vi "Lab Panel V4.5.vi"() -> ()   [LabVIEW 2013]
uses:
  <vilib>/Platform/TimedLoop/XDataNode/timing_clust.ctl
  <vilib>/Platform/TimedLoop/XDataNode/nitl_modes.ctl
  <vilib>/Platform/TimedLoop/XDataNode/wakeup.ctl
  Global 1.vi
  <vilib>/platform/TimedLoop/XDataNode/XDataNode.xnode
  <vilib>/Platform/TimedLoop/XDataNode/XDNodeRunTimeDep.lvlib
panel:
  in  "ADMIN PAGE":bool
  out "TEMP update":bool
  out "AI update":bool
  in  "Tab Control 2":T1(tab)
  out "SIG LAB05-2":T2 {"PF" format="%.2f"; "AMPS" format="%.1f"}
  out "SIG LAB05-1":T2 {"PF" format="%.2f"; "AMPS" format="%.1f"}
  out "SIG LAB04-2":T2 {"PF" format="%.2f"; "AMPS" format="%.1f"}
  out "SIG LAB04-1":T2 {"PF" format="%.2f"; "AMPS" format="%.1f"}
  out "SIG LAB03-2":T2 {"PF" format="%.2f"; "AMPS" format="%.1f"}
  out "SIG LAB03-1":T2 {"PF" format="%.2f"; "AMPS" format="%.1f"}
  out "SIG LAB02-2":T2 {"PF" format="%.2f"; "AMPS" format="%.1f"}
  in  "RUN LAB01-1":bool
  in  "O/I  LAB05-1":bool
  in  "O/I  LAB05-2":bool
  in  "O/I  LAB04-1":bool
  in  "O/I  LAB04-2":bool
  in  "O/I  LAB02-1":bool
  in  "O/I  LAB02-2":bool
  in  "O/I  LAB01-2":bool
  in  "O/I  LAB01-1":bool
  in  "O/I  LAB03-1":bool
  in  "RUN LAB05-2":bool
  in  "RUN LAB05-1":bool
  in  "RUN LAB04-2":bool
  in  "RUN LAB04-1":bool
  in  "RUN LAB03-2":bool
  in  "RUN LAB03-1":bool
  in  "RUN LAB02-2":bool
  in  "RUN LAB02-1":bool
  in  "RUN LAB01-2":bool
  in  "SELECT LAB05-2":T3(radio)
  in  "SELECT LAB05-1":T3(radio)
  in  "SELECT LAB04-2":T3(radio)
  in  "SELECT LAB04-1":T3(radio)
  in  "SELECT LAB03-2":T3(radio)
  in  "SELECT LAB03-1":T3(radio)
  in  "SELECT LAB02-2":T3(radio)
  in  "SELECT LAB02-1":T3(radio)
  in  "SELECT LAB01-2":T3(radio)
  in  "SELECT LAB01-1":T3(radio)
  in  "O/I  LAB03-2":bool
  out "SIG LAB01-1":T2 {"PF" format="%.2f"; "AMPS" format="%.1f"}
  out "SIG LAB01-2":T2 {"PF" format="%.2f"; "AMPS" format="%.1f"}
  out "SIG LAB02-1":T2 {"PF" format="%.2f"; "AMPS" format="%.1f"}
  out "DISP LAB05-2":T4 {"MINS" format="%.2g"}
  out "DISP LAB05-1":T4 {"MINS" format="%.2g"}
  out "DISP LAB04-2":T4 {"MINS" format="%.2g"}
  out "DISP LAB04-1":T4 {"MINS" format="%.2g"}
  out "DISP LAB03-2":T4 {"MINS" format="%.2g"}
  out "DISP LAB03-1":T4 {"MINS" format="%.2g"}
  in  "SET LAB05-2":T5={"NAME"="", "DESCRIPTION"="", "CYCLES"=5.0, "T-RISE mins"=0.0, "T-RISE deg C"=0.0} {"CYCLES" min=5.0 step=1.0}
  in  "SET LAB05-1":T5={"NAME"="", "DESCRIPTION"="", "CYCLES"=5.0, "T-RISE mins"=0.0, "T-RISE deg C"=0.0} {"CYCLES" min=5.0 step=1.0}
  in  "SET LAB04-2":T5={"NAME"="", "DESCRIPTION"="", "CYCLES"=5.0, "T-RISE mins"=0.0, "T-RISE deg C"=0.0} {"CYCLES" min=5.0 step=1.0}
  in  "SET LAB04-1":T5={"NAME"="", "DESCRIPTION"="", "CYCLES"=5.0, "T-RISE mins"=0.0, "T-RISE deg C"=0.0} {"CYCLES" min=5.0 step=1.0}
  in  "SET LAB03-2":T5={"NAME"="", "DESCRIPTION"="", "CYCLES"=5.0, "T-RISE mins"=0.0, "T-RISE deg C"=0.0} {"CYCLES" min=5.0 step=1.0}
  in  "SET LAB03-1":T5={"NAME"="", "DESCRIPTION"="", "CYCLES"=5.0, "T-RISE mins"=0.0, "T-RISE deg C"=0.0} {"CYCLES" min=5.0 step=1.0}
  out "DISP LAB02-2":T4 {"MINS" format="%.2g"}
  out "DISP LAB02-1":T4 {"MINS" format="%.2g"}
  in  "SET LAB02-2":T5={"NAME"="", "DESCRIPTION"="", "CYCLES"=5.0, "T-RISE mins"=0.0, "T-RISE deg C"=0.0} {"CYCLES" min=5.0 step=1.0}
  in  "SET LAB02-1":T5={"NAME"="", "DESCRIPTION"="", "CYCLES"=5.0, "T-RISE mins"=0.0, "T-RISE deg C"=0.0} {"CYCLES" min=5.0 step=1.0}
  out "RESULT LAB05-2":bool
  out "RESULT LAB05-1":bool
  out "RESULT LAB04-2":bool
  out "RESULT LAB04-1":bool
  out "RESULT LAB03-2":bool
  out "RESULT LAB03-1":bool
  out "RESULT LAB02-2":bool
  out "RESULT LAB02-1":bool
  out "RESULT LAB01-2":bool
  out "RESULT LAB01-1":bool
  in  "SET LAB01-1":T5={"NAME"="", "DESCRIPTION"="", "CYCLES"=5.0, "T-RISE mins"=0.0, "T-RISE deg C"=0.0} {"CYCLES" min=5.0 step=1.0}
  in  "SET LAB01-2":T5={"NAME"="", "DESCRIPTION"="", "CYCLES"=5.0, "T-RISE mins"=0.0, "T-RISE deg C"=0.0} {"CYCLES" min=5.0 step=1.0}
  out "DISP LAB01-1":T4 {"MINS" format="%.2g"}
  out "DISP LAB01-2":T4 {"MINS" format="%.2f"}
  out "TEMP RISE LAB05-2":cluster{"TL":dbl, "TN":dbl}
  out "TEMP RISE LAB05-1":cluster{"TL":dbl, "TN":dbl}
  out "TEMP RISE LAB04-2":cluster{"TL":dbl, "TN":dbl}
  out "TEMP RISE LAB04-1":cluster{"TL":dbl, "TN":dbl}
  out "TEMP RISE LAB03-2":cluster{"TL":dbl, "TN":dbl}
  out "TEMP RISE LAB03-1":cluster{"TL":dbl, "TN":dbl}
  out "TEMP RISE LAB02-2":cluster{"TL":dbl, "TN":dbl}
  out "TEMP RISE LAB02-1":cluster{"TL":dbl, "TN":dbl}
  out "TEMP RISE LAB01-2":cluster{"TL":dbl, "TN":dbl}
  out "TEMP RISE LAB01-1":cluster{"TL":dbl, "TN":dbl}
  in  "JIG OFF TIME (S)":dbl=2.0 min=2.0 max=10.0 step=0.5 format="%.1g"
  in  "JIG ON TIME (S)":dbl=1.0 min=1.0 max=10.0 step=0.5 format="%.1g"
  out "JIG LAB05-2":bool
  out "JIG LAB05-1":bool
  out "JIG LAB04-2":bool
  out "JIG LAB04-1":bool
  out "JIG LAB03-2":bool
  out "JIG LAB03-1":bool
  out "JIG LAB02-2":bool
  out "JIG LAB02-1":bool
  out "JIG LAB01-2":bool
  out "JIG LAB01-1":bool
  out "TEMP START LAB01-1":cluster{"TL":dbl, "TN":dbl}
  out "TEMP START LAB02-1":cluster{"TL":dbl, "TN":dbl}
  out "TEMP START LAB03-1":cluster{"TL":dbl, "TN":dbl}
  out "TEMP START LAB04-1":cluster{"TL":dbl, "TN":dbl}
  out "TEMP START LAB01-2":cluster{"TL":dbl, "TN":dbl}
  out "TEMP START LAB02-2":cluster{"TL":dbl, "TN":dbl}
  out "TEMP START LAB03-2":cluster{"TL":dbl, "TN":dbl}
  out "TEMP START LAB04-2":cluster{"TL":dbl, "TN":dbl}
  out "TEMP START LAB05-2":cluster{"TL":dbl, "TN":dbl}
  out "TEMP START LAB05-1":cluster{"TL":dbl, "TN":dbl}
  in  "MAIL SETTINGS":T6
  out "MAIL REPORT":string
  in  "TO (string):":string
  in  "Send Mail Now":bool
  in  "Auto Mail Send":bool
  in  "Network Directory":path
  out "CAL LAB01":T7 {"2 (TN) cal" min=0.0 step=0.01 format="%.2f"; "2 (TL) cal" min=0.0 step=0.01 format="%.2f"; "2 (PF) cal" min=0.0 step=0.01 format="%.2f"; "2 (V) cal" min=0.0 step=0.01 format="%.2f"; "2 (A) cal" min=0.0 step=0.01 format="%.2f"; "1 (TN) cal" min=0.0 step=0.01 format="%.2f"; "1 (TL) cal" min=0.0 step=0.01 format="%.2f"; "1 (PF) cal" min=0.0 step=0.01 format="%.2f"; "1 (V) cal" min=0.0 step=0.01 format="%.2f"; "1  (A) cal" min=0.0 step=0.01 format="%.2f"}
  out "CAL LAB03":T7 {"2 (TN) cal" min=0.0 step=0.01 format="%.2f"; "2 (TL) cal" min=0.0 step=0.01 format="%.2f"; "2 (PF) cal" min=0.0 step=0.01 format="%.2f"; "2 (V) cal" min=0.0 step=0.01 format="%.2f"; "2 (A) cal" min=0.0 step=0.01 format="%.2f"; "1 (TN) cal" min=0.0 step=0.01 format="%.2f"; "1 (TL) cal" min=0.0 step=0.01 format="%.2f"; "1 (PF) cal" min=0.0 step=0.01 format="%.2f"; "1 (V) cal" min=0.0 step=0.01 format="%.2f"; "1  (A) cal" min=0.0 step=0.01 format="%.2f"}
  out "CAL LAB02":T8 {"2 (TN) cal" min=0.0 step=0.01 format="%.2f"; "2 (TL) cal" min=0.0 step=0.01 format="%.2f"; "2 (PF) cal" min=0.0 step=0.01 format="%.2f"; "2 (V) cal" min=0.0 step=0.01 format="%.2f"; "2 (A) cal" min=0.0 step=0.01 format="%.2f"; "1 (TN) cal" min=0.0 step=0.01 format="%.2f"; "1 (TL) cal" min=0.0 step=0.01 format="%.2f"; "1 (PF) cal" min=0.0 step=0.01 format="%.2f"; "1 (V) cal" min=0.0 step=0.01 format="%.2f"; "1 (A) cal" min=0.0 step=0.01 format="%.2f"}
  out "CAL LAB05":T7 {"2 (TN) cal" min=0.0 step=0.01 format="%.2f"; "2 (TL) cal" min=0.0 step=0.01 format="%.2f"; "2 (PF) cal" min=0.0 step=0.01 format="%.2f"; "2 (V) cal" min=0.0 step=0.01 format="%.2f"; "2 (A) cal" min=0.0 step=0.01 format="%.2f"; "1 (TN) cal" min=0.0 step=0.01 format="%.2f"; "1 (TL) cal" min=0.0 step=0.01 format="%.2f"; "1 (PF) cal" min=0.0 step=0.01 format="%.2f"; "1 (V) cal" min=0.0 step=0.01 format="%.2f"; "1  (A) cal" min=0.0 step=0.01 format="%.2f"}
  out "CAL LAB04":T7 {"2 (TN) cal" min=0.0 step=0.01 format="%.2f"; "2 (TL) cal" min=0.0 step=0.01 format="%.2f"; "2 (PF) cal" min=0.0 step=0.01 format="%.2f"; "2 (V) cal" min=0.0 step=0.01 format="%.2f"; "2 (A) cal" min=0.0 step=0.01 format="%.2f"; "1 (TN) cal" min=0.0 step=0.01 format="%.2f"; "1 (TL) cal" min=0.0 step=0.01 format="%.2f"; "1 (PF) cal" min=0.0 step=0.01 format="%.2f"; "1 (V) cal" min=0.0 step=0.01 format="%.2f"; "1  (A) cal" min=0.0 step=0.01 format="%.2f"}
  out "calibration file error out":errorcluster
  in  "CALIBRATE":bool
  out "ON L05-2":cluster{"amps":dbl, "volts":dbl, "pf":dbl}
  out "ON L05-1":cluster{"amps":dbl, "volts":dbl, "pf":dbl}
  out "FAIL LAB05-2":cluster{"LO":dbl, "HI":dbl}
  out "FAIL LAB05-1":cluster{"LO":dbl, "HI":dbl}
  out "FAIL LAB04-2":cluster{"LO":dbl, "HI":dbl}
  out "FAIL LAB04-1":cluster{"LO":dbl, "HI":dbl}
  out "FAIL LAB03-2":cluster{"LO":dbl, "HI":dbl}
  out "FAIL LAB03-1":cluster{"LO":dbl, "HI":dbl}
  out "FAIL LAB02-2":cluster{"LO":dbl, "HI":dbl}
  out "FAIL LAB02-1":cluster{"LO":dbl, "HI":dbl}
  out "FAIL LAB01-2":cluster{"LO":dbl, "HI":dbl}
  out "FAIL LAB01-1":cluster{"LO":dbl, "HI":dbl}
  out "ON L01-1":cluster{"amps":dbl, "volts":dbl, "pf":dbl}
  out "ON L01-2":cluster{"amps":dbl, "volts":dbl, "pf":dbl}
  out "ON L02-1":cluster{"amps":dbl, "volts":dbl, "pf":dbl}
  out "ON L02-2":cluster{"amps":dbl, "volts":dbl, "pf":dbl}
  out "ON L03-1":cluster{"amps":dbl, "volts":dbl, "pf":dbl}
  out "ON L03-2":cluster{"amps":dbl, "volts":dbl, "pf":dbl}
  out "ON L04-1":cluster{"amps":dbl, "volts":dbl, "pf":dbl}
  out "ON L04-2":cluster{"amps":dbl, "volts":dbl, "pf":dbl}
  out "TEST VOLTS CHART":T9(graph)
  in  "Select  Cycle":enum32{"ON CYCLE", "OFF CYCLE"}(radio)
  out "TEST AMPS CHART":T9(graph)
  out "TEMPERATURE (N) CHART":T9(graph)
  out "TEMPERATURE (L) CHART":T9(graph)
  in  "SAMPLES":dbl
  in  "RATE (Hz)":dbl
  in  "JIG TEST":T10
  in  "C drive data root dir":path
  out "run lab05-2":bool
  out "run lab05-1":bool
  out "run lab04-2":bool
  out "run lab04-1":bool
  out "run lab03-2":bool
  out "run lab03-1":bool
  out "run lab02-2":bool
  out "run lab02-1":bool
  out "run lab01-2":bool
  out "run lab01-1":bool
  out "stop2":bool
  in  "Tab Control":T11(tab)
  out "LAB01-2 (GRAPH)":dynamicdata(graph)
  out "LAB01-1 (GRAPH)":dynamicdata(graph)
  out "LAB02-2 (GRAPH)":dynamicdata(graph)
  out "LAB02-1 (GRAPH)":dynamicdata(graph)
  out "LAB03-2 (GRAPH)":dynamicdata(graph)
  out "LAB03-1 (GRAPH)":dynamicdata(graph)
  out "LAB04-2 (GRAPH)":dynamicdata(graph)
  out "LAB04-1 (GRAPH)":dynamicdata(graph)
  out "LAB05-2 (GRAPH)":dynamicdata(graph)
  out "LAB05-1 (GRAPH)":dynamicdata(graph)
  out "LAB05 TEMP":T12
  out "LAB04 TEMP":T12
  out "LAB02 TEMP":T12
  out "LAB01 TEMP":T12
  out "LAB03 TEMP":T12
  out "Analog Error Array":errorcluster[](array[cluster])
  out "AI loop time":dbl format="%.6g"
  out "loops":dbl
  in  "loop  delay(mS)":dbl
  out "on loops":dbl
  out "off loops":dbl
  out "jig cycle":dbl
  out "TDMS LAB01-1":refnum<k34>
  out "data file error":errorcluster
  out "TDMS LAB02-1":refnum<k34>
  out "TDMS LAB01-2":refnum<k34>
  out "TDMS LAB02-2":refnum<k34>
  out "TDMS LAB03-1":refnum<k34>
  out "TDMS LAB03-2":refnum<k34>
  out "TDMS LAB04-1":refnum<k34>
  out "TDMS LAB04-2":refnum<k34>
  out "TDMS LAB05-1":refnum<k34>
  out "TDMS LAB05-2":refnum<k34>
  out "mail control":string
  out "File Time Stamp":timestamp
  in  "stop":bool
  # "LAB01"
  # "LAB02"
  # "LAB05"
  # "LAB03"
  # "LAB04"
  # "LAB01"
  # "LAB02"
  # "LAB03"
  # "LAB04"
  # "LAB05"
  # "JIG SET"
  # "(Enter recipients address seperated by comma)"
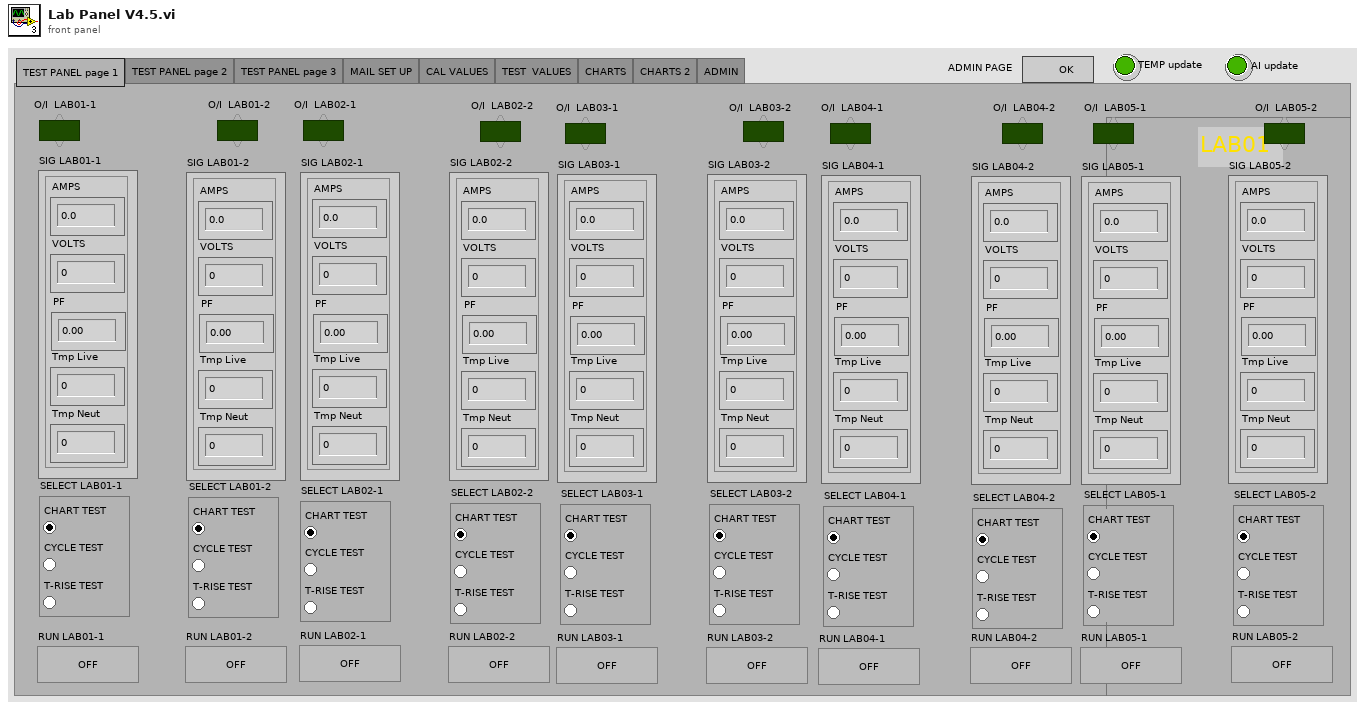
[diagram p1: front panel]
types:
  T1 = enum32{"TEST PANEL page 1", "TEST PANEL page 2", "TEST PANEL page 3", "MAIL SET UP", "CAL VALUES", "TEST  VALUES", "CHARTS", "CHARTS 2", "ADMIN"}
  T2 = cluster{"AMPS":dbl, "VOLTS":dbl, "PF":dbl, "Tmp Live":dbl, "Tmp Neut":dbl}
  T3 = enum32{"CHART TEST", "CYCLE TEST", "T-RISE TEST"}
  T4 = cluster{"CYCLE":dbl, "MINS":dbl, "STATUS":string}
  T5 = cluster{"NAME":string, "DESCRIPTION":string, "CYCLES":dbl, "T-RISE mins":dbl, "T-RISE deg C":dbl}
  T6 = cluster{"OUT SERVER ADDRESS":string, "FROM ACCOUNT":string, "USER NAME":string, "PASSWORD":string, "TEST MAIL":bool, "TEST MAIL STATUS":string, "mail error":errorcluster}
  T7 = cluster{"1  (A) cal":dbl, "1 (V) cal":dbl, "1 (PF) cal":dbl, "1 (TL) cal":dbl, "1 (TN) cal":dbl, "2 (A) cal":dbl, "2 (V) cal":dbl, "2 (PF) cal":dbl, "2 (TL) cal":dbl, "2 (TN) cal":dbl}
  T8 = cluster{"1 (A) cal":dbl, "1 (V) cal":dbl, "1 (PF) cal":dbl, "1 (TL) cal":dbl, "1 (TN) cal":dbl, "2 (A) cal":dbl, "2 (V) cal":dbl, "2 (PF) cal":dbl, "2 (TL) cal":dbl, "2 (TN) cal":dbl}
  T9 = cluster{"AMPS":dbl, "AMPS":dbl, "AMPS":dbl, "AMPS":dbl, "AMPS":dbl, "AMPS":dbl, "AMPS":dbl, "AMPS":dbl, "AMPS":dbl, "AMPS":dbl}
  T10 = cluster{" LAB01-1":bool, " LAB01-2":bool, "LAB02-1":bool, " LAB02-2":bool, "LAB03-1":bool, "LAB03-2":bool, "LAB04-1":bool, "LAB04-2":bool, "LAB05-1":bool, "LAB05-2":bool}
  T11 = enum32{"LAB01", "LAB02", "LAB03", "LAB04", "LAB05", "TEMPERATURE", "ERROR"}
  T12 = cluster{"T1 Live":dbl, "T1 Neut":dbl, "T2 Live":dbl, "T2 Neut":dbl, "ID":dbl, "ER":dbl}
  T13 = enum8{"Enabled", "Disabled", "Disabled and Grayed Out"}
  T14 = typedef "XDNodeRunTimeDep.lvlib/timing_clust.ctl" = cluster{"Expected End [f-1]":u64, "Actual End [f-1]":u64, "Finished Late? [f-1]":bool, "Expected End [i-1]":u64, "Actual End [i-1]":u64, "Finished Late? [i-1]":bool, "Expected Start [i]":u64, "Actual Start [i]":u64, "Expected Start [f]":u64, "Actual Start [f]":u64, "Source Name":string, "Structure Name":string, "Period":i64, "Deadline":i64, "Offset":i64, "Start":i64, "Priority":i32, "Timeout":i32, "Mode":T15, "Wakeup Reason":T16, "Error":errorcluster, "Source Type":string, "Secondary Source Type":string, "Global End Time":u64, "Global Start Time":u64, "Frame Duration":u64, "Iteration Duration":u64, "Assigned CPU":i32, "I/O Scan Engine Mode":u32}
  T15 = typedef "XDNodeRunTimeDep.lvlib/nitl_modes.ctl" = enum32{"No Change", "Process missed periods, maintain original phase", "Discard missed periods, maintain original phase", "Process missed periods, ignore original phase", "Discard missed periods, ignore original phase"}
  T16 = typedef "XDNodeRunTimeDep.lvlib/wakeup.ctl" = enum32{"Normal", "Aborted", "Asynchronous wakeup", "Timing source error", "Timed loop error", "Timeout"}
  T17 = enum16{"open", "open or create", "create or replace", "create", "open (read-only)"}
  T18 = enum16{"open", "replace", "create", "open or create", "replace or create", "replace or create with confirmation"}
  T19 = cluster{"SET LAB01-1":cluster{"NAME":string, "DESCRIPTION":string, "CYCLES":dbl, "T-RISE mins":dbl, "T-RISE deg C":dbl}, "SET LAB01-2":cluster{"NAME":string, "DESCRIPTION":string, "CYCLES":dbl, "T-RISE mins":dbl, "T-RISE deg C":dbl}, "SET LAB02-1":cluster{"NAME":string, "DESCRIPTION":string, "CYCLES":dbl, "T-RISE mins":dbl, "T-RISE deg C":dbl}, "SET LAB02-2":cluster{"NAME":string, "DESCRIPTION":string, "CYCLES":dbl, "T-RISE mins":dbl, "T-RISE deg C":dbl}, "SET LAB03-1":cluster{"NAME":string, "DESCRIPTION":string, "CYCLES":dbl, "T-RISE mins":dbl, "T-RISE deg C":dbl}, "SET LAB03-2":cluster{"NAME":string, "DESCRIPTION":string, "CYCLES":dbl, "T-RISE mins":dbl, "T-RISE deg C":dbl}, "SET LAB04-1":cluster{"NAME":string, "DESCRIPTION":string, "CYCLES":dbl, "T-RISE mins":dbl, "T-RISE deg C":dbl}, "SET LAB04-2":cluster{"NAME":string, "DESCRIPTION":string, "CYCLES":dbl, "T-RISE mins":dbl, "T-RISE deg C":dbl}, "SET LAB05-1":cluster{"NAME":string, "DESCRIPTION":string, "CYCLES":dbl, "T-RISE mins":dbl, "T-RISE deg C":dbl}, "SET LAB05-2":cluster{"NAME":string, "DESCRIPTION":string, "CYCLES":dbl, "T-RISE mins":dbl, "T-RISE deg C":dbl}, "Network Directory":path, "C drive data root dir":path, "RATE (Hz)":dbl, "SAMPLES":dbl}
  T20 = cluster{"MAIL SETTINGS":cluster{"OUT SERVER ADDRESS":string, "FROM ACCOUNT":string, "USER NAME":string, "PASSWORD":string, "TEST MAIL":bool, "TEST MAIL STATUS":string, "mail error":errorcluster}, "Auto Mail Send":bool, string}
  T21 = cluster{"T1":dbl, "T2":dbl, "T3":dbl, "T4":dbl, "ID":dbl, "ER":dbl}
  T22 = cluster{"LAB01-1 (A)":dbl, "LAB01-1 (V)":dbl, "LAB01-1 (PF)":dbl, "LAB01-2 (A)":dbl, "LAB01-2 (V)":dbl, "LAB01-2 (PF)":dbl}
  T23 = cluster{"LAB02-1 (A)":dbl, "LAB02-1 (V)":dbl, "LAB02-1 (PF)":dbl, "LAB02-2 (A)":dbl, "LAB02-2 (V)":dbl, "LAB02-2 (PF)":dbl}
  T24 = cluster{"LAB03-1 (A)":dbl, "LAB03-1 (V)":dbl, "LAB03-1 (PF)":dbl, "LAB03-2 (A)":dbl, "LAB03-2 (V)":dbl, "LAB03-2 (PF)":dbl}
  T25 = cluster{"LAB04-1 (A)":dbl, "LAB04-1 (V)":dbl, "LAB04-1 (PF)":dbl, "LAB04-2 (A)":dbl, "LAB04-2 (V)":dbl, "LAB04-2 (PF)":dbl}
  T26 = cluster{"LAB05-1 (A)":dbl, "LAB05-1 (V)":dbl, "LAB05-1 (PF)":dbl, "LAB05-2 (A)":dbl, "LAB05-2 (V)":dbl, "LAB05-2 (PF)":dbl}
  T27 = cluster{"VOLTS":dbl, "VOLTS":dbl, "VOLTS":dbl, "VOLTS":dbl, "VOLTS":dbl, "VOLTS":dbl, "VOLTS":dbl, "VOLTS":dbl, "VOLTS":dbl, "VOLTS":dbl}
  T28 = cluster{"Tmp Live":dbl, "Tmp Live":dbl, "Tmp Live":dbl, "Tmp Live":dbl, "Tmp Live":dbl, "Tmp Live":dbl, "Tmp Live":dbl, "Tmp Live":dbl, "Tmp Live":dbl, "Tmp Live":dbl}
  T29 = cluster{"Tmp Neut":dbl, "Tmp Neut":dbl, "Tmp Neut":dbl, "Tmp Neut":dbl, "Tmp Neut":dbl, "Tmp Neut":dbl, "Tmp Neut":dbl, "Tmp Neut":dbl, "Tmp Neut":dbl, "Tmp Neut":dbl}
  T30 = cluster{"FAIL LAB01-1":cluster{"LO":dbl, "HI":dbl}, "SIG LAB01-1":cluster{"AMPS":dbl, "VOLTS":dbl, "PF":dbl, "Tmp Live":dbl, "Tmp Neut":dbl}, "TEMP START LAB01-1":cluster{"TL":dbl, "TN":dbl}, "DISP LAB01-1":cluster{"CYCLE":dbl, "MINS":dbl, "STATUS":string}, "SET LAB01-1":cluster{"NAME":string, "DESCRIPTION":string, "CYCLES":dbl, "T-RISE mins":dbl, "T-RISE deg C":dbl}, "TDMS LAB01-1":refnum<k34>}
  T31 = cluster{"FAIL LAB01-2":cluster{"LO":dbl, "HI":dbl}, "SIG LAB01-2":cluster{"AMPS":dbl, "VOLTS":dbl, "PF":dbl, "Tmp Live":dbl, "Tmp Neut":dbl}, "TEMP START LAB01-2":cluster{"TL":dbl, "TN":dbl}, "DISP LAB01-2":cluster{"CYCLE":dbl, "MINS":dbl, "STATUS":string}, "SET LAB01-2":cluster{"NAME":string, "DESCRIPTION":string, "CYCLES":dbl, "T-RISE mins":dbl, "T-RISE deg C":dbl}, "TDMS LAB01-2":refnum<k34>}
  T32 = cluster{"FAIL LAB02-1":cluster{"LO":dbl, "HI":dbl}, "SIG LAB02-1":cluster{"AMPS":dbl, "VOLTS":dbl, "PF":dbl, "Tmp Live":dbl, "Tmp Neut":dbl}, "TEMP START LAB02-1":cluster{"TL":dbl, "TN":dbl}, "DISP LAB02-1":cluster{"CYCLE":dbl, "MINS":dbl, "STATUS":string}, "SET LAB02-1":cluster{"NAME":string, "DESCRIPTION":string, "CYCLES":dbl, "T-RISE mins":dbl, "T-RISE deg C":dbl}, "TDMS LAB02-1":refnum<k34>}
  T33 = cluster{"FAIL LAB02-2":cluster{"LO":dbl, "HI":dbl}, "SIG LAB02-2":cluster{"AMPS":dbl, "VOLTS":dbl, "PF":dbl, "Tmp Live":dbl, "Tmp Neut":dbl}, "TEMP START LAB02-2":cluster{"TL":dbl, "TN":dbl}, "DISP LAB02-2":cluster{"CYCLE":dbl, "MINS":dbl, "STATUS":string}, "SET LAB02-2":cluster{"NAME":string, "DESCRIPTION":string, "CYCLES":dbl, "T-RISE mins":dbl, "T-RISE deg C":dbl}, "TDMS LAB02-2":refnum<k34>}
  T34 = cluster{"FAIL LAB03-1":cluster{"LO":dbl, "HI":dbl}, "SIG LAB03-1":cluster{"AMPS":dbl, "VOLTS":dbl, "PF":dbl, "Tmp Live":dbl, "Tmp Neut":dbl}, "TEMP START LAB03-1":cluster{"TL":dbl, "TN":dbl}, "DISP LAB03-1":cluster{"CYCLE":dbl, "MINS":dbl, "STATUS":string}, "SET LAB03-1":cluster{"NAME":string, "DESCRIPTION":string, "CYCLES":dbl, "T-RISE mins":dbl, "T-RISE deg C":dbl}, "TDMS LAB03-1":refnum<k34>}
  T35 = cluster{"FAIL LAB03-2":cluster{"LO":dbl, "HI":dbl}, "SIG LAB03-2":cluster{"AMPS":dbl, "VOLTS":dbl, "PF":dbl, "Tmp Live":dbl, "Tmp Neut":dbl}, "TEMP START LAB03-2":cluster{"TL":dbl, "TN":dbl}, "DISP LAB03-2":cluster{"CYCLE":dbl, "MINS":dbl, "STATUS":string}, "SET LAB03-2":cluster{"NAME":string, "DESCRIPTION":string, "CYCLES":dbl, "T-RISE mins":dbl, "T-RISE deg C":dbl}, "TDMS LAB03-2":refnum<k34>}
  T36 = cluster{"FAIL LAB04-1":cluster{"LO":dbl, "HI":dbl}, "SIG LAB04-1":cluster{"AMPS":dbl, "VOLTS":dbl, "PF":dbl, "Tmp Live":dbl, "Tmp Neut":dbl}, "TEMP START LAB04-1":cluster{"TL":dbl, "TN":dbl}, "DISP LAB04-1":cluster{"CYCLE":dbl, "MINS":dbl, "STATUS":string}, "SET LAB04-1":cluster{"NAME":string, "DESCRIPTION":string, "CYCLES":dbl, "T-RISE mins":dbl, "T-RISE deg C":dbl}, "TDMS LAB04-1":refnum<k34>}
  T37 = cluster{"FAIL LAB04-2":cluster{"LO":dbl, "HI":dbl}, "SIG LAB04-2":cluster{"AMPS":dbl, "VOLTS":dbl, "PF":dbl, "Tmp Live":dbl, "Tmp Neut":dbl}, "TEMP START LAB04-2":cluster{"TL":dbl, "TN":dbl}, "DISP LAB04-2":cluster{"CYCLE":dbl, "MINS":dbl, "STATUS":string}, "SET LAB04-2":cluster{"NAME":string, "DESCRIPTION":string, "CYCLES":dbl, "T-RISE mins":dbl, "T-RISE deg C":dbl}, "TDMS LAB04-2":refnum<k34>}
  T38 = cluster{"FAIL LAB05-1":cluster{"LO":dbl, "HI":dbl}, "SIG LAB05-1":cluster{"AMPS":dbl, "VOLTS":dbl, "PF":dbl, "Tmp Live":dbl, "Tmp Neut":dbl}, "TEMP START LAB05-1":cluster{"TL":dbl, "TN":dbl}, "DISP LAB05-1":cluster{"CYCLE":dbl, "MINS":dbl, "STATUS":string}, "SET LAB05-1":cluster{"NAME":string, "DESCRIPTION":string, "CYCLES":dbl, "T-RISE mins":dbl, "T-RISE deg C":dbl}, "TDMS LAB05-1":refnum<k34>}
  T39 = cluster{"FAIL LAB05-2":cluster{"LO":dbl, "HI":dbl}, "SIG LAB05-2":cluster{"AMPS":dbl, "VOLTS":dbl, "PF":dbl, "Tmp Live":dbl, "Tmp Neut":dbl}, "TEMP START LAB05-2":cluster{"TL":dbl, "TN":dbl}, "DISP LAB05-2":cluster{"CYCLE":dbl, "MINS":dbl, "STATUS":string}, "SET LAB05-2":cluster{"NAME":string, "DESCRIPTION":string, "CYCLES":dbl, "T-RISE mins":dbl, "T-RISE deg C":dbl}, "TDMS LAB05-2":refnum<k34>}
  T40 = cluster{"MAIL SETTINGS":cluster{"OUT SERVER ADDRESS":string, "FROM ACCOUNT":string, "USER NAME":string, "PASSWORD":string, "TEST MAIL":bool, "TEST MAIL STATUS":string, "mail error":errorcluster}, "Auto Mail Send":bool, "TO (string):":string}
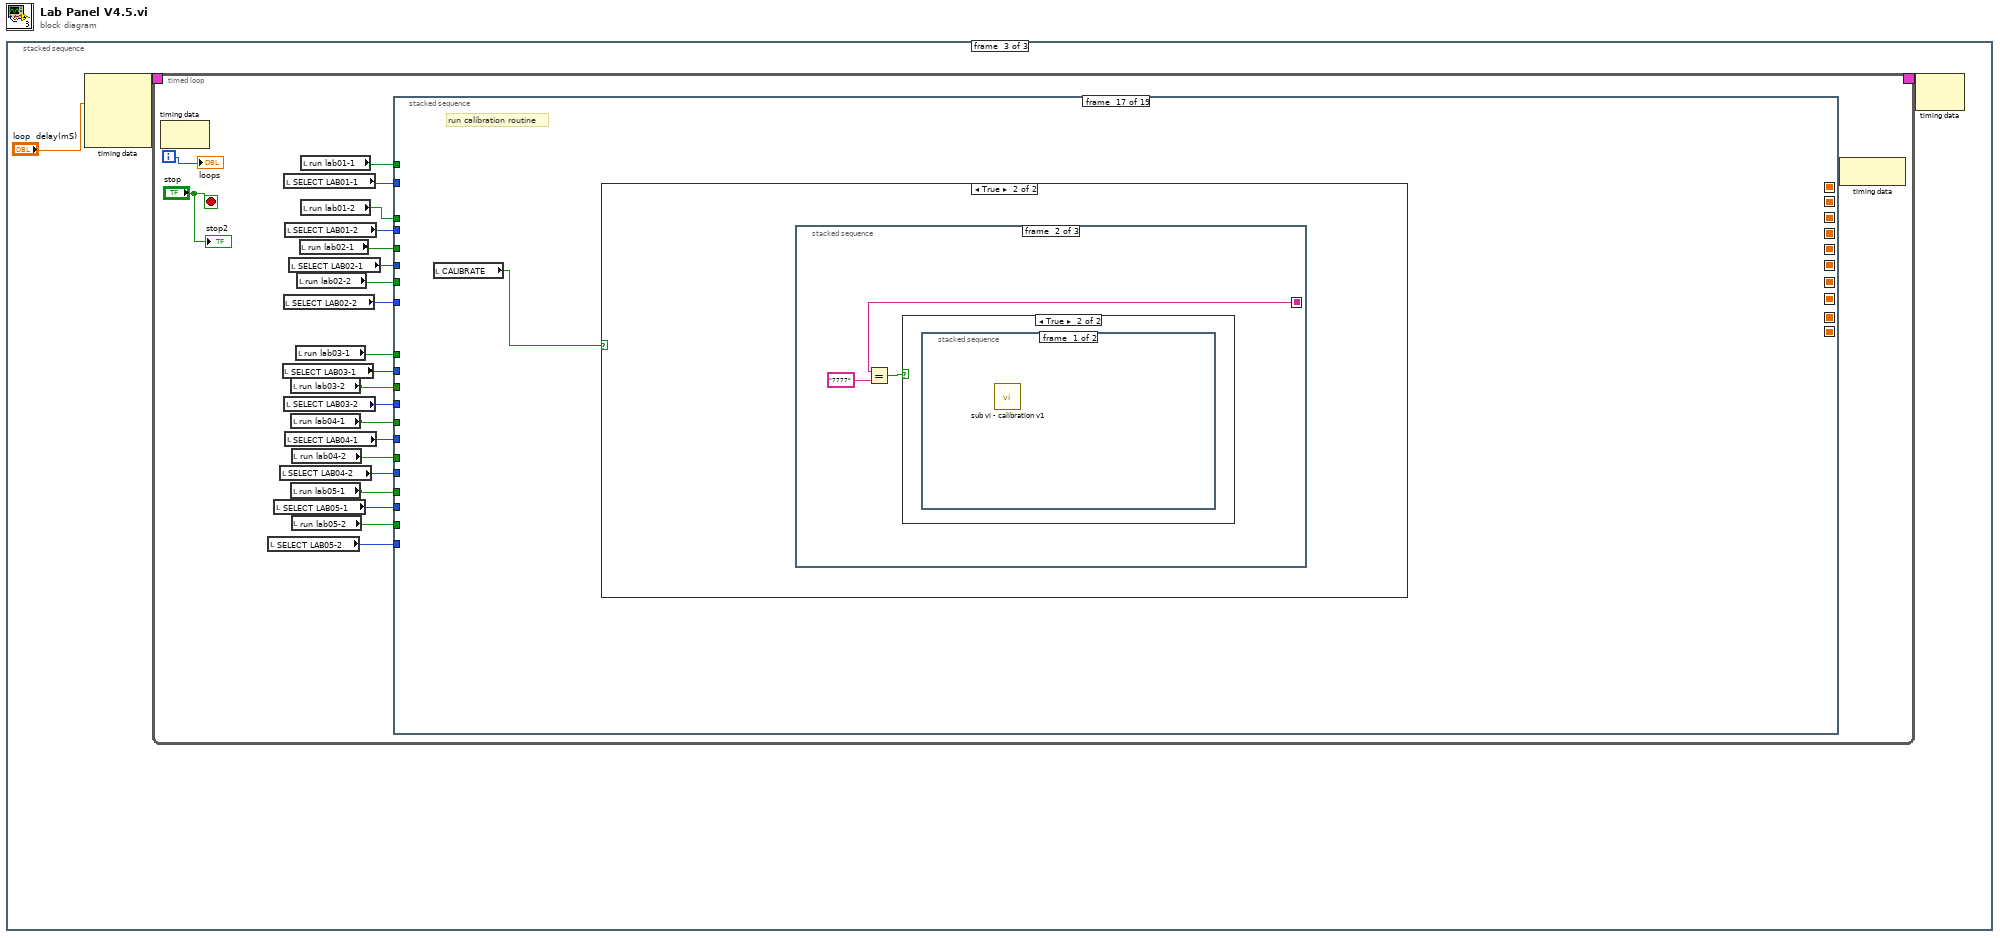
[diagram p0: block diagram]
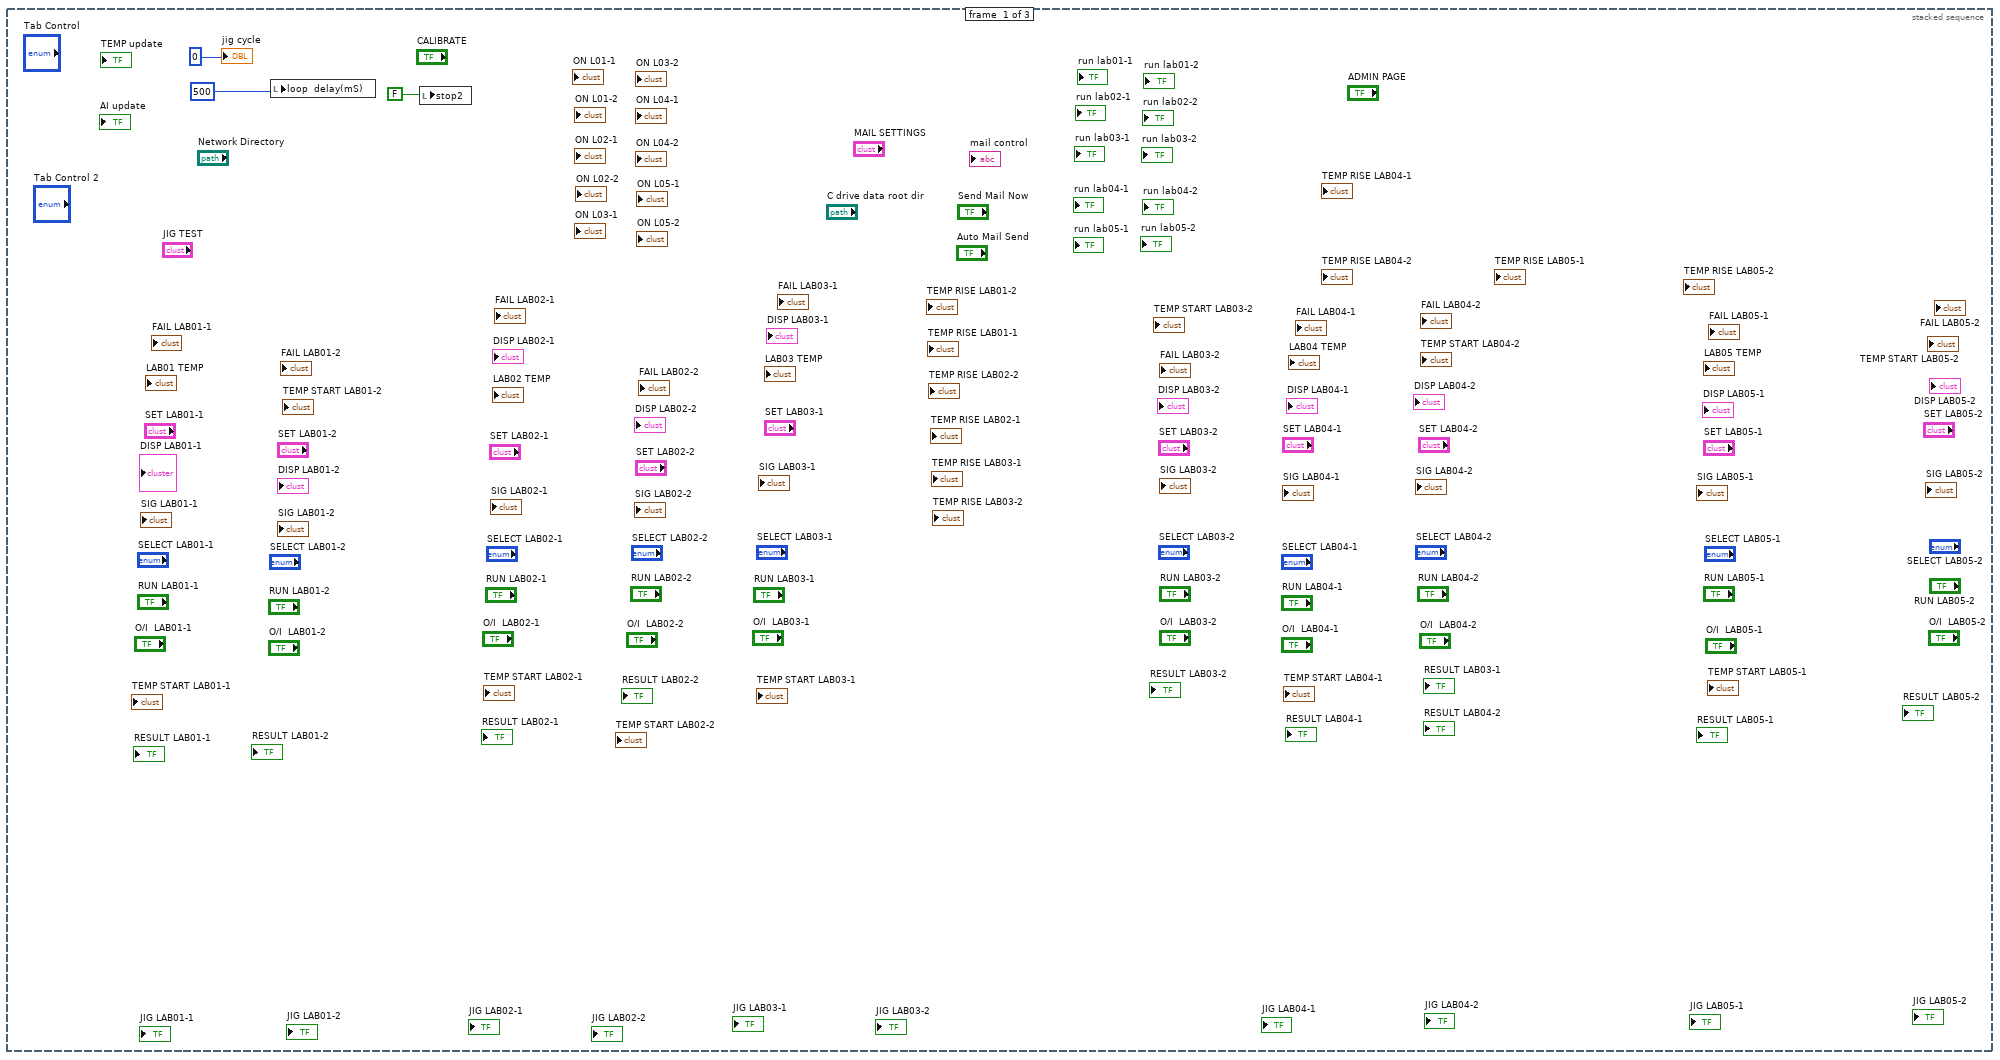
[diagram p2: hidden frame]
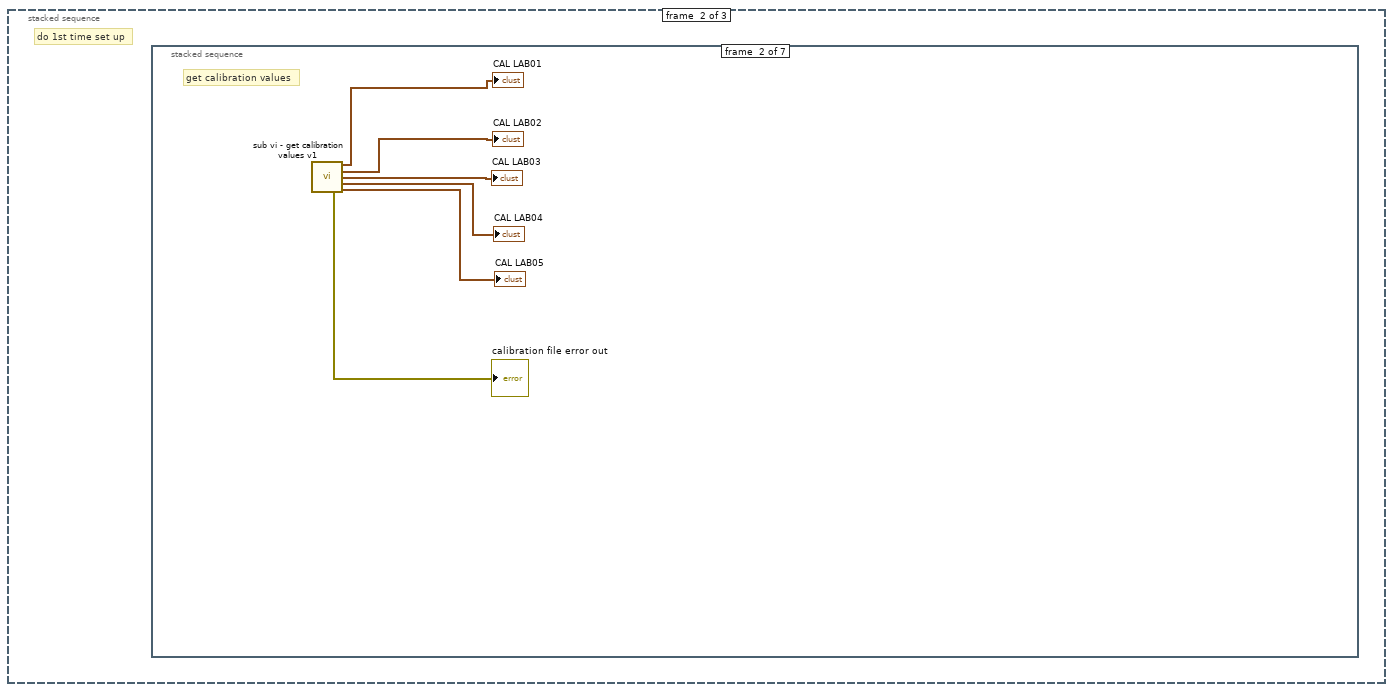
[diagram p3: hidden frame]
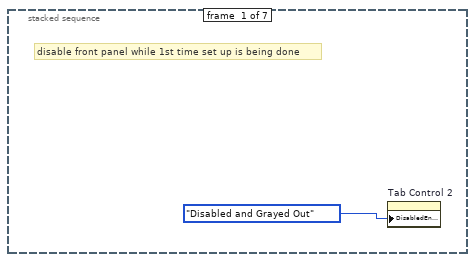
[diagram p4: hidden frame]
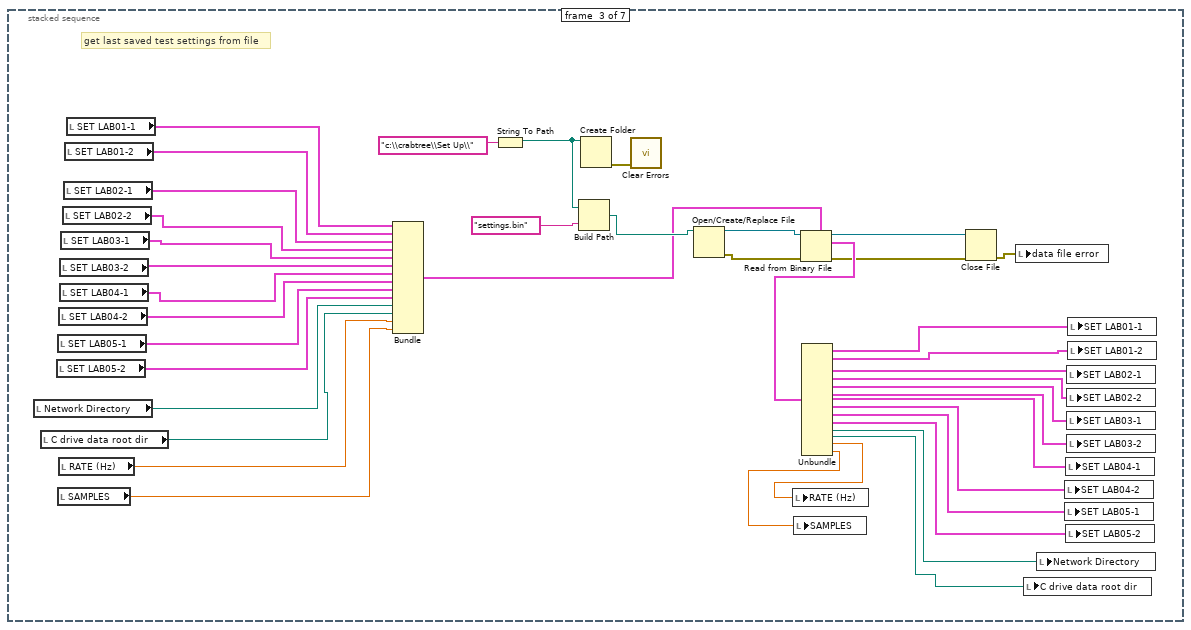
[diagram p5: hidden frame]
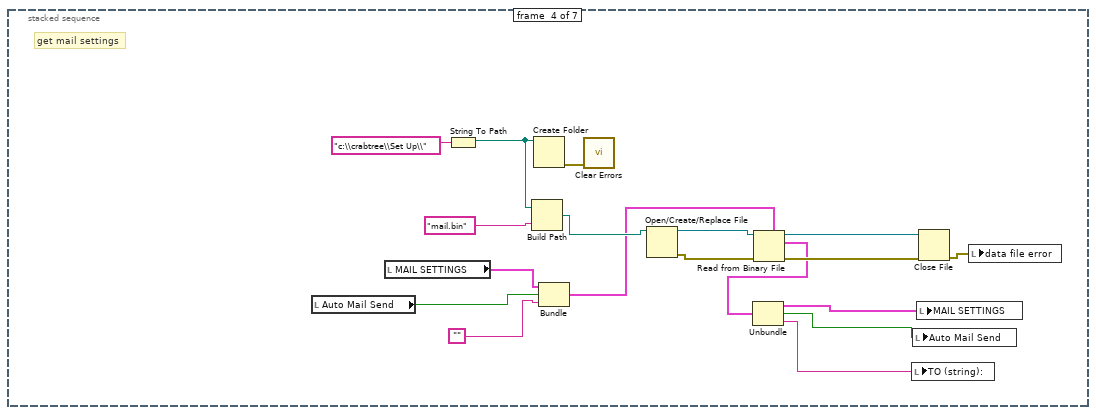
[diagram p6: hidden frame]
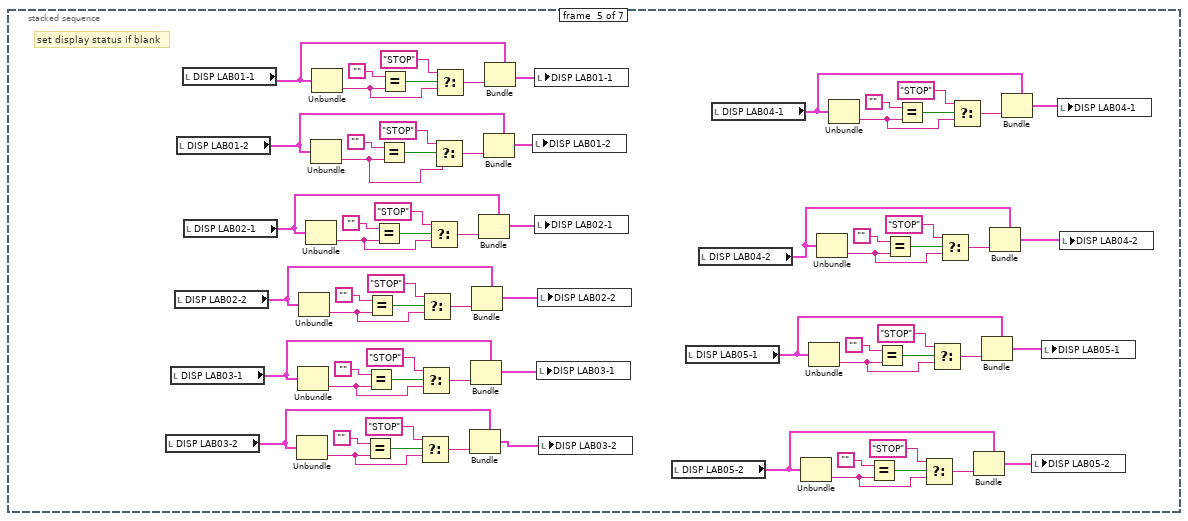
[diagram p7: hidden frame]
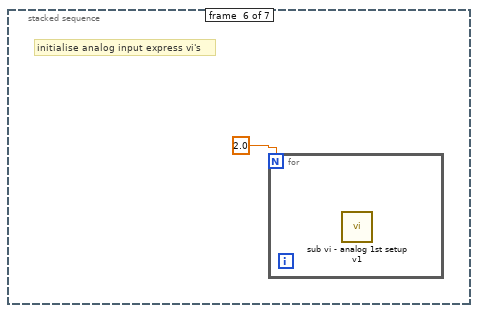
[diagram p8: hidden frame]
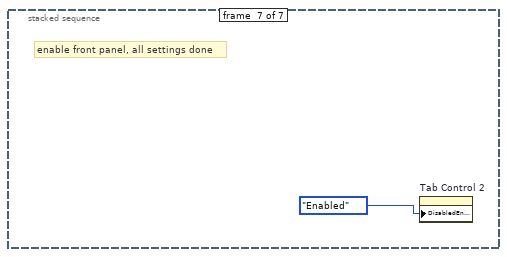
[diagram p9: hidden frame]
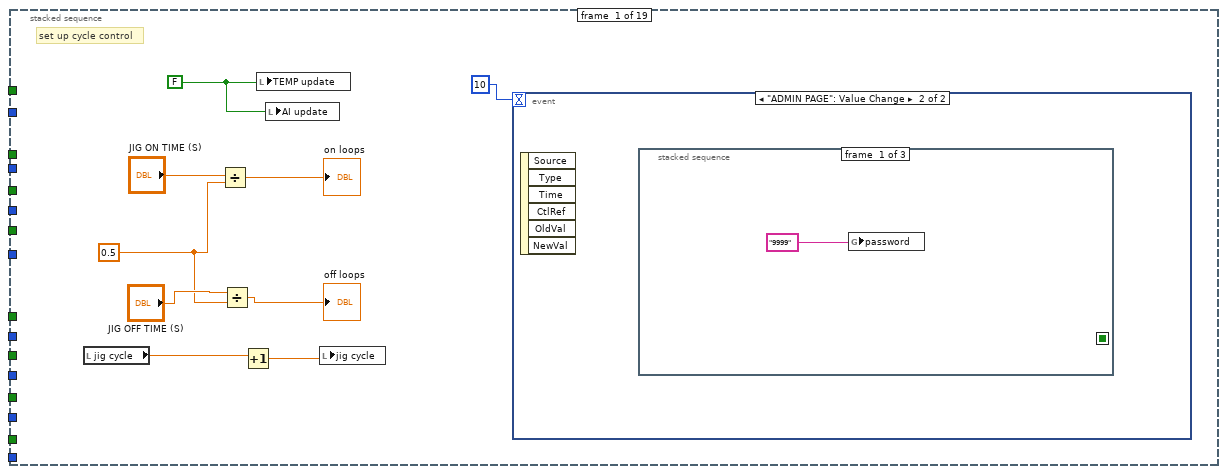
[diagram p10: hidden frame]
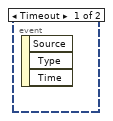
[diagram p11: hidden frame]
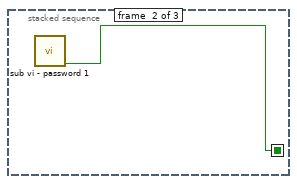
[diagram p12: hidden frame]
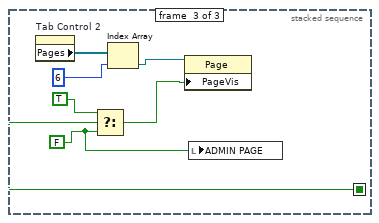
[diagram p13: hidden frame]
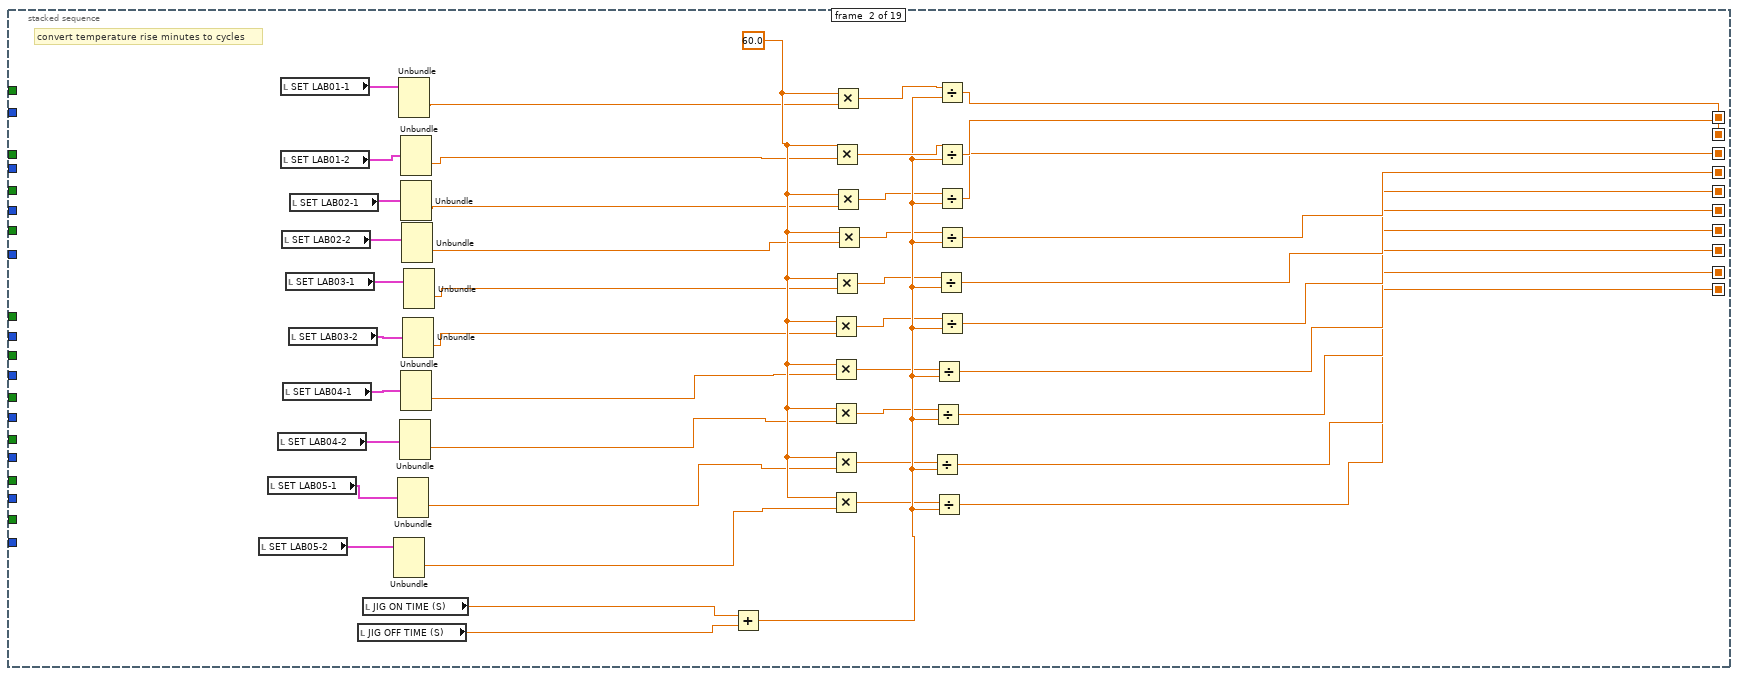
[diagram p14: hidden frame]
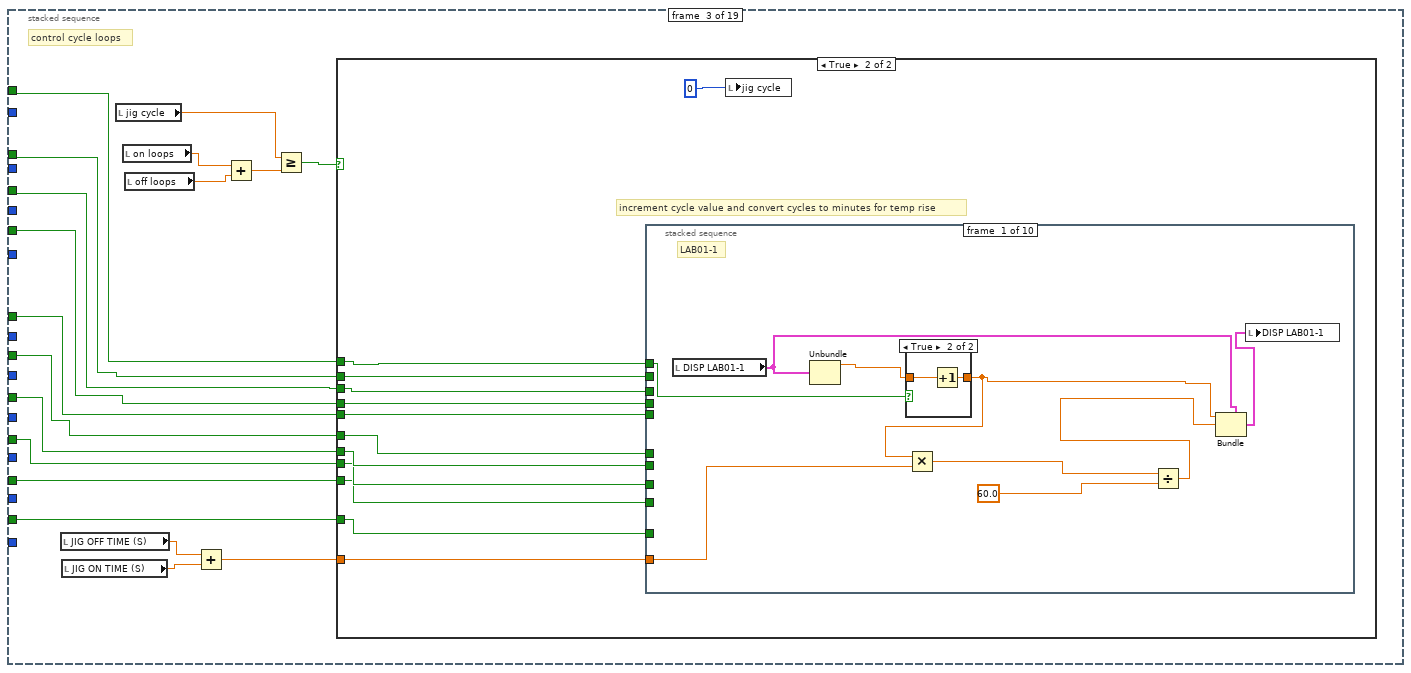
[diagram p15: hidden frame]
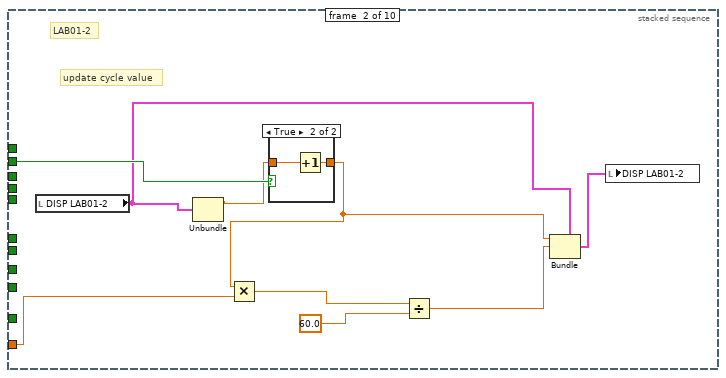
[diagram p18: hidden frame]
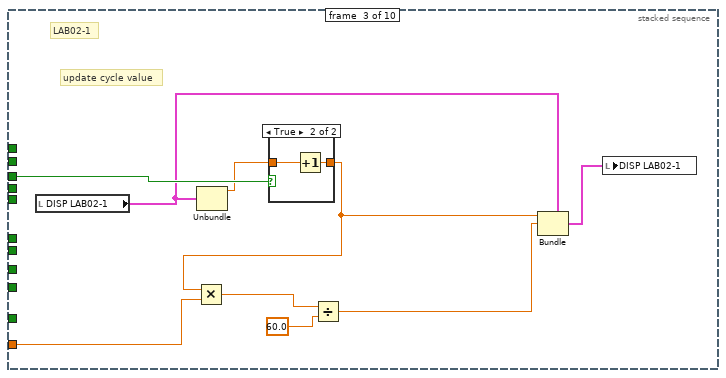
[diagram p20: hidden frame]
diagram:
  n1 = stacked-sequence {
    frame #0 {
      n2 = local write "loop  delay(mS)"(500) -> ()
      n3 = local write "stop2"(FALSE) -> ()
      "jig cycle" <- 0
    }
    frame #1 {
      # "do 1st time set up"
      n4 = stacked-sequence {
        frame #0 {
          # "disable front panel while 1st time set up is being done"
          n5 = property on="Tab Control 2" class="TabCtl (strict)"("DisabledEnum"=T13."Disabled and Grayed Out" ("Disabled")) -> ()  [unwired: 2 in, 2 out]
        }
        frame #1 {
          # "get calibration values"
          n6 = call "sub vi - get calibration values v1.vi"() -> ("LAB01 (CAL)"=→"CAL LAB01":T7, "LAB02 (CAL)"=→"CAL LAB02":T8, "LAB03 (CAL)"=→"CAL LAB03":T7, "LAB04 (CAL)"=→"CAL LAB04":T7, "calibration file error out"=→"calibration file error out":errorcluster, "LAB05 (CAL)"=→"CAL LAB05":T7)  [unwired: 10 in]
        }
        frame #2 {
          # "get last saved test settings from file"
          n7 = local read "Network Directory"() -> (w17:path)
          n8 = local read "C drive data root dir"() -> (w15:path)
          n9 = local read "SET LAB05-2"() -> (w47:T5)
          n10 = local read "SET LAB05-1"() -> (w48:T5)
          n11 = local read "SAMPLES"() -> (w13:dbl)
          n12 = local read "SET LAB04-2"() -> (w49:T5)
          n13 = local read "RATE (Hz)"() -> (w14:dbl)
          n14 = local read "SET LAB03-2"() -> (w46:T5)
          n15 = local read "SET LAB04-1"() -> (w50:T5)
          n16 = local read "SET LAB03-1"() -> (w45:T5)
          n17 = local read "SET LAB02-2"() -> (w44:T5)
          n18 = local read "SET LAB02-1"() -> (w43:T5)
          n19 = local read "SET LAB01-2"() -> (w42:T5)
          n20 = local read "SET LAB01-1"() -> (w41:T5)
          n21 = Bundle("SET LAB01-1"=w41, "SET LAB01-2"=w42, "SET LAB02-1"=w43, "SET LAB02-2"=w44, "SET LAB03-1"=w45, "SET LAB03-2"=w46, "SET LAB04-1"=w50, "SET LAB04-2"=w49, "SET LAB05-1"=w48, "SET LAB05-2"=w47, "Network Directory"=w17, "C drive data root dir"=w15, "RATE (Hz)"=w14, "SAMPLES"=w13) -> (w34:T19)  [unwired: 1 in]
          n22 = String To Path(string="c:\\crabtree\\Set Up\\") -> (path=w38:path)
          n23 = Build Path(base path=w38, name or relative path="settings.bin") -> (appended path=w36:path)
          n24 = Create Folder(path (use dialog)=w38) -> (error out=w40:errorcluster)  [unwired: 2 in, 2 out]
          n25 = call <vilib>:"Clear Errors.vi"("error in (no error)"=w40) -> ()  [unwired: 6 in, 1 out]
          n26 = Open/Create/Replace File(file path (use dialog)=w36) -> (refnum out=w33:refnum<file>, error out=w35:errorcluster)  [unwired: 5 in, 1 out]
          n27 = Read from Binary File(5:w34, 8:w35, 11:w33) -> (0:w30:errorcluster, 2:w32:T19, 3:w31:refnum<file>)  [unwired: 3 in, 1 out]
          n28 = Unbundle(w32) -> ("SET LAB01-1"=w28:T5, "SET LAB01-2"=w27:T5, "SET LAB02-1"=w26:T5, "SET LAB02-2"=w25:T5, "SET LAB03-1"=w24:T5, "SET LAB03-2"=w23:T5, "SET LAB04-1"=w22:T5, "SET LAB04-2"=w21:T5, "SET LAB05-1"=w20:T5, "SET LAB05-2"=w19:T5, "Network Directory"=w18:path, "C drive data root dir"=w16:path, "RATE (Hz)"=w11:dbl, "SAMPLES"=w12:dbl)
          n29 = local write "RATE (Hz)"(w11) -> ()
          n30 = local write "SAMPLES"(w12) -> ()
          n31 = Close File(refnum=w31, error in=w30) -> (error out=w29:errorcluster)  [unwired: 1 out]
          n32 = local write "data file error"(w29) -> ()
          n33 = local write "C drive data root dir"(w16) -> ()
          n34 = local write "Network Directory"(w18) -> ()
          n35 = local write "SET LAB04-2"(w21) -> ()
          n36 = local write "SET LAB05-1"(w20) -> ()
          n37 = local write "SET LAB04-1"(w22) -> ()
          n38 = local write "SET LAB05-2"(w19) -> ()
          n39 = local write "SET LAB02-1"(w26) -> ()
          n40 = local write "SET LAB02-2"(w25) -> ()
          n41 = local write "SET LAB03-1"(w24) -> ()
          n42 = local write "SET LAB03-2"(w23) -> ()
          n43 = local write "SET LAB01-1"(w28) -> ()
          n44 = local write "SET LAB01-2"(w27) -> ()
        }
        frame #3 {
          # "get mail settings"
          n45 = local read "Auto Mail Send"() -> (w54:bool)
          n46 = local read "MAIL SETTINGS"() -> (w58:T6)
          n47 = String To Path(string="c:\\crabtree\\Set Up\\") -> (path=w66:path)
          n48 = Build Path(base path=w66, name or relative path="mail.bin") -> (appended path=w64:path)
          n49 = Create Folder(path (use dialog)=w66) -> (error out=w68:errorcluster)  [unwired: 2 in, 2 out]
          n50 = Bundle("MAIL SETTINGS"=w58, "Auto Mail Send"=w54, "") -> (w57:T20)  [unwired: 1 in]
          n51 = call <vilib>:"Clear Errors.vi"("error in (no error)"=w68) -> ()  [unwired: 6 in, 1 out]
          n52 = Open/Create/Replace File(file path (use dialog)=w64) -> (refnum out=w62:refnum<file>, error out=w63:errorcluster)  [unwired: 5 in, 1 out]
          n53 = Read from Binary File(5:w57, 8:w63, 11:w62) -> (0:w60:errorcluster, 2:w56:T20, 3:w61:refnum<file>)  [unwired: 3 in, 1 out]
          n54 = Unbundle(w56) -> ("MAIL SETTINGS"=w55:T6, "Auto Mail Send"=w53:bool, w52:string)
          n55 = local write "TO (string):"(w52) -> ()
          n56 = local write "Auto Mail Send"(w53) -> ()
          n57 = local write "MAIL SETTINGS"(w55) -> ()
          n58 = Close File(refnum=w61, error in=w60) -> (error out=w59:errorcluster)  [unwired: 1 out]
          n59 = local write "data file error"(w59) -> ()
        }
        frame #4 {
          # "set display status if blank"
          n60 = local read "DISP LAB03-2"() -> (w98:T4)
          n61 = local read "DISP LAB03-1"() -> (w105:T4)
          n62 = local read "DISP LAB02-2"() -> (w112:T4)
          n63 = local read "DISP LAB01-2"() -> (w125:T4)
          n64 = local read "DISP LAB01-1"() -> (w134:T4)
          n65 = local read "DISP LAB02-1"() -> (w119:T4)
          n66 = Unbundle(w98) -> ("STATUS"=w100:string)  [unwired: 2 out]
          n67 = Unbundle(w105) -> ("STATUS"=w107:string)  [unwired: 2 out]
          n68 = Unbundle(w112) -> ("STATUS"=w114:string)  [unwired: 2 out]
          n69 = Unbundle(w119) -> ("STATUS"=w121:string)  [unwired: 2 out]
          n70 = Unbundle(w125) -> ("STATUS"=w128:string)  [unwired: 2 out]
          n71 = Unbundle(w134) -> ("STATUS"=w135:string)  [unwired: 2 out]
          n72 = Equal?(x="", y=w100) -> (x = y?=w102:bool)
          n73 = Equal?(x="", y=w107) -> (x = y?=w109:bool)
          n74 = Equal?(x="", y=w114) -> (x = y?=w116:bool)
          n75 = Equal?(x="", y=w121) -> (x = y?=w123:bool)
          n76 = Equal?(x="", y=w128) -> (x = y?=w130:bool)
          n77 = Equal?(x="", y=w135) -> (x = y?=w137:bool)
          n78 = Select(t="STOP", s=w102, f=w100) -> (s? t:f=w99:string)
          n79 = Select(t="STOP", s=w109, f=w107) -> (s? t:f=w106:string)
          n80 = Select(t="STOP", s=w116, f=w114) -> (s? t:f=w113:string)
          n81 = Select(t="STOP", s=w123, f=w121) -> (s? t:f=w120:string)
          n82 = Select(t="STOP", s=w130, f=w128) -> (s? t:f=w127:string)
          n83 = Select(t="STOP", s=w137, f=w135) -> (s? t:f=w133:string)
          n84 = Bundle(cluster=w98, "STATUS"=w99) -> (w97:T4)  [unwired: 2 in]
          n85 = Bundle(cluster=w105, "STATUS"=w106) -> (w104:T4)  [unwired: 2 in]
          n86 = Bundle(cluster=w112, "STATUS"=w113) -> (w111:T4)  [unwired: 2 in]
          n87 = Bundle(cluster=w119, "STATUS"=w120) -> (w118:T4)  [unwired: 2 in]
          n88 = Bundle(cluster=w125, "STATUS"=w127) -> (w126:T4)  [unwired: 2 in]
          n89 = Bundle(cluster=w134, "STATUS"=w133) -> (w132:T4)  [unwired: 2 in]
          n90 = local write "DISP LAB01-2"(w126) -> ()
          n91 = local write "DISP LAB01-1"(w132) -> ()
          n92 = local write "DISP LAB02-1"(w118) -> ()
          n93 = local write "DISP LAB03-1"(w104) -> ()
          n94 = local write "DISP LAB02-2"(w111) -> ()
          n95 = local write "DISP LAB03-2"(w97) -> ()
          n96 = local read "DISP LAB05-2"() -> (w70:T4)
          n97 = local read "DISP LAB05-1"() -> (w77:T4)
          n98 = local read "DISP LAB04-2"() -> (w79:T4)
          n99 = local read "DISP LAB04-1"() -> (w81:T4)
          n100 = Unbundle(w70) -> ("STATUS"=w72:string)  [unwired: 2 out]
          n101 = Unbundle(w77) -> ("STATUS"=w83:string)  [unwired: 2 out]
          n102 = Unbundle(w79) -> ("STATUS"=w88:string)  [unwired: 2 out]
          n103 = Unbundle(w81) -> ("STATUS"=w93:string)  [unwired: 2 out]
          n104 = Equal?(x="", y=w72) -> (x = y?=w74:bool)
          n105 = Equal?(x="", y=w83) -> (x = y?=w85:bool)
          n106 = Equal?(x="", y=w88) -> (x = y?=w90:bool)
          n107 = Equal?(x="", y=w93) -> (x = y?=w95:bool)
          n108 = Select(t="STOP", s=w74, f=w72) -> (s? t:f=w71:string)
          n109 = Select(t="STOP", s=w85, f=w83) -> (s? t:f=w82:string)
          n110 = Select(t="STOP", s=w90, f=w88) -> (s? t:f=w87:string)
          n111 = Select(t="STOP", s=w95, f=w93) -> (s? t:f=w92:string)
          n112 = Bundle(cluster=w70, "STATUS"=w71) -> (w69:T4)  [unwired: 2 in]
          n113 = Bundle(cluster=w77, "STATUS"=w82) -> (w76:T4)  [unwired: 2 in]
          n114 = Bundle(cluster=w79, "STATUS"=w87) -> (w78:T4)  [unwired: 2 in]
          n115 = Bundle(cluster=w81, "STATUS"=w92) -> (w80:T4)  [unwired: 2 in]
          n116 = local write "DISP LAB05-2"(w69) -> ()
          n117 = local write "DISP LAB05-1"(w76) -> ()
          n118 = local write "DISP LAB04-1"(w80) -> ()
          n119 = local write "DISP LAB04-2"(w78) -> ()
        }
        frame #5 {
          # "initialise analog input express vi's"
          n120 = for {
            N: 2.0 -> [_]
            n121 = call "sub vi - analog 1st setup v1.vi"() -> ()  [unwired: 11 in, 5 out]
          }
        }
        frame #6 {
          # "enable front panel, all settings done"
          n122 = property on="Tab Control 2" class="TabCtl (strict)"("DisabledEnum"=T13."Enabled" ("Disabled")) -> ()  [unwired: 2 in, 2 out]
        }
      }
    }
    frame #2 {
      n123 = node-c288("loop  delay(mS)") -> (w143:T14)  [unwired: 3 in]
      n124 = timed-loop {
        timing: w143 -> [_]
        timing-out: [_] -> w142
        i -> [w165]
        stop <- "stop" stop-if-true
        n125 = node-c288() -> ()  [unwired: 1 in, 1 out]
        n126 = local read "SELECT LAB05-2"() -> (w145:T3)
        n127 = local read "SELECT LAB05-1"() -> (w146:T3)
        n128 = local read "SELECT LAB04-2"() -> (w147:T3)
        n129 = local read "SELECT LAB03-1"() -> (w150:T3)
        n130 = local read "SELECT LAB02-2"() -> (w151:T3)
        n131 = local read "SELECT LAB01-1"() -> (w154:T3)
        n132 = local read "SELECT LAB03-2"() -> (w149:T3)
        n133 = local read "SELECT LAB01-2"() -> (w153:T3)
        n134 = local read "SELECT LAB04-1"() -> (w148:T3)
        n135 = local read "SELECT LAB02-1"() -> (w152:T3)
        n136 = local read "run lab03-2"() -> (w159:bool)
        n137 = local read "run lab04-1"() -> (w158:bool)
        n138 = local read "run lab05-1"() -> (w156:bool)
        n139 = local read "run lab04-2"() -> (w157:bool)
        n140 = local read "run lab05-2"() -> (w155:bool)
        n141 = local read "run lab03-1"() -> (w160:bool)
        n142 = local read "run lab02-2"() -> (w161:bool)
        n143 = local read "run lab02-1"() -> (w162:bool)
        n144 = local read "run lab01-1"() -> (w164:bool)
        n145 = local read "run lab01-2"() -> (w163:bool)
        n146 = stacked-sequence {
          seq-local: [_ w227 _ _ _ _ _ _ _ _ _ _ _ _ _ _ _ _ _] -> [_ _ _ _ _ w1762 _ _ _ _ _ _ _ _ _ _ _ _ _]
          seq-local: [_ w226 _ _ _ _ _ _ _ _ _ _ _ _ _ _ _ _ _] -> [_ _ _ _ _ w1761 _ _ _ _ _ _ _ _ _ _ _ _ _]
          seq-local: [_ w213 _ _ _ _ _ _ _ _ _ _ _ _ _ _ _ _ _] -> [_ _ _ _ _ w1760 _ _ _ _ _ _ _ _ _ _ _ _ _]
          seq-local: [_ w212 _ _ _ _ _ _ _ _ _ _ _ _ _ _ _ _ _] -> [_ _ _ _ _ w1759 _ _ _ _ _ _ _ _ _ _ _ _ _]
          seq-local: [_ w211 _ _ _ _ _ _ _ _ _ _ _ _ _ _ _ _ _] -> [_ _ _ _ _ w1758 _ _ _ _ _ _ _ _ _ _ _ _ _]
          seq-local: [_ w210 _ _ _ _ _ _ _ _ _ _ _ _ _ _ _ _ _] -> [_ _ _ _ _ w1757 _ _ _ _ _ _ _ _ _ _ _ _ _]
          seq-local: [_ w209 _ _ _ _ _ _ _ _ _ _ _ _ _ _ _ _ _] -> [_ _ _ _ _ w1756 _ _ _ _ _ _ _ _ _ _ _ _ _]
          seq-local: [_ w208 _ _ _ _ _ _ _ _ _ _ _ _ _ _ _ _ _] -> [_ _ _ _ _ w1755 _ _ _ _ _ _ _ _ _ _ _ _ _]
          seq-local: [_ w207 _ _ _ _ _ _ _ _ _ _ _ _ _ _ _ _ _] -> [_ _ _ _ _ w1754 _ _ _ _ _ _ _ _ _ _ _ _ _]
          seq-local: [_ w206 _ _ _ _ _ _ _ _ _ _ _ _ _ _ _ _ _] -> [_ _ _ _ _ w1753 _ _ _ _ _ _ _ _ _ _ _ _ _]
          tunnel: w164 -> [_ _ w243 w408 w1352 w1782 w2092 w2337 _ _ _ _ _ w2812 _ w3739 _ _ w4016]
          tunnel: w163 -> [_ _ w242 w406 w1351 w1781 w2093 w2336 _ _ _ _ _ w2811 _ w3737 _ _ w4015]
          tunnel: w162 -> [_ _ w241 w404 w1350 w1780 w2091 w2335 _ _ _ _ _ w2810 _ w3735 _ _ w4014]
          tunnel: w161 -> [_ _ w240 w402 w1349 w1779 w2090 w2334 _ _ _ _ _ w2809 _ w3733 _ _ w4013]
          tunnel: w160 -> [_ _ w239 w400 w1348 w1778 w2089 w2333 _ _ _ _ _ w2808 _ w3731 _ _ w4012]
          tunnel: w159 -> [_ _ w238 w398 w1347 w1777 w2088 w2332 _ _ _ _ _ w2807 _ w3729 _ _ w4011]
          tunnel: w158 -> [_ _ w237 w396 w1346 w1776 w2087 w2331 _ _ _ _ _ w2806 _ w3727 _ _ w4010]
          tunnel: w157 -> [_ _ w236 w394 w1345 w1775 w2086 w2330 _ _ _ _ _ w2805 _ w3725 _ _ w4009]
          tunnel: w156 -> [_ _ w235 w392 w1344 w1774 w2085 w2329 _ _ _ _ _ w2804 _ w3723 _ _ w4008]
          tunnel: w155 -> [_ _ w234 w390 w1343 w1773 w2084 w2328 _ _ _ _ _ w2803 _ w3721 _ _ w4007]
          tunnel: w154 -> [_ _ _ w407 w1342 w1772 _ _ _ _ _ _ _ _ _ w3741 _ _ _]
          tunnel: w153 -> [_ _ _ w405 w1341 w1771 _ _ _ _ _ _ _ _ _ w3736 _ _ _]
          tunnel: w152 -> [_ _ _ w403 w1340 w1770 _ _ _ _ _ _ _ _ _ w3734 _ _ _]
          tunnel: w151 -> [_ _ _ w401 w1339 w1769 _ _ _ _ _ _ _ _ _ w3732 _ _ _]
          tunnel: w150 -> [_ _ _ w399 w1338 w1768 _ _ _ _ _ _ _ _ _ w3730 _ _ _]
          tunnel: w149 -> [_ _ _ w397 w1337 w1767 _ _ _ _ _ _ _ _ _ w3728 _ _ _]
          tunnel: w148 -> [_ _ _ w395 w1336 w1766 _ _ _ _ _ _ _ _ _ w3726 _ _ _]
          tunnel: w147 -> [_ _ _ w393 w1335 w1765 _ _ _ _ _ _ _ _ _ w3724 _ _ _]
          tunnel: w146 -> [_ _ _ w391 w1334 w1764 _ _ _ _ _ _ _ _ _ w3722 _ _ _]
          tunnel: w145 -> [_ _ _ w389 w1333 w1763 _ _ _ _ _ _ _ _ _ w3720 _ _ _]
          frame #0 {
            w169 = FALSE
            w174 = 0.5
            # "set up cycle control"
            n147 = local read "jig cycle"() -> (w173:dbl)
            n148 = Divide(x="JIG ON TIME (S)", y=w174) -> (x/y=→"on loops":dbl)
            n149 = Divide(x="JIG OFF TIME (S)", y=w174) -> (x/y=→"off loops":dbl)
            n150 = Increment(x=w173) -> (x+1=w172:dbl)
            n151 = local write "TEMP update"(w169) -> ()
            n152 = local write "AI update"(w169) -> ()
            n153 = local write "jig cycle"(w172) -> ()
            n154 = event shown="[1] \"ADMIN PAGE\": Value Change" {
              selector: _ -> [_ _]
              dyn-events: _ -> [_ _]
              timeout: 10 -> [_ _]
              event Timeout {
                n155 = event-data() -> ()  [unwired: 1 in, 3 out]
              }
              event "ADMIN PAGE": Value Change {
                n156 = event-data() -> ()  [unwired: 1 in, 6 out]
                n157 = stacked-sequence {
                  seq-local: [_ w178 _] -> [_ _ w179]
                  frame #0 {
                    n158 = global write "Global 1.vi" "password"("9999") -> ()
                  }
                  frame #1 {
                    n159 = call "sub vi - password 1.vi"() -> ("RESULT"=w178:bool)  [unwired: 11 in]
                  }
                  frame #2 {
                    w181 = FALSE
                    n160 = property on="Tab Control 2" class="TabCtl (strict)"() -> ("Pages"=w185:refnum<vi>[])  [unwired: 2 in, 2 out]
                    n161 = Select(t=TRUE, s=w179, f=w181) -> (s? t:f=w180:bool)
                    n162 = Index Array(array=w185, index=6) -> (element=w183:refnum<vi>)
                    n163 = property class="Page"(reference=w183, "PageVis"=w180) -> ()  [unwired: 1 in, 2 out]
                    n164 = local write "ADMIN PAGE"(w181) -> ()
                  }
                }
              }
            }
          }
          frame #1 {
            w223 = 60.0
            # "convert temperature rise minutes to cycles"
            n165 = local read "SET LAB05-2"() -> (w187:T5)
            n166 = local read "SET LAB05-1"() -> (w189:T5)
            n167 = local read "SET LAB04-2"() -> (w191:T5)
            n168 = local read "SET LAB01-1"() -> (w205:T5)
            n169 = local read "SET LAB01-2"() -> (w203:T5)
            n170 = local read "SET LAB02-2"() -> (w199:T5)
            n171 = local read "SET LAB04-1"() -> (w193:T5)
            n172 = local read "SET LAB03-1"() -> (w197:T5)
            n173 = local read "SET LAB03-2"() -> (w195:T5)
            n174 = local read "SET LAB02-1"() -> (w201:T5)
            n175 = local read "JIG OFF TIME (S)"() -> (w228:dbl)
            n176 = local read "JIG ON TIME (S)"() -> (w229:dbl)
            n177 = Unbundle(w187) -> ("T-RISE mins"=w186:dbl)  [unwired: 4 out]
            n178 = Unbundle(w189) -> ("T-RISE mins"=w188:dbl)  [unwired: 4 out]
            n179 = Unbundle(w205) -> ("T-RISE mins"=w204:dbl)  [unwired: 4 out]
            n180 = Unbundle(w191) -> ("T-RISE mins"=w190:dbl)  [unwired: 4 out]
            n181 = Unbundle(w203) -> ("T-RISE mins"=w202:dbl)  [unwired: 4 out]
            n182 = Unbundle(w201) -> ("T-RISE mins"=w200:dbl)  [unwired: 4 out]
            n183 = Unbundle(w193) -> ("T-RISE mins"=w192:dbl)  [unwired: 4 out]
            n184 = Unbundle(w199) -> ("T-RISE mins"=w198:dbl)  [unwired: 4 out]
            n185 = Unbundle(w195) -> ("T-RISE mins"=w194:dbl)  [unwired: 4 out]
            n186 = Unbundle(w197) -> ("T-RISE mins"=w196:dbl)  [unwired: 4 out]
            n187 = Add(x=w229, y=w228) -> (x+y=w222:dbl)
            n188 = Multiply(x=w223, y=w194) -> (x*y=w218:dbl)
            n189 = Multiply(x=w223, y=w192) -> (x*y=w217:dbl)
            n190 = Multiply(x=w223, y=w190) -> (x*y=w216:dbl)
            n191 = Multiply(x=w223, y=w188) -> (x*y=w215:dbl)
            n192 = Multiply(x=w223, y=w186) -> (x*y=w214:dbl)
            n193 = Multiply(x=w223, y=w202) -> (x*y=w224:dbl)
            n194 = Multiply(x=w223, y=w196) -> (x*y=w219:dbl)
            n195 = Multiply(x=w223, y=w204) -> (x*y=w225:dbl)
            n196 = Multiply(x=w223, y=w200) -> (x*y=w221:dbl)
            n197 = Multiply(x=w223, y=w198) -> (x*y=w220:dbl)
            n198 = Divide(x=w215, y=w222) -> (x/y=w207:dbl)
            n199 = Divide(x=w216, y=w222) -> (x/y=w208:dbl)
            n200 = Divide(x=w217, y=w222) -> (x/y=w209:dbl)
            n201 = Divide(x=w214, y=w222) -> (x/y=w206:dbl)
            n202 = Divide(x=w219, y=w222) -> (x/y=w211:dbl)
            n203 = Divide(x=w225, y=w222) -> (x/y=w227:dbl)
            n204 = Divide(x=w224, y=w222) -> (x/y=w226:dbl)
            n205 = Divide(x=w221, y=w222) -> (x/y=w213:dbl)
            n206 = Divide(x=w220, y=w222) -> (x/y=w212:dbl)
            n207 = Divide(x=w218, y=w222) -> (x/y=w210:dbl)
          }
          frame #2 {
            # "control cycle loops"
            n208 = local read "JIG OFF TIME (S)"() -> (w232:dbl)
            n209 = local read "JIG ON TIME (S)"() -> (w231:dbl)
            n210 = local read "jig cycle"() -> (w245:dbl)
            n211 = local read "on loops"() -> (w247:dbl)
            n212 = local read "off loops"() -> (w246:dbl)
            n213 = Add(x=w232, y=w231) -> (x+y=w230:dbl)
            n214 = Add(x=w247, y=w246) -> (x+y=w233:dbl)
            n215 = Greater Or Equal?(x=w245, y=w233) -> (x >= y?=w244:bool)
            n216 = case shown="True" w244 {
              tunnel: w243 -> [_ w258]
              tunnel: w242 -> [_ w257]
              tunnel: w241 -> [_ w256]
              tunnel: w240 -> [_ w255]
              tunnel: w239 -> [_ w254]
              tunnel: w238 -> [_ w253]
              tunnel: w237 -> [_ w252]
              tunnel: w236 -> [_ w251]
              tunnel: w235 -> [_ w250]
              tunnel: w234 -> [_ w249]
              tunnel: w230 -> [_ w248]
              frame False {
              }
              frame True {
                # "increment cycle value and convert cycles to minutes for temp rise"
                n217 = stacked-sequence {
                  tunnel: w258 -> [w268 _ _ _ _ _ _ _ _ _]
                  tunnel: w257 -> [_ w280 _ _ _ _ _ _ _ _]
                  tunnel: w256 -> [_ _ w292 _ _ _ _ _ _ _]
                  tunnel: w255 -> [_ _ _ w304 _ _ _ _ _ _]
                  tunnel: w254 -> [_ _ _ _ w316 _ _ _ _ _]
                  tunnel: w253 -> [_ _ _ _ _ w328 _ _ _ _]
                  tunnel: w252 -> [_ _ _ _ _ _ w340 _ _ _]
                  tunnel: w251 -> [_ _ _ _ _ _ _ w352 _ _]
                  tunnel: w250 -> [_ _ _ _ _ _ _ _ w364 _]
                  tunnel: w249 -> [_ _ _ _ _ _ _ _ _ w376]
                  tunnel: w248 -> [w265 w277 w289 w301 w313 w325 w337 w349 w361 w373]
                  frame #0 {
                    # "LAB01-1"
                    n218 = local read "DISP LAB01-1"() -> (w263:T4)
                    n219 = Unbundle(w263) -> ("CYCLE"=w264:dbl)  [unwired: 2 out]
                    n220 = case shown="True" w268 {
                      tunnel: w264 -> [w269 w271]
                      tunnel: [w269 w270] -> w262
                      frame False {
                      }
                      frame True {
                        n221 = Increment(x=w271) -> (x+1=w270:dbl)
                      }
                    }
                    n222 = Multiply(x=w262, y=w265) -> (x*y=w266:dbl)
                    n223 = Divide(x=w266, y=60.0) -> (x/y=w261:dbl)
                    n224 = Bundle(cluster=w263, "CYCLE"=w262, "MINS"=w261) -> (w260:T4)  [unwired: 1 in]
                    n225 = local write "DISP LAB01-1"(w260) -> ()
                  }
                  frame #1 {
                    # "update cycle value"
                    # "LAB01-2"
                    n226 = local read "DISP LAB01-2"() -> (w275:T4)
                    n227 = Unbundle(w275) -> ("CYCLE"=w276:dbl)  [unwired: 2 out]
                    n228 = case shown="True" w280 {
                      tunnel: w276 -> [w281 w283]
                      tunnel: [w281 w282] -> w273
                      frame False {
                      }
                      frame True {
                        n229 = Increment(x=w283) -> (x+1=w282:dbl)
                      }
                    }
                    n230 = Multiply(x=w273, y=w277) -> (x*y=w278:dbl)
                    n231 = Divide(x=w278, y=60.0) -> (x/y=w272:dbl)
                    n232 = Bundle(cluster=w275, "CYCLE"=w273, "MINS"=w272) -> (w274:T4)  [unwired: 1 in]
                    n233 = local write "DISP LAB01-2"(w274) -> ()
                  }
                  frame #2 {
                    # "update cycle value"
                    # "LAB02-1"
                    n234 = local read "DISP LAB02-1"() -> (w287:T4)
                    n235 = Unbundle(w287) -> ("CYCLE"=w288:dbl)  [unwired: 2 out]
                    n236 = case shown="True" w292 {
                      tunnel: [w293 w295] -> w285
                      tunnel: w288 -> [w293 w294]
                      frame False {
                      }
                      frame True {
                        n237 = Increment(x=w294) -> (x+1=w295:dbl)
                      }
                    }
                    n238 = Multiply(x=w285, y=w289) -> (x*y=w290:dbl)
                    n239 = Divide(x=w290, y=60.0) -> (x/y=w284:dbl)
                    n240 = Bundle(cluster=w287, "CYCLE"=w285, "MINS"=w284) -> (w286:T4)  [unwired: 1 in]
                    n241 = local write "DISP LAB02-1"(w286) -> ()
                  }
                  frame #3 {
                    # "update cycle value"
                    # "LAB02-2"
                    n242 = local read "DISP LAB02-2"() -> (w299:T4)
                    n243 = Unbundle(w299) -> ("CYCLE"=w300:dbl)  [unwired: 2 out]
                    n244 = case shown="True" w304 {
                      tunnel: [w305 w307] -> w298
                      tunnel: w300 -> [w305 w306]
                      frame False {
                      }
                      frame True {
                        n245 = Increment(x=w306) -> (x+1=w307:dbl)
                      }
                    }
                    n246 = Multiply(x=w298, y=w301) -> (x*y=w302:dbl)
                    n247 = Divide(x=w302, y=60.0) -> (x/y=w297:dbl)
                    n248 = Bundle(cluster=w299, "CYCLE"=w298, "MINS"=w297) -> (w296:T4)  [unwired: 1 in]
                    n249 = local write "DISP LAB02-2"(w296) -> ()
                  }
                  frame #4 {
                    # "update cycle value"
                    # "LAB03-1"
                    n250 = local read "DISP LAB03-1"() -> (w311:T4)
                    n251 = Unbundle(w311) -> ("CYCLE"=w312:dbl)  [unwired: 2 out]
                    n252 = case shown="True" w316 {
                      tunnel: [w317 w319] -> w308
                      tunnel: w312 -> [w317 w318]
                      frame False {
                      }
                      frame True {
                        n253 = Increment(x=w318) -> (x+1=w319:dbl)
                      }
                    }
                    n254 = Multiply(x=w308, y=w313) -> (x*y=w314:dbl)
                    n255 = Divide(x=w314, y=60.0) -> (x/y=w309:dbl)
                    n256 = Bundle(cluster=w311, "CYCLE"=w308, "MINS"=w309) -> (w310:T4)  [unwired: 1 in]
                    n257 = local write "DISP LAB03-1"(w310) -> ()
                  }
                  frame #5 {
                    # "update cycle value"
                    # "LAB03-2"
                    n258 = local read "DISP LAB03-2"() -> (w323:T4)
                    n259 = Unbundle(w323) -> ("CYCLE"=w324:dbl)  [unwired: 2 out]
                    n260 = case shown="False" w328 {
                      tunnel: [w329 w331] -> w322
                      tunnel: w324 -> [w329 w330]
                      frame False {
                      }
                      frame True {
                        n261 = Increment(x=w330) -> (x+1=w331:dbl)
                      }
                    }
                    n262 = Multiply(x=w322, y=w325) -> (x*y=w326:dbl)
                    n263 = Divide(x=w326, y=60.0) -> (x/y=w321:dbl)
                    n264 = Bundle(cluster=w323, "CYCLE"=w322, "MINS"=w321) -> (w320:T4)  [unwired: 1 in]
                    n265 = local write "DISP LAB03-2"(w320) -> ()
                  }
                  frame #6 {
                    # "update cycle value"
                    # "LAB04-1"
                    n266 = local read "DISP LAB04-1"() -> (w335:T4)
                    n267 = Unbundle(w335) -> ("CYCLE"=w336:dbl)  [unwired: 2 out]
                    n268 = case shown="True" w340 {
                      tunnel: [w341 w343] -> w333
                      tunnel: w336 -> [w341 w342]
                      frame False {
                      }
                      frame True {
                        n269 = Increment(x=w342) -> (x+1=w343:dbl)
                      }
                    }
                    n270 = Multiply(x=w333, y=w337) -> (x*y=w338:dbl)
                    n271 = Divide(x=w338, y=60.0) -> (x/y=w332:dbl)
                    n272 = Bundle(cluster=w335, "CYCLE"=w333, "MINS"=w332) -> (w334:T4)  [unwired: 1 in]
                    n273 = local write "DISP LAB04-1"(w334) -> ()
                  }
                  frame #7 {
                    # "update cycle value"
                    # "LAB04-2"
                    n274 = local read "DISP LAB04-2"() -> (w347:T4)
                    n275 = Unbundle(w347) -> ("CYCLE"=w348:dbl)  [unwired: 2 out]
                    n276 = case shown="True" w352 {
                      tunnel: [w353 w355] -> w345
                      tunnel: w348 -> [w353 w354]
                      frame False {
                      }
                      frame True {
                        n277 = Increment(x=w354) -> (x+1=w355:dbl)
                      }
                    }
                    n278 = Multiply(x=w345, y=w349) -> (x*y=w351:dbl)
                    n279 = Divide(x=w351, y=60.0) -> (x/y=w344:dbl)
                    n280 = Bundle(cluster=w347, "CYCLE"=w345, "MINS"=w344) -> (w346:T4)  [unwired: 1 in]
                    n281 = local write "DISP LAB04-2"(w346) -> ()
                  }
                  frame #8 {
                    # "update cycle value"
                    # "LAB05-1"
                    n282 = local read "DISP LAB05-1"() -> (w359:T4)
                    n283 = Unbundle(w359) -> ("CYCLE"=w360:dbl)  [unwired: 2 out]
                    n284 = case shown="True" w364 {
                      tunnel: [w365 w367] -> w357
                      tunnel: w360 -> [w365 w366]
                      frame False {
                      }
                      frame True {
                        n285 = Increment(x=w366) -> (x+1=w367:dbl)
                      }
                    }
                    n286 = Multiply(x=w357, y=w361) -> (x*y=w362:dbl)
                    n287 = Divide(x=w362, y=60.0) -> (x/y=w356:dbl)
                    n288 = Bundle(cluster=w359, "CYCLE"=w357, "MINS"=w356) -> (w358:T4)  [unwired: 1 in]
                    n289 = local write "DISP LAB05-1"(w358) -> ()
                  }
                  frame #9 {
                    # "update cycle value"
                    # "LAB05-2"
                    n290 = local read "DISP LAB05-2"() -> (w372:T4)
                    n291 = Unbundle(w372) -> ("CYCLE"=w371:dbl)  [unwired: 2 out]
                    n292 = case shown="True" w376 {
                      tunnel: [w377 w379] -> w370
                      tunnel: w371 -> [w377 w378]
                      frame False {
                      }
                      frame True {
                        n293 = Increment(x=w378) -> (x+1=w379:dbl)
                      }
                    }
                    n294 = Multiply(x=w370, y=w373) -> (x*y=w374:dbl)
                    n295 = Divide(x=w374, y=60.0) -> (x/y=w369:dbl)
                    n296 = Bundle(cluster=w372, "CYCLE"=w370, "MINS"=w369) -> (w368:T4)  [unwired: 1 in]
                    n297 = local write "DISP LAB05-2"(w368) -> ()
                  }
                }
                n298 = local write "jig cycle"(0) -> ()
              }
            }
          }
          frame #3 {
            # "START & STOP test RUN switch change, start test if true and stop test if false"
            n299 = Get Date/Time In Seconds() -> (seconds since 1Jan1904=w387:timestamp)
            n300 = local read "C drive data root dir"() -> (w380:path)
            n301 = Format Date/Time String(time format string (%c)="%b\\%a%d", seconds (now)=w387) -> (date/time string=w411:string)  [unwired: 1 in]
            n302 = Format Date/Time String(time format string (%c)="%H%M", seconds (now)=w387) -> (date/time string=w409:string)  [unwired: 1 in]
            n303 = Format Date/Time String(time format string (%c)="LabPanel%Y", seconds (now)=w387) -> (date/time string=w386:string)  [unwired: 1 in]
            n304 = Path To String(path=w380) -> (string=w383:string)
            n305 = global write "Global 1.vi" "C drive root path"(w380) -> ()
            n306 = Concatenate Strings(w383, "\\") -> (w381:string)
            n307 = event shown="[2] \"RUN LAB01-2\": Value Change" {
              selector: _ -> [_ _ _ _ _ _ _ _ _ _ _]
              dyn-events: _ -> [_ _ _ _ _ _ _ _ _ _ _]
              timeout: 10 -> [_ _ _ _ _ _ _ _ _ _ _]
              tunnel: w381 -> [_ w419 w511 w603 w695 w787 w879 w971 w1063 w1155 w1247]
              tunnel: w411 -> [_ w418 w510 w602 w694 w786 w878 w970 w1062 w1154 w1246]
              tunnel: w409 -> [_ w416 w509 w601 w693 w785 w877 w969 w1061 w1153 w1245]
              tunnel: w407 -> [_ w417 _ _ _ _ _ _ _ _ _]
              tunnel: w408 -> [_ _ _ _ _ _ _ _ _ _ _]
              tunnel: w406 -> [_ _ _ _ _ _ _ _ _ _ _]
              tunnel: w405 -> [_ _ w508 _ _ _ _ _ _ _ _]
              tunnel: w404 -> [_ _ _ _ _ _ _ _ _ _ _]
              tunnel: w403 -> [_ _ _ w600 _ _ _ _ _ _ _]
              tunnel: w402 -> [_ _ _ _ _ _ _ _ _ _ _]
              tunnel: w401 -> [_ _ _ _ w692 _ _ _ _ _ _]
              tunnel: w400 -> [_ _ _ _ _ _ _ _ _ _ _]
              tunnel: w399 -> [_ _ _ _ _ w784 _ _ _ _ _]
              tunnel: w398 -> [_ _ _ _ _ _ _ _ _ _ _]
              tunnel: w397 -> [_ _ _ _ _ _ w876 _ _ _ _]
              tunnel: w396 -> [_ _ _ _ _ _ _ _ _ _ _]
              tunnel: w395 -> [_ _ _ _ _ _ _ w968 _ _ _]
              tunnel: w394 -> [_ _ _ _ _ _ _ _ _ _ _]
              tunnel: w393 -> [_ _ _ _ _ _ _ _ w1060 _ _]
              tunnel: w392 -> [_ _ _ _ _ _ _ _ _ _ _]
              tunnel: w391 -> [_ _ _ _ _ _ _ _ _ w1152 _]
              tunnel: w390 -> [_ _ _ _ _ _ _ _ _ _ _]
              tunnel: w389 -> [_ _ _ _ _ _ _ _ _ _ w1244]
              tunnel: w386 -> [_ w415 w507 w599 w691 w783 w875 w967 w1059 w1151 w1243]
              tunnel: [_ w414 w506 w598 w690 w782 w874 w966 w1058 w1150 w1242] -> w384
              event Timeout {
                n308 = event-data() -> ()  [unwired: 1 in, 3 out]
              }
              event "RUN LAB01-1": Value Change {
                n309 = event-data() -> ("NewVal"=w413:bool)  [unwired: 1 in, 5 out]
                n310 = local write "run lab01-1"(w413) -> ()
                n311 = case shown="True" w413 {
                  tunnel: w419 -> [_ w452]
                  tunnel: w418 -> [_ w451]
                  tunnel: w417 -> [w421 w450]
                  tunnel: w416 -> [_ w449]
                  tunnel: w415 -> [_ w448]
                  tunnel: [w420 w447] -> w414
                  frame False {
                    # "stop test"
                    n312 = stacked-sequence {
                      tunnel: w421 -> [_ w433 _ _]
                      tunnel: [_ w425 _ _] -> w420
                      frame #0 {
                        n313 = local read "DISP LAB01-1"() -> (w424:T4)
                        n314 = Bundle(cluster=w424, "STATUS"="STOP") -> (w422:T4)  [unwired: 2 in]
                        n315 = local write "DISP LAB01-1"(w422) -> ()
                      }
                      frame #1 {
                        n316 = local read "DISP LAB01-1"() -> (w432:T4)
                        n317 = Unbundle(w432) -> ("CYCLE"=w430:dbl, "MINS"=w431:dbl)  [unwired: 1 out]
                        n318 = case shown="\"CYCLE TEST\"" w433 {
                          tunnel: w431 -> [_ _ w440]
                          tunnel: w430 -> [w438 w439 _]
                          tunnel: [w438 w439 w440] -> w429
                          frame "CHART TEST", Default {
                          }
                          frame "CYCLE TEST" {
                          }
                          frame "T-RISE TEST" {
                          }
                        }
                        n319 = local read "TDMS LAB01-1"() -> (w437:refnum<k34>)
                        n320 = Build Array("STOPPED") -> (w434:string[])
                        n321 = Build Array(w429) -> (w428:dbl[])
                        n322 = TDMS Write(0:w437, 5:"TEST RESULT", 7:w434, 9:w428) -> (4:w426:refnum<k34>, 15:w427:errorcluster)  [unwired: 2 in, 2 out]
                        n323 = TDMS Close(8:w427, 11:w426) -> (0:w425:errorcluster)  [unwired: 1 out]
                      }
                      frame #2 {
                        n324 = stacked-sequence {
                          tunnel: "LAB01-1" -> [w443 w445]
                          frame #0 {
                            n325 = call "sub vi - defrag tdms v1.vi"("panel id"=w443) -> ("error out"=w442:errorcluster)  [unwired: 10 in]
                            n326 = local write "data file error"(w442) -> ()
                          }
                          frame #1 {
                            n327 = call "Save data file to network drive v1.vi"("panel id"=w445) -> ("network file save error"=w444:errorcluster)  [unwired: 9 in, 1 out]
                            n328 = local write "RESULT LAB01-1"(FALSE) -> ()
                            n329 = local write "data file error"(w444) -> ()
                          }
                        }
                      }
                      frame #3 {
                      }
                    }
                  }
                  frame True {
                    # "start new test and create test file"
                    n330 = stacked-sequence {
                      seq-local: [w453 _ _ _ _] -> [_ w474 _ _ _]
                      tunnel: w452 -> [w458 _ _ _ _]
                      tunnel: w451 -> [w454 _ _ _ _]
                      tunnel: w450 -> [w468 _ _ _ _]
                      tunnel: w449 -> [w461 _ _ _ _]
                      tunnel: w448 -> [w456 _ _ _ _]
                      tunnel: [_ w475 _ _ _] -> w447
                      frame #0 {
                        w455 = "\\"
                        n331 = case shown="\"CHART TEST\", Default" w468 {
                          tunnel: ["L01-1-CHART TEST-" "L01-1-CYCLE TEST-" "L01-1-T-RISE TEST-"] -> w464
                          frame "CHART TEST", Default {
                          }
                          frame "CYCLE TEST" {
                          }
                          frame "T-RISE TEST" {
                          }
                        }
                        n332 = local read "SET LAB01-1"() -> (w463:T5)
                        n333 = Unbundle(w463) -> ("DESCRIPTION"=w462:string)  [unwired: 4 out]
                        n334 = Concatenate Strings(w458, "\\", w456, w455, w454, w455) -> (w465:string)
                        n335 = String To Path(string=w465) -> (path=w467:path)
                        n336 = Concatenate Strings(w465, w464, w462, "-", w461, ".tdms") -> (w453:string)
                        n337 = Create Folder(path (use dialog)=w467) -> (error out=w466:errorcluster)  [unwired: 2 in, 2 out]
                        n338 = call <vilib>:"Clear Errors.vi"("error in (no error)"=w466) -> ()  [unwired: 6 in, 1 out]
                        n339 = global write "Global 1.vi" "LAB01-1 FILE"(w453) -> ()
                      }
                      frame #1 {
                        n340 = String To Path(string=w474) -> (path=w472:path)
                        n341 = TDMS Open(5:FALSE, 6:FALSE, 10:T17."create or replace" ("operation (0:open)"), 11:w472) -> (0:w475:errorcluster, 3:→"TDMS LAB01-1":refnum<k34>)  [unwired: 3 in]
                      }
                      frame #2 {
                        n342 = local read "TDMS LAB01-1"() -> (w495:refnum<k34>)
                        n343 = local read "SET LAB01-1"() -> (w484:T5)
                        n344 = Build Array("Testers Name", "Description", "Set Test Cycles", "T-Rise minutes", "T-Rise Deg C") -> (w485:string[])
                        n345 = Unbundle(w484) -> ("NAME"=w483:string, "DESCRIPTION"=w482:string, "CYCLES"=w481:dbl, "T-RISE mins"=w480:dbl, "T-RISE deg C"=w479:dbl)
                        n346 = Number To Decimal String(number=w481) -> (decimal integer string=w494:string)  [unwired: 1 in]
                        n347 = Number To Decimal String(number=w480) -> (decimal integer string=w493:string)  [unwired: 1 in]
                        n348 = Number To Decimal String(number=w479) -> (decimal integer string=w492:string)  [unwired: 1 in]
                        n349 = Build Array(w483, w482, w494, w493, w492) -> (w491:string[])
                        n350 = TDMS Set Properties(5:w491, 7:w485, 11:w495) -> ()  [unwired: 3 in, 4 out]
                      }
                      frame #3 {
                        w496 = 0.0
                        n351 = local read "DISP LAB01-1"() -> (w499:T4)
                        n352 = Bundle(cluster=w499, "CYCLE"=w496, "MINS"=w496, "STATUS"="RUN") -> (w498:T4)
                        n353 = local write "DISP LAB01-1"(w498) -> ()
                      }
                      frame #4 {
                        n354 = local read "SIG LAB01-1"() -> (w502:T2)
                        n355 = local read "TEMP START LAB01-1"() -> (w504:cluster{"TL":dbl, "TN":dbl})
                        n356 = Unbundle(w502) -> ("Tmp Live"=w501:dbl, "Tmp Neut"=w500:dbl)  [unwired: 3 out]
                        n357 = Bundle(cluster=w504, "TL"=w501, "TN"=w500) -> (w503:cluster{"TL":dbl, "TN":dbl})
                        n358 = local write "TEMP START LAB01-1"(w503) -> ()
                      }
                    }
                  }
                }
              }
              event "RUN LAB01-2": Value Change {
                n359 = event-data() -> ("NewVal"=w505:bool)  [unwired: 1 in, 5 out]
                n360 = local write "run lab01-2"(w505) -> ()
                n361 = case shown="True" w505 {
                  tunnel: w511 -> [_ w544]
                  tunnel: w510 -> [_ w543]
                  tunnel: w508 -> [w513 w542]
                  tunnel: w509 -> [_ w541]
                  tunnel: w507 -> [_ w540]
                  tunnel: [w512 w539] -> w506
                  frame False {
                    # "stop test"
                    n362 = stacked-sequence {
                      tunnel: w513 -> [w522 _]
                      tunnel: [w514 _] -> w512
                      frame #0 {
                        n363 = local read "DISP LAB01-2"() -> (w521:T4)
                        n364 = Unbundle(w521) -> ("CYCLE"=w519:dbl, "MINS"=w520:dbl)  [unwired: 1 out]
                        n365 = case shown="\"CHART TEST\", Default" w522 {
                          tunnel: w520 -> [_ _ w529]
                          tunnel: w519 -> [w527 w528 _]
                          tunnel: [w527 w528 w529] -> w518
                          frame "CHART TEST", Default {
                          }
                          frame "CYCLE TEST" {
                          }
                          frame "T-RISE TEST" {
                          }
                        }
                        n366 = local read "TDMS LAB01-2"() -> (w526:refnum<k34>)
                        n367 = Build Array("STOPPED") -> (w523:string[])
                        n368 = Build Array(w518) -> (w517:dbl[])
                        n369 = TDMS Write(0:w526, 5:"TEST RESULT", 7:w523, 9:w517) -> (4:w515:refnum<k34>, 15:w516:errorcluster)  [unwired: 2 in, 2 out]
                        n370 = TDMS Close(8:w516, 11:w515) -> (0:w514:errorcluster)  [unwired: 1 out]
                      }
                      frame #1 {
                        n371 = local read "DISP LAB01-2"() -> (w533:T4)
                        n372 = stacked-sequence {
                          tunnel: "LAB01-2" -> [w535 w537]
                          frame #0 {
                            n373 = call "sub vi - defrag tdms v1.vi"("panel id"=w535) -> ("error out"=w534:errorcluster)  [unwired: 10 in]
                            n374 = local write "data file error"(w534) -> ()
                          }
                          frame #1 {
                            n375 = call "Save data file to network drive v1.vi"("panel id"=w537) -> ("network file save error"=w536:errorcluster)  [unwired: 9 in, 1 out]
                            n376 = local write "RESULT LAB01-2"(FALSE) -> ()
                            n377 = local write "data file error"(w536) -> ()
                          }
                        }
                        n378 = Bundle(cluster=w533, "STATUS"="STOP") -> (w531:T4)  [unwired: 2 in]
                        n379 = local write "DISP LAB01-2"(w531) -> ()
                      }
                    }
                  }
                  frame True {
                    # "start new test and create test file"
                    n380 = stacked-sequence {
                      seq-local: [w545 _ _ _ _] -> [_ w570 _ _ _]
                      tunnel: w544 -> [w550 _ _ _ _]
                      tunnel: w543 -> [w547 _ _ _ _]
                      tunnel: w542 -> [w560 _ _ _ _]
                      tunnel: w541 -> [w553 _ _ _ _]
                      tunnel: w540 -> [w548 _ _ _ _]
                      tunnel: [_ w564 _ _ _] -> w539
                      frame #0 {
                        w546 = "\\"
                        n381 = local read "SET LAB01-2"() -> (w555:T5)
                        n382 = case shown="\"CYCLE TEST\"" w560 {
                          tunnel: ["L01-2-CHART TEST-" "L01-2-CYCLE TEST-" "L01-2-T-RISE TEST-"] -> w556
                          frame "CHART TEST", Default {
                          }
                          frame "CYCLE TEST" {
                          }
                          frame "T-RISE TEST" {
                          }
                        }
                        n383 = Unbundle(w555) -> ("DESCRIPTION"=w554:string)  [unwired: 4 out]
                        n384 = Concatenate Strings(w550, "\\", w548, w546, w547, w546) -> (w557:string)
                        n385 = String To Path(string=w557) -> (path=w559:path)
                        n386 = Concatenate Strings(w557, w556, w554, "-", w553, ".tdms") -> (w545:string)
                        n387 = Create Folder(path (use dialog)=w559) -> (error out=w558:errorcluster)  [unwired: 2 in, 2 out]
                        n388 = global write "Global 1.vi" "LAB01-2 FILE"(w545) -> ()
                        n389 = call <vilib>:"Clear Errors.vi"("error in (no error)"=w558) -> ()  [unwired: 6 in, 1 out]
                      }
                      frame #1 {
                        n390 = String To Path(string=w570) -> (path=w565:path)
                        n391 = TDMS Open(5:FALSE, 6:FALSE, 10:T17."create or replace" ("operation (0:open)"), 11:w565) -> (0:w564:errorcluster, 3:→"TDMS LAB01-2":refnum<k34>)  [unwired: 3 in]
                      }
                      frame #2 {
                        n392 = local read "SET LAB01-2"() -> (w576:T5)
                        n393 = local read "TDMS LAB01-2"() -> (w587:refnum<k34>)
                        n394 = Build Array("Testers Name", "Description", "Set Test Cycles", "T-Rise minutes", "T-Rise Deg C") -> (w577:string[])
                        n395 = Unbundle(w576) -> ("NAME"=w575:string, "DESCRIPTION"=w574:string, "CYCLES"=w573:dbl, "T-RISE mins"=w572:dbl, "T-RISE deg C"=w571:dbl)
                        n396 = Number To Decimal String(number=w573) -> (decimal integer string=w586:string)  [unwired: 1 in]
                        n397 = Number To Decimal String(number=w572) -> (decimal integer string=w585:string)  [unwired: 1 in]
                        n398 = Number To Decimal String(number=w571) -> (decimal integer string=w584:string)  [unwired: 1 in]
                        n399 = Build Array(w575, w574, w586, w585, w584) -> (w583:string[])
                        n400 = TDMS Set Properties(5:w583, 7:w577, 11:w587) -> ()  [unwired: 3 in, 4 out]
                      }
                      frame #3 {
                        w589 = 0.0
                        n401 = local read "DISP LAB01-2"() -> (w591:T4)
                        n402 = Bundle(cluster=w591, "CYCLE"=w589, "MINS"=w589, "STATUS"="RUN") -> (w590:T4)
                        n403 = local write "DISP LAB01-2"(w590) -> ()
                      }
                      frame #4 {
                        n404 = local read "SIG LAB01-2"() -> (w594:T2)
                        n405 = local read "TEMP START LAB01-2"() -> (w596:cluster{"TL":dbl, "TN":dbl})
                        n406 = Unbundle(w594) -> ("Tmp Live"=w593:dbl, "Tmp Neut"=w592:dbl)  [unwired: 3 out]
                        n407 = Bundle(cluster=w596, "TL"=w593, "TN"=w592) -> (w595:cluster{"TL":dbl, "TN":dbl})
                        n408 = local write "TEMP START LAB01-2"(w595) -> ()
                      }
                    }
                  }
                }
              }
              event "RUN LAB02-1": Value Change {
                n409 = event-data() -> ("NewVal"=w597:bool)  [unwired: 1 in, 5 out]
                n410 = local write "run lab02-1"(w597) -> ()
                n411 = case shown="True" w597 {
                  tunnel: w603 -> [_ w636]
                  tunnel: w602 -> [_ w635]
                  tunnel: w600 -> [w605 w634]
                  tunnel: w601 -> [_ w633]
                  tunnel: w599 -> [_ w632]
                  tunnel: [w604 w631] -> w598
                  frame False {
                    # "stop test"
                    n412 = stacked-sequence {
                      tunnel: w605 -> [w614 _]
                      tunnel: [w606 _] -> w604
                      frame #0 {
                        n413 = local read "DISP LAB02-1"() -> (w613:T4)
                        n414 = Unbundle(w613) -> ("CYCLE"=w611:dbl, "MINS"=w612:dbl)  [unwired: 1 out]
                        n415 = case shown="\"CYCLE TEST\"" w614 {
                          tunnel: w612 -> [_ _ w621]
                          tunnel: w611 -> [w619 w620 _]
                          tunnel: [w619 w620 w621] -> w610
                          frame "CHART TEST", Default {
                          }
                          frame "CYCLE TEST" {
                          }
                          frame "T-RISE TEST" {
                          }
                        }
                        n416 = local read "TDMS LAB02-1"() -> (w618:refnum<k34>)
                        n417 = Build Array("STOPPED") -> (w615:string[])
                        n418 = Build Array(w610) -> (w609:dbl[])
                        n419 = TDMS Write(0:w618, 5:"TEST RESULT", 7:w615, 9:w609) -> (4:w607:refnum<k34>, 15:w608:errorcluster)  [unwired: 2 in, 2 out]
                        n420 = TDMS Close(8:w608, 11:w607) -> (0:w606:errorcluster)  [unwired: 1 out]
                      }
                      frame #1 {
                        n421 = local read "DISP LAB02-1"() -> (w625:T4)
                        n422 = stacked-sequence {
                          tunnel: "LAB02-1" -> [w627 w629]
                          frame #0 {
                            n423 = call "sub vi - defrag tdms v1.vi"("panel id"=w627) -> ("error out"=w626:errorcluster)  [unwired: 10 in]
                            n424 = local write "data file error"(w626) -> ()
                          }
                          frame #1 {
                            n425 = local write "RESULT LAB02-1"(FALSE) -> ()
                            n426 = call "Save data file to network drive v1.vi"("panel id"=w629) -> ("network file save error"=w628:errorcluster)  [unwired: 9 in, 1 out]
                            n427 = local write "data file error"(w628) -> ()
                          }
                        }
                        n428 = Bundle(cluster=w625, "STATUS"="STOP") -> (w623:T4)  [unwired: 2 in]
                        n429 = local write "DISP LAB02-1"(w623) -> ()
                      }
                    }
                  }
                  frame True {
                    # "start new test and create test file"
                    n430 = stacked-sequence {
                      seq-local: [w637 _ _ _ _] -> [_ w662 _ _ _]
                      tunnel: w636 -> [w642 _ _ _ _]
                      tunnel: w635 -> [w639 _ _ _ _]
                      tunnel: w634 -> [w652 _ _ _ _]
                      tunnel: w633 -> [w645 _ _ _ _]
                      tunnel: w632 -> [w640 _ _ _ _]
                      tunnel: [_ w656 _ _ _] -> w631
                      frame #0 {
                        w638 = "\\"
                        n431 = local read "SET LAB02-1"() -> (w647:T5)
                        n432 = case shown="\"CYCLE TEST\"" w652 {
                          tunnel: ["L02-1-CHART TEST-" "L02-1-CYCLE TEST-" "L02-1-T-RISE TEST-"] -> w648
                          frame "CHART TEST", Default {
                          }
                          frame "CYCLE TEST" {
                          }
                          frame "T-RISE TEST" {
                          }
                        }
                        n433 = Unbundle(w647) -> ("DESCRIPTION"=w646:string)  [unwired: 4 out]
                        n434 = Concatenate Strings(w642, "\\", w640, w638, w639, w638) -> (w649:string)
                        n435 = String To Path(string=w649) -> (path=w651:path)
                        n436 = Concatenate Strings(w649, w648, w646, "-", w645, ".tdms") -> (w637:string)
                        n437 = Create Folder(path (use dialog)=w651) -> (error out=w650:errorcluster)  [unwired: 2 in, 2 out]
                        n438 = global write "Global 1.vi" "LAB02-1 FILE"(w637) -> ()
                        n439 = call <vilib>:"Clear Errors.vi"("error in (no error)"=w650) -> ()  [unwired: 6 in, 1 out]
                      }
                      frame #1 {
                        n440 = String To Path(string=w662) -> (path=w657:path)
                        n441 = TDMS Open(5:FALSE, 6:FALSE, 10:T17."create or replace" ("operation (0:open)"), 11:w657) -> (0:w656:errorcluster, 3:→"TDMS LAB02-1":refnum<k34>)  [unwired: 3 in]
                      }
                      frame #2 {
                        n442 = local read "SET LAB02-1"() -> (w668:T5)
                        n443 = local read "TDMS LAB02-1"() -> (w679:refnum<k34>)
                        n444 = Build Array("Testers Name", "Description", "Set Test Cycles", "T-Rise minutes", "T-Rise Deg C") -> (w669:string[])
                        n445 = Unbundle(w668) -> ("NAME"=w667:string, "DESCRIPTION"=w666:string, "CYCLES"=w665:dbl, "T-RISE mins"=w664:dbl, "T-RISE deg C"=w663:dbl)
                        n446 = Number To Decimal String(number=w665) -> (decimal integer string=w678:string)  [unwired: 1 in]
                        n447 = Number To Decimal String(number=w664) -> (decimal integer string=w677:string)  [unwired: 1 in]
                        n448 = Number To Decimal String(number=w663) -> (decimal integer string=w676:string)  [unwired: 1 in]
                        n449 = Build Array(w667, w666, w678, w677, w676) -> (w675:string[])
                        n450 = TDMS Set Properties(5:w675, 7:w669, 11:w679) -> ()  [unwired: 3 in, 4 out]
                      }
                      frame #3 {
                        w681 = 0.0
                        n451 = local read "DISP LAB02-1"() -> (w683:T4)
                        n452 = Bundle(cluster=w683, "CYCLE"=w681, "MINS"=w681, "STATUS"="RUN") -> (w682:T4)
                        n453 = local write "DISP LAB02-1"(w682) -> ()
                      }
                      frame #4 {
                        n454 = local read "SIG LAB02-1"() -> (w686:T2)
                        n455 = local read "TEMP START LAB02-1"() -> (w688:cluster{"TL":dbl, "TN":dbl})
                        n456 = Unbundle(w686) -> ("Tmp Live"=w685:dbl, "Tmp Neut"=w684:dbl)  [unwired: 3 out]
                        n457 = Bundle(cluster=w688, "TL"=w685, "TN"=w684) -> (w687:cluster{"TL":dbl, "TN":dbl})
                        n458 = local write "TEMP START LAB02-1"(w687) -> ()
                      }
                    }
                  }
                }
              }
              event "RUN LAB02-2": Value Change {
                n459 = event-data() -> ("NewVal"=w689:bool)  [unwired: 1 in, 5 out]
                n460 = local write "run lab02-2"(w689) -> ()
                n461 = case shown="True" w689 {
                  tunnel: w695 -> [_ w728]
                  tunnel: w694 -> [_ w727]
                  tunnel: w692 -> [w697 w726]
                  tunnel: w693 -> [_ w725]
                  tunnel: w691 -> [_ w724]
                  tunnel: [w696 w723] -> w690
                  frame False {
                    # "stop test"
                    n462 = stacked-sequence {
                      tunnel: w697 -> [w706 _]
                      tunnel: [w698 _] -> w696
                      frame #0 {
                        n463 = local read "DISP LAB02-2"() -> (w705:T4)
                        n464 = Unbundle(w705) -> ("CYCLE"=w703:dbl, "MINS"=w704:dbl)  [unwired: 1 out]
                        n465 = case shown="\"CYCLE TEST\"" w706 {
                          tunnel: w704 -> [_ _ w713]
                          tunnel: w703 -> [w711 w712 _]
                          tunnel: [w711 w712 w713] -> w702
                          frame "CHART TEST", Default {
                          }
                          frame "CYCLE TEST" {
                          }
                          frame "T-RISE TEST" {
                          }
                        }
                        n466 = local read "TDMS LAB02-2"() -> (w710:refnum<k34>)
                        n467 = Build Array("STOPPED") -> (w707:string[])
                        n468 = Build Array(w702) -> (w701:dbl[])
                        n469 = TDMS Write(0:w710, 5:"TEST RESULT", 7:w707, 9:w701) -> (4:w699:refnum<k34>, 15:w700:errorcluster)  [unwired: 2 in, 2 out]
                        n470 = TDMS Close(8:w700, 11:w699) -> (0:w698:errorcluster)  [unwired: 1 out]
                      }
                      frame #1 {
                        n471 = local read "DISP LAB02-2"() -> (w717:T4)
                        n472 = stacked-sequence {
                          tunnel: "LAB02-2" -> [w719 w721]
                          frame #0 {
                            n473 = call "sub vi - defrag tdms v1.vi"("panel id"=w719) -> ("error out"=w718:errorcluster)  [unwired: 10 in]
                            n474 = local write "data file error"(w718) -> ()
                          }
                          frame #1 {
                            n475 = call "Save data file to network drive v1.vi"("panel id"=w721) -> ("network file save error"=w720:errorcluster)  [unwired: 9 in, 1 out]
                            n476 = local write "RESULT LAB02-2"(FALSE) -> ()
                            n477 = local write "data file error"(w720) -> ()
                          }
                        }
                        n478 = Bundle(cluster=w717, "STATUS"="STOP") -> (w715:T4)  [unwired: 2 in]
                        n479 = local write "DISP LAB02-2"(w715) -> ()
                      }
                    }
                  }
                  frame True {
                    # "start new test and create test file"
                    n480 = stacked-sequence {
                      seq-local: [w729 _ _ _ _] -> [_ w754 _ _ _]
                      tunnel: w728 -> [w734 _ _ _ _]
                      tunnel: w727 -> [w731 _ _ _ _]
                      tunnel: w726 -> [w744 _ _ _ _]
                      tunnel: w725 -> [w737 _ _ _ _]
                      tunnel: w724 -> [w732 _ _ _ _]
                      tunnel: [_ w748 _ _ _] -> w723
                      frame #0 {
                        w730 = "\\"
                        n481 = local read "SET LAB02-2"() -> (w739:T5)
                        n482 = case shown="\"CYCLE TEST\"" w744 {
                          tunnel: ["L02-2-CHART TEST-" "L02-2-CYCLE TEST-" "L02-2-T-RISE TEST-"] -> w740
                          frame "CHART TEST", Default {
                          }
                          frame "CYCLE TEST" {
                          }
                          frame "T-RISE TEST" {
                          }
                        }
                        n483 = Unbundle(w739) -> ("DESCRIPTION"=w738:string)  [unwired: 4 out]
                        n484 = Concatenate Strings(w734, "\\", w732, w730, w731, w730) -> (w741:string)
                        n485 = String To Path(string=w741) -> (path=w743:path)
                        n486 = Concatenate Strings(w741, w740, w738, "-", w737, ".tdms") -> (w729:string)
                        n487 = Create Folder(path (use dialog)=w743) -> (error out=w742:errorcluster)  [unwired: 2 in, 2 out]
                        n488 = global write "Global 1.vi" "LAB02-2 FILE"(w729) -> ()
                        n489 = call <vilib>:"Clear Errors.vi"("error in (no error)"=w742) -> ()  [unwired: 6 in, 1 out]
                      }
                      frame #1 {
                        n490 = String To Path(string=w754) -> (path=w749:path)
                        n491 = TDMS Open(5:FALSE, 6:FALSE, 10:T17."create or replace" ("operation (0:open)"), 11:w749) -> (0:w748:errorcluster, 3:→"TDMS LAB02-2":refnum<k34>)  [unwired: 3 in]
                      }
                      frame #2 {
                        n492 = local read "SET LAB02-2"() -> (w760:T5)
                        n493 = local read "TDMS LAB02-2"() -> (w771:refnum<k34>)
                        n494 = Build Array("Testers Name", "Description", "Set Test Cycles", "T-Rise minutes", "T-Rise Deg C") -> (w761:string[])
                        n495 = Unbundle(w760) -> ("NAME"=w759:string, "DESCRIPTION"=w758:string, "CYCLES"=w757:dbl, "T-RISE mins"=w756:dbl, "T-RISE deg C"=w755:dbl)
                        n496 = Number To Decimal String(number=w757) -> (decimal integer string=w770:string)  [unwired: 1 in]
                        n497 = Number To Decimal String(number=w756) -> (decimal integer string=w769:string)  [unwired: 1 in]
                        n498 = Number To Decimal String(number=w755) -> (decimal integer string=w768:string)  [unwired: 1 in]
                        n499 = Build Array(w759, w758, w770, w769, w768) -> (w767:string[])
                        n500 = TDMS Set Properties(5:w767, 7:w761, 11:w771) -> ()  [unwired: 3 in, 4 out]
                      }
                      frame #3 {
                        w773 = 0.0
                        n501 = local read "DISP LAB02-2"() -> (w775:T4)
                        n502 = Bundle(cluster=w775, "CYCLE"=w773, "MINS"=w773, "STATUS"="RUN") -> (w774:T4)
                        n503 = local write "DISP LAB02-2"(w774) -> ()
                      }
                      frame #4 {
                        n504 = local read "SIG LAB02-2"() -> (w778:T2)
                        n505 = local read "TEMP START LAB02-2"() -> (w780:cluster{"TL":dbl, "TN":dbl})
                        n506 = Unbundle(w778) -> ("Tmp Live"=w777:dbl, "Tmp Neut"=w776:dbl)  [unwired: 3 out]
                        n507 = Bundle(cluster=w780, "TL"=w777, "TN"=w776) -> (w779:cluster{"TL":dbl, "TN":dbl})
                        n508 = local write "TEMP START LAB02-2"(w779) -> ()
                      }
                    }
                  }
                }
              }
              event "RUN LAB03-1": Value Change {
                n509 = event-data() -> ("NewVal"=w781:bool)  [unwired: 1 in, 5 out]
                n510 = local write "run lab03-1"(w781) -> ()
                n511 = case shown="True" w781 {
                  tunnel: w787 -> [_ w820]
                  tunnel: w786 -> [_ w819]
                  tunnel: w784 -> [w789 w818]
                  tunnel: w785 -> [_ w817]
                  tunnel: w783 -> [_ w816]
                  tunnel: [w788 w815] -> w782
                  frame False {
                    # "stop test"
                    n512 = stacked-sequence {
                      tunnel: w789 -> [w798 _]
                      tunnel: [w790 _] -> w788
                      frame #0 {
                        n513 = local read "DISP LAB03-1"() -> (w797:T4)
                        n514 = Unbundle(w797) -> ("CYCLE"=w795:dbl, "MINS"=w796:dbl)  [unwired: 1 out]
                        n515 = case shown="\"CYCLE TEST\"" w798 {
                          tunnel: w796 -> [_ _ w805]
                          tunnel: w795 -> [w803 w804 _]
                          tunnel: [w803 w804 w805] -> w794
                          frame "CHART TEST", Default {
                          }
                          frame "CYCLE TEST" {
                          }
                          frame "T-RISE TEST" {
                          }
                        }
                        n516 = local read "TDMS LAB03-1"() -> (w802:refnum<k34>)
                        n517 = Build Array("STOPPED") -> (w799:string[])
                        n518 = Build Array(w794) -> (w793:dbl[])
                        n519 = TDMS Write(0:w802, 5:"TEST RESULT", 7:w799, 9:w793) -> (4:w791:refnum<k34>, 15:w792:errorcluster)  [unwired: 2 in, 2 out]
                        n520 = TDMS Close(8:w792, 11:w791) -> (0:w790:errorcluster)  [unwired: 1 out]
                      }
                      frame #1 {
                        n521 = local read "DISP LAB03-1"() -> (w809:T4)
                        n522 = stacked-sequence {
                          tunnel: "LAB03-1" -> [w811 w813]
                          frame #0 {
                            n523 = call "sub vi - defrag tdms v1.vi"("panel id"=w811) -> ("error out"=w810:errorcluster)  [unwired: 10 in]
                            n524 = local write "data file error"(w810) -> ()
                          }
                          frame #1 {
                            n525 = call "Save data file to network drive v1.vi"("panel id"=w813) -> ("network file save error"=w812:errorcluster)  [unwired: 9 in, 1 out]
                            n526 = local write "RESULT LAB03-1"(FALSE) -> ()
                            n527 = local write "data file error"(w812) -> ()
                          }
                        }
                        n528 = Bundle(cluster=w809, "STATUS"="STOP") -> (w807:T4)  [unwired: 2 in]
                        n529 = local write "DISP LAB03-1"(w807) -> ()
                      }
                    }
                  }
                  frame True {
                    # "start new test and create test file"
                    n530 = stacked-sequence {
                      seq-local: [w821 _ _ _ _] -> [_ w846 _ _ _]
                      tunnel: w820 -> [w826 _ _ _ _]
                      tunnel: w819 -> [w823 _ _ _ _]
                      tunnel: w818 -> [w836 _ _ _ _]
                      tunnel: w817 -> [w829 _ _ _ _]
                      tunnel: w816 -> [w824 _ _ _ _]
                      tunnel: [_ w840 _ _ _] -> w815
                      frame #0 {
                        w822 = "\\"
                        n531 = local read "SET LAB03-1"() -> (w831:T5)
                        n532 = case shown="\"T-RISE TEST\"" w836 {
                          tunnel: ["L03-1-CHART TEST-" "L03-1-CYCLE TEST-" "L03-1-T-RISE TEST-"] -> w832
                          frame "CHART TEST", Default {
                          }
                          frame "CYCLE TEST" {
                          }
                          frame "T-RISE TEST" {
                          }
                        }
                        n533 = Unbundle(w831) -> ("DESCRIPTION"=w830:string)  [unwired: 4 out]
                        n534 = Concatenate Strings(w826, "\\", w824, w822, w823, w822) -> (w833:string)
                        n535 = String To Path(string=w833) -> (path=w835:path)
                        n536 = Concatenate Strings(w833, w832, w830, "-", w829, ".tdms") -> (w821:string)
                        n537 = Create Folder(path (use dialog)=w835) -> (error out=w834:errorcluster)  [unwired: 2 in, 2 out]
                        n538 = global write "Global 1.vi" "LAB03-1 FILE"(w821) -> ()
                        n539 = call <vilib>:"Clear Errors.vi"("error in (no error)"=w834) -> ()  [unwired: 6 in, 1 out]
                      }
                      frame #1 {
                        n540 = String To Path(string=w846) -> (path=w841:path)
                        n541 = TDMS Open(5:FALSE, 6:FALSE, 10:T17."create or replace" ("operation (0:open)"), 11:w841) -> (0:w840:errorcluster, 3:→"TDMS LAB03-1":refnum<k34>)  [unwired: 3 in]
                      }
                      frame #2 {
                        n542 = local read "SET LAB03-1"() -> (w852:T5)
                        n543 = local read "TDMS LAB03-1"() -> (w863:refnum<k34>)
                        n544 = Build Array("Testers Name", "Description", "Set Test Cycles", "T-Rise minutes", "T-Rise Deg C") -> (w853:string[])
                        n545 = Unbundle(w852) -> ("NAME"=w851:string, "DESCRIPTION"=w850:string, "CYCLES"=w849:dbl, "T-RISE mins"=w848:dbl, "T-RISE deg C"=w847:dbl)
                        n546 = Number To Decimal String(number=w849) -> (decimal integer string=w862:string)  [unwired: 1 in]
                        n547 = Number To Decimal String(number=w848) -> (decimal integer string=w861:string)  [unwired: 1 in]
                        n548 = Number To Decimal String(number=w847) -> (decimal integer string=w860:string)  [unwired: 1 in]
                        n549 = Build Array(w851, w850, w862, w861, w860) -> (w859:string[])
                        n550 = TDMS Set Properties(5:w859, 7:w853, 11:w863) -> ()  [unwired: 3 in, 4 out]
                      }
                      frame #3 {
                        w865 = 0.0
                        n551 = local read "DISP LAB03-1"() -> (w867:T4)
                        n552 = Bundle(cluster=w867, "CYCLE"=w865, "MINS"=w865, "STATUS"="RUN") -> (w866:T4)
                        n553 = local write "DISP LAB03-1"(w866) -> ()
                      }
                      frame #4 {
                        n554 = local read "SIG LAB03-1"() -> (w870:T2)
                        n555 = local read "TEMP START LAB03-1"() -> (w872:cluster{"TL":dbl, "TN":dbl})
                        n556 = Unbundle(w870) -> ("Tmp Live"=w869:dbl, "Tmp Neut"=w868:dbl)  [unwired: 3 out]
                        n557 = Bundle(cluster=w872, "TL"=w869, "TN"=w868) -> (w871:cluster{"TL":dbl, "TN":dbl})
                        n558 = local write "TEMP START LAB03-1"(w871) -> ()
                      }
                    }
                  }
                }
              }
              event "RUN LAB03-2": Value Change {
                n559 = event-data() -> ("NewVal"=w873:bool)  [unwired: 1 in, 5 out]
                n560 = local write "run lab03-2"(w873) -> ()
                n561 = case shown="True" w873 {
                  tunnel: w879 -> [_ w912]
                  tunnel: w878 -> [_ w911]
                  tunnel: w876 -> [w881 w910]
                  tunnel: w877 -> [_ w909]
                  tunnel: w875 -> [_ w908]
                  tunnel: [w880 w907] -> w874
                  frame False {
                    # "stop test"
                    n562 = stacked-sequence {
                      tunnel: w881 -> [w890 _]
                      tunnel: [w882 _] -> w880
                      frame #0 {
                        n563 = local read "DISP LAB03-2"() -> (w889:T4)
                        n564 = Unbundle(w889) -> ("CYCLE"=w887:dbl, "MINS"=w888:dbl)  [unwired: 1 out]
                        n565 = case shown="\"CYCLE TEST\"" w890 {
                          tunnel: w888 -> [_ _ w897]
                          tunnel: w887 -> [w895 w896 _]
                          tunnel: [w895 w896 w897] -> w886
                          frame "CHART TEST", Default {
                          }
                          frame "CYCLE TEST" {
                          }
                          frame "T-RISE TEST" {
                          }
                        }
                        n566 = local read "TDMS LAB03-2"() -> (w894:refnum<k34>)
                        n567 = Build Array("STOPPED") -> (w891:string[])
                        n568 = Build Array(w886) -> (w885:dbl[])
                        n569 = TDMS Write(0:w894, 5:"TEST RESULT", 7:w891, 9:w885) -> (4:w883:refnum<k34>, 15:w884:errorcluster)  [unwired: 2 in, 2 out]
                        n570 = TDMS Close(8:w884, 11:w883) -> (0:w882:errorcluster)  [unwired: 1 out]
                      }
                      frame #1 {
                        n571 = local read "DISP LAB03-2"() -> (w901:T4)
                        n572 = stacked-sequence {
                          tunnel: "LAB03-2" -> [w903 w905]
                          frame #0 {
                            n573 = call "sub vi - defrag tdms v1.vi"("panel id"=w903) -> ("error out"=w902:errorcluster)  [unwired: 10 in]
                            n574 = local write "data file error"(w902) -> ()
                          }
                          frame #1 {
                            n575 = call "Save data file to network drive v1.vi"("panel id"=w905) -> ("network file save error"=w904:errorcluster)  [unwired: 9 in, 1 out]
                            n576 = local write "RESULT LAB03-2"(FALSE) -> ()
                            n577 = local write "data file error"(w904) -> ()
                          }
                        }
                        n578 = Bundle(cluster=w901, "STATUS"="STOP") -> (w899:T4)  [unwired: 2 in]
                        n579 = local write "DISP LAB03-2"(w899) -> ()
                      }
                    }
                  }
                  frame True {
                    # "start new test and create test file"
                    n580 = stacked-sequence {
                      seq-local: [w913 _ _ _ _] -> [_ w938 _ _ _]
                      tunnel: w912 -> [w918 _ _ _ _]
                      tunnel: w911 -> [w915 _ _ _ _]
                      tunnel: w910 -> [w928 _ _ _ _]
                      tunnel: w909 -> [w921 _ _ _ _]
                      tunnel: w908 -> [w916 _ _ _ _]
                      tunnel: [_ w932 _ _ _] -> w907
                      frame #0 {
                        w914 = "\\"
                        n581 = local read "SET LAB03-2"() -> (w923:T5)
                        n582 = case shown="\"T-RISE TEST\"" w928 {
                          tunnel: ["L03-2-CHART TEST-" "L03-2-CYCLE TEST-" "L03-2-T-RISE TEST-"] -> w924
                          frame "CHART TEST", Default {
                          }
                          frame "CYCLE TEST" {
                          }
                          frame "T-RISE TEST" {
                          }
                        }
                        n583 = Unbundle(w923) -> ("DESCRIPTION"=w922:string)  [unwired: 4 out]
                        n584 = Concatenate Strings(w918, "\\", w916, w914, w915, w914) -> (w925:string)
                        n585 = String To Path(string=w925) -> (path=w927:path)
                        n586 = Concatenate Strings(w925, w924, w922, "-", w921, ".tdms") -> (w913:string)
                        n587 = Create Folder(path (use dialog)=w927) -> (error out=w926:errorcluster)  [unwired: 2 in, 2 out]
                        n588 = global write "Global 1.vi" "LAB03-2 FILE"(w913) -> ()
                        n589 = call <vilib>:"Clear Errors.vi"("error in (no error)"=w926) -> ()  [unwired: 6 in, 1 out]
                      }
                      frame #1 {
                        n590 = String To Path(string=w938) -> (path=w933:path)
                        n591 = TDMS Open(5:FALSE, 6:FALSE, 10:T17."create or replace" ("operation (0:open)"), 11:w933) -> (0:w932:errorcluster, 3:→"TDMS LAB03-2":refnum<k34>)  [unwired: 3 in]
                      }
                      frame #2 {
                        n592 = local read "SET LAB03-2"() -> (w944:T5)
                        n593 = local read "TDMS LAB03-2"() -> (w955:refnum<k34>)
                        n594 = Build Array("Testers Name", "Description", "Set Test Cycles", "T-Rise minutes", "T-Rise Deg C") -> (w945:string[])
                        n595 = Unbundle(w944) -> ("NAME"=w943:string, "DESCRIPTION"=w942:string, "CYCLES"=w941:dbl, "T-RISE mins"=w940:dbl, "T-RISE deg C"=w939:dbl)
                        n596 = Number To Decimal String(number=w941) -> (decimal integer string=w954:string)  [unwired: 1 in]
                        n597 = Number To Decimal String(number=w940) -> (decimal integer string=w953:string)  [unwired: 1 in]
                        n598 = Number To Decimal String(number=w939) -> (decimal integer string=w952:string)  [unwired: 1 in]
                        n599 = Build Array(w943, w942, w954, w953, w952) -> (w951:string[])
                        n600 = TDMS Set Properties(5:w951, 7:w945, 11:w955) -> ()  [unwired: 3 in, 4 out]
                      }
                      frame #3 {
                        w957 = 0.0
                        n601 = local read "DISP LAB03-2"() -> (w959:T4)
                        n602 = Bundle(cluster=w959, "CYCLE"=w957, "MINS"=w957, "STATUS"="RUN") -> (w958:T4)
                        n603 = local write "DISP LAB03-2"(w958) -> ()
                      }
                      frame #4 {
                        n604 = local read "SIG LAB03-2"() -> (w962:T2)
                        n605 = local read "TEMP START LAB03-2"() -> (w964:cluster{"TL":dbl, "TN":dbl})
                        n606 = Unbundle(w962) -> ("Tmp Live"=w961:dbl, "Tmp Neut"=w960:dbl)  [unwired: 3 out]
                        n607 = Bundle(cluster=w964, "TL"=w961, "TN"=w960) -> (w963:cluster{"TL":dbl, "TN":dbl})
                        n608 = local write "TEMP START LAB03-2"(w963) -> ()
                      }
                    }
                  }
                }
              }
              event "RUN LAB04-1": Value Change {
                n609 = event-data() -> ("NewVal"=w965:bool)  [unwired: 1 in, 5 out]
                n610 = local write "run lab04-1"(w965) -> ()
                n611 = case shown="True" w965 {
                  tunnel: w971 -> [_ w1004]
                  tunnel: w970 -> [_ w1003]
                  tunnel: w968 -> [w973 w1002]
                  tunnel: w969 -> [_ w1001]
                  tunnel: w967 -> [_ w1000]
                  tunnel: [w972 w999] -> w966
                  frame False {
                    # "stop test"
                    n612 = stacked-sequence {
                      tunnel: w973 -> [w982 _]
                      tunnel: [w974 _] -> w972
                      frame #0 {
                        n613 = local read "DISP LAB04-1"() -> (w981:T4)
                        n614 = Unbundle(w981) -> ("CYCLE"=w979:dbl, "MINS"=w980:dbl)  [unwired: 1 out]
                        n615 = case shown="\"CYCLE TEST\"" w982 {
                          tunnel: w980 -> [_ _ w989]
                          tunnel: w979 -> [w987 w988 _]
                          tunnel: [w987 w988 w989] -> w978
                          frame "CHART TEST", Default {
                          }
                          frame "CYCLE TEST" {
                          }
                          frame "T-RISE TEST" {
                          }
                        }
                        n616 = local read "TDMS LAB04-1"() -> (w986:refnum<k34>)
                        n617 = Build Array("STOPPED") -> (w983:string[])
                        n618 = Build Array(w978) -> (w977:dbl[])
                        n619 = TDMS Write(0:w986, 5:"TEST RESULT", 7:w983, 9:w977) -> (4:w975:refnum<k34>, 15:w976:errorcluster)  [unwired: 2 in, 2 out]
                        n620 = TDMS Close(8:w976, 11:w975) -> (0:w974:errorcluster)  [unwired: 1 out]
                      }
                      frame #1 {
                        n621 = local read "DISP LAB04-1"() -> (w993:T4)
                        n622 = stacked-sequence {
                          tunnel: "LAB04-1" -> [w995 w997]
                          frame #0 {
                            n623 = call "sub vi - defrag tdms v1.vi"("panel id"=w995) -> ("error out"=w994:errorcluster)  [unwired: 10 in]
                            n624 = local write "data file error"(w994) -> ()
                          }
                          frame #1 {
                            n625 = call "Save data file to network drive v1.vi"("panel id"=w997) -> ("network file save error"=w996:errorcluster)  [unwired: 9 in, 1 out]
                            n626 = local write "RESULT LAB04-1"(FALSE) -> ()
                            n627 = local write "data file error"(w996) -> ()
                          }
                        }
                        n628 = Bundle(cluster=w993, "STATUS"="STOP") -> (w991:T4)  [unwired: 2 in]
                        n629 = local write "DISP LAB04-1"(w991) -> ()
                      }
                    }
                  }
                  frame True {
                    # "start new test and create test file"
                    n630 = stacked-sequence {
                      seq-local: [w1005 _ _ _ _] -> [_ w1030 _ _ _]
                      tunnel: w1004 -> [w1010 _ _ _ _]
                      tunnel: w1003 -> [w1006 _ _ _ _]
                      tunnel: w1002 -> [w1020 _ _ _ _]
                      tunnel: w1001 -> [w1013 _ _ _ _]
                      tunnel: w1000 -> [w1008 _ _ _ _]
                      tunnel: [_ w1024 _ _ _] -> w999
                      frame #0 {
                        w1007 = "\\"
                        n631 = local read "SET LAB04-1"() -> (w1015:T5)
                        n632 = case shown="\"CYCLE TEST\"" w1020 {
                          tunnel: ["L04-1-CHART TEST-" "L04-1-CYCLE TEST-" "L04-1-T-RISE TEST-"] -> w1016
                          frame "CHART TEST", Default {
                          }
                          frame "CYCLE TEST" {
                          }
                          frame "T-RISE TEST" {
                          }
                        }
                        n633 = Unbundle(w1015) -> ("DESCRIPTION"=w1014:string)  [unwired: 4 out]
                        n634 = Concatenate Strings(w1010, "\\", w1008, w1007, w1006, w1007) -> (w1017:string)
                        n635 = String To Path(string=w1017) -> (path=w1019:path)
                        n636 = Concatenate Strings(w1017, w1016, w1014, "-", w1013, ".tdms") -> (w1005:string)
                        n637 = Create Folder(path (use dialog)=w1019) -> (error out=w1018:errorcluster)  [unwired: 2 in, 2 out]
                        n638 = global write "Global 1.vi" "LAB04-1 FILE"(w1005) -> ()
                        n639 = call <vilib>:"Clear Errors.vi"("error in (no error)"=w1018) -> ()  [unwired: 6 in, 1 out]
                      }
                      frame #1 {
                        n640 = String To Path(string=w1030) -> (path=w1025:path)
                        n641 = TDMS Open(5:FALSE, 6:FALSE, 10:T17."create or replace" ("operation (0:open)"), 11:w1025) -> (0:w1024:errorcluster, 3:→"TDMS LAB04-1":refnum<k34>)  [unwired: 3 in]
                      }
                      frame #2 {
                        n642 = local read "SET LAB04-1"() -> (w1036:T5)
                        n643 = local read "TDMS LAB04-1"() -> (w1047:refnum<k34>)
                        n644 = Build Array("Testers Name", "Description", "Set Test Cycles", "T-Rise minutes", "T-Rise Deg C") -> (w1037:string[])
                        n645 = Unbundle(w1036) -> ("NAME"=w1035:string, "DESCRIPTION"=w1034:string, "CYCLES"=w1033:dbl, "T-RISE mins"=w1032:dbl, "T-RISE deg C"=w1031:dbl)
                        n646 = Number To Decimal String(number=w1033) -> (decimal integer string=w1046:string)  [unwired: 1 in]
                        n647 = Number To Decimal String(number=w1032) -> (decimal integer string=w1045:string)  [unwired: 1 in]
                        n648 = Number To Decimal String(number=w1031) -> (decimal integer string=w1044:string)  [unwired: 1 in]
                        n649 = Build Array(w1035, w1034, w1046, w1045, w1044) -> (w1043:string[])
                        n650 = TDMS Set Properties(5:w1043, 7:w1037, 11:w1047) -> ()  [unwired: 3 in, 4 out]
                      }
                      frame #3 {
                        w1049 = 0.0
                        n651 = local read "DISP LAB04-1"() -> (w1051:T4)
                        n652 = Bundle(cluster=w1051, "CYCLE"=w1049, "MINS"=w1049, "STATUS"="RUN") -> (w1050:T4)
                        n653 = local write "DISP LAB04-1"(w1050) -> ()
                      }
                      frame #4 {
                        n654 = local read "SIG LAB04-1"() -> (w1054:T2)
                        n655 = local read "TEMP START LAB04-1"() -> (w1056:cluster{"TL":dbl, "TN":dbl})
                        n656 = Unbundle(w1054) -> ("Tmp Live"=w1053:dbl, "Tmp Neut"=w1052:dbl)  [unwired: 3 out]
                        n657 = Bundle(cluster=w1056, "TL"=w1053, "TN"=w1052) -> (w1055:cluster{"TL":dbl, "TN":dbl})
                        n658 = local write "TEMP START LAB04-1"(w1055) -> ()
                      }
                    }
                  }
                }
              }
              event "RUN LAB04-2": Value Change {
                n659 = event-data() -> ("NewVal"=w1057:bool)  [unwired: 1 in, 5 out]
                n660 = local write "run lab04-2"(w1057) -> ()
                n661 = case shown="True" w1057 {
                  tunnel: w1063 -> [_ w1096]
                  tunnel: w1062 -> [_ w1095]
                  tunnel: w1060 -> [w1065 w1094]
                  tunnel: w1061 -> [_ w1093]
                  tunnel: w1059 -> [_ w1092]
                  tunnel: [w1064 w1091] -> w1058
                  frame False {
                    # "stop test"
                    n662 = stacked-sequence {
                      tunnel: w1065 -> [w1074 _]
                      tunnel: [w1066 _] -> w1064
                      frame #0 {
                        n663 = local read "DISP LAB04-2"() -> (w1073:T4)
                        n664 = Unbundle(w1073) -> ("CYCLE"=w1071:dbl, "MINS"=w1072:dbl)  [unwired: 1 out]
                        n665 = case shown="\"CYCLE TEST\"" w1074 {
                          tunnel: w1072 -> [_ _ w1081]
                          tunnel: w1071 -> [w1079 w1080 _]
                          tunnel: [w1079 w1080 w1081] -> w1070
                          frame "CHART TEST", Default {
                          }
                          frame "CYCLE TEST" {
                          }
                          frame "T-RISE TEST" {
                          }
                        }
                        n666 = local read "TDMS LAB04-2"() -> (w1078:refnum<k34>)
                        n667 = Build Array("STOPPED") -> (w1075:string[])
                        n668 = Build Array(w1070) -> (w1069:dbl[])
                        n669 = TDMS Write(0:w1078, 5:"TEST RESULT", 7:w1075, 9:w1069) -> (4:w1067:refnum<k34>, 15:w1068:errorcluster)  [unwired: 2 in, 2 out]
                        n670 = TDMS Close(8:w1068, 11:w1067) -> (0:w1066:errorcluster)  [unwired: 1 out]
                      }
                      frame #1 {
                        n671 = local read "DISP LAB04-2"() -> (w1085:T4)
                        n672 = stacked-sequence {
                          tunnel: "LAB04-2" -> [w1087 w1089]
                          frame #0 {
                            n673 = call "sub vi - defrag tdms v1.vi"("panel id"=w1087) -> ("error out"=w1086:errorcluster)  [unwired: 10 in]
                            n674 = local write "data file error"(w1086) -> ()
                          }
                          frame #1 {
                            n675 = call "Save data file to network drive v1.vi"("panel id"=w1089) -> ("network file save error"=w1088:errorcluster)  [unwired: 9 in, 1 out]
                            n676 = local write "RESULT LAB04-2"(FALSE) -> ()
                            n677 = local write "data file error"(w1088) -> ()
                          }
                        }
                        n678 = Bundle(cluster=w1085, "STATUS"="STOP") -> (w1083:T4)  [unwired: 2 in]
                        n679 = local write "DISP LAB04-2"(w1083) -> ()
                      }
                    }
                  }
                  frame True {
                    # "start new test and create test file"
                    n680 = stacked-sequence {
                      seq-local: [w1097 _ _ _ _] -> [_ w1122 _ _ _]
                      tunnel: w1096 -> [w1102 _ _ _ _]
                      tunnel: w1095 -> [w1098 _ _ _ _]
                      tunnel: w1094 -> [w1112 _ _ _ _]
                      tunnel: w1093 -> [w1105 _ _ _ _]
                      tunnel: w1092 -> [w1100 _ _ _ _]
                      tunnel: [_ w1116 _ _ _] -> w1091
                      frame #0 {
                        w1099 = "\\"
                        n681 = local read "SET LAB04-2"() -> (w1107:T5)
                        n682 = case shown="\"CHART TEST\", Default" w1112 {
                          tunnel: ["L04-2-CHART TEST-" "L04-2-CYCLE TEST-" "L04-2-T-RISE TEST-"] -> w1108
                          frame "CHART TEST", Default {
                          }
                          frame "CYCLE TEST" {
                          }
                          frame "T-RISE TEST" {
                          }
                        }
                        n683 = Unbundle(w1107) -> ("DESCRIPTION"=w1106:string)  [unwired: 4 out]
                        n684 = Concatenate Strings(w1102, "\\", w1100, w1099, w1098, w1099) -> (w1109:string)
                        n685 = String To Path(string=w1109) -> (path=w1111:path)
                        n686 = Concatenate Strings(w1109, w1108, w1106, "-", w1105, ".tdms") -> (w1097:string)
                        n687 = Create Folder(path (use dialog)=w1111) -> (error out=w1110:errorcluster)  [unwired: 2 in, 2 out]
                        n688 = global write "Global 1.vi" "LAB04-2 FILE"(w1097) -> ()
                        n689 = call <vilib>:"Clear Errors.vi"("error in (no error)"=w1110) -> ()  [unwired: 6 in, 1 out]
                      }
                      frame #1 {
                        n690 = String To Path(string=w1122) -> (path=w1117:path)
                        n691 = TDMS Open(5:FALSE, 6:FALSE, 10:T17."create or replace" ("operation (0:open)"), 11:w1117) -> (0:w1116:errorcluster, 3:→"TDMS LAB04-2":refnum<k34>)  [unwired: 3 in]
                      }
                      frame #2 {
                        n692 = local read "SET LAB04-2"() -> (w1128:T5)
                        n693 = local read "TDMS LAB04-2"() -> (w1139:refnum<k34>)
                        n694 = Build Array("Testers Name", "Description", "Set Test Cycles", "T-Rise minutes", "T-Rise Deg C") -> (w1129:string[])
                        n695 = Unbundle(w1128) -> ("NAME"=w1127:string, "DESCRIPTION"=w1126:string, "CYCLES"=w1125:dbl, "T-RISE mins"=w1124:dbl, "T-RISE deg C"=w1123:dbl)
                        n696 = Number To Decimal String(number=w1125) -> (decimal integer string=w1138:string)  [unwired: 1 in]
                        n697 = Number To Decimal String(number=w1124) -> (decimal integer string=w1137:string)  [unwired: 1 in]
                        n698 = Number To Decimal String(number=w1123) -> (decimal integer string=w1136:string)  [unwired: 1 in]
                        n699 = Build Array(w1127, w1126, w1138, w1137, w1136) -> (w1135:string[])
                        n700 = TDMS Set Properties(5:w1135, 7:w1129, 11:w1139) -> ()  [unwired: 3 in, 4 out]
                      }
                      frame #3 {
                        w1141 = 0.0
                        n701 = local read "DISP LAB04-2"() -> (w1143:T4)
                        n702 = Bundle(cluster=w1143, "CYCLE"=w1141, "MINS"=w1141, "STATUS"="RUN") -> (w1142:T4)
                        n703 = local write "DISP LAB04-2"(w1142) -> ()
                      }
                      frame #4 {
                        n704 = local read "SIG LAB04-2"() -> (w1146:T2)
                        n705 = local read "TEMP START LAB04-2"() -> (w1148:cluster{"TL":dbl, "TN":dbl})
                        n706 = Unbundle(w1146) -> ("Tmp Live"=w1145:dbl, "Tmp Neut"=w1144:dbl)  [unwired: 3 out]
                        n707 = Bundle(cluster=w1148, "TL"=w1145, "TN"=w1144) -> (w1147:cluster{"TL":dbl, "TN":dbl})
                        n708 = local write "TEMP START LAB04-2"(w1147) -> ()
                      }
                    }
                  }
                }
              }
              event "RUN LAB05-1": Value Change {
                n709 = event-data() -> ("NewVal"=w1149:bool)  [unwired: 1 in, 5 out]
                n710 = local write "run lab05-1"(w1149) -> ()
                n711 = case shown="True" w1149 {
                  tunnel: w1155 -> [_ w1188]
                  tunnel: w1154 -> [_ w1187]
                  tunnel: w1152 -> [w1157 w1186]
                  tunnel: w1153 -> [_ w1185]
                  tunnel: w1151 -> [_ w1184]
                  tunnel: [w1156 w1183] -> w1150
                  frame False {
                    # "stop test"
                    n712 = stacked-sequence {
                      tunnel: w1157 -> [w1166 _]
                      tunnel: [w1158 _] -> w1156
                      frame #0 {
                        n713 = local read "DISP LAB05-1"() -> (w1165:T4)
                        n714 = Unbundle(w1165) -> ("CYCLE"=w1163:dbl, "MINS"=w1164:dbl)  [unwired: 1 out]
                        n715 = case shown="\"CYCLE TEST\"" w1166 {
                          tunnel: w1164 -> [_ _ w1173]
                          tunnel: w1163 -> [w1171 w1172 _]
                          tunnel: [w1171 w1172 w1173] -> w1162
                          frame "CHART TEST", Default {
                          }
                          frame "CYCLE TEST" {
                          }
                          frame "T-RISE TEST" {
                          }
                        }
                        n716 = local read "TDMS LAB05-1"() -> (w1170:refnum<k34>)
                        n717 = Build Array("STOPPED") -> (w1167:string[])
                        n718 = Build Array(w1162) -> (w1161:dbl[])
                        n719 = TDMS Write(0:w1170, 5:"TEST RESULT", 7:w1167, 9:w1161) -> (4:w1159:refnum<k34>, 15:w1160:errorcluster)  [unwired: 2 in, 2 out]
                        n720 = TDMS Close(8:w1160, 11:w1159) -> (0:w1158:errorcluster)  [unwired: 1 out]
                      }
                      frame #1 {
                        n721 = local read "DISP LAB05-1"() -> (w1177:T4)
                        n722 = stacked-sequence {
                          tunnel: "LAB05-1" -> [w1179 w1181]
                          frame #0 {
                            n723 = call "sub vi - defrag tdms v1.vi"("panel id"=w1179) -> ("error out"=w1178:errorcluster)  [unwired: 10 in]
                            n724 = local write "data file error"(w1178) -> ()
                          }
                          frame #1 {
                            n725 = call "Save data file to network drive v1.vi"("panel id"=w1181) -> ("network file save error"=w1180:errorcluster)  [unwired: 9 in, 1 out]
                            n726 = local write "RESULT LAB05-1"(FALSE) -> ()
                            n727 = local write "data file error"(w1180) -> ()
                          }
                        }
                        n728 = Bundle(cluster=w1177, "STATUS"="STOP") -> (w1175:T4)  [unwired: 2 in]
                        n729 = local write "DISP LAB05-1"(w1175) -> ()
                      }
                    }
                  }
                  frame True {
                    # "start new test and create test file"
                    n730 = stacked-sequence {
                      seq-local: [w1189 _ _ _ _] -> [_ w1214 _ _ _]
                      tunnel: w1188 -> [w1194 _ _ _ _]
                      tunnel: w1187 -> [w1190 _ _ _ _]
                      tunnel: w1186 -> [w1204 _ _ _ _]
                      tunnel: w1185 -> [w1197 _ _ _ _]
                      tunnel: w1184 -> [w1192 _ _ _ _]
                      tunnel: [_ w1208 _ _ _] -> w1183
                      frame #0 {
                        w1191 = "\\"
                        n731 = local read "SET LAB05-1"() -> (w1199:T5)
                        n732 = case shown="\"CYCLE TEST\"" w1204 {
                          tunnel: ["L05-1-CHART TEST-" "L05-1-CYCLE TEST-" "L05-1-T-RISE TEST-"] -> w1200
                          frame "CHART TEST", Default {
                          }
                          frame "CYCLE TEST" {
                          }
                          frame "T-RISE TEST" {
                          }
                        }
                        n733 = Unbundle(w1199) -> ("DESCRIPTION"=w1198:string)  [unwired: 4 out]
                        n734 = Concatenate Strings(w1194, "\\", w1192, w1191, w1190, w1191) -> (w1201:string)
                        n735 = String To Path(string=w1201) -> (path=w1203:path)
                        n736 = Concatenate Strings(w1201, w1200, w1198, "-", w1197, ".tdms") -> (w1189:string)
                        n737 = Create Folder(path (use dialog)=w1203) -> (error out=w1202:errorcluster)  [unwired: 2 in, 2 out]
                        n738 = global write "Global 1.vi" "LAB05-1 FILE"(w1189) -> ()
                        n739 = call <vilib>:"Clear Errors.vi"("error in (no error)"=w1202) -> ()  [unwired: 6 in, 1 out]
                      }
                      frame #1 {
                        n740 = String To Path(string=w1214) -> (path=w1209:path)
                        n741 = TDMS Open(5:FALSE, 6:FALSE, 10:T17."create or replace" ("operation (0:open)"), 11:w1209) -> (0:w1208:errorcluster, 3:→"TDMS LAB05-1":refnum<k34>)  [unwired: 3 in]
                      }
                      frame #2 {
                        n742 = local read "SET LAB05-1"() -> (w1220:T5)
                        n743 = local read "TDMS LAB05-1"() -> (w1231:refnum<k34>)
                        n744 = Build Array("Testers Name", "Description", "Set Test Cycles", "T-Rise minutes", "T-Rise Deg C") -> (w1221:string[])
                        n745 = Unbundle(w1220) -> ("NAME"=w1219:string, "DESCRIPTION"=w1218:string, "CYCLES"=w1217:dbl, "T-RISE mins"=w1216:dbl, "T-RISE deg C"=w1215:dbl)
                        n746 = Number To Decimal String(number=w1217) -> (decimal integer string=w1230:string)  [unwired: 1 in]
                        n747 = Number To Decimal String(number=w1216) -> (decimal integer string=w1229:string)  [unwired: 1 in]
                        n748 = Number To Decimal String(number=w1215) -> (decimal integer string=w1228:string)  [unwired: 1 in]
                        n749 = Build Array(w1219, w1218, w1230, w1229, w1228) -> (w1227:string[])
                        n750 = TDMS Set Properties(5:w1227, 7:w1221, 11:w1231) -> ()  [unwired: 3 in, 4 out]
                      }
                      frame #3 {
                        w1233 = 0.0
                        n751 = local read "DISP LAB05-1"() -> (w1235:T4)
                        n752 = Bundle(cluster=w1235, "CYCLE"=w1233, "MINS"=w1233, "STATUS"="RUN") -> (w1234:T4)
                        n753 = local write "DISP LAB05-1"(w1234) -> ()
                      }
                      frame #4 {
                        n754 = local read "SIG LAB05-1"() -> (w1238:T2)
                        n755 = local read "TEMP START LAB05-1"() -> (w1240:cluster{"TL":dbl, "TN":dbl})
                        n756 = Unbundle(w1238) -> ("Tmp Live"=w1237:dbl, "Tmp Neut"=w1236:dbl)  [unwired: 3 out]
                        n757 = Bundle(cluster=w1240, "TL"=w1237, "TN"=w1236) -> (w1239:cluster{"TL":dbl, "TN":dbl})
                        n758 = local write "TEMP START LAB05-1"(w1239) -> ()
                      }
                    }
                  }
                }
              }
              event "RUN LAB05-2": Value Change {
                n759 = event-data() -> ("NewVal"=w1241:bool)  [unwired: 1 in, 5 out]
                n760 = local write "run lab05-2"(w1241) -> ()
                n761 = case shown="True" w1241 {
                  tunnel: w1247 -> [_ w1280]
                  tunnel: w1246 -> [_ w1279]
                  tunnel: w1244 -> [w1249 w1278]
                  tunnel: w1245 -> [_ w1277]
                  tunnel: w1243 -> [_ w1276]
                  tunnel: [w1248 w1275] -> w1242
                  frame False {
                    # "stop test"
                    n762 = stacked-sequence {
                      tunnel: w1249 -> [w1258 _]
                      tunnel: [w1250 _] -> w1248
                      frame #0 {
                        n763 = local read "DISP LAB05-2"() -> (w1257:T4)
                        n764 = Unbundle(w1257) -> ("CYCLE"=w1255:dbl, "MINS"=w1256:dbl)  [unwired: 1 out]
                        n765 = case shown="\"CYCLE TEST\"" w1258 {
                          tunnel: w1256 -> [_ _ w1265]
                          tunnel: w1255 -> [w1263 w1264 _]
                          tunnel: [w1263 w1264 w1265] -> w1254
                          frame "CHART TEST", Default {
                          }
                          frame "CYCLE TEST" {
                          }
                          frame "T-RISE TEST" {
                          }
                        }
                        n766 = local read "TDMS LAB05-2"() -> (w1262:refnum<k34>)
                        n767 = Build Array("STOPPED") -> (w1259:string[])
                        n768 = Build Array(w1254) -> (w1253:dbl[])
                        n769 = TDMS Write(0:w1262, 5:"TEST RESULT", 7:w1259, 9:w1253) -> (4:w1251:refnum<k34>, 15:w1252:errorcluster)  [unwired: 2 in, 2 out]
                        n770 = TDMS Close(8:w1252, 11:w1251) -> (0:w1250:errorcluster)  [unwired: 1 out]
                      }
                      frame #1 {
                        n771 = local read "DISP LAB05-2"() -> (w1269:T4)
                        n772 = stacked-sequence {
                          tunnel: "LAB05-2" -> [w1271 w1273]
                          frame #0 {
                            n773 = call "sub vi - defrag tdms v1.vi"("panel id"=w1271) -> ("error out"=w1270:errorcluster)  [unwired: 10 in]
                            n774 = local write "data file error"(w1270) -> ()
                          }
                          frame #1 {
                            n775 = local write "RESULT LAB05-2"(FALSE) -> ()
                            n776 = call "Save data file to network drive v1.vi"("panel id"=w1273) -> ("network file save error"=w1272:errorcluster)  [unwired: 9 in, 1 out]
                            n777 = local write "data file error"(w1272) -> ()
                          }
                        }
                        n778 = Bundle(cluster=w1269, "STATUS"="STOP") -> (w1267:T4)  [unwired: 2 in]
                        n779 = local write "DISP LAB05-2"(w1267) -> ()
                      }
                    }
                  }
                  frame True {
                    # "start new test and create test file"
                    n780 = stacked-sequence {
                      seq-local: [w1281 _ _ _ _] -> [_ w1306 _ _ _]
                      tunnel: w1280 -> [w1286 _ _ _ _]
                      tunnel: w1279 -> [w1282 _ _ _ _]
                      tunnel: w1278 -> [w1296 _ _ _ _]
                      tunnel: w1277 -> [w1289 _ _ _ _]
                      tunnel: w1276 -> [w1284 _ _ _ _]
                      tunnel: [_ w1300 _ _ _] -> w1275
                      frame #0 {
                        w1283 = "\\"
                        n781 = local read "SET LAB05-2"() -> (w1291:T5)
                        n782 = case shown="\"CYCLE TEST\"" w1296 {
                          tunnel: ["L05-2-CHART TEST-" "L05-2-CYCLE TEST-" "L05-2-T-RISE TEST-"] -> w1292
                          frame "CHART TEST", Default {
                          }
                          frame "CYCLE TEST" {
                          }
                          frame "T-RISE TEST" {
                          }
                        }
                        n783 = Unbundle(w1291) -> ("DESCRIPTION"=w1290:string)  [unwired: 4 out]
                        n784 = Concatenate Strings(w1286, "\\", w1284, w1283, w1282, w1283) -> (w1293:string)
                        n785 = String To Path(string=w1293) -> (path=w1295:path)
                        n786 = Concatenate Strings(w1293, w1292, w1290, "-", w1289, ".tdms") -> (w1281:string)
                        n787 = Create Folder(path (use dialog)=w1295) -> (error out=w1294:errorcluster)  [unwired: 2 in, 2 out]
                        n788 = global write "Global 1.vi" "LAB05-2 FILE"(w1281) -> ()
                        n789 = call <vilib>:"Clear Errors.vi"("error in (no error)"=w1294) -> ()  [unwired: 6 in, 1 out]
                      }
                      frame #1 {
                        n790 = String To Path(string=w1306) -> (path=w1301:path)
                        n791 = TDMS Open(5:FALSE, 6:FALSE, 10:T17."create or replace" ("operation (0:open)"), 11:w1301) -> (0:w1300:errorcluster, 3:→"TDMS LAB05-2":refnum<k34>)  [unwired: 3 in]
                      }
                      frame #2 {
                        n792 = local read "SET LAB05-2"() -> (w1312:T5)
                        n793 = local read "TDMS LAB05-2"() -> (w1323:refnum<k34>)
                        n794 = Build Array("Testers Name", "Description", "Set Test Cycles", "T-Rise minutes", "T-Rise Deg C") -> (w1313:string[])
                        n795 = Unbundle(w1312) -> ("NAME"=w1311:string, "DESCRIPTION"=w1310:string, "CYCLES"=w1309:dbl, "T-RISE mins"=w1308:dbl, "T-RISE deg C"=w1307:dbl)
                        n796 = Number To Decimal String(number=w1309) -> (decimal integer string=w1322:string)  [unwired: 1 in]
                        n797 = Number To Decimal String(number=w1308) -> (decimal integer string=w1321:string)  [unwired: 1 in]
                        n798 = Number To Decimal String(number=w1307) -> (decimal integer string=w1320:string)  [unwired: 1 in]
                        n799 = Build Array(w1311, w1310, w1322, w1321, w1320) -> (w1319:string[])
                        n800 = TDMS Set Properties(5:w1319, 7:w1313, 11:w1323) -> ()  [unwired: 3 in, 4 out]
                      }
                      frame #3 {
                        w1325 = 0.0
                        n801 = local read "DISP LAB05-2"() -> (w1327:T4)
                        n802 = Bundle(cluster=w1327, "CYCLE"=w1325, "MINS"=w1325, "STATUS"="RUN") -> (w1326:T4)
                        n803 = local write "DISP LAB05-2"(w1326) -> ()
                      }
                      frame #4 {
                        n804 = local read "SIG LAB05-2"() -> (w1330:T2)
                        n805 = local read "TEMP START LAB05-2"() -> (w1332:cluster{"TL":dbl, "TN":dbl})
                        n806 = Unbundle(w1330) -> ("Tmp Live"=w1329:dbl, "Tmp Neut"=w1328:dbl)  [unwired: 3 out]
                        n807 = Bundle(cluster=w1332, "TL"=w1329, "TN"=w1328) -> (w1331:cluster{"TL":dbl, "TN":dbl})
                        n808 = local write "TEMP START LAB05-2"(w1331) -> ()
                      }
                    }
                  }
                }
              }
            }
            n809 = local write "data file error"(w384) -> ()
          }
          frame #4 {
            # "check if test cycles reached for cycle tests, if so then test pass"
            n810 = stacked-sequence {
              tunnel: w1352 -> [_ _ _ _ _ _ _ _ _ _]
              tunnel: w1351 -> [_ _ _ _ _ _ _ _ _ _]
              tunnel: w1350 -> [_ _ _ _ _ _ _ _ _ _]
              tunnel: w1349 -> [_ _ _ _ _ _ _ _ _ _]
              tunnel: w1348 -> [_ _ _ _ _ _ _ _ _ _]
              tunnel: w1347 -> [_ _ _ _ _ _ _ _ _ _]
              tunnel: w1346 -> [_ _ _ _ _ _ _ _ _ _]
              tunnel: w1345 -> [_ _ _ _ _ _ _ _ _ _]
              tunnel: w1344 -> [_ _ _ _ _ _ _ _ _ _]
              tunnel: w1343 -> [_ _ _ _ _ _ _ _ _ _]
              tunnel: w1342 -> [w1358 _ _ _ _ _ _ _ _ _]
              tunnel: w1341 -> [_ w1393 _ _ _ _ _ _ _ _]
              tunnel: w1340 -> [_ _ w1433 _ _ _ _ _ _ _]
              tunnel: w1339 -> [_ _ _ w1473 _ _ _ _ _ _]
              tunnel: w1338 -> [_ _ _ _ w1513 _ _ _ _ _]
              tunnel: w1337 -> [_ _ _ _ _ w1553 _ _ _ _]
              tunnel: w1336 -> [_ _ _ _ _ _ w1593 _ _ _]
              tunnel: w1335 -> [_ _ _ _ _ _ _ w1633 _ _]
              tunnel: w1334 -> [_ _ _ _ _ _ _ _ w1673 _]
              tunnel: w1333 -> [_ _ _ _ _ _ _ _ _ w1713]
              frame #0 {
                # "LAB01-1"
                n811 = Less?(x=w1358, y=2) -> (x < y?=w1356:bool)
                n812 = local read "DISP LAB01-1"() -> (w1359:T4)
                n813 = Unbundle(w1359) -> ("STATUS"=w1353:string)  [unwired: 2 out]
                n814 = Equal?(x=w1353, y="RUN") -> (x = y?=w1355:bool)
                n815 = And(x=w1355, y=w1356) -> (x .and. y?=w1354:bool)
                n816 = case shown="True" w1354 {
                  tunnel: w1359 -> [_ w1364]
                  tunnel: w1358 -> [_ w1368]
                  frame False {
                  }
                  frame True {
                    n817 = local read "SET LAB01-1"() -> (w1370:T5)
                    n818 = local read "TDMS LAB01-1"() -> (w1363:refnum<k34>)
                    n819 = Unbundle(w1370) -> ("CYCLES"=w1361:dbl, "T-RISE mins"=w1367:dbl)  [unwired: 3 out]
                    n820 = case shown="\"CYCLE TEST\"" w1368 {
                      tunnel: w1367 -> [_ _ w1377]
                      tunnel: [w1372 w1374 w1377] -> w1366
                      tunnel: w1361 -> [w1372 w1374 _]
                      tunnel: ["CHART PASS" "CYCLE PASS" "T-RISE PASS"] -> w1365
                      frame "CHART TEST", Default {
                      }
                      frame "CYCLE TEST" {
                      }
                      frame "T-RISE TEST" {
                      }
                    }
                    n821 = Unbundle(w1364) -> ("CYCLE"=w1369:dbl)  [unwired: 2 out]
                    n822 = Increment(x=w1361) -> (x+1=w1362:dbl)
                    n823 = Greater Or Equal?(x=w1369, y=w1362) -> (x >= y?=w1371:bool)
                    n824 = case shown="True" w1371 {
                      tunnel: w1366 -> [w1381 _]
                      tunnel: w1365 -> [w1380 _]
                      tunnel: w1364 -> [w1379 _]
                      tunnel: w1363 -> [w1378 _]
                      frame True {
                        n825 = stacked-sequence {
                          tunnel: w1381 -> [w1385 _]
                          tunnel: w1380 -> [w1383 w1389]
                          tunnel: w1379 -> [_ w1392]
                          tunnel: w1378 -> [w1382 _]
                          frame #0 {
                            n826 = Build Array(w1383) -> (w1386:string[])
                            n827 = Build Array(w1385) -> (w1384:dbl[])
                            n828 = TDMS Write(0:w1382, 5:"TEST PASS", 7:w1386, 9:w1384) -> (15:w1388:errorcluster)  [unwired: 2 in, 3 out]
                            n829 = local write "data file error"(w1388) -> ()
                          }
                          frame #1 {
                            n830 = Bundle(cluster=w1392, "STATUS"=w1389) -> (w1390:T4)  [unwired: 2 in]
                            n831 = local write "RESULT LAB01-1"(TRUE) -> ()
                            n832 = local write "DISP LAB01-1"(w1390) -> ()
                          }
                        }
                      }
                      frame False {
                      }
                    }
                  }
                }
              }
              frame #1 {
                # "LAB01-2"
                n833 = Less?(x=w1393, y=2) -> (x < y?=w1396:bool)
                n834 = local read "DISP LAB01-2"() -> (w1398:T4)
                n835 = Unbundle(w1398) -> ("STATUS"=w1399:string)  [unwired: 2 out]
                n836 = Equal?(x=w1399, y="RUN") -> (x = y?=w1395:bool)
                n837 = And(x=w1395, y=w1396) -> (x .and. y?=w1394:bool)
                n838 = case shown="True" w1394 {
                  tunnel: w1398 -> [_ w1404]
                  tunnel: w1393 -> [_ w1408]
                  frame False {
                  }
                  frame True {
                    n839 = local read "SET LAB01-2"() -> (w1410:T5)
                    n840 = local read "TDMS LAB01-2"() -> (w1403:refnum<k34>)
                    n841 = Unbundle(w1410) -> ("CYCLES"=w1401:dbl, "T-RISE mins"=w1407:dbl)  [unwired: 3 out]
                    n842 = case shown="\"T-RISE TEST\"" w1408 {
                      tunnel: w1407 -> [_ _ w1417]
                      tunnel: [w1412 w1414 w1417] -> w1406
                      tunnel: w1401 -> [w1412 w1414 _]
                      tunnel: ["CHART PASS" "CYCLE PASS" "T-RISE PASS"] -> w1405
                      frame "CHART TEST", Default {
                      }
                      frame "CYCLE TEST" {
                      }
                      frame "T-RISE TEST" {
                      }
                    }
                    n843 = Unbundle(w1404) -> ("CYCLE"=w1409:dbl)  [unwired: 2 out]
                    n844 = Increment(x=w1401) -> (x+1=w1402:dbl)
                    n845 = Greater Or Equal?(x=w1409, y=w1402) -> (x >= y?=w1411:bool)
                    n846 = case shown="True" w1411 {
                      tunnel: w1406 -> [w1421 _]
                      tunnel: w1405 -> [w1420 _]
                      tunnel: w1404 -> [w1419 _]
                      tunnel: w1403 -> [w1418 _]
                      frame True {
                        n847 = stacked-sequence {
                          tunnel: w1421 -> [w1425 _]
                          tunnel: w1420 -> [w1423 w1429]
                          tunnel: w1419 -> [_ w1432]
                          tunnel: w1418 -> [w1422 _]
                          frame #0 {
                            n848 = Build Array(w1423) -> (w1426:string[])
                            n849 = Build Array(w1425) -> (w1424:dbl[])
                            n850 = TDMS Write(0:w1422, 5:"TEST PASS", 7:w1426, 9:w1424) -> (15:w1428:errorcluster)  [unwired: 2 in, 3 out]
                            n851 = local write "data file error"(w1428) -> ()
                          }
                          frame #1 {
                            n852 = Bundle(cluster=w1432, "STATUS"=w1429) -> (w1430:T4)  [unwired: 2 in]
                            n853 = local write "RESULT LAB01-2"(TRUE) -> ()
                            n854 = local write "DISP LAB01-2"(w1430) -> ()
                          }
                        }
                      }
                      frame False {
                      }
                    }
                  }
                }
              }
              frame #2 {
                # "LAB02-1"
                n855 = Less?(x=w1433, y=2) -> (x < y?=w1436:bool)
                n856 = local read "DISP LAB02-1"() -> (w1438:T4)
                n857 = Unbundle(w1438) -> ("STATUS"=w1439:string)  [unwired: 2 out]
                n858 = Equal?(x=w1439, y="RUN") -> (x = y?=w1435:bool)
                n859 = And(x=w1435, y=w1436) -> (x .and. y?=w1434:bool)
                n860 = case shown="True" w1434 {
                  tunnel: w1438 -> [_ w1444]
                  tunnel: w1433 -> [_ w1448]
                  frame False {
                  }
                  frame True {
                    n861 = local read "SET LAB02-1"() -> (w1450:T5)
                    n862 = local read "TDMS LAB02-1"() -> (w1443:refnum<k34>)
                    n863 = Unbundle(w1444) -> ("CYCLE"=w1449:dbl)  [unwired: 2 out]
                    n864 = Unbundle(w1450) -> ("CYCLES"=w1441:dbl, "T-RISE mins"=w1447:dbl)  [unwired: 3 out]
                    n865 = case shown="\"T-RISE TEST\"" w1448 {
                      tunnel: w1447 -> [_ _ w1457]
                      tunnel: [w1452 w1454 w1457] -> w1446
                      tunnel: w1441 -> [w1452 w1454 _]
                      tunnel: ["CHART PASS" "CYCLE PASS" "T-RISE PASS"] -> w1445
                      frame "CHART TEST", Default {
                      }
                      frame "CYCLE TEST" {
                      }
                      frame "T-RISE TEST" {
                      }
                    }
                    n866 = Increment(x=w1441) -> (x+1=w1442:dbl)
                    n867 = Greater Or Equal?(x=w1449, y=w1442) -> (x >= y?=w1451:bool)
                    n868 = case shown="True" w1451 {
                      tunnel: w1446 -> [w1461 _]
                      tunnel: w1445 -> [w1460 _]
                      tunnel: w1444 -> [w1459 _]
                      tunnel: w1443 -> [w1458 _]
                      frame True {
                        n869 = stacked-sequence {
                          tunnel: w1461 -> [w1465 _]
                          tunnel: w1460 -> [w1463 w1469]
                          tunnel: w1459 -> [_ w1472]
                          tunnel: w1458 -> [w1462 _]
                          frame #0 {
                            n870 = Build Array(w1463) -> (w1466:string[])
                            n871 = Build Array(w1465) -> (w1464:dbl[])
                            n872 = TDMS Write(0:w1462, 5:"TEST PASS", 7:w1466, 9:w1464) -> (15:w1468:errorcluster)  [unwired: 2 in, 3 out]
                            n873 = local write "data file error"(w1468) -> ()
                          }
                          frame #1 {
                            n874 = Bundle(cluster=w1472, "STATUS"=w1469) -> (w1470:T4)  [unwired: 2 in]
                            n875 = local write "RESULT LAB02-1"(TRUE) -> ()
                            n876 = local write "DISP LAB02-1"(w1470) -> ()
                          }
                        }
                      }
                      frame False {
                      }
                    }
                  }
                }
              }
              frame #3 {
                # "LAB02-2"
                n877 = Less?(x=w1473, y=2) -> (x < y?=w1476:bool)
                n878 = local read "DISP LAB02-2"() -> (w1478:T4)
                n879 = Unbundle(w1478) -> ("STATUS"=w1479:string)  [unwired: 2 out]
                n880 = Equal?(x=w1479, y="RUN") -> (x = y?=w1475:bool)
                n881 = And(x=w1475, y=w1476) -> (x .and. y?=w1474:bool)
                n882 = case shown="True" w1474 {
                  tunnel: w1478 -> [_ w1484]
                  tunnel: w1473 -> [_ w1488]
                  frame False {
                  }
                  frame True {
                    n883 = local read "SET LAB02-2"() -> (w1490:T5)
                    n884 = local read "TDMS LAB02-2"() -> (w1483:refnum<k34>)
                    n885 = Unbundle(w1484) -> ("CYCLE"=w1489:dbl)  [unwired: 2 out]
                    n886 = Unbundle(w1490) -> ("CYCLES"=w1481:dbl, "T-RISE mins"=w1487:dbl)  [unwired: 3 out]
                    n887 = case shown="\"T-RISE TEST\"" w1488 {
                      tunnel: w1487 -> [_ _ w1497]
                      tunnel: [w1492 w1494 w1497] -> w1486
                      tunnel: w1481 -> [w1492 w1494 _]
                      tunnel: ["CHART PASS" "CYCLE PASS" "T-RISE PASS"] -> w1485
                      frame "CHART TEST", Default {
                      }
                      frame "CYCLE TEST" {
                      }
                      frame "T-RISE TEST" {
                      }
                    }
                    n888 = Increment(x=w1481) -> (x+1=w1482:dbl)
                    n889 = Greater Or Equal?(x=w1489, y=w1482) -> (x >= y?=w1491:bool)
                    n890 = case shown="True" w1491 {
                      tunnel: w1486 -> [w1501 _]
                      tunnel: w1485 -> [w1500 _]
                      tunnel: w1484 -> [w1499 _]
                      tunnel: w1483 -> [w1498 _]
                      frame True {
                        n891 = stacked-sequence {
                          tunnel: w1501 -> [w1505 _]
                          tunnel: w1500 -> [w1503 w1509]
                          tunnel: w1499 -> [_ w1512]
                          tunnel: w1498 -> [w1502 _]
                          frame #0 {
                            n892 = Build Array(w1503) -> (w1506:string[])
                            n893 = Build Array(w1505) -> (w1504:dbl[])
                            n894 = TDMS Write(0:w1502, 5:"TEST PASS", 7:w1506, 9:w1504) -> (15:w1508:errorcluster)  [unwired: 2 in, 3 out]
                            n895 = local write "data file error"(w1508) -> ()
                          }
                          frame #1 {
                            n896 = Bundle(cluster=w1512, "STATUS"=w1509) -> (w1510:T4)  [unwired: 2 in]
                            n897 = local write "RESULT LAB02-2"(TRUE) -> ()
                            n898 = local write "DISP LAB02-2"(w1510) -> ()
                          }
                        }
                      }
                      frame False {
                      }
                    }
                  }
                }
              }
              frame #4 {
                # "LAB03-1"
                n899 = Less?(x=w1513, y=2) -> (x < y?=w1516:bool)
                n900 = local read "DISP LAB03-1"() -> (w1518:T4)
                n901 = Unbundle(w1518) -> ("STATUS"=w1519:string)  [unwired: 2 out]
                n902 = Equal?(x=w1519, y="RUN") -> (x = y?=w1515:bool)
                n903 = And(x=w1515, y=w1516) -> (x .and. y?=w1514:bool)
                n904 = case shown="True" w1514 {
                  tunnel: w1518 -> [_ w1524]
                  tunnel: w1513 -> [_ w1528]
                  frame False {
                  }
                  frame True {
                    n905 = local read "SET LAB03-1"() -> (w1530:T5)
                    n906 = local read "TDMS LAB03-1"() -> (w1523:refnum<k34>)
                    n907 = Unbundle(w1524) -> ("CYCLE"=w1529:dbl)  [unwired: 2 out]
                    n908 = Unbundle(w1530) -> ("CYCLES"=w1521:dbl, "T-RISE mins"=w1527:dbl)  [unwired: 3 out]
                    n909 = case shown="\"T-RISE TEST\"" w1528 {
                      tunnel: w1527 -> [_ _ w1537]
                      tunnel: [w1532 w1534 w1537] -> w1526
                      tunnel: w1521 -> [w1532 w1534 _]
                      tunnel: ["CHART PASS" "CYCLE PASS" "T-RISE PASS"] -> w1525
                      frame "CHART TEST", Default {
                      }
                      frame "CYCLE TEST" {
                      }
                      frame "T-RISE TEST" {
                      }
                    }
                    n910 = Increment(x=w1521) -> (x+1=w1522:dbl)
                    n911 = Greater Or Equal?(x=w1529, y=w1522) -> (x >= y?=w1531:bool)
                    n912 = case shown="True" w1531 {
                      tunnel: w1526 -> [w1541 _]
                      tunnel: w1525 -> [w1540 _]
                      tunnel: w1524 -> [w1539 _]
                      tunnel: w1523 -> [w1538 _]
                      frame True {
                        n913 = stacked-sequence {
                          tunnel: w1541 -> [w1545 _]
                          tunnel: w1540 -> [w1543 w1549]
                          tunnel: w1539 -> [_ w1552]
                          tunnel: w1538 -> [w1542 _]
                          frame #0 {
                            n914 = Build Array(w1543) -> (w1546:string[])
                            n915 = Build Array(w1545) -> (w1544:dbl[])
                            n916 = TDMS Write(0:w1542, 5:"TEST PASS", 7:w1546, 9:w1544) -> (15:w1548:errorcluster)  [unwired: 2 in, 3 out]
                            n917 = local write "data file error"(w1548) -> ()
                          }
                          frame #1 {
                            n918 = Bundle(cluster=w1552, "STATUS"=w1549) -> (w1550:T4)  [unwired: 2 in]
                            n919 = local write "RESULT LAB03-1"(TRUE) -> ()
                            n920 = local write "DISP LAB03-1"(w1550) -> ()
                          }
                        }
                      }
                      frame False {
                      }
                    }
                  }
                }
              }
              frame #5 {
                # "LAB03-2"
                n921 = Less?(x=w1553, y=2) -> (x < y?=w1556:bool)
                n922 = local read "DISP LAB03-2"() -> (w1558:T4)
                n923 = Unbundle(w1558) -> ("STATUS"=w1559:string)  [unwired: 2 out]
                n924 = Equal?(x=w1559, y="RUN") -> (x = y?=w1555:bool)
                n925 = And(x=w1555, y=w1556) -> (x .and. y?=w1554:bool)
                n926 = case shown="True" w1554 {
                  tunnel: w1558 -> [_ w1564]
                  tunnel: w1553 -> [_ w1568]
                  frame False {
                  }
                  frame True {
                    n927 = local read "SET LAB03-2"() -> (w1570:T5)
                    n928 = local read "TDMS LAB03-2"() -> (w1563:refnum<k34>)
                    n929 = Unbundle(w1564) -> ("CYCLE"=w1569:dbl)  [unwired: 2 out]
                    n930 = Unbundle(w1570) -> ("CYCLES"=w1561:dbl, "T-RISE mins"=w1567:dbl)  [unwired: 3 out]
                    n931 = case shown="\"T-RISE TEST\"" w1568 {
                      tunnel: w1567 -> [_ _ w1577]
                      tunnel: [w1572 w1574 w1577] -> w1566
                      tunnel: w1561 -> [w1572 w1574 _]
                      tunnel: ["CHART PASS" "CYCLE PASS" "T-RISE PASS"] -> w1565
                      frame "CHART TEST", Default {
                      }
                      frame "CYCLE TEST" {
                      }
                      frame "T-RISE TEST" {
                      }
                    }
                    n932 = Increment(x=w1561) -> (x+1=w1562:dbl)
                    n933 = Greater Or Equal?(x=w1569, y=w1562) -> (x >= y?=w1571:bool)
                    n934 = case shown="True" w1571 {
                      tunnel: w1566 -> [w1581 _]
                      tunnel: w1565 -> [w1580 _]
                      tunnel: w1564 -> [w1579 _]
                      tunnel: w1563 -> [w1578 _]
                      frame True {
                        n935 = stacked-sequence {
                          tunnel: w1581 -> [w1585 _]
                          tunnel: w1580 -> [w1583 w1589]
                          tunnel: w1579 -> [_ w1592]
                          tunnel: w1578 -> [w1582 _]
                          frame #0 {
                            n936 = Build Array(w1583) -> (w1586:string[])
                            n937 = Build Array(w1585) -> (w1584:dbl[])
                            n938 = TDMS Write(0:w1582, 5:"TEST PASS", 7:w1586, 9:w1584) -> (15:w1588:errorcluster)  [unwired: 2 in, 3 out]
                            n939 = local write "data file error"(w1588) -> ()
                          }
                          frame #1 {
                            n940 = Bundle(cluster=w1592, "STATUS"=w1589) -> (w1590:T4)  [unwired: 2 in]
                            n941 = local write "RESULT LAB03-2"(TRUE) -> ()
                            n942 = local write "DISP LAB03-2"(w1590) -> ()
                          }
                        }
                      }
                      frame False {
                      }
                    }
                  }
                }
              }
              frame #6 {
                # "LAB04-1"
                n943 = Less?(x=w1593, y=2) -> (x < y?=w1596:bool)
                n944 = local read "DISP LAB04-1"() -> (w1598:T4)
                n945 = Unbundle(w1598) -> ("STATUS"=w1599:string)  [unwired: 2 out]
                n946 = Equal?(x=w1599, y="RUN") -> (x = y?=w1595:bool)
                n947 = And(x=w1595, y=w1596) -> (x .and. y?=w1594:bool)
                n948 = case shown="True" w1594 {
                  tunnel: w1598 -> [_ w1604]
                  tunnel: w1593 -> [_ w1608]
                  frame False {
                  }
                  frame True {
                    n949 = local read "SET LAB04-1"() -> (w1610:T5)
                    n950 = local read "TDMS LAB04-1"() -> (w1603:refnum<k34>)
                    n951 = Unbundle(w1604) -> ("CYCLE"=w1609:dbl)  [unwired: 2 out]
                    n952 = Unbundle(w1610) -> ("CYCLES"=w1601:dbl, "T-RISE mins"=w1607:dbl)  [unwired: 3 out]
                    n953 = case shown="\"T-RISE TEST\"" w1608 {
                      tunnel: w1607 -> [_ _ w1617]
                      tunnel: [w1612 w1614 w1617] -> w1606
                      tunnel: w1601 -> [w1612 w1614 _]
                      tunnel: ["CHART PASS" "CYCLE PASS" "T-RISE PASS"] -> w1605
                      frame "CHART TEST", Default {
                      }
                      frame "CYCLE TEST" {
                      }
                      frame "T-RISE TEST" {
                      }
                    }
                    n954 = Increment(x=w1601) -> (x+1=w1602:dbl)
                    n955 = Greater Or Equal?(x=w1609, y=w1602) -> (x >= y?=w1611:bool)
                    n956 = case shown="True" w1611 {
                      tunnel: w1606 -> [w1621 _]
                      tunnel: w1605 -> [w1620 _]
                      tunnel: w1604 -> [w1619 _]
                      tunnel: w1603 -> [w1618 _]
                      frame True {
                        n957 = stacked-sequence {
                          tunnel: w1621 -> [w1625 _]
                          tunnel: w1620 -> [w1623 w1629]
                          tunnel: w1619 -> [_ w1632]
                          tunnel: w1618 -> [w1622 _]
                          frame #0 {
                            n958 = Build Array(w1623) -> (w1626:string[])
                            n959 = Build Array(w1625) -> (w1624:dbl[])
                            n960 = TDMS Write(0:w1622, 5:"TEST PASS", 7:w1626, 9:w1624) -> (15:w1628:errorcluster)  [unwired: 2 in, 3 out]
                            n961 = local write "data file error"(w1628) -> ()
                          }
                          frame #1 {
                            n962 = Bundle(cluster=w1632, "STATUS"=w1629) -> (w1630:T4)  [unwired: 2 in]
                            n963 = local write "RESULT LAB04-1"(TRUE) -> ()
                            n964 = local write "DISP LAB04-1"(w1630) -> ()
                          }
                        }
                      }
                      frame False {
                      }
                    }
                  }
                }
              }
              frame #7 {
                # "LAB04-2"
                n965 = Less?(x=w1633, y=2) -> (x < y?=w1636:bool)
                n966 = local read "DISP LAB04-2"() -> (w1638:T4)
                n967 = Unbundle(w1638) -> ("STATUS"=w1639:string)  [unwired: 2 out]
                n968 = Equal?(x=w1639, y="RUN") -> (x = y?=w1635:bool)
                n969 = And(x=w1635, y=w1636) -> (x .and. y?=w1634:bool)
                n970 = case shown="True" w1634 {
                  tunnel: w1638 -> [_ w1644]
                  tunnel: w1633 -> [_ w1648]
                  frame False {
                  }
                  frame True {
                    n971 = local read "SET LAB04-2"() -> (w1650:T5)
                    n972 = local read "TDMS LAB04-2"() -> (w1643:refnum<k34>)
                    n973 = Unbundle(w1644) -> ("CYCLE"=w1649:dbl)  [unwired: 2 out]
                    n974 = Unbundle(w1650) -> ("CYCLES"=w1641:dbl, "T-RISE mins"=w1647:dbl)  [unwired: 3 out]
                    n975 = case shown="\"T-RISE TEST\"" w1648 {
                      tunnel: w1647 -> [_ _ w1657]
                      tunnel: [w1652 w1654 w1657] -> w1646
                      tunnel: w1641 -> [w1652 w1654 _]
                      tunnel: ["CHART PASS" "CYCLE PASS" "T-RISE PASS"] -> w1645
                      frame "CHART TEST", Default {
                      }
                      frame "CYCLE TEST" {
                      }
                      frame "T-RISE TEST" {
                      }
                    }
                    n976 = Increment(x=w1641) -> (x+1=w1642:dbl)
                    n977 = Greater Or Equal?(x=w1649, y=w1642) -> (x >= y?=w1651:bool)
                    n978 = case shown="True" w1651 {
                      tunnel: w1646 -> [w1661 _]
                      tunnel: w1645 -> [w1660 _]
                      tunnel: w1644 -> [w1659 _]
                      tunnel: w1643 -> [w1658 _]
                      frame True {
                        n979 = stacked-sequence {
                          tunnel: w1661 -> [w1665 _]
                          tunnel: w1660 -> [w1663 w1669]
                          tunnel: w1659 -> [_ w1672]
                          tunnel: w1658 -> [w1662 _]
                          frame #0 {
                            n980 = Build Array(w1663) -> (w1666:string[])
                            n981 = Build Array(w1665) -> (w1664:dbl[])
                            n982 = TDMS Write(0:w1662, 5:"TEST PASS", 7:w1666, 9:w1664) -> (15:w1668:errorcluster)  [unwired: 2 in, 3 out]
                            n983 = local write "data file error"(w1668) -> ()
                          }
                          frame #1 {
                            n984 = Bundle(cluster=w1672, "STATUS"=w1669) -> (w1670:T4)  [unwired: 2 in]
                            n985 = local write "RESULT LAB04-2"(TRUE) -> ()
                            n986 = local write "DISP LAB04-2"(w1670) -> ()
                          }
                        }
                      }
                      frame False {
                      }
                    }
                  }
                }
              }
              frame #8 {
                # "LAB05-1"
                n987 = Less?(x=w1673, y=2) -> (x < y?=w1676:bool)
                n988 = local read "DISP LAB05-1"() -> (w1678:T4)
                n989 = Unbundle(w1678) -> ("STATUS"=w1679:string)  [unwired: 2 out]
                n990 = Equal?(x=w1679, y="RUN") -> (x = y?=w1675:bool)
                n991 = And(x=w1675, y=w1676) -> (x .and. y?=w1674:bool)
                n992 = case shown="True" w1674 {
                  tunnel: w1678 -> [_ w1684]
                  tunnel: w1673 -> [_ w1688]
                  frame False {
                  }
                  frame True {
                    n993 = local read "SET LAB05-1"() -> (w1690:T5)
                    n994 = local read "TDMS LAB05-1"() -> (w1683:refnum<k34>)
                    n995 = Unbundle(w1684) -> ("CYCLE"=w1689:dbl)  [unwired: 2 out]
                    n996 = Unbundle(w1690) -> ("CYCLES"=w1681:dbl, "T-RISE mins"=w1687:dbl)  [unwired: 3 out]
                    n997 = case shown="\"T-RISE TEST\"" w1688 {
                      tunnel: w1687 -> [_ _ w1697]
                      tunnel: [w1692 w1694 w1697] -> w1686
                      tunnel: w1681 -> [w1692 w1694 _]
                      tunnel: ["CHART PASS" "CYCLE PASS" "T-RISE PASS"] -> w1685
                      frame "CHART TEST", Default {
                      }
                      frame "CYCLE TEST" {
                      }
                      frame "T-RISE TEST" {
                      }
                    }
                    n998 = Increment(x=w1681) -> (x+1=w1682:dbl)
                    n999 = Greater Or Equal?(x=w1689, y=w1682) -> (x >= y?=w1691:bool)
                    n1000 = case shown="True" w1691 {
                      tunnel: w1686 -> [w1701 _]
                      tunnel: w1685 -> [w1700 _]
                      tunnel: w1684 -> [w1699 _]
                      tunnel: w1683 -> [w1698 _]
                      frame True {
                        n1001 = stacked-sequence {
                          tunnel: w1701 -> [w1705 _]
                          tunnel: w1700 -> [w1703 w1709]
                          tunnel: w1699 -> [_ w1712]
                          tunnel: w1698 -> [w1702 _]
                          frame #0 {
                            n1002 = Build Array(w1703) -> (w1706:string[])
                            n1003 = Build Array(w1705) -> (w1704:dbl[])
                            n1004 = TDMS Write(0:w1702, 5:"TEST PASS", 7:w1706, 9:w1704) -> (15:w1708:errorcluster)  [unwired: 2 in, 3 out]
                            n1005 = local write "data file error"(w1708) -> ()
                          }
                          frame #1 {
                            n1006 = Bundle(cluster=w1712, "STATUS"=w1709) -> (w1710:T4)  [unwired: 2 in]
                            n1007 = local write "RESULT LAB05-1"(TRUE) -> ()
                            n1008 = local write "DISP LAB05-1"(w1710) -> ()
                          }
                        }
                      }
                      frame False {
                      }
                    }
                  }
                }
              }
              frame #9 {
                # "LAB05-2"
                n1009 = Less?(x=w1713, y=2) -> (x < y?=w1716:bool)
                n1010 = local read "DISP LAB05-2"() -> (w1718:T4)
                n1011 = Unbundle(w1718) -> ("STATUS"=w1719:string)  [unwired: 2 out]
                n1012 = Equal?(x=w1719, y="RUN") -> (x = y?=w1715:bool)
                n1013 = And(x=w1715, y=w1716) -> (x .and. y?=w1714:bool)
                n1014 = case shown="True" w1714 {
                  tunnel: w1718 -> [_ w1724]
                  tunnel: w1713 -> [_ w1728]
                  frame False {
                  }
                  frame True {
                    n1015 = local read "SET LAB05-2"() -> (w1730:T5)
                    n1016 = local read "TDMS LAB05-2"() -> (w1723:refnum<k34>)
                    n1017 = Unbundle(w1724) -> ("CYCLE"=w1729:dbl)  [unwired: 2 out]
                    n1018 = Unbundle(w1730) -> ("CYCLES"=w1721:dbl, "T-RISE mins"=w1727:dbl)  [unwired: 3 out]
                    n1019 = case shown="\"T-RISE TEST\"" w1728 {
                      tunnel: w1727 -> [_ _ w1737]
                      tunnel: [w1732 w1734 w1737] -> w1726
                      tunnel: w1721 -> [w1732 w1734 _]
                      tunnel: ["CHART PASS" "CYCLE PASS" "T-RISE PASS"] -> w1725
                      frame "CHART TEST", Default {
                      }
                      frame "CYCLE TEST" {
                      }
                      frame "T-RISE TEST" {
                      }
                    }
                    n1020 = Increment(x=w1721) -> (x+1=w1722:dbl)
                    n1021 = Greater Or Equal?(x=w1729, y=w1722) -> (x >= y?=w1731:bool)
                    n1022 = case shown="True" w1731 {
                      tunnel: w1726 -> [w1741 _]
                      tunnel: w1725 -> [w1740 _]
                      tunnel: w1724 -> [w1739 _]
                      tunnel: w1723 -> [w1738 _]
                      frame True {
                        n1023 = stacked-sequence {
                          tunnel: w1741 -> [w1745 _]
                          tunnel: w1740 -> [w1743 w1749]
                          tunnel: w1739 -> [_ w1752]
                          tunnel: w1738 -> [w1742 _]
                          frame #0 {
                            n1024 = Build Array(w1743) -> (w1746:string[])
                            n1025 = Build Array(w1745) -> (w1744:dbl[])
                            n1026 = TDMS Write(0:w1742, 5:"TEST PASS", 7:w1746, 9:w1744) -> (15:w1748:errorcluster)  [unwired: 2 in, 3 out]
                            n1027 = local write "data file error"(w1748) -> ()
                          }
                          frame #1 {
                            n1028 = Bundle(cluster=w1752, "STATUS"=w1749) -> (w1750:T4)  [unwired: 2 in]
                            n1029 = local write "RESULT LAB05-2"(TRUE) -> ()
                            n1030 = local write "DISP LAB05-2"(w1750) -> ()
                          }
                        }
                      }
                      frame False {
                      }
                    }
                  }
                }
              }
            }
          }
          frame #5 {
            # "check if test cycles reached for temperature rise test"
            n1031 = stacked-sequence {
              tunnel: w1782 -> [_ _ _ _ _ _ _ _ _ _]
              tunnel: w1781 -> [_ _ _ _ _ _ _ _ _ _]
              tunnel: w1780 -> [_ _ _ _ _ _ _ _ _ _]
              tunnel: w1779 -> [_ _ _ _ _ _ _ _ _ _]
              tunnel: w1778 -> [_ _ _ _ _ _ _ _ _ _]
              tunnel: w1777 -> [_ _ _ _ _ _ _ _ _ _]
              tunnel: w1776 -> [_ _ _ _ _ _ _ _ _ _]
              tunnel: w1775 -> [_ _ _ _ _ _ _ _ _ _]
              tunnel: w1774 -> [_ _ _ _ _ _ _ _ _ _]
              tunnel: w1773 -> [_ _ _ _ _ _ _ _ _ _]
              tunnel: w1772 -> [w1788 _ _ _ _ _ _ _ _ _]
              tunnel: w1762 -> [w1783 _ _ _ _ _ _ _ _ _]
              tunnel: w1771 -> [_ w1814 _ _ _ _ _ _ _ _]
              tunnel: w1770 -> [_ _ w1844 _ _ _ _ _ _ _]
              tunnel: w1769 -> [_ _ _ w1874 _ _ _ _ _ _]
              tunnel: w1768 -> [_ _ _ _ w1904 _ _ _ _ _]
              tunnel: w1767 -> [_ _ _ _ _ w1934 _ _ _ _]
              tunnel: w1766 -> [_ _ _ _ _ _ w1964 _ _ _]
              tunnel: w1765 -> [_ _ _ _ _ _ _ w1994 _ _]
              tunnel: w1764 -> [_ _ _ _ _ _ _ _ w2024 _]
              tunnel: w1763 -> [_ _ _ _ _ _ _ _ _ w2054]
              tunnel: w1761 -> [_ w1813 _ _ _ _ _ _ _ _]
              tunnel: w1760 -> [_ _ w1843 _ _ _ _ _ _ _]
              tunnel: w1759 -> [_ _ _ w1873 _ _ _ _ _ _]
              tunnel: w1758 -> [_ _ _ _ w1903 _ _ _ _ _]
              tunnel: w1757 -> [_ _ _ _ _ w1933 _ _ _ _]
              tunnel: w1756 -> [_ _ _ _ _ _ w1963 _ _ _]
              tunnel: w1755 -> [_ _ _ _ _ _ _ w1993 _ _]
              tunnel: w1754 -> [_ _ _ _ _ _ _ _ w2023 _]
              tunnel: w1753 -> [_ _ _ _ _ _ _ _ _ w2053]
              frame #0 {
                # "LAB01-1"
                n1032 = Equal?(x=w1788, y=2) -> (x = y?=w1786:bool)
                n1033 = local read "DISP LAB01-1"() -> (w1789:T4)
                n1034 = Unbundle(w1789) -> ("STATUS"=w1790:string)  [unwired: 2 out]
                n1035 = Equal?(x=w1790, y="RUN") -> (x = y?=w1785:bool)
                n1036 = And(x=w1785, y=w1786) -> (x .and. y?=w1784:bool)
                n1037 = case shown="True" w1784 {
                  tunnel: w1789 -> [_ w1793]
                  tunnel: w1783 -> [_ w1796]
                  frame False {
                  }
                  frame True {
                    n1038 = local read "SET LAB01-1"() -> (w1795:T5)
                    n1039 = local read "TDMS LAB01-1"() -> (w1792:refnum<k34>)
                    n1040 = Unbundle(w1793) -> ("CYCLE"=w1797:dbl)  [unwired: 2 out]
                    n1041 = Unbundle(w1795) -> ("T-RISE mins"=w1794:dbl)  [unwired: 4 out]
                    n1042 = Greater Or Equal?(x=w1797, y=w1796) -> (x >= y?=w1798:bool)
                    n1043 = case shown="True" w1798 {
                      tunnel: w1794 -> [w1801 _]
                      tunnel: w1793 -> [w1800 _]
                      tunnel: w1792 -> [w1799 _]
                      frame True {
                        n1044 = stacked-sequence {
                          tunnel: w1801 -> [w1804 _]
                          tunnel: w1800 -> [_ w1809]
                          tunnel: w1799 -> [w1802 _]
                          frame #0 {
                            n1045 = Build Array("T-RISE") -> (w1806:string[])
                            n1046 = Build Array(w1804) -> (w1805:dbl[])
                            n1047 = TDMS Write(0:w1802, 5:"TEST PASS", 7:w1806, 9:w1805) -> (15:w1808:errorcluster)  [unwired: 2 in, 3 out]
                            n1048 = local write "data file error"(w1808) -> ()
                          }
                          frame #1 {
                            n1049 = Bundle(cluster=w1809, "STATUS"="T-RISE PASS") -> (w1811:T4)  [unwired: 2 in]
                            n1050 = local write "RESULT LAB01-1"(TRUE) -> ()
                            n1051 = local write "DISP LAB01-1"(w1811) -> ()
                          }
                        }
                      }
                      frame False {
                      }
                    }
                  }
                }
              }
              frame #1 {
                # "LAB01-2"
                n1052 = Equal?(x=w1814, y=2) -> (x = y?=w1817:bool)
                n1053 = local read "DISP LAB01-2"() -> (w1819:T4)
                n1054 = Unbundle(w1819) -> ("STATUS"=w1820:string)  [unwired: 2 out]
                n1055 = Equal?(x=w1820, y="RUN") -> (x = y?=w1816:bool)
                n1056 = And(x=w1816, y=w1817) -> (x .and. y?=w1815:bool)
                n1057 = case shown="True" w1815 {
                  tunnel: w1819 -> [_ w1823]
                  tunnel: w1813 -> [_ w1826]
                  frame False {
                  }
                  frame True {
                    n1058 = local read "SET LAB01-2"() -> (w1825:T5)
                    n1059 = local read "TDMS LAB01-2"() -> (w1822:refnum<k34>)
                    n1060 = Unbundle(w1823) -> ("CYCLE"=w1827:dbl)  [unwired: 2 out]
                    n1061 = Unbundle(w1825) -> ("T-RISE mins"=w1824:dbl)  [unwired: 4 out]
                    n1062 = Greater Or Equal?(x=w1827, y=w1826) -> (x >= y?=w1828:bool)
                    n1063 = case shown="True" w1828 {
                      tunnel: w1824 -> [w1831 _]
                      tunnel: w1823 -> [w1830 _]
                      tunnel: w1822 -> [w1829 _]
                      frame True {
                        n1064 = stacked-sequence {
                          tunnel: w1831 -> [w1834 _]
                          tunnel: w1830 -> [_ w1839]
                          tunnel: w1829 -> [w1832 _]
                          frame #0 {
                            n1065 = Build Array("T-RISE") -> (w1836:string[])
                            n1066 = Build Array(w1834) -> (w1835:dbl[])
                            n1067 = TDMS Write(0:w1832, 5:"TEST PASS", 7:w1836, 9:w1835) -> (15:w1838:errorcluster)  [unwired: 2 in, 3 out]
                            n1068 = local write "data file error"(w1838) -> ()
                          }
                          frame #1 {
                            n1069 = Bundle(cluster=w1839, "STATUS"="T-RISE PASS") -> (w1841:T4)  [unwired: 2 in]
                            n1070 = local write "RESULT LAB01-2"(TRUE) -> ()
                            n1071 = local write "DISP LAB01-2"(w1841) -> ()
                          }
                        }
                      }
                      frame False {
                      }
                    }
                  }
                }
              }
              frame #2 {
                # "LAB02-1"
                n1072 = Equal?(x=w1844, y=2) -> (x = y?=w1847:bool)
                n1073 = local read "DISP LAB02-1"() -> (w1849:T4)
                n1074 = Unbundle(w1849) -> ("STATUS"=w1850:string)  [unwired: 2 out]
                n1075 = Equal?(x=w1850, y="RUN") -> (x = y?=w1846:bool)
                n1076 = And(x=w1846, y=w1847) -> (x .and. y?=w1845:bool)
                n1077 = case shown="True" w1845 {
                  tunnel: w1849 -> [_ w1853]
                  tunnel: w1843 -> [_ w1856]
                  frame False {
                  }
                  frame True {
                    n1078 = local read "SET LAB02-1"() -> (w1855:T5)
                    n1079 = local read "TDMS LAB02-1"() -> (w1852:refnum<k34>)
                    n1080 = Unbundle(w1853) -> ("CYCLE"=w1857:dbl)  [unwired: 2 out]
                    n1081 = Unbundle(w1855) -> ("T-RISE mins"=w1854:dbl)  [unwired: 4 out]
                    n1082 = Greater Or Equal?(x=w1857, y=w1856) -> (x >= y?=w1858:bool)
                    n1083 = case shown="True" w1858 {
                      tunnel: w1854 -> [w1861 _]
                      tunnel: w1853 -> [w1860 _]
                      tunnel: w1852 -> [w1859 _]
                      frame True {
                        n1084 = stacked-sequence {
                          tunnel: w1861 -> [w1864 _]
                          tunnel: w1860 -> [_ w1869]
                          tunnel: w1859 -> [w1862 _]
                          frame #0 {
                            n1085 = Build Array("T-RISE") -> (w1866:string[])
                            n1086 = Build Array(w1864) -> (w1865:dbl[])
                            n1087 = TDMS Write(0:w1862, 5:"TEST PASS", 7:w1866, 9:w1865) -> (15:w1868:errorcluster)  [unwired: 2 in, 3 out]
                            n1088 = local write "data file error"(w1868) -> ()
                          }
                          frame #1 {
                            n1089 = Bundle(cluster=w1869, "STATUS"="T-RISE PASS") -> (w1871:T4)  [unwired: 2 in]
                            n1090 = local write "RESULT LAB02-1"(TRUE) -> ()
                            n1091 = local write "DISP LAB02-1"(w1871) -> ()
                          }
                        }
                      }
                      frame False {
                      }
                    }
                  }
                }
              }
              frame #3 {
                # "LAB02-2"
                n1092 = Equal?(x=w1874, y=2) -> (x = y?=w1877:bool)
                n1093 = local read "DISP LAB02-2"() -> (w1879:T4)
                n1094 = Unbundle(w1879) -> ("STATUS"=w1880:string)  [unwired: 2 out]
                n1095 = Equal?(x=w1880, y="RUN") -> (x = y?=w1876:bool)
                n1096 = And(x=w1876, y=w1877) -> (x .and. y?=w1875:bool)
                n1097 = case shown="True" w1875 {
                  tunnel: w1879 -> [_ w1883]
                  tunnel: w1873 -> [_ w1886]
                  frame False {
                  }
                  frame True {
                    n1098 = local read "SET LAB02-2"() -> (w1885:T5)
                    n1099 = local read "TDMS LAB02-2"() -> (w1882:refnum<k34>)
                    n1100 = Unbundle(w1883) -> ("CYCLE"=w1887:dbl)  [unwired: 2 out]
                    n1101 = Unbundle(w1885) -> ("T-RISE mins"=w1884:dbl)  [unwired: 4 out]
                    n1102 = Greater Or Equal?(x=w1887, y=w1886) -> (x >= y?=w1888:bool)
                    n1103 = case shown="True" w1888 {
                      tunnel: w1884 -> [w1891 _]
                      tunnel: w1883 -> [w1890 _]
                      tunnel: w1882 -> [w1889 _]
                      frame True {
                        n1104 = stacked-sequence {
                          tunnel: w1891 -> [w1894 _]
                          tunnel: w1890 -> [_ w1899]
                          tunnel: w1889 -> [w1892 _]
                          frame #0 {
                            n1105 = Build Array("T-RISE") -> (w1896:string[])
                            n1106 = Build Array(w1894) -> (w1895:dbl[])
                            n1107 = TDMS Write(0:w1892, 5:"TEST PASS", 7:w1896, 9:w1895) -> (15:w1898:errorcluster)  [unwired: 2 in, 3 out]
                            n1108 = local write "data file error"(w1898) -> ()
                          }
                          frame #1 {
                            n1109 = Bundle(cluster=w1899, "STATUS"="T-RISE PASS") -> (w1901:T4)  [unwired: 2 in]
                            n1110 = local write "RESULT LAB02-2"(TRUE) -> ()
                            n1111 = local write "DISP LAB02-2"(w1901) -> ()
                          }
                        }
                      }
                      frame False {
                      }
                    }
                  }
                }
              }
              frame #4 {
                # "LAB03-1"
                n1112 = Equal?(x=w1904, y=2) -> (x = y?=w1907:bool)
                n1113 = local read "DISP LAB03-1"() -> (w1909:T4)
                n1114 = Unbundle(w1909) -> ("STATUS"=w1910:string)  [unwired: 2 out]
                n1115 = Equal?(x=w1910, y="RUN") -> (x = y?=w1906:bool)
                n1116 = And(x=w1906, y=w1907) -> (x .and. y?=w1905:bool)
                n1117 = case shown="True" w1905 {
                  tunnel: w1909 -> [_ w1913]
                  tunnel: w1903 -> [_ w1916]
                  frame False {
                  }
                  frame True {
                    n1118 = local read "SET LAB03-1"() -> (w1915:T5)
                    n1119 = local read "TDMS LAB03-1"() -> (w1912:refnum<k34>)
                    n1120 = Unbundle(w1913) -> ("CYCLE"=w1917:dbl)  [unwired: 2 out]
                    n1121 = Unbundle(w1915) -> ("T-RISE mins"=w1914:dbl)  [unwired: 4 out]
                    n1122 = Greater Or Equal?(x=w1917, y=w1916) -> (x >= y?=w1918:bool)
                    n1123 = case shown="True" w1918 {
                      tunnel: w1914 -> [w1921 _]
                      tunnel: w1913 -> [w1920 _]
                      tunnel: w1912 -> [w1919 _]
                      frame True {
                        n1124 = stacked-sequence {
                          tunnel: w1921 -> [w1924 _]
                          tunnel: w1920 -> [_ w1929]
                          tunnel: w1919 -> [w1922 _]
                          frame #0 {
                            n1125 = Build Array("T-RISE") -> (w1926:string[])
                            n1126 = Build Array(w1924) -> (w1925:dbl[])
                            n1127 = TDMS Write(0:w1922, 5:"TEST PASS", 7:w1926, 9:w1925) -> (15:w1928:errorcluster)  [unwired: 2 in, 3 out]
                            n1128 = local write "data file error"(w1928) -> ()
                          }
                          frame #1 {
                            n1129 = Bundle(cluster=w1929, "STATUS"="T-RISE PASS") -> (w1931:T4)  [unwired: 2 in]
                            n1130 = local write "RESULT LAB03-1"(TRUE) -> ()
                            n1131 = local write "DISP LAB03-1"(w1931) -> ()
                          }
                        }
                      }
                      frame False {
                      }
                    }
                  }
                }
              }
              frame #5 {
                # "LAB03-2"
                n1132 = Equal?(x=w1934, y=2) -> (x = y?=w1937:bool)
                n1133 = local read "DISP LAB03-2"() -> (w1939:T4)
                n1134 = Unbundle(w1939) -> ("STATUS"=w1940:string)  [unwired: 2 out]
                n1135 = Equal?(x=w1940, y="RUN") -> (x = y?=w1936:bool)
                n1136 = And(x=w1936, y=w1937) -> (x .and. y?=w1935:bool)
                n1137 = case shown="True" w1935 {
                  tunnel: w1939 -> [_ w1943]
                  tunnel: w1933 -> [_ w1946]
                  frame False {
                  }
                  frame True {
                    n1138 = local read "SET LAB03-2"() -> (w1945:T5)
                    n1139 = local read "TDMS LAB03-2"() -> (w1942:refnum<k34>)
                    n1140 = Unbundle(w1943) -> ("CYCLE"=w1947:dbl)  [unwired: 2 out]
                    n1141 = Unbundle(w1945) -> ("T-RISE mins"=w1944:dbl)  [unwired: 4 out]
                    n1142 = Greater Or Equal?(x=w1947, y=w1946) -> (x >= y?=w1948:bool)
                    n1143 = case shown="True" w1948 {
                      tunnel: w1944 -> [w1951 _]
                      tunnel: w1943 -> [w1950 _]
                      tunnel: w1942 -> [w1949 _]
                      frame True {
                        n1144 = stacked-sequence {
                          tunnel: w1951 -> [w1954 _]
                          tunnel: w1950 -> [_ w1959]
                          tunnel: w1949 -> [w1952 _]
                          frame #0 {
                            n1145 = Build Array("T-RISE") -> (w1956:string[])
                            n1146 = Build Array(w1954) -> (w1955:dbl[])
                            n1147 = TDMS Write(0:w1952, 5:"TEST PASS", 7:w1956, 9:w1955) -> (15:w1958:errorcluster)  [unwired: 2 in, 3 out]
                            n1148 = local write "data file error"(w1958) -> ()
                          }
                          frame #1 {
                            n1149 = Bundle(cluster=w1959, "STATUS"="T-RISE PASS") -> (w1961:T4)  [unwired: 2 in]
                            n1150 = local write "RESULT LAB03-2"(TRUE) -> ()
                            n1151 = local write "DISP LAB03-2"(w1961) -> ()
                          }
                        }
                      }
                      frame False {
                      }
                    }
                  }
                }
              }
              frame #6 {
                # "LAB04-1"
                n1152 = Equal?(x=w1964, y=2) -> (x = y?=w1967:bool)
                n1153 = local read "DISP LAB04-1"() -> (w1969:T4)
                n1154 = Unbundle(w1969) -> ("STATUS"=w1970:string)  [unwired: 2 out]
                n1155 = Equal?(x=w1970, y="RUN") -> (x = y?=w1966:bool)
                n1156 = And(x=w1966, y=w1967) -> (x .and. y?=w1965:bool)
                n1157 = case shown="True" w1965 {
                  tunnel: w1969 -> [_ w1973]
                  tunnel: w1963 -> [_ w1976]
                  frame False {
                  }
                  frame True {
                    n1158 = local read "SET LAB04-1"() -> (w1975:T5)
                    n1159 = local read "TDMS LAB04-1"() -> (w1972:refnum<k34>)
                    n1160 = Unbundle(w1973) -> ("CYCLE"=w1977:dbl)  [unwired: 2 out]
                    n1161 = Unbundle(w1975) -> ("T-RISE mins"=w1974:dbl)  [unwired: 4 out]
                    n1162 = Greater Or Equal?(x=w1977, y=w1976) -> (x >= y?=w1978:bool)
                    n1163 = case shown="True" w1978 {
                      tunnel: w1974 -> [w1981 _]
                      tunnel: w1973 -> [w1980 _]
                      tunnel: w1972 -> [w1979 _]
                      frame True {
                        n1164 = stacked-sequence {
                          tunnel: w1981 -> [w1984 _]
                          tunnel: w1980 -> [_ w1989]
                          tunnel: w1979 -> [w1982 _]
                          frame #0 {
                            n1165 = Build Array("T-RISE") -> (w1986:string[])
                            n1166 = Build Array(w1984) -> (w1985:dbl[])
                            n1167 = TDMS Write(0:w1982, 5:"TEST PASS", 7:w1986, 9:w1985) -> (15:w1988:errorcluster)  [unwired: 2 in, 3 out]
                            n1168 = local write "data file error"(w1988) -> ()
                          }
                          frame #1 {
                            n1169 = Bundle(cluster=w1989, "STATUS"="T-RISE PASS") -> (w1991:T4)  [unwired: 2 in]
                            n1170 = local write "RESULT LAB04-1"(TRUE) -> ()
                            n1171 = local write "DISP LAB04-1"(w1991) -> ()
                          }
                        }
                      }
                      frame False {
                      }
                    }
                  }
                }
              }
              frame #7 {
                # "LAB04-2"
                n1172 = Equal?(x=w1994, y=2) -> (x = y?=w1997:bool)
                n1173 = local read "DISP LAB04-2"() -> (w1999:T4)
                n1174 = Unbundle(w1999) -> ("STATUS"=w2000:string)  [unwired: 2 out]
                n1175 = Equal?(x=w2000, y="RUN") -> (x = y?=w1996:bool)
                n1176 = And(x=w1996, y=w1997) -> (x .and. y?=w1995:bool)
                n1177 = case shown="True" w1995 {
                  tunnel: w1999 -> [_ w2003]
                  tunnel: w1993 -> [_ w2006]
                  frame False {
                  }
                  frame True {
                    n1178 = local read "SET LAB04-2"() -> (w2005:T5)
                    n1179 = local read "TDMS LAB04-2"() -> (w2002:refnum<k34>)
                    n1180 = Unbundle(w2003) -> ("CYCLE"=w2007:dbl)  [unwired: 2 out]
                    n1181 = Unbundle(w2005) -> ("T-RISE mins"=w2004:dbl)  [unwired: 4 out]
                    n1182 = Greater Or Equal?(x=w2007, y=w2006) -> (x >= y?=w2008:bool)
                    n1183 = case shown="True" w2008 {
                      tunnel: w2004 -> [w2011 _]
                      tunnel: w2003 -> [w2010 _]
                      tunnel: w2002 -> [w2009 _]
                      frame True {
                        n1184 = stacked-sequence {
                          tunnel: w2011 -> [w2014 _]
                          tunnel: w2010 -> [_ w2019]
                          tunnel: w2009 -> [w2012 _]
                          frame #0 {
                            n1185 = Build Array("T-RISE") -> (w2016:string[])
                            n1186 = Build Array(w2014) -> (w2015:dbl[])
                            n1187 = TDMS Write(0:w2012, 5:"TEST PASS", 7:w2016, 9:w2015) -> (15:w2018:errorcluster)  [unwired: 2 in, 3 out]
                            n1188 = local write "data file error"(w2018) -> ()
                          }
                          frame #1 {
                            n1189 = Bundle(cluster=w2019, "STATUS"="T-RISE PASS") -> (w2021:T4)  [unwired: 2 in]
                            n1190 = local write "RESULT LAB04-2"(TRUE) -> ()
                            n1191 = local write "DISP LAB04-2"(w2021) -> ()
                          }
                        }
                      }
                      frame False {
                      }
                    }
                  }
                }
              }
              frame #8 {
                # "LAB05-1"
                n1192 = Equal?(x=w2024, y=2) -> (x = y?=w2027:bool)
                n1193 = local read "DISP LAB05-1"() -> (w2029:T4)
                n1194 = Unbundle(w2029) -> ("STATUS"=w2030:string)  [unwired: 2 out]
                n1195 = Equal?(x=w2030, y="RUN") -> (x = y?=w2026:bool)
                n1196 = And(x=w2026, y=w2027) -> (x .and. y?=w2025:bool)
                n1197 = case shown="True" w2025 {
                  tunnel: w2029 -> [_ w2033]
                  tunnel: w2023 -> [_ w2036]
                  frame False {
                  }
                  frame True {
                    n1198 = local read "SET LAB05-1"() -> (w2035:T5)
                    n1199 = local read "TDMS LAB05-1"() -> (w2032:refnum<k34>)
                    n1200 = Unbundle(w2033) -> ("CYCLE"=w2037:dbl)  [unwired: 2 out]
                    n1201 = Unbundle(w2035) -> ("T-RISE mins"=w2034:dbl)  [unwired: 4 out]
                    n1202 = Greater Or Equal?(x=w2037, y=w2036) -> (x >= y?=w2038:bool)
                    n1203 = case shown="True" w2038 {
                      tunnel: w2034 -> [w2041 _]
                      tunnel: w2033 -> [w2040 _]
                      tunnel: w2032 -> [w2039 _]
                      frame True {
                        n1204 = stacked-sequence {
                          tunnel: w2041 -> [w2044 _]
                          tunnel: w2040 -> [_ w2049]
                          tunnel: w2039 -> [w2042 _]
                          frame #0 {
                            n1205 = Build Array("T-RISE") -> (w2046:string[])
                            n1206 = Build Array(w2044) -> (w2045:dbl[])
                            n1207 = TDMS Write(0:w2042, 5:"TEST PASS", 7:w2046, 9:w2045) -> (15:w2048:errorcluster)  [unwired: 2 in, 3 out]
                            n1208 = local write "data file error"(w2048) -> ()
                          }
                          frame #1 {
                            n1209 = Bundle(cluster=w2049, "STATUS"="T-RISE PASS") -> (w2051:T4)  [unwired: 2 in]
                            n1210 = local write "RESULT LAB05-1"(TRUE) -> ()
                            n1211 = local write "DISP LAB05-1"(w2051) -> ()
                          }
                        }
                      }
                      frame False {
                      }
                    }
                  }
                }
              }
              frame #9 {
                # "LAB05-2"
                n1212 = Equal?(x=w2054, y=2) -> (x = y?=w2057:bool)
                n1213 = local read "DISP LAB05-2"() -> (w2059:T4)
                n1214 = Unbundle(w2059) -> ("STATUS"=w2060:string)  [unwired: 2 out]
                n1215 = Equal?(x=w2060, y="RUN") -> (x = y?=w2056:bool)
                n1216 = And(x=w2056, y=w2057) -> (x .and. y?=w2055:bool)
                n1217 = case shown="True" w2055 {
                  tunnel: w2059 -> [_ w2063]
                  tunnel: w2053 -> [_ w2066]
                  frame False {
                  }
                  frame True {
                    n1218 = local read "SET LAB05-2"() -> (w2065:T5)
                    n1219 = local read "TDMS LAB05-2"() -> (w2062:refnum<k34>)
                    n1220 = Unbundle(w2063) -> ("CYCLE"=w2067:dbl)  [unwired: 2 out]
                    n1221 = Unbundle(w2065) -> ("T-RISE mins"=w2064:dbl)  [unwired: 4 out]
                    n1222 = Greater Or Equal?(x=w2067, y=w2066) -> (x >= y?=w2068:bool)
                    n1223 = case shown="True" w2068 {
                      tunnel: w2064 -> [w2071 _]
                      tunnel: w2063 -> [w2070 _]
                      tunnel: w2062 -> [w2069 _]
                      frame True {
                        n1224 = stacked-sequence {
                          tunnel: w2071 -> [w2074 _]
                          tunnel: w2070 -> [_ w2079]
                          tunnel: w2069 -> [w2072 _]
                          frame #0 {
                            n1225 = Build Array("T-RISE") -> (w2076:string[])
                            n1226 = Build Array(w2074) -> (w2075:dbl[])
                            n1227 = TDMS Write(0:w2072, 5:"TEST PASS", 7:w2076, 9:w2075) -> (15:w2078:errorcluster)  [unwired: 2 in, 3 out]
                            n1228 = local write "data file error"(w2078) -> ()
                          }
                          frame #1 {
                            n1229 = Bundle(cluster=w2079, "STATUS"="T-RISE PASS") -> (w2081:T4)  [unwired: 2 in]
                            n1230 = local write "RESULT LAB05-2"(TRUE) -> ()
                            n1231 = local write "DISP LAB05-2"(w2081) -> ()
                          }
                        }
                      }
                      frame False {
                      }
                    }
                  }
                }
              }
            }
          }
          frame #6 {
            # "end test & close test files"
            n1232 = stacked-sequence {
              tunnel: w2092 -> [_ _ _ _ _ _ _ _ _ _]
              tunnel: w2093 -> [_ _ _ _ _ _ _ _ _ _]
              tunnel: w2091 -> [_ _ _ _ _ _ _ _ _ _]
              tunnel: w2090 -> [_ _ _ _ _ _ _ _ _ _]
              tunnel: w2089 -> [_ _ _ _ _ _ _ _ _ _]
              tunnel: w2088 -> [_ _ _ _ _ _ _ _ _ _]
              tunnel: w2087 -> [_ _ _ _ _ _ _ _ _ _]
              tunnel: w2086 -> [_ _ _ _ _ _ _ _ _ _]
              tunnel: w2085 -> [_ _ _ _ _ _ _ _ _ _]
              tunnel: w2084 -> [_ _ _ _ _ _ _ _ _ _]
              frame #0 {
                # "LAB01-1"
                n1233 = local read "DISP LAB01-1"() -> (w2097:T4)
                n1234 = local read "run lab01-1"() -> (w2094:bool)
                n1235 = local read "TDMS LAB01-1"() -> (w2095:refnum<k34>)
                n1236 = Unbundle(w2097) -> ("CYCLE"=w2098:dbl, "STATUS"=w2096:string)  [unwired: 1 out]
                n1237 = case shown="True" w2094 {
                  tunnel: w2098 -> [_ w2102]
                  tunnel: w2097 -> [_ w2101]
                  tunnel: w2096 -> [_ w2100]
                  tunnel: w2095 -> [_ w2099]
                  frame False {
                  }
                  frame True {
                    n1238 = Not Equal?(x=w2100, y="RUN") -> (x != y?=w2103:bool)
                    n1239 = Greater?(x=w2102, y=2.0) -> (0:w2105:bool)
                    n1240 = And(x=w2105, y=w2103) -> (x .and. y?=w2104:bool)
                    n1241 = case shown="True" w2104 {
                      tunnel: w2101 -> [_ w2109]
                      tunnel: w2099 -> [_ w2108]
                      frame False {
                      }
                      frame True {
                        n1242 = stacked-sequence {
                          tunnel: w2109 -> [w2113 _ _]
                          tunnel: w2108 -> [_ w2115 _]
                          frame #0 {
                            w2110 = FALSE
                            n1243 = local write "mail control"("END") -> ()
                            n1244 = Bundle(cluster=w2113) -> (w2112:T4)  [unwired: 3 in]
                            n1245 = local write "DISP LAB01-1"(w2112) -> ()
                            n1246 = local write "O/I  LAB01-1"(w2110) -> ()
                            n1247 = local write "run lab01-1"(w2110) -> ()
                            n1248 = local write "RUN LAB01-1"(w2110) -> ()
                          }
                          frame #1 {
                            n1249 = TDMS Close(11:w2115) -> (0:w2114:errorcluster)  [unwired: 1 in, 1 out]
                            n1250 = local write "data file error"(w2114) -> ()
                          }
                          frame #2 {
                            n1251 = stacked-sequence {
                              tunnel: "LAB01-1" -> [w2118 w2120]
                              frame #0 {
                                n1252 = call "sub vi - defrag tdms v1.vi"("panel id"=w2118) -> ("error out"=w2117:errorcluster)  [unwired: 10 in]
                                n1253 = local write "data file error"(w2117) -> ()
                              }
                              frame #1 {
                                n1254 = call "Save data file to network drive v1.vi"("panel id"=w2120) -> ("network file save error"=w2119:errorcluster)  [unwired: 9 in, 1 out]
                                n1255 = local write "data file error"(w2119) -> ()
                              }
                            }
                          }
                        }
                      }
                    }
                  }
                }
              }
              frame #1 {
                # "LAB01-2"
                n1256 = local read "run lab01-2"() -> (w2121:bool)
                n1257 = case shown="True" w2121 {
                  frame False {
                  }
                  frame True {
                    n1258 = local read "DISP LAB01-2"() -> (w2128:T4)
                    n1259 = local read "TDMS LAB01-2"() -> (w2127:refnum<k34>)
                    n1260 = Unbundle(w2128) -> ("CYCLE"=w2124:dbl, "STATUS"=w2129:string)  [unwired: 1 out]
                    n1261 = Not Equal?(x=w2129, y="RUN") -> (x != y?=w2123:bool)
                    n1262 = Greater?(x=w2124, y=2.0) -> (0:w2125:bool)
                    n1263 = And(x=w2125, y=w2123) -> (x .and. y?=w2122:bool)
                    n1264 = case shown="True" w2122 {
                      tunnel: w2128 -> [_ w2132]
                      tunnel: w2127 -> [_ w2131]
                      frame False {
                      }
                      frame True {
                        n1265 = stacked-sequence {
                          tunnel: w2132 -> [w2135 _ _]
                          tunnel: w2131 -> [_ w2137 _]
                          frame #0 {
                            w2133 = FALSE
                            n1266 = local write "mail control"("END") -> ()
                            n1267 = Bundle(cluster=w2135) -> (w2136:T4)  [unwired: 3 in]
                            n1268 = local write "RUN LAB01-2"(w2133) -> ()
                            n1269 = local write "run lab01-2"(w2133) -> ()
                            n1270 = local write "O/I  LAB01-2"(w2133) -> ()
                            n1271 = local write "DISP LAB01-2"(w2136) -> ()
                          }
                          frame #1 {
                            n1272 = TDMS Close(11:w2137) -> (0:w2138:errorcluster)  [unwired: 1 in, 1 out]
                            n1273 = local write "data file error"(w2138) -> ()
                          }
                          frame #2 {
                            n1274 = stacked-sequence {
                              tunnel: "LAB01-2" -> [w2141 w2143]
                              frame #0 {
                                n1275 = call "sub vi - defrag tdms v1.vi"("panel id"=w2141) -> ("error out"=w2140:errorcluster)  [unwired: 10 in]
                                n1276 = local write "data file error"(w2140) -> ()
                              }
                              frame #1 {
                                n1277 = call "Save data file to network drive v1.vi"("panel id"=w2143) -> ("network file save error"=w2142:errorcluster)  [unwired: 9 in, 1 out]
                                n1278 = local write "data file error"(w2142) -> ()
                              }
                            }
                          }
                        }
                      }
                    }
                  }
                }
              }
              frame #2 {
                # "LAB02-1"
                n1279 = local read "run lab02-1"() -> (w2144:bool)
                n1280 = case shown="True" w2144 {
                  frame False {
                  }
                  frame True {
                    n1281 = local read "DISP LAB02-1"() -> (w2151:T4)
                    n1282 = Unbundle(w2151) -> ("CYCLE"=w2147:dbl, "STATUS"=w2152:string)  [unwired: 1 out]
                    n1283 = local read "TDMS LAB02-1"() -> (w2150:refnum<k34>)
                    n1284 = Not Equal?(x=w2152, y="RUN") -> (x != y?=w2146:bool)
                    n1285 = Greater?(x=w2147, y=2.0) -> (0:w2148:bool)
                    n1286 = And(x=w2148, y=w2146) -> (x .and. y?=w2145:bool)
                    n1287 = case shown="True" w2145 {
                      tunnel: w2151 -> [_ w2155]
                      tunnel: w2150 -> [_ w2154]
                      frame False {
                      }
                      frame True {
                        n1288 = stacked-sequence {
                          tunnel: w2155 -> [w2158 _ _]
                          tunnel: w2154 -> [_ w2160 _]
                          frame #0 {
                            w2156 = FALSE
                            n1289 = local write "mail control"("END") -> ()
                            n1290 = Bundle(cluster=w2158) -> (w2159:T4)  [unwired: 3 in]
                            n1291 = local write "O/I  LAB02-1"(w2156) -> ()
                            n1292 = local write "RUN LAB02-1"(w2156) -> ()
                            n1293 = local write "run lab02-1"(w2156) -> ()
                            n1294 = local write "DISP LAB02-1"(w2159) -> ()
                          }
                          frame #1 {
                            n1295 = TDMS Close(11:w2160) -> (0:w2161:errorcluster)  [unwired: 1 in, 1 out]
                            n1296 = local write "data file error"(w2161) -> ()
                          }
                          frame #2 {
                            n1297 = stacked-sequence {
                              tunnel: "LAB02-1" -> [w2164 w2166]
                              frame #0 {
                                n1298 = call "sub vi - defrag tdms v1.vi"("panel id"=w2164) -> ("error out"=w2163:errorcluster)  [unwired: 10 in]
                                n1299 = local write "data file error"(w2163) -> ()
                              }
                              frame #1 {
                                n1300 = call "Save data file to network drive v1.vi"("panel id"=w2166) -> ("network file save error"=w2165:errorcluster)  [unwired: 9 in, 1 out]
                                n1301 = local write "data file error"(w2165) -> ()
                              }
                            }
                          }
                        }
                      }
                    }
                  }
                }
              }
              frame #3 {
                # "LAB02-2"
                n1302 = local read "run lab02-2"() -> (w2167:bool)
                n1303 = case shown="True" w2167 {
                  frame False {
                  }
                  frame True {
                    n1304 = local read "DISP LAB02-2"() -> (w2174:T4)
                    n1305 = local read "TDMS LAB02-2"() -> (w2173:refnum<k34>)
                    n1306 = Unbundle(w2174) -> ("CYCLE"=w2170:dbl, "STATUS"=w2175:string)  [unwired: 1 out]
                    n1307 = Not Equal?(x=w2175, y="RUN") -> (x != y?=w2169:bool)
                    n1308 = Greater?(x=w2170, y=2.0) -> (0:w2171:bool)
                    n1309 = And(x=w2171, y=w2169) -> (x .and. y?=w2168:bool)
                    n1310 = case shown="True" w2168 {
                      tunnel: w2174 -> [_ w2178]
                      tunnel: w2173 -> [_ w2177]
                      frame False {
                      }
                      frame True {
                        n1311 = stacked-sequence {
                          tunnel: w2178 -> [w2181 _ _]
                          tunnel: w2177 -> [_ w2183 _]
                          frame #0 {
                            w2179 = FALSE
                            n1312 = local write "mail control"("END") -> ()
                            n1313 = Bundle(cluster=w2181) -> (w2182:T4)  [unwired: 3 in]
                            n1314 = local write "O/I  LAB02-2"(w2179) -> ()
                            n1315 = local write "run lab02-2"(w2179) -> ()
                            n1316 = local write "RUN LAB02-2"(w2179) -> ()
                            n1317 = local write "DISP LAB02-2"(w2182) -> ()
                          }
                          frame #1 {
                            n1318 = TDMS Close(11:w2183) -> (0:w2184:errorcluster)  [unwired: 1 in, 1 out]
                            n1319 = local write "data file error"(w2184) -> ()
                          }
                          frame #2 {
                            n1320 = stacked-sequence {
                              tunnel: "LAB02-2" -> [w2187 w2189]
                              frame #0 {
                                n1321 = call "sub vi - defrag tdms v1.vi"("panel id"=w2187) -> ("error out"=w2186:errorcluster)  [unwired: 10 in]
                                n1322 = local write "data file error"(w2186) -> ()
                              }
                              frame #1 {
                                n1323 = call "Save data file to network drive v1.vi"("panel id"=w2189) -> ("network file save error"=w2188:errorcluster)  [unwired: 9 in, 1 out]
                                n1324 = local write "data file error"(w2188) -> ()
                              }
                            }
                          }
                        }
                      }
                    }
                  }
                }
              }
              frame #4 {
                # "LAB03-1"
                n1325 = local read "run lab03-1"() -> (w2190:bool)
                n1326 = case shown="True" w2190 {
                  frame False {
                  }
                  frame True {
                    n1327 = local read "DISP LAB03-1"() -> (w2197:T4)
                    n1328 = local read "TDMS LAB03-1"() -> (w2196:refnum<k34>)
                    n1329 = Unbundle(w2197) -> ("CYCLE"=w2193:dbl, "STATUS"=w2198:string)  [unwired: 1 out]
                    n1330 = Not Equal?(x=w2198, y="RUN") -> (x != y?=w2192:bool)
                    n1331 = Greater?(x=w2193, y=2.0) -> (0:w2194:bool)
                    n1332 = And(x=w2194, y=w2192) -> (x .and. y?=w2191:bool)
                    n1333 = case shown="True" w2191 {
                      tunnel: w2197 -> [_ w2201]
                      tunnel: w2196 -> [_ w2200]
                      frame False {
                      }
                      frame True {
                        n1334 = stacked-sequence {
                          tunnel: w2201 -> [w2204 _ _]
                          tunnel: w2200 -> [_ w2206 _]
                          frame #0 {
                            w2202 = FALSE
                            n1335 = local write "mail control"("END") -> ()
                            n1336 = Bundle(cluster=w2204) -> (w2205:T4)  [unwired: 3 in]
                            n1337 = local write "O/I  LAB03-1"(w2202) -> ()
                            n1338 = local write "run lab03-1"(w2202) -> ()
                            n1339 = local write "RUN LAB03-1"(w2202) -> ()
                            n1340 = local write "DISP LAB03-1"(w2205) -> ()
                          }
                          frame #1 {
                            n1341 = TDMS Close(11:w2206) -> (0:w2207:errorcluster)  [unwired: 1 in, 1 out]
                            n1342 = local write "data file error"(w2207) -> ()
                          }
                          frame #2 {
                            n1343 = stacked-sequence {
                              tunnel: "LAB03-1" -> [w2210 w2212]
                              frame #0 {
                                n1344 = call "sub vi - defrag tdms v1.vi"("panel id"=w2210) -> ("error out"=w2209:errorcluster)  [unwired: 10 in]
                                n1345 = local write "data file error"(w2209) -> ()
                              }
                              frame #1 {
                                n1346 = call "Save data file to network drive v1.vi"("panel id"=w2212) -> ("network file save error"=w2211:errorcluster)  [unwired: 9 in, 1 out]
                                n1347 = local write "data file error"(w2211) -> ()
                              }
                            }
                          }
                        }
                      }
                    }
                  }
                }
              }
              frame #5 {
                # "LAB03-2"
                n1348 = local read "run lab03-2"() -> (w2213:bool)
                n1349 = case shown="True" w2213 {
                  frame False {
                  }
                  frame True {
                    n1350 = local read "DISP LAB03-2"() -> (w2220:T4)
                    n1351 = Unbundle(w2220) -> ("CYCLE"=w2216:dbl, "STATUS"=w2221:string)  [unwired: 1 out]
                    n1352 = local read "TDMS LAB03-2"() -> (w2219:refnum<k34>)
                    n1353 = Not Equal?(x=w2221, y="RUN") -> (x != y?=w2215:bool)
                    n1354 = Greater?(x=w2216, y=2.0) -> (0:w2217:bool)
                    n1355 = And(x=w2217, y=w2215) -> (x .and. y?=w2214:bool)
                    n1356 = case shown="True" w2214 {
                      tunnel: w2220 -> [_ w2224]
                      tunnel: w2219 -> [_ w2223]
                      frame False {
                      }
                      frame True {
                        n1357 = stacked-sequence {
                          tunnel: w2224 -> [w2227 _ _]
                          tunnel: w2223 -> [_ w2229 _]
                          frame #0 {
                            w2225 = FALSE
                            n1358 = local write "mail control"("END") -> ()
                            n1359 = Bundle(cluster=w2227) -> (w2228:T4)  [unwired: 3 in]
                            n1360 = local write "RUN LAB03-2"(w2225) -> ()
                            n1361 = local write "O/I  LAB03-2"(w2225) -> ()
                            n1362 = local write "DISP LAB03-2"(w2228) -> ()
                            n1363 = local write "run lab03-2"(w2225) -> ()
                          }
                          frame #1 {
                            n1364 = TDMS Close(11:w2229) -> (0:w2230:errorcluster)  [unwired: 1 in, 1 out]
                            n1365 = local write "data file error"(w2230) -> ()
                          }
                          frame #2 {
                            n1366 = stacked-sequence {
                              tunnel: "LAB03-2" -> [w2233 w2235]
                              frame #0 {
                                n1367 = call "sub vi - defrag tdms v1.vi"("panel id"=w2233) -> ("error out"=w2232:errorcluster)  [unwired: 10 in]
                                n1368 = local write "data file error"(w2232) -> ()
                              }
                              frame #1 {
                                n1369 = call "Save data file to network drive v1.vi"("panel id"=w2235) -> ("network file save error"=w2234:errorcluster)  [unwired: 9 in, 1 out]
                                n1370 = local write "data file error"(w2234) -> ()
                              }
                            }
                          }
                        }
                      }
                    }
                  }
                }
              }
              frame #6 {
                # "LAB04-1"
                n1371 = local read "run lab04-1"() -> (w2236:bool)
                n1372 = case shown="True" w2236 {
                  frame False {
                  }
                  frame True {
                    n1373 = local read "DISP LAB04-1"() -> (w2243:T4)
                    n1374 = Unbundle(w2243) -> ("CYCLE"=w2239:dbl, "STATUS"=w2244:string)  [unwired: 1 out]
                    n1375 = local read "TDMS LAB04-1"() -> (w2242:refnum<k34>)
                    n1376 = Not Equal?(x=w2244, y="RUN") -> (x != y?=w2238:bool)
                    n1377 = Greater?(x=w2239, y=2.0) -> (0:w2240:bool)
                    n1378 = And(x=w2240, y=w2238) -> (x .and. y?=w2237:bool)
                    n1379 = case shown="True" w2237 {
                      tunnel: w2243 -> [_ w2247]
                      tunnel: w2242 -> [_ w2246]
                      frame False {
                      }
                      frame True {
                        n1380 = stacked-sequence {
                          tunnel: w2247 -> [w2250 _ _]
                          tunnel: w2246 -> [_ w2252 _]
                          frame #0 {
                            w2248 = FALSE
                            n1381 = local write "mail control"("END") -> ()
                            n1382 = Bundle(cluster=w2250) -> (w2251:T4)  [unwired: 3 in]
                            n1383 = local write "RUN LAB04-1"(w2248) -> ()
                            n1384 = local write "O/I  LAB04-1"(w2248) -> ()
                            n1385 = local write "run lab04-1"(w2248) -> ()
                            n1386 = local write "DISP LAB04-1"(w2251) -> ()
                          }
                          frame #1 {
                            n1387 = TDMS Close(11:w2252) -> (0:w2253:errorcluster)  [unwired: 1 in, 1 out]
                            n1388 = local write "data file error"(w2253) -> ()
                          }
                          frame #2 {
                            n1389 = stacked-sequence {
                              tunnel: "LAB04-1" -> [w2256 w2258]
                              frame #0 {
                                n1390 = call "sub vi - defrag tdms v1.vi"("panel id"=w2256) -> ("error out"=w2255:errorcluster)  [unwired: 10 in]
                                n1391 = local write "data file error"(w2255) -> ()
                              }
                              frame #1 {
                                n1392 = call "Save data file to network drive v1.vi"("panel id"=w2258) -> ("network file save error"=w2257:errorcluster)  [unwired: 9 in, 1 out]
                                n1393 = local write "data file error"(w2257) -> ()
                              }
                            }
                          }
                        }
                      }
                    }
                  }
                }
              }
              frame #7 {
                # "LAB04-2"
                n1394 = local read "run lab04-2"() -> (w2259:bool)
                n1395 = case shown="True" w2259 {
                  frame False {
                  }
                  frame True {
                    n1396 = local read "DISP LAB04-2"() -> (w2266:T4)
                    n1397 = Unbundle(w2266) -> ("CYCLE"=w2262:dbl, "STATUS"=w2267:string)  [unwired: 1 out]
                    n1398 = Not Equal?(x=w2267, y="RUN") -> (x != y?=w2261:bool)
                    n1399 = local read "TDMS LAB04-2"() -> (w2265:refnum<k34>)
                    n1400 = Greater?(x=w2262, y=2.0) -> (0:w2263:bool)
                    n1401 = And(x=w2263, y=w2261) -> (x .and. y?=w2260:bool)
                    n1402 = case shown="True" w2260 {
                      tunnel: w2266 -> [_ w2270]
                      tunnel: w2265 -> [_ w2269]
                      frame False {
                      }
                      frame True {
                        n1403 = stacked-sequence {
                          tunnel: w2270 -> [w2273 _ _]
                          tunnel: w2269 -> [_ w2275 _]
                          frame #0 {
                            w2271 = FALSE
                            n1404 = local write "mail control"("END") -> ()
                            n1405 = Bundle(cluster=w2273) -> (w2274:T4)  [unwired: 3 in]
                            n1406 = local write "O/I  LAB04-2"(w2271) -> ()
                            n1407 = local write "RUN LAB04-2"(w2271) -> ()
                            n1408 = local write "run lab04-2"(w2271) -> ()
                            n1409 = local write "DISP LAB04-2"(w2274) -> ()
                          }
                          frame #1 {
                            n1410 = TDMS Close(11:w2275) -> (0:w2276:errorcluster)  [unwired: 1 in, 1 out]
                            n1411 = local write "data file error"(w2276) -> ()
                          }
                          frame #2 {
                            n1412 = stacked-sequence {
                              tunnel: "LAB04-2" -> [w2279 w2281]
                              frame #0 {
                                n1413 = call "sub vi - defrag tdms v1.vi"("panel id"=w2279) -> ("error out"=w2278:errorcluster)  [unwired: 10 in]
                                n1414 = local write "data file error"(w2278) -> ()
                              }
                              frame #1 {
                                n1415 = call "Save data file to network drive v1.vi"("panel id"=w2281) -> ("network file save error"=w2280:errorcluster)  [unwired: 9 in, 1 out]
                                n1416 = local write "data file error"(w2280) -> ()
                              }
                            }
                          }
                        }
                      }
                    }
                  }
                }
              }
              frame #8 {
                # "LAB05-1"
                n1417 = local read "run lab05-1"() -> (w2282:bool)
                n1418 = case shown="True" w2282 {
                  frame False {
                  }
                  frame True {
                    n1419 = local read "DISP LAB05-1"() -> (w2289:T4)
                    n1420 = Unbundle(w2289) -> ("CYCLE"=w2285:dbl, "STATUS"=w2290:string)  [unwired: 1 out]
                    n1421 = Not Equal?(x=w2290, y="RUN") -> (x != y?=w2284:bool)
                    n1422 = local read "TDMS LAB05-1"() -> (w2288:refnum<k34>)
                    n1423 = Greater?(x=w2285, y=2.0) -> (0:w2286:bool)
                    n1424 = And(x=w2286, y=w2284) -> (x .and. y?=w2283:bool)
                    n1425 = case shown="True" w2283 {
                      tunnel: w2289 -> [_ w2293]
                      tunnel: w2288 -> [_ w2292]
                      frame False {
                      }
                      frame True {
                        n1426 = stacked-sequence {
                          tunnel: w2293 -> [w2296 _ _]
                          tunnel: w2292 -> [_ w2298 _]
                          frame #0 {
                            w2294 = FALSE
                            n1427 = local write "mail control"("END") -> ()
                            n1428 = Bundle(cluster=w2296) -> (w2297:T4)  [unwired: 3 in]
                            n1429 = local write "O/I  LAB05-1"(w2294) -> ()
                            n1430 = local write "RUN LAB05-1"(w2294) -> ()
                            n1431 = local write "run lab05-1"(w2294) -> ()
                            n1432 = local write "DISP LAB05-1"(w2297) -> ()
                          }
                          frame #1 {
                            n1433 = TDMS Close(11:w2298) -> (0:w2299:errorcluster)  [unwired: 1 in, 1 out]
                            n1434 = local write "data file error"(w2299) -> ()
                          }
                          frame #2 {
                            n1435 = stacked-sequence {
                              tunnel: "LAB05-1" -> [w2302 w2304]
                              frame #0 {
                                n1436 = call "sub vi - defrag tdms v1.vi"("panel id"=w2302) -> ("error out"=w2301:errorcluster)  [unwired: 10 in]
                                n1437 = local write "data file error"(w2301) -> ()
                              }
                              frame #1 {
                                n1438 = call "Save data file to network drive v1.vi"("panel id"=w2304) -> ("network file save error"=w2303:errorcluster)  [unwired: 9 in, 1 out]
                                n1439 = local write "data file error"(w2303) -> ()
                              }
                            }
                          }
                        }
                      }
                    }
                  }
                }
              }
              frame #9 {
                # "LAB05-2"
                n1440 = local read "run lab05-2"() -> (w2305:bool)
                n1441 = case shown="True" w2305 {
                  frame False {
                  }
                  frame True {
                    n1442 = local read "DISP LAB05-2"() -> (w2312:T4)
                    n1443 = Unbundle(w2312) -> ("CYCLE"=w2308:dbl, "STATUS"=w2313:string)  [unwired: 1 out]
                    n1444 = Not Equal?(x=w2313, y="RUN") -> (x != y?=w2307:bool)
                    n1445 = local read "TDMS LAB05-2"() -> (w2311:refnum<k34>)
                    n1446 = Greater?(x=w2308, y=2.0) -> (0:w2309:bool)
                    n1447 = And(x=w2309, y=w2307) -> (x .and. y?=w2306:bool)
                    n1448 = case shown="True" w2306 {
                      tunnel: w2312 -> [_ w2316]
                      tunnel: w2311 -> [_ w2315]
                      frame False {
                      }
                      frame True {
                        n1449 = stacked-sequence {
                          tunnel: w2316 -> [w2319 _ _]
                          tunnel: w2315 -> [_ w2321 _]
                          frame #0 {
                            w2317 = FALSE
                            n1450 = local write "mail control"("END") -> ()
                            n1451 = Bundle(cluster=w2319) -> (w2320:T4)  [unwired: 3 in]
                            n1452 = local write "RUN LAB05-2"(w2317) -> ()
                            n1453 = local write "O/I  LAB05-2"(w2317) -> ()
                            n1454 = local write "run lab05-2"(w2317) -> ()
                            n1455 = local write "DISP LAB05-2"(w2320) -> ()
                          }
                          frame #1 {
                            n1456 = TDMS Close(11:w2321) -> (0:w2322:errorcluster)  [unwired: 1 in, 1 out]
                            n1457 = local write "data file error"(w2322) -> ()
                          }
                          frame #2 {
                            n1458 = stacked-sequence {
                              tunnel: "LAB05-2" -> [w2325 w2327]
                              frame #0 {
                                n1459 = call "sub vi - defrag tdms v1.vi"("panel id"=w2325) -> ("error out"=w2324:errorcluster)  [unwired: 10 in]
                                n1460 = local write "data file error"(w2324) -> ()
                              }
                              frame #1 {
                                n1461 = call "Save data file to network drive v1.vi"("panel id"=w2327) -> ("network file save error"=w2326:errorcluster)  [unwired: 9 in, 1 out]
                                n1462 = local write "data file error"(w2326) -> ()
                              }
                            }
                          }
                        }
                      }
                    }
                  }
                }
              }
            }
            n1463 = local read "Network Directory"() -> (w2083:path)
            n1464 = global write "Global 1.vi" "Network Drive"(w2083) -> ()
          }
          frame #7 {
            # "disable functions"
            n1465 = stacked-sequence {
              tunnel: w2337 -> [w2351 _ w2407]
              tunnel: w2336 -> [w2346 _ w2406]
              tunnel: w2335 -> [w2345 _ w2405]
              tunnel: w2334 -> [w2343 _ w2404]
              tunnel: w2333 -> [w2344 _ w2403]
              tunnel: w2332 -> [_ w2368 w2402]
              tunnel: w2331 -> [_ w2369 w2401]
              tunnel: w2330 -> [_ w2370 w2400]
              tunnel: w2329 -> [_ w2371 w2399]
              tunnel: w2328 -> [_ w2372 w2398]
              frame #0 {
                n1466 = Select(t=2, s=w2343, f=0) -> (s? t:f=w2339:i32)
                n1467 = Select(t=2, s=w2345, f=0) -> (s? t:f=w2340:i32)
                n1468 = Select(t=2, s=w2344, f=0) -> (s? t:f=w2338:i32)
                n1469 = Select(t=2, s=w2351, f=0) -> (s? t:f=w2342:i32)
                n1470 = Select(t=2, s=w2346, f=0) -> (s? t:f=w2341:i32)
                n1471 = property on="SELECT LAB02-2" class="RadioBtnsControl (strict)"("DisabledEnum"=w2339) -> ()  [unwired: 2 in, 2 out]
                n1472 = property on="SELECT LAB02-1" class="RadioBtnsControl (strict)"("DisabledEnum"=w2340) -> ()  [unwired: 2 in, 2 out]
                n1473 = property on="SELECT LAB03-1" class="RadioBtnsControl (strict)"("DisabledEnum"=w2338) -> ()  [unwired: 2 in, 2 out]
                n1474 = property on="SELECT LAB01-1" class="RadioBtnsControl (strict)"("DisabledEnum"=w2342) -> ()  [unwired: 2 in, 2 out]
                n1475 = property on="SELECT LAB01-2" class="RadioBtnsControl (strict)"("DisabledEnum"=w2341) -> ()  [unwired: 2 in, 2 out]
                n1476 = Not(x=w2351) -> (.not. x?=w2352:bool)
                n1477 = property on="RESULT LAB01-1" class="Bool (strict)"("Visible"=w2352) -> ()  [unwired: 2 in, 2 out]
                n1478 = Not(x=w2346) -> (.not. x?=w2350:bool)
                n1479 = Not(x=w2345) -> (.not. x?=w2349:bool)
                n1480 = Not(x=w2343) -> (.not. x?=w2348:bool)
                n1481 = property on="RESULT LAB01-2" class="Bool (strict)"("Visible"=w2350) -> ()  [unwired: 2 in, 2 out]
                n1482 = Not(x=w2344) -> (.not. x?=w2347:bool)
                n1483 = property on="RESULT LAB02-1" class="Bool (strict)"("Visible"=w2349) -> ()  [unwired: 2 in, 2 out]
                n1484 = property on="RESULT LAB02-2" class="Bool (strict)"("Visible"=w2348) -> ()  [unwired: 2 in, 2 out]
                n1485 = property on="RESULT LAB03-1" class="Bool (strict)"("Visible"=w2347) -> ()  [unwired: 2 in, 2 out]
                n1486 = property on="SET LAB01-1" class="Clust (strict)"("DisabledEnum"=w2342) -> ()  [unwired: 2 in, 2 out]
                n1487 = property on="SET LAB01-2" class="Clust (strict)"("DisabledEnum"=w2341) -> ()  [unwired: 2 in, 2 out]
                n1488 = property on="SET LAB02-1" class="Clust (strict)"("DisabledEnum"=w2340) -> ()  [unwired: 2 in, 2 out]
                n1489 = property on="SET LAB02-2" class="Clust (strict)"("DisabledEnum"=w2339) -> ()  [unwired: 2 in, 2 out]
                n1490 = property on="SET LAB03-1" class="Clust (strict)"("DisabledEnum"=w2338) -> ()  [unwired: 2 in, 2 out]
                n1491 = property on="O/I  LAB01-1" class="Bool (strict)"("DisabledEnum"=w2342) -> ()  [unwired: 2 in, 2 out]
                n1492 = property on="O/I  LAB01-2" class="Bool (strict)"("DisabledEnum"=w2341) -> ()  [unwired: 2 in, 2 out]
                n1493 = property on="O/I  LAB02-1" class="Bool (strict)"("DisabledEnum"=w2340) -> ()  [unwired: 2 in, 2 out]
                n1494 = property on="O/I  LAB02-2" class="Bool (strict)"("DisabledEnum"=w2339) -> ()  [unwired: 2 in, 2 out]
                n1495 = property on="O/I  LAB03-1" class="Bool (strict)"("DisabledEnum"=w2338) -> ()  [unwired: 2 in, 2 out]
              }
              frame #1 {
                n1496 = Select(t=2, s=w2372, f=0) -> (s? t:f=w2363:i32)
                n1497 = Select(t=2, s=w2371, f=0) -> (s? t:f=w2364:i32)
                n1498 = Select(t=2, s=w2368, f=0) -> (s? t:f=w2367:i32)
                n1499 = Select(t=2, s=w2369, f=0) -> (s? t:f=w2366:i32)
                n1500 = Select(t=2, s=w2370, f=0) -> (s? t:f=w2365:i32)
                n1501 = property on="SELECT LAB05-2" class="RadioBtnsControl (strict)"("DisabledEnum"=w2363) -> ()  [unwired: 2 in, 2 out]
                n1502 = property on="SELECT LAB05-1" class="RadioBtnsControl (strict)"("DisabledEnum"=w2364) -> ()  [unwired: 2 in, 2 out]
                n1503 = property on="SELECT LAB03-2" class="RadioBtnsControl (strict)"("DisabledEnum"=w2367) -> ()  [unwired: 2 in, 2 out]
                n1504 = property on="SELECT LAB04-1" class="RadioBtnsControl (strict)"("DisabledEnum"=w2366) -> ()  [unwired: 2 in, 2 out]
                n1505 = property on="SELECT LAB04-2" class="RadioBtnsControl (strict)"("DisabledEnum"=w2365) -> ()  [unwired: 2 in, 2 out]
                n1506 = property on="SET LAB05-2" class="Clust (strict)"("DisabledEnum"=w2363) -> ()  [unwired: 2 in, 2 out]
                n1507 = property on="SET LAB05-1" class="Clust (strict)"("DisabledEnum"=w2364) -> ()  [unwired: 2 in, 2 out]
                n1508 = property on="SET LAB03-2" class="Clust (strict)"("DisabledEnum"=w2367) -> ()  [unwired: 2 in, 2 out]
                n1509 = property on="SET LAB04-1" class="Clust (strict)"("DisabledEnum"=w2366) -> ()  [unwired: 2 in, 2 out]
                n1510 = property on="SET LAB04-2" class="Clust (strict)"("DisabledEnum"=w2365) -> ()  [unwired: 2 in, 2 out]
                n1511 = property on="O/I  LAB05-2" class="Bool (strict)"("DisabledEnum"=w2363) -> ()  [unwired: 2 in, 2 out]
                n1512 = property on="O/I  LAB05-1" class="Bool (strict)"("DisabledEnum"=w2364) -> ()  [unwired: 2 in, 2 out]
                n1513 = property on="O/I  LAB04-1" class="Bool (strict)"("DisabledEnum"=w2366) -> ()  [unwired: 2 in, 2 out]
                n1514 = property on="O/I  LAB04-2" class="Bool (strict)"("DisabledEnum"=w2365) -> ()  [unwired: 2 in, 2 out]
                n1515 = property on="O/I  LAB03-2" class="Bool (strict)"("DisabledEnum"=w2367) -> ()  [unwired: 2 in, 2 out]
                n1516 = Not(x=w2372) -> (.not. x?=w2373:bool)
                n1517 = Not(x=w2371) -> (.not. x?=w2374:bool)
                n1518 = Not(x=w2370) -> (.not. x?=w2375:bool)
                n1519 = property on="RESULT LAB05-2" class="Bool (strict)"("Visible"=w2373) -> ()  [unwired: 2 in, 2 out]
                n1520 = property on="RESULT LAB05-1" class="Bool (strict)"("Visible"=w2374) -> ()  [unwired: 2 in, 2 out]
                n1521 = Not(x=w2369) -> (.not. x?=w2376:bool)
                n1522 = property on="RESULT LAB04-2" class="Bool (strict)"("Visible"=w2375) -> ()  [unwired: 2 in, 2 out]
                n1523 = Not(x=w2368) -> (.not. x?=w2377:bool)
                n1524 = property on="RESULT LAB04-1" class="Bool (strict)"("Visible"=w2376) -> ()  [unwired: 2 in, 2 out]
                n1525 = property on="RESULT LAB03-2" class="Bool (strict)"("Visible"=w2377) -> ()  [unwired: 2 in, 2 out]
              }
              frame #2 {
                # "disable calibrate if any test running"
                n1526 = Or(x=w2399, y=w2398) -> (x .or. y?=w2392:bool)
                n1527 = Or(x=w2401, y=w2400) -> (x .or. y?=w2394:bool)
                n1528 = Or(x=w2405, y=w2404) -> (x .or. y?=w2396:bool)
                n1529 = Or(x=w2403, y=w2402) -> (x .or. y?=w2395:bool)
                n1530 = Or(x=w2407, y=w2406) -> (x .or. y?=w2397:bool)
                n1531 = Or(x=w2395, y=w2394) -> (x .or. y?=w2393:bool)
                n1532 = Or(x=w2397, y=w2396) -> (x .or. y?=w2391:bool)
                n1533 = Or(x=w2393, y=w2392) -> (x .or. y?=w2390:bool)
                n1534 = Or(x=w2391, y=w2390) -> (x .or. y?=w2389:bool)
                n1535 = case shown="True" w2389 {
                  tunnel: [0 2] -> w2388
                  frame False {
                  }
                  frame True {
                  }
                }
                n1536 = property on="JIG TEST" class="Clust (strict)"("DisabledEnum"=w2388) -> ()  [unwired: 2 in, 2 out]
                n1537 = property on="Network Directory" class="Path"("DisabledEnum"=w2388) -> ()  [unwired: 2 in, 2 out]
                n1538 = property on="MAIL SETTINGS" class="Clust (strict)"("DisabledEnum"=w2388) -> ()  [unwired: 2 in, 2 out]
                n1539 = property on="CALIBRATE" class="Bool (strict)"("DisabledEnum"=w2388) -> ()  [unwired: 2 in, 2 out]
                n1540 = property on="ADMIN PAGE" class="Bool (strict)"("DisabledEnum"=w2388) -> ()  [unwired: 2 in, 2 out]
              }
            }
          }
          frame #8 {
            # "drive jigs"
            n1541 = stacked-sequence {
              frame #0 {
                # "jig on"
                n1542 = local read "jig cycle"() -> (w2415:dbl)
                n1543 = property on="JIG TEST" class="Clust (strict)"() -> ("DisabledEnum"=w2412:T13)  [unwired: 2 in, 2 out]
                n1544 = Equal?(x=w2412, y=2) -> (x = y?=w2411:bool)
                n1545 = Equal?(x=w2415, y=0) -> (x = y?=w2413:bool)
                n1546 = And(x=w2413, y=w2411) -> (x .and. y?=w2410:bool)
                n1547 = case shown="True" w2410 {
                  frame False {
                  }
                  frame True {
                    n1548 = local read "run lab01-1"() -> (w2426:bool)
                    n1549 = local read "run lab01-2"() -> (w2425:bool)
                    n1550 = local read "run lab02-1"() -> (w2424:bool)
                    n1551 = local read "run lab02-2"() -> (w2423:bool)
                    n1552 = local read "run lab03-1"() -> (w2422:bool)
                    n1553 = local read "run lab03-2"() -> (w2421:bool)
                    n1554 = local read "run lab04-1"() -> (w2420:bool)
                    n1555 = local read "run lab04-2"() -> (w2419:bool)
                    n1556 = local read "run lab05-1"() -> (w2418:bool)
                    n1557 = local read "run lab05-2"() -> (w2417:bool)
                    n1558 = local write "JIG LAB03-2"(w2421) -> ()
                    n1559 = local write "JIG LAB01-1"(w2426) -> ()
                    n1560 = local write "JIG LAB01-2"(w2425) -> ()
                    n1561 = local write "JIG LAB02-1"(w2424) -> ()
                    n1562 = local write "JIG LAB02-2"(w2423) -> ()
                    n1563 = local write "JIG LAB03-1"(w2422) -> ()
                    n1564 = local write "JIG LAB04-1"(w2420) -> ()
                    n1565 = local write "JIG LAB04-2"(w2419) -> ()
                    n1566 = local write "JIG LAB05-1"(w2418) -> ()
                    n1567 = local write "JIG LAB05-2"(w2417) -> ()
                  }
                }
              }
              frame #1 {
                # "jig off"
                n1568 = local read "jig cycle"() -> (w2433:dbl)
                n1569 = local read "on loops"() -> (w2432:dbl)
                n1570 = property on="JIG TEST" class="Clust (strict)"() -> ("DisabledEnum"=w2431:T13)  [unwired: 2 in, 2 out]
                n1571 = Equal?(x=w2431, y=2) -> (x = y?=w2429:bool)
                n1572 = Equal?(x=w2433, y=w2432) -> (x = y?=w2428:bool)
                n1573 = And(x=w2428, y=w2429) -> (x .and. y?=w2427:bool)
                n1574 = case shown="True" w2427 {
                  frame False {
                  }
                  frame True {
                    w2484 = FALSE
                    w2485 = TRUE
                    w2483 = 2
                    n1575 = local read "SELECT LAB05-2"() -> (w2474:T3)
                    n1576 = local read "SELECT LAB04-2"() -> (w2476:T3)
                    n1577 = local read "SELECT LAB04-1"() -> (w2477:T3)
                    n1578 = local read "SELECT LAB05-1"() -> (w2475:T3)
                    n1579 = local read "SELECT LAB03-2"() -> (w2478:T3)
                    n1580 = local read "SELECT LAB02-1"() -> (w2481:T3)
                    n1581 = local read "SELECT LAB03-1"() -> (w2479:T3)
                    n1582 = local read "SELECT LAB02-2"() -> (w2480:T3)
                    n1583 = local read "SELECT LAB01-2"() -> (w2482:T3)
                    n1584 = local read "run lab05-1"() -> (w2444:bool)
                    n1585 = local read "run lab05-2"() -> (w2443:bool)
                    n1586 = local read "SELECT LAB01-1"() -> (w2486:T3)
                    n1587 = local read "run lab04-2"() -> (w2445:bool)
                    n1588 = local read "run lab04-1"() -> (w2446:bool)
                    n1589 = local read "run lab01-1"() -> (w2462:bool)
                    n1590 = local read "run lab01-2"() -> (w2451:bool)
                    n1591 = local read "run lab03-2"() -> (w2447:bool)
                    n1592 = local read "run lab03-1"() -> (w2448:bool)
                    n1593 = local read "run lab02-1"() -> (w2450:bool)
                    n1594 = local read "run lab02-2"() -> (w2449:bool)
                    n1595 = Equal?(x=w2483, y=w2479) -> (x = y?=w2457:bool)
                    n1596 = Equal?(x=w2483, y=w2478) -> (x = y?=w2456:bool)
                    n1597 = Equal?(x=w2483, y=w2477) -> (x = y?=w2455:bool)
                    n1598 = Equal?(x=w2483, y=w2476) -> (x = y?=w2454:bool)
                    n1599 = Equal?(x=w2483, y=w2475) -> (x = y?=w2453:bool)
                    n1600 = Equal?(x=w2483, y=w2474) -> (x = y?=w2452:bool)
                    n1601 = Equal?(x=w2483, y=w2486) -> (x = y?=w2463:bool)
                    n1602 = Equal?(x=w2483, y=w2481) -> (x = y?=w2459:bool)
                    n1603 = Equal?(x=w2483, y=w2480) -> (x = y?=w2458:bool)
                    n1604 = Equal?(x=w2483, y=w2482) -> (x = y?=w2460:bool)
                    n1605 = And(x=w2454, y=w2445) -> (x .and. y?=w2436:bool)
                    n1606 = And(x=w2457, y=w2448) -> (x .and. y?=w2439:bool)
                    n1607 = And(x=w2455, y=w2446) -> (x .and. y?=w2437:bool)
                    n1608 = And(x=w2452, y=w2443) -> (x .and. y?=w2434:bool)
                    n1609 = And(x=w2458, y=w2449) -> (x .and. y?=w2440:bool)
                    n1610 = And(x=w2456, y=w2447) -> (x .and. y?=w2438:bool)
                    n1611 = And(x=w2453, y=w2444) -> (x .and. y?=w2435:bool)
                    n1612 = And(x=w2460, y=w2451) -> (x .and. y?=w2442:bool)
                    n1613 = And(x=w2463, y=w2462) -> (x .and. y?=w2461:bool)
                    n1614 = And(x=w2459, y=w2450) -> (x .and. y?=w2441:bool)
                    n1615 = Select(t=w2485, s=w2461, f=w2484) -> (s? t:f=w2464:bool)
                    n1616 = Select(t=w2485, s=w2442, f=w2484) -> (s? t:f=w2465:bool)
                    n1617 = Select(t=w2485, s=w2441, f=w2484) -> (s? t:f=w2466:bool)
                    n1618 = Select(t=w2485, s=w2440, f=w2484) -> (s? t:f=w2467:bool)
                    n1619 = Select(t=w2485, s=w2439, f=w2484) -> (s? t:f=w2468:bool)
                    n1620 = Select(t=w2485, s=w2438, f=w2484) -> (s? t:f=w2469:bool)
                    n1621 = Select(t=w2485, s=w2437, f=w2484) -> (s? t:f=w2470:bool)
                    n1622 = Select(t=w2485, s=w2436, f=w2484) -> (s? t:f=w2471:bool)
                    n1623 = Select(t=w2485, s=w2435, f=w2484) -> (s? t:f=w2472:bool)
                    n1624 = Select(t=w2485, s=w2434, f=w2484) -> (s? t:f=w2473:bool)
                    n1625 = local write "JIG LAB03-2"(w2469) -> ()
                    n1626 = local write "JIG LAB02-1"(w2466) -> ()
                    n1627 = local write "JIG LAB02-2"(w2467) -> ()
                    n1628 = local write "JIG LAB01-2"(w2465) -> ()
                    n1629 = local write "JIG LAB03-1"(w2468) -> ()
                    n1630 = local write "JIG LAB01-1"(w2464) -> ()
                    n1631 = local write "JIG LAB05-2"(w2473) -> ()
                    n1632 = local write "JIG LAB04-1"(w2470) -> ()
                    n1633 = local write "JIG LAB05-1"(w2472) -> ()
                    n1634 = local write "JIG LAB04-2"(w2471) -> ()
                  }
                }
              }
            }
          }
          frame #9 {
            # "enable  jig test output if no test busy"
            n1635 = property on="JIG TEST" class="Clust (strict)"() -> ("DisabledEnum"=w2489:T13)  [unwired: 2 in, 2 out]
            n1636 = Equal?(x=w2489, y=0) -> (x = y?=w2487:bool)
            n1637 = case shown="True" w2487 {
              frame False {
              }
              frame True {
                n1638 = local read "JIG TEST"() -> (w2500:T10)
                n1639 = Unbundle(w2500) -> ("LAB01-1"=w2499:bool, "LAB01-2"=w2498:bool, "LAB02-1"=w2497:bool, "LAB02-2"=w2496:bool, "LAB03-1"=w2495:bool, "LAB03-2"=w2494:bool, "LAB04-1"=w2493:bool, "LAB04-2"=w2492:bool, "LAB05-1"=w2491:bool, "LAB05-2"=w2490:bool)
                n1640 = local write "JIG LAB05-1"(w2491) -> ()
                n1641 = local write "JIG LAB05-2"(w2490) -> ()
                n1642 = local write "JIG LAB04-1"(w2493) -> ()
                n1643 = local write "JIG LAB04-2"(w2492) -> ()
                n1644 = local write "JIG LAB03-2"(w2494) -> ()
                n1645 = local write "JIG LAB01-1"(w2499) -> ()
                n1646 = local write "JIG LAB02-1"(w2497) -> ()
                n1647 = local write "JIG LAB03-1"(w2495) -> ()
                n1648 = local write "JIG LAB01-2"(w2498) -> ()
                n1649 = local write "JIG LAB02-2"(w2496) -> ()
              }
            }
          }
          frame #10 {
            # "drive digital output"
            n1650 = local read "O/I  LAB05-2"() -> (w2506:bool)
            n1651 = local read "O/I  LAB05-1"() -> (w2508:bool)
            n1652 = local read "JIG LAB05-2"() -> (w2505:bool)
            n1653 = local read "O/I  LAB04-2"() -> (w2510:bool)
            n1654 = local read "JIG LAB05-1"() -> (w2507:bool)
            n1655 = local read "JIG LAB04-2"() -> (w2509:bool)
            n1656 = local read "O/I  LAB03-1"() -> (w2515:bool)
            n1657 = local read "O/I  LAB04-1"() -> (w2511:bool)
            n1658 = local read "O/I  LAB02-1"() -> (w2519:bool)
            n1659 = local read "O/I  LAB02-2"() -> (w2517:bool)
            n1660 = local read "O/I  LAB03-2"() -> (w2513:bool)
            n1661 = local read "JIG LAB04-1"() -> (w2504:bool)
            n1662 = local read "JIG LAB03-2"() -> (w2512:bool)
            n1663 = local read "O/I  LAB01-2"() -> (w2521:bool)
            n1664 = local read "JIG LAB02-1"() -> (w2518:bool)
            n1665 = local read "JIG LAB02-2"() -> (w2516:bool)
            n1666 = local read "JIG LAB03-1"() -> (w2514:bool)
            n1667 = local read "O/I  LAB01-1"() -> (w2523:bool)
            n1668 = local read "JIG LAB01-2"() -> (w2520:bool)
            n1669 = local read "JIG LAB01-1"() -> (w2522:bool)
            n1670 = Build Array(w2510, w2509, w2508, w2507, w2506, w2505) -> (w2501:bool[])
            n1671 = Build Array(w2516, w2515, w2514, w2513, w2512, w2511, w2504) -> (w2502:bool[])
            n1672 = Build Array(w2523, w2522, w2521, w2520, w2519, w2518, w2517) -> (w2503:bool[])
            n1673 = call "sub vi - Drive Relays All v6.vi"("Array #2"=w2501, "Array #1"=w2502, "Array #0"=w2503) -> ()  [unwired: 8 in, 1 out]
          }
          frame #11 {
            # "get temperature values"
            n1674 = stacked-sequence {
              frame #0 {
                n1675 = local read "jig cycle"() -> (w2524:dbl)
                n1676 = local read "on loops"() -> (w2527:dbl)
                n1677 = local read "jig cycle"() -> (w2529:dbl)
                n1678 = Add(x=w2527, y=2) -> (x+y=w2528:dbl)
                n1679 = Equal?(x=w2529, y=0) -> (x = y?=w2530:bool)
                n1680 = Equal?(x=w2524, y=w2528) -> (x = y?=w2525:bool)
                n1681 = case shown="True" w2530 {
                  frame False {
                  }
                  frame True {
                    w2542 = FALSE
                    w2543 = TRUE
                    n1682 = local write "TEMP update"(TRUE) -> ()
                    n1683 = call "sub vi - GET ALL TEMP v3.vi"("LA01-EN"=w2543, "LA02-EN"=w2543, "LA03-EN"=w2543, "LA04-EN"=w2542, "LA05-EN"=w2542, "Gen Cal Value"=1.0) -> ("LA01 TEMP"=w2541:T21, "LA02 TEMP"=w2539:T21, "LA03 TEMP"=w2538:T21)  [unwired: 4 in, 3 out]
                    n1684 = local write "LAB03 TEMP"(w2538) -> ()
                    n1685 = local write "LAB02 TEMP"(w2539) -> ()
                    n1686 = local write "LAB01 TEMP"(w2541) -> ()
                  }
                }
                n1687 = case shown="True" w2525 {
                  frame False {
                  }
                  frame True {
                    w2535 = TRUE
                    w2536 = FALSE
                    n1688 = local write "TEMP update"(TRUE) -> ()
                    n1689 = call "sub vi - GET ALL TEMP v3.vi"("LA01-EN"=w2536, "LA02-EN"=w2536, "LA03-EN"=w2536, "LA04-EN"=w2535, "LA05-EN"=w2535, "Gen Cal Value"=1.0) -> ("LA04 TEMP"=w2533:T21, "LA05 TEMP"=w2532:T21)  [unwired: 4 in, 4 out]
                    n1690 = local write "LAB04 TEMP"(w2533) -> ()
                    n1691 = local write "LAB05 TEMP"(w2532) -> ()
                  }
                }
              }
              frame #1 {
                n1692 = local read "CAL LAB01"() -> (w2561:T7)
                n1693 = local read "LAB01 TEMP"() -> (w2562:T12)
                n1694 = Unbundle By Name(w2562) -> ("T1 Live"=w2552:dbl, "T1 Neut"=w2551:dbl, "T2 Live"=w2550:dbl, "T2 Neut"=w2549:dbl)  [unwired: 2 out]
                n1695 = Unbundle By Name(w2561) -> ("1 (TL) cal"=w2548:dbl, "1 (TN) cal"=w2547:dbl, "2 (TL) cal"=w2546:dbl, "2 (TN) cal"=w2545:dbl)  [unwired: 6 out]
                n1696 = Multiply(x=w2552, y=w2548) -> (x*y=w2558:dbl)
                n1697 = Multiply(x=w2551, y=w2547) -> (x*y=w2557:dbl)
                n1698 = Multiply(x=w2550, y=w2546) -> (x*y=w2554:dbl)
                n1699 = Multiply(x=w2549, y=w2545) -> (x*y=w2553:dbl)
                n1700 = local read "SIG LAB01-2"() -> (w2556:T2)
                n1701 = local read "SIG LAB01-1"() -> (w2560:T2)
                n1702 = Bundle By Name(cluster=w2560, "Tmp Live"=w2558, "Tmp Neut"=w2557) -> (w2559:T2)
                n1703 = Bundle By Name(cluster=w2556, "Tmp Live"=w2554, "Tmp Neut"=w2553) -> (w2555:T2)
                n1704 = local write "SIG LAB01-1"(w2559) -> ()
                n1705 = local write "SIG LAB01-2"(w2555) -> ()
              }
              frame #2 {
                n1706 = local read "CAL LAB02"() -> (w2579:T8)
                n1707 = local read "LAB02 TEMP"() -> (w2580:T12)
                n1708 = Unbundle By Name(w2580) -> ("T1 Live"=w2570:dbl, "T1 Neut"=w2569:dbl, "T2 Live"=w2568:dbl, "T2 Neut"=w2567:dbl)  [unwired: 2 out]
                n1709 = Unbundle By Name(w2579) -> ("1 (TL) cal"=w2566:dbl, "1 (TN) cal"=w2565:dbl, "2 (TL) cal"=w2564:dbl, "2 (TN) cal"=w2563:dbl)  [unwired: 6 out]
                n1710 = Multiply(x=w2570, y=w2566) -> (x*y=w2576:dbl)
                n1711 = Multiply(x=w2569, y=w2565) -> (x*y=w2575:dbl)
                n1712 = Multiply(x=w2568, y=w2564) -> (x*y=w2572:dbl)
                n1713 = Multiply(x=w2567, y=w2563) -> (x*y=w2571:dbl)
                n1714 = local read "SIG LAB02-2"() -> (w2574:T2)
                n1715 = local read "SIG LAB02-1"() -> (w2578:T2)
                n1716 = Bundle By Name(cluster=w2578, "Tmp Live"=w2576, "Tmp Neut"=w2575) -> (w2577:T2)
                n1717 = Bundle By Name(cluster=w2574, "Tmp Live"=w2572, "Tmp Neut"=w2571) -> (w2573:T2)
                n1718 = local write "SIG LAB02-1"(w2577) -> ()
                n1719 = local write "SIG LAB02-2"(w2573) -> ()
              }
              frame #3 {
                n1720 = local read "CAL LAB03"() -> (w2597:T7)
                n1721 = local read "LAB03 TEMP"() -> (w2598:T12)
                n1722 = Unbundle By Name(w2598) -> ("T1 Live"=w2588:dbl, "T1 Neut"=w2587:dbl, "T2 Live"=w2586:dbl, "T2 Neut"=w2585:dbl)  [unwired: 2 out]
                n1723 = Unbundle By Name(w2597) -> ("1 (TL) cal"=w2584:dbl, "1 (TN) cal"=w2583:dbl, "2 (TL) cal"=w2582:dbl, "2 (TN) cal"=w2581:dbl)  [unwired: 6 out]
                n1724 = Multiply(x=w2588, y=w2584) -> (x*y=w2594:dbl)
                n1725 = Multiply(x=w2587, y=w2583) -> (x*y=w2593:dbl)
                n1726 = Multiply(x=w2586, y=w2582) -> (x*y=w2590:dbl)
                n1727 = Multiply(x=w2585, y=w2581) -> (x*y=w2589:dbl)
                n1728 = local read "SIG LAB03-2"() -> (w2592:T2)
                n1729 = local read "SIG LAB03-1"() -> (w2596:T2)
                n1730 = Bundle By Name(cluster=w2596, "Tmp Live"=w2594, "Tmp Neut"=w2593) -> (w2595:T2)
                n1731 = Bundle By Name(cluster=w2592, "Tmp Live"=w2590, "Tmp Neut"=w2589) -> (w2591:T2)
                n1732 = local write "SIG LAB03-1"(w2595) -> ()
                n1733 = local write "SIG LAB03-2"(w2591) -> ()
              }
              frame #4 {
                n1734 = local read "CAL LAB04"() -> (w2615:T7)
                n1735 = local read "LAB04 TEMP"() -> (w2616:T12)
                n1736 = Unbundle By Name(w2616) -> ("T1 Live"=w2606:dbl, "T1 Neut"=w2605:dbl, "T2 Live"=w2604:dbl, "T2 Neut"=w2603:dbl)  [unwired: 2 out]
                n1737 = Unbundle By Name(w2615) -> ("1 (TL) cal"=w2602:dbl, "1 (TN) cal"=w2601:dbl, "2 (TL) cal"=w2600:dbl, "2 (TN) cal"=w2599:dbl)  [unwired: 6 out]
                n1738 = Multiply(x=w2606, y=w2602) -> (x*y=w2612:dbl)
                n1739 = Multiply(x=w2605, y=w2601) -> (x*y=w2611:dbl)
                n1740 = Multiply(x=w2604, y=w2600) -> (x*y=w2608:dbl)
                n1741 = Multiply(x=w2603, y=w2599) -> (x*y=w2607:dbl)
                n1742 = local read "SIG LAB04-2"() -> (w2610:T2)
                n1743 = local read "SIG LAB04-1"() -> (w2614:T2)
                n1744 = Bundle By Name(cluster=w2614, "Tmp Live"=w2612, "Tmp Neut"=w2611) -> (w2613:T2)
                n1745 = Bundle By Name(cluster=w2610, "Tmp Live"=w2608, "Tmp Neut"=w2607) -> (w2609:T2)
                n1746 = local write "SIG LAB04-1"(w2613) -> ()
                n1747 = local write "SIG LAB04-2"(w2609) -> ()
              }
              frame #5 {
                n1748 = local read "CAL LAB05"() -> (w2633:T7)
                n1749 = local read "LAB05 TEMP"() -> (w2634:T12)
                n1750 = Unbundle By Name(w2634) -> ("T1 Live"=w2624:dbl, "T1 Neut"=w2623:dbl, "T2 Live"=w2622:dbl, "T2 Neut"=w2621:dbl)  [unwired: 2 out]
                n1751 = Unbundle By Name(w2633) -> ("1 (TL) cal"=w2620:dbl, "1 (TN) cal"=w2619:dbl, "2 (TL) cal"=w2618:dbl, "2 (TN) cal"=w2617:dbl)  [unwired: 6 out]
                n1752 = Multiply(x=w2624, y=w2620) -> (x*y=w2630:dbl)
                n1753 = Multiply(x=w2623, y=w2619) -> (x*y=w2629:dbl)
                n1754 = Multiply(x=w2622, y=w2618) -> (x*y=w2626:dbl)
                n1755 = Multiply(x=w2621, y=w2617) -> (x*y=w2625:dbl)
                n1756 = local read "SIG LAB05-2"() -> (w2628:T2)
                n1757 = local read "SIG LAB05-1"() -> (w2632:T2)
                n1758 = Bundle By Name(cluster=w2632, "Tmp Live"=w2630, "Tmp Neut"=w2629) -> (w2631:T2)
                n1759 = Bundle By Name(cluster=w2628, "Tmp Live"=w2626, "Tmp Neut"=w2625) -> (w2627:T2)
                n1760 = local write "SIG LAB05-1"(w2631) -> ()
                n1761 = local write "SIG LAB05-2"(w2627) -> ()
              }
            }
          }
          frame #12 {
            # "get analog values"
            n1762 = local read "on loops"() -> (w2641:dbl)
            n1763 = local read "jig cycle"() -> (w2638:dbl)
            n1764 = Add(x=w2641, y=1) -> (x+y=w2639:dbl)
            n1765 = Equal?(x=w2638, y=1) -> (x = y?=w2636:bool)
            n1766 = Equal?(x=w2638, y=w2639) -> (x = y?=w2637:bool)
            n1767 = Or(x=w2636, y=w2637) -> (x .or. y?=w2635:bool)
            n1768 = case shown="True" w2635 {
              frame False {
              }
              frame True {
                n1769 = call "sub vi - Read Analog All v8.vi"() -> ("Analog loop time"=w2649:dbl, "array GRAPH"=w2648:dynamicdata[], "LAB01"=w2647:T22, "LAB02"=w2646:T23, "LAB03"=w2645:T24, "LAB04"=w2644:T25, "array ERROR"=w2650:errorcluster[], "LAB05"=w2643:T26)  [unwired: 8 in]
                n1770 = stacked-sequence {
                  tunnel: w2650 -> [w2655 _ _ _ _ _]
                  tunnel: w2649 -> [w2654 _ _ _ _ _]
                  tunnel: w2648 -> [w2653 _ _ _ _ _]
                  tunnel: w2647 -> [_ w2700 _ _ _ _]
                  tunnel: w2646 -> [_ _ w2701 _ _ _]
                  tunnel: w2645 -> [_ _ _ w2726 _ _]
                  tunnel: w2644 -> [_ _ _ _ w2749 _]
                  tunnel: w2643 -> [_ _ _ _ _ w2774]
                  frame #0 {
                    n1771 = local write "AI update"(TRUE) -> ()
                    n1772 = global write "Global 1.vi" "RATE(Hz)"("RATE (Hz)") -> ()
                    n1773 = global write "Global 1.vi" "SAMPLES"("SAMPLES") -> ()
                    n1774 = Index Array(array=w2653, index=6) -> (element=→"LAB04-1 (GRAPH)":dynamicdata)
                    n1775 = Index Array(array=w2653, index=7) -> (element=→"LAB04-2 (GRAPH)":dynamicdata)
                    n1776 = Index Array(array=w2653, index=9) -> (element=→"LAB05-2 (GRAPH)":dynamicdata)
                    n1777 = Index Array(array=w2653, index=8) -> (element=→"LAB05-1 (GRAPH)":dynamicdata)
                    n1778 = Index Array(array=w2653, index=5) -> (element=→"LAB03-2 (GRAPH)":dynamicdata)
                    n1779 = Index Array(array=w2653, index=0) -> (element=→"LAB01-1 (GRAPH)":dynamicdata)
                    n1780 = Index Array(array=w2653, index=1) -> (element=→"LAB01-2 (GRAPH)":dynamicdata)
                    n1781 = Index Array(array=w2653, index=2) -> (element=→"LAB02-1 (GRAPH)":dynamicdata)
                    n1782 = Index Array(array=w2653, index=3) -> (element=→"LAB02-2 (GRAPH)":dynamicdata)
                    n1783 = Index Array(array=w2653, index=4) -> (element=→"LAB03-1 (GRAPH)":dynamicdata)
                    "AI loop time" <- w2654
                    "Analog Error Array" <- w2655
                  }
                  frame #1 {
                    n1784 = local read "CAL LAB01"() -> (w2699:T7)
                    n1785 = Unbundle By Name(w2700) -> ("LAB01-1 (A)"=w2698:dbl, "LAB01-1 (V)"=w2697:dbl, "LAB01-1 (PF)"=w2696:dbl, "LAB01-2 (A)"=w2695:dbl, "LAB01-2 (V)"=w2694:dbl, "LAB01-2 (PF)"=w2693:dbl)
                    n1786 = Unbundle By Name(w2699) -> ("1  (A) cal"=w2692:dbl, "1 (V) cal"=w2691:dbl, "1 (PF) cal"=w2690:dbl, "2 (A) cal"=w2689:dbl, "2 (V) cal"=w2688:dbl, "2 (PF) cal"=w2687:dbl)  [unwired: 4 out]
                    n1787 = Multiply(x=w2698, y=w2692) -> (x*y=w2685:dbl)
                    n1788 = Multiply(x=w2697, y=w2691) -> (x*y=w2684:dbl)
                    n1789 = Multiply(x=w2696, y=w2690) -> (x*y=w2683:dbl)
                    n1790 = Multiply(x=w2695, y=w2689) -> (x*y=w2679:dbl)
                    n1791 = Multiply(x=w2694, y=w2688) -> (x*y=w2678:dbl)
                    n1792 = Multiply(x=w2693, y=w2687) -> (x*y=w2677:dbl)
                    n1793 = local read "SIG LAB01-1"() -> (w2686:T2)
                    n1794 = local read "SIG LAB01-2"() -> (w2681:T2)
                    n1795 = Bundle By Name(cluster=w2686, "AMPS"=w2685, "VOLTS"=w2684, "PF"=w2683) -> (w2682:T2)
                    n1796 = Bundle By Name(cluster=w2681, "AMPS"=w2679, "VOLTS"=w2678, "PF"=w2677) -> (w2680:T2)
                    n1797 = local write "SIG LAB01-2"(w2680) -> ()
                    n1798 = local write "SIG LAB01-1"(w2682) -> ()
                  }
                  frame #2 {
                    n1799 = local read "CAL LAB02"() -> (w2724:T8)
                    n1800 = Unbundle By Name(w2701) -> ("LAB02-1 (A)"=w2723:dbl, "LAB02-1 (V)"=w2722:dbl, "LAB02-1 (PF)"=w2721:dbl, "LAB02-2 (A)"=w2720:dbl, "LAB02-2 (V)"=w2719:dbl, "LAB02-2 (PF)"=w2718:dbl)
                    n1801 = Unbundle By Name(w2724) -> ("1 (A) cal"=w2717:dbl, "1 (V) cal"=w2716:dbl, "1 (PF) cal"=w2715:dbl, "2 (A) cal"=w2714:dbl, "2 (V) cal"=w2713:dbl, "2 (PF) cal"=w2712:dbl)  [unwired: 4 out]
                    n1802 = Multiply(x=w2723, y=w2717) -> (x*y=w2710:dbl)
                    n1803 = Multiply(x=w2722, y=w2716) -> (x*y=w2709:dbl)
                    n1804 = Multiply(x=w2721, y=w2715) -> (x*y=w2708:dbl)
                    n1805 = Multiply(x=w2720, y=w2714) -> (x*y=w2704:dbl)
                    n1806 = Multiply(x=w2719, y=w2713) -> (x*y=w2703:dbl)
                    n1807 = Multiply(x=w2718, y=w2712) -> (x*y=w2702:dbl)
                    n1808 = local read "SIG LAB02-1"() -> (w2711:T2)
                    n1809 = local read "SIG LAB02-2"() -> (w2706:T2)
                    n1810 = Bundle By Name(cluster=w2711, "AMPS"=w2710, "VOLTS"=w2709, "PF"=w2708) -> (w2707:T2)
                    n1811 = Bundle By Name(cluster=w2706, "AMPS"=w2704, "VOLTS"=w2703, "PF"=w2702) -> (w2705:T2)
                    n1812 = local write "SIG LAB02-2"(w2705) -> ()
                    n1813 = local write "SIG LAB02-1"(w2707) -> ()
                  }
                  frame #3 {
                    n1814 = local read "CAL LAB03"() -> (w2748:T7)
                    n1815 = Unbundle By Name(w2726) -> ("LAB03-1 (A)"=w2747:dbl, "LAB03-1 (V)"=w2746:dbl, "LAB03-1 (PF)"=w2745:dbl, "LAB03-2 (A)"=w2744:dbl, "LAB03-2 (V)"=w2743:dbl, "LAB03-2 (PF)"=w2742:dbl)
                    n1816 = Unbundle By Name(w2748) -> ("1  (A) cal"=w2741:dbl, "1 (V) cal"=w2740:dbl, "1 (PF) cal"=w2739:dbl, "2 (A) cal"=w2738:dbl, "2 (V) cal"=w2737:dbl, "2 (PF) cal"=w2736:dbl)  [unwired: 4 out]
                    n1817 = Multiply(x=w2747, y=w2741) -> (x*y=w2734:dbl)
                    n1818 = Multiply(x=w2746, y=w2740) -> (x*y=w2725:dbl)
                    n1819 = Multiply(x=w2745, y=w2739) -> (x*y=w2733:dbl)
                    n1820 = Multiply(x=w2744, y=w2738) -> (x*y=w2729:dbl)
                    n1821 = Multiply(x=w2743, y=w2737) -> (x*y=w2728:dbl)
                    n1822 = Multiply(x=w2742, y=w2736) -> (x*y=w2727:dbl)
                    n1823 = local read "SIG LAB03-1"() -> (w2735:T2)
                    n1824 = local read "SIG LAB03-2"() -> (w2731:T2)
                    n1825 = Bundle By Name(cluster=w2735, "AMPS"=w2734, "VOLTS"=w2725, "PF"=w2733) -> (w2732:T2)
                    n1826 = Bundle By Name(cluster=w2731, "AMPS"=w2729, "VOLTS"=w2728, "PF"=w2727) -> (w2730:T2)
                    n1827 = local write "SIG LAB03-2"(w2730) -> ()
                    n1828 = local write "SIG LAB03-1"(w2732) -> ()
                  }
                  frame #4 {
                    n1829 = local read "CAL LAB04"() -> (w2772:T7)
                    n1830 = Unbundle By Name(w2749) -> ("LAB04-1 (A)"=w2771:dbl, "LAB04-1 (V)"=w2770:dbl, "LAB04-1 (PF)"=w2769:dbl, "LAB04-2 (A)"=w2768:dbl, "LAB04-2 (V)"=w2767:dbl, "LAB04-2 (PF)"=w2766:dbl)
                    n1831 = Unbundle By Name(w2772) -> ("1  (A) cal"=w2765:dbl, "1 (V) cal"=w2764:dbl, "1 (PF) cal"=w2763:dbl, "2 (A) cal"=w2762:dbl, "2 (V) cal"=w2761:dbl, "2 (PF) cal"=w2760:dbl)  [unwired: 4 out]
                    n1832 = Multiply(x=w2771, y=w2765) -> (x*y=w2758:dbl)
                    n1833 = Multiply(x=w2770, y=w2764) -> (x*y=w2757:dbl)
                    n1834 = Multiply(x=w2769, y=w2763) -> (x*y=w2756:dbl)
                    n1835 = Multiply(x=w2768, y=w2762) -> (x*y=w2752:dbl)
                    n1836 = Multiply(x=w2767, y=w2761) -> (x*y=w2751:dbl)
                    n1837 = Multiply(x=w2766, y=w2760) -> (x*y=w2750:dbl)
                    n1838 = local read "SIG LAB04-1"() -> (w2759:T2)
                    n1839 = local read "SIG LAB04-2"() -> (w2754:T2)
                    n1840 = Bundle By Name(cluster=w2759, "AMPS"=w2758, "VOLTS"=w2757, "PF"=w2756) -> (w2755:T2)
                    n1841 = Bundle By Name(cluster=w2754, "AMPS"=w2752, "VOLTS"=w2751, "PF"=w2750) -> (w2753:T2)
                    n1842 = local write "SIG LAB04-2"(w2753) -> ()
                    n1843 = local write "SIG LAB04-1"(w2755) -> ()
                  }
                  frame #5 {
                    n1844 = local read "CAL LAB05"() -> (w2796:T7)
                    n1845 = Unbundle By Name(w2774) -> ("LAB05-1 (A)"=w2795:dbl, "LAB05-1 (V)"=w2773:dbl, "LAB05-1 (PF)"=w2794:dbl, "LAB05-2 (A)"=w2793:dbl, "LAB05-2 (V)"=w2792:dbl, "LAB05-2 (PF)"=w2791:dbl)
                    n1846 = Unbundle By Name(w2796) -> ("1  (A) cal"=w2790:dbl, "1 (V) cal"=w2789:dbl, "1 (PF) cal"=w2788:dbl, "2 (A) cal"=w2787:dbl, "2 (V) cal"=w2786:dbl, "2 (PF) cal"=w2785:dbl)  [unwired: 4 out]
                    n1847 = Multiply(x=w2795, y=w2790) -> (x*y=w2783:dbl)
                    n1848 = Multiply(x=w2773, y=w2789) -> (x*y=w2782:dbl)
                    n1849 = Multiply(x=w2794, y=w2788) -> (x*y=w2781:dbl)
                    n1850 = Multiply(x=w2793, y=w2787) -> (x*y=w2777:dbl)
                    n1851 = Multiply(x=w2792, y=w2786) -> (x*y=w2776:dbl)
                    n1852 = Multiply(x=w2791, y=w2785) -> (x*y=w2775:dbl)
                    n1853 = local read "SIG LAB05-1"() -> (w2784:T2)
                    n1854 = local read "SIG LAB05-2"() -> (w2779:T2)
                    n1855 = Bundle By Name(cluster=w2784, "AMPS"=w2783, "VOLTS"=w2782, "PF"=w2781) -> (w2780:T2)
                    n1856 = Bundle By Name(cluster=w2779, "AMPS"=w2777, "VOLTS"=w2776, "PF"=w2775) -> (w2778:T2)
                    n1857 = local write "SIG LAB05-2"(w2778) -> ()
                    n1858 = local write "SIG LAB05-1"(w2780) -> ()
                  }
                }
              }
            }
          }
          frame #13 {
            # "save test data to file"
            n1859 = Get Date/Time In Seconds() -> (seconds since 1Jan1904=w2797:timestamp)
            "File Time Stamp" <- w2797
            n1860 = local read "on loops"() -> (w2816:dbl)
            n1861 = local read "jig cycle"() -> (w2813:dbl)
            n1862 = Format Date/Time String(time format string (%c)="%H:%M%:%S", seconds (now)=w2797) -> (date/time string=w2801:string)  [unwired: 1 in]
            n1863 = Add(x=w2816, y=2) -> (x+y=w2814:dbl)
            n1864 = Build Array(w2801) -> (w2800:string[])
            n1865 = Equal?(x=w2813, y=1) -> (x = y?=w2799:bool)
            n1866 = Equal?(x=w2813, y=w2814) -> (x = y?=w2798:bool)
            n1867 = stacked-sequence {
              tunnel: w2812 -> [w2822 _ _ _ _ _ _ _ _ _]
              tunnel: w2811 -> [_ w2898 _ _ _ _ _ _ _ _]
              tunnel: w2810 -> [_ _ w2978 _ _ _ _ _ _ _]
              tunnel: w2809 -> [_ _ _ w3058 _ _ _ _ _ _]
              tunnel: w2808 -> [_ _ _ _ w3138 _ _ _ _ _]
              tunnel: w2807 -> [_ _ _ _ _ w3218 _ _ _ _]
              tunnel: w2806 -> [_ _ _ _ _ _ w3298 _ _ _]
              tunnel: w2805 -> [_ _ _ _ _ _ _ w3378 _ _]
              tunnel: w2804 -> [_ _ _ _ _ _ _ _ w3458 _]
              tunnel: w2803 -> [_ _ _ _ _ _ _ _ _ w3538]
              tunnel: w2800 -> [w2821 w2902 w2982 w3062 w3142 w3222 w3302 w3382 w3462 w3542]
              tunnel: w2799 -> [w2820 w2901 w2981 w3061 w3141 w3221 w3301 w3381 w3461 w3541]
              tunnel: w2798 -> [w2819 w2900 w2980 w3060 w3140 w3220 w3300 w3380 w3460 w3540]
              tunnel: w2797 -> [w2818 w2899 w2979 w3059 w3139 w3219 w3299 w3379 w3459 w3539]
              frame #0 {
                n1868 = case shown="True" w2822 {
                  tunnel: w2821 -> [_ w2827]
                  tunnel: w2820 -> [_ w2826]
                  tunnel: w2819 -> [_ w2824]
                  tunnel: w2818 -> [_ w2823]
                  frame False {
                  }
                  frame True {
                    n1869 = local read "DISP LAB01-1"() -> (w2828:T4)
                    n1870 = local read "SIG LAB01-1"() -> (w2829:T2)
                    n1871 = local read "ON L01-1"() -> (w2825:cluster{"amps":dbl, "volts":dbl, "pf":dbl})
                    n1872 = Unbundle(w2829) -> ("AMPS"=w2835:dbl, "VOLTS"=w2833:dbl, "PF"=w2832:dbl, "Tmp Live"=w2831:dbl, "Tmp Neut"=w2834:dbl)
                    n1873 = Unbundle(w2828) -> ("CYCLE"=w2830:dbl)  [unwired: 2 out]
                    n1874 = stacked-sequence {
                      tunnel: w2835 -> [w2839 w2858]
                      tunnel: w2834 -> [_ w2857]
                      tunnel: w2833 -> [w2838 w2856]
                      tunnel: w2832 -> [w2837 w2855]
                      tunnel: w2831 -> [_ w2854]
                      tunnel: w2830 -> [_ w2853]
                      tunnel: w2827 -> [_ w2852]
                      tunnel: w2826 -> [w2840 _]
                      tunnel: w2825 -> [w2836 w2850]
                      tunnel: w2824 -> [_ w2851]
                      tunnel: w2823 -> [_ w2846]
                      frame #0 {
                        n1875 = case shown="True" w2840 {
                          tunnel: w2839 -> [_ w2845]
                          tunnel: w2838 -> [_ w2844]
                          tunnel: w2837 -> [_ w2843]
                          tunnel: w2836 -> [_ w2841]
                          frame False {
                          }
                          frame True {
                            n1876 = Bundle(cluster=w2841, "amps"=w2845, "volts"=w2844, "pf"=w2843) -> (w2842:cluster{"amps":dbl, "volts":dbl, "pf":dbl})
                            n1877 = local write "ON L01-1"(w2842) -> ()
                          }
                        }
                      }
                      frame #1 {
                        n1878 = Unbundle(w2850) -> ("amps"=w2849:dbl, "volts"=w2848:dbl, "pf"=w2847:dbl)
                        n1879 = case shown="True" w2851 {
                          tunnel: w2858 -> [_ w2859]
                          tunnel: w2857 -> [_ w2897]
                          tunnel: w2856 -> [_ _]
                          tunnel: w2855 -> [_ _]
                          tunnel: w2854 -> [_ w2896]
                          tunnel: w2853 -> [_ w2895]
                          tunnel: w2852 -> [_ w2863]
                          tunnel: w2849 -> [_ w2860]
                          tunnel: w2848 -> [_ w2892]
                          tunnel: w2847 -> [_ w2891]
                          tunnel: w2846 -> [_ w2861]
                          frame False {
                          }
                          frame True {
                            n1880 = local read "TDMS LAB01-1"() -> (w2894:refnum<k34>)
                            n1881 = Build Array(w2892) -> (w2888:dbl[])
                            n1882 = Build Array(w2891) -> (w2887:dbl[])
                            n1883 = Build Array(w2896) -> (w2886:dbl[])
                            n1884 = Build Array(w2897) -> (w2885:dbl[])
                            n1885 = Build Array(w2860) -> (w2890:dbl[])
                            n1886 = Build Array(w2859) -> (w2889:dbl[])
                            n1887 = Build Array(w2895) -> (w2884:dbl[])
                            n1888 = Build Array("AMPS ON", "AMPS OFF", "VOLTS", "PF", "TEMP Live", "TEMP Neut", "CYCLE") -> (w2868:string[])
                            n1889 = Bundle By Name("Y"=w2890, "t0"=w2861) -> (w2883:waveform(dbl))  [unwired: 1 in]
                            n1890 = Bundle By Name("Y"=w2889, "t0"=w2861) -> (w2882:waveform(dbl))  [unwired: 1 in]
                            n1891 = Bundle By Name("Y"=w2888, "t0"=w2861) -> (w2881:waveform(dbl))  [unwired: 1 in]
                            n1892 = Bundle By Name("Y"=w2887, "t0"=w2861) -> (w2880:waveform(dbl))  [unwired: 1 in]
                            n1893 = Bundle By Name("Y"=w2886, "t0"=w2861) -> (w2879:waveform(dbl))  [unwired: 1 in]
                            n1894 = Bundle By Name("Y"=w2885, "t0"=w2861) -> (w2878:waveform(dbl))  [unwired: 1 in]
                            n1895 = Bundle By Name("Y"=w2884, "t0"=w2861) -> (w2877:waveform(dbl))  [unwired: 1 in]
                            n1896 = Build Array(w2883, w2882, w2881, w2880, w2879, w2878, w2877) -> (w2876:waveform(dbl)[])
                            n1897 = TDMS Write(0:w2894, 5:"TEST VALUES", 7:w2868, 9:w2876) -> (4:w2867:refnum<k34>, 6:w2866:string, 15:w2865:errorcluster)  [unwired: 2 in, 1 out]
                            n1898 = TDMS Write(0:w2867, 5:w2866, 7:"TIME", 9:w2863, 11:w2865) -> (15:w2862:errorcluster)  [unwired: 1 in, 3 out]
                            n1899 = local write "data file error"(w2862) -> ()
                          }
                        }
                      }
                    }
                  }
                }
              }
              frame #1 {
                n1900 = case shown="True" w2898 {
                  tunnel: w2902 -> [_ w2907]
                  tunnel: w2901 -> [_ w2906]
                  tunnel: w2900 -> [_ w2904]
                  tunnel: w2899 -> [_ w2903]
                  frame False {
                  }
                  frame True {
                    n1901 = local read "DISP LAB01-2"() -> (w2908:T4)
                    n1902 = local read "SIG LAB01-2"() -> (w2909:T2)
                    n1903 = local read "ON L01-2"() -> (w2905:cluster{"amps":dbl, "volts":dbl, "pf":dbl})
                    n1904 = Unbundle(w2909) -> ("AMPS"=w2915:dbl, "VOLTS"=w2913:dbl, "PF"=w2912:dbl, "Tmp Live"=w2911:dbl, "Tmp Neut"=w2914:dbl)
                    n1905 = Unbundle(w2908) -> ("CYCLE"=w2910:dbl)  [unwired: 2 out]
                    n1906 = stacked-sequence {
                      tunnel: w2915 -> [w2919 w2938]
                      tunnel: w2914 -> [_ w2937]
                      tunnel: w2913 -> [w2918 w2936]
                      tunnel: w2912 -> [w2917 w2935]
                      tunnel: w2911 -> [_ w2934]
                      tunnel: w2910 -> [_ w2933]
                      tunnel: w2907 -> [_ w2932]
                      tunnel: w2906 -> [w2920 _]
                      tunnel: w2905 -> [w2916 w2930]
                      tunnel: w2904 -> [_ w2931]
                      tunnel: w2903 -> [_ w2926]
                      frame #0 {
                        n1907 = case shown="True" w2920 {
                          tunnel: w2919 -> [_ w2925]
                          tunnel: w2918 -> [_ w2924]
                          tunnel: w2917 -> [_ w2923]
                          tunnel: w2916 -> [_ w2921]
                          frame False {
                          }
                          frame True {
                            n1908 = Bundle(cluster=w2921, "amps"=w2925, "volts"=w2924, "pf"=w2923) -> (w2922:cluster{"amps":dbl, "volts":dbl, "pf":dbl})
                            n1909 = local write "ON L01-2"(w2922) -> ()
                          }
                        }
                      }
                      frame #1 {
                        n1910 = Unbundle(w2930) -> ("amps"=w2929:dbl, "volts"=w2928:dbl, "pf"=w2927:dbl)
                        n1911 = case shown="True" w2931 {
                          tunnel: w2938 -> [_ w2970]
                          tunnel: w2937 -> [_ w2977]
                          tunnel: w2936 -> [_ _]
                          tunnel: w2935 -> [_ _]
                          tunnel: w2934 -> [_ w2976]
                          tunnel: w2933 -> [_ w2975]
                          tunnel: w2932 -> [_ w2940]
                          tunnel: w2929 -> [_ w2972]
                          tunnel: w2928 -> [_ w2971]
                          tunnel: w2927 -> [_ w2969]
                          tunnel: w2926 -> [_ w2961]
                          frame False {
                          }
                          frame True {
                            n1912 = local read "TDMS LAB01-2"() -> (w2974:refnum<k34>)
                            n1913 = Build Array(w2971) -> (w2966:dbl[])
                            n1914 = Build Array(w2969) -> (w2965:dbl[])
                            n1915 = Build Array(w2976) -> (w2964:dbl[])
                            n1916 = Build Array(w2977) -> (w2963:dbl[])
                            n1917 = Build Array(w2972) -> (w2968:dbl[])
                            n1918 = Build Array(w2970) -> (w2967:dbl[])
                            n1919 = Build Array(w2975) -> (w2962:dbl[])
                            n1920 = Build Array("AMPS ON", "AMPS OFF", "VOLTS", "PF", "TEMP Live", "TEMP Neut", "CYCLE") -> (w2945:string[])
                            n1921 = Bundle By Name("Y"=w2968, "t0"=w2961) -> (w2960:waveform(dbl))  [unwired: 1 in]
                            n1922 = Bundle By Name("Y"=w2967, "t0"=w2961) -> (w2959:waveform(dbl))  [unwired: 1 in]
                            n1923 = Bundle By Name("Y"=w2966, "t0"=w2961) -> (w2958:waveform(dbl))  [unwired: 1 in]
                            n1924 = Bundle By Name("Y"=w2965, "t0"=w2961) -> (w2957:waveform(dbl))  [unwired: 1 in]
                            n1925 = Bundle By Name("Y"=w2964, "t0"=w2961) -> (w2956:waveform(dbl))  [unwired: 1 in]
                            n1926 = Bundle By Name("Y"=w2963, "t0"=w2961) -> (w2955:waveform(dbl))  [unwired: 1 in]
                            n1927 = Bundle By Name("Y"=w2962, "t0"=w2961) -> (w2954:waveform(dbl))  [unwired: 1 in]
                            n1928 = Build Array(w2960, w2959, w2958, w2957, w2956, w2955, w2954) -> (w2953:waveform(dbl)[])
                            n1929 = TDMS Write(0:w2974, 5:"TEST VALUES", 7:w2945, 9:w2953) -> (4:w2944:refnum<k34>, 6:w2943:string, 15:w2942:errorcluster)  [unwired: 2 in, 1 out]
                            n1930 = TDMS Write(0:w2944, 5:w2943, 7:"TIME", 9:w2940, 11:w2942) -> (15:w2939:errorcluster)  [unwired: 1 in, 3 out]
                            n1931 = local write "data file error"(w2939) -> ()
                          }
                        }
                      }
                    }
                  }
                }
              }
              frame #2 {
                n1932 = case shown="True" w2978 {
                  tunnel: w2982 -> [_ w2987]
                  tunnel: w2981 -> [_ w2986]
                  tunnel: w2980 -> [_ w2984]
                  tunnel: w2979 -> [_ w2983]
                  frame False {
                  }
                  frame True {
                    n1933 = local read "DISP LAB02-1"() -> (w2988:T4)
                    n1934 = local read "SIG LAB02-1"() -> (w2989:T2)
                    n1935 = local read "ON L02-1"() -> (w2985:cluster{"amps":dbl, "volts":dbl, "pf":dbl})
                    n1936 = Unbundle(w2989) -> ("AMPS"=w2995:dbl, "VOLTS"=w2993:dbl, "PF"=w2992:dbl, "Tmp Live"=w2991:dbl, "Tmp Neut"=w2994:dbl)
                    n1937 = Unbundle(w2988) -> ("CYCLE"=w2990:dbl)  [unwired: 2 out]
                    n1938 = stacked-sequence {
                      tunnel: w2995 -> [w2999 w3018]
                      tunnel: w2994 -> [_ w3017]
                      tunnel: w2993 -> [w2998 w3016]
                      tunnel: w2992 -> [w2997 w3015]
                      tunnel: w2991 -> [_ w3014]
                      tunnel: w2990 -> [_ w3013]
                      tunnel: w2987 -> [_ w3012]
                      tunnel: w2986 -> [w3000 _]
                      tunnel: w2985 -> [w2996 w3010]
                      tunnel: w2984 -> [_ w3011]
                      tunnel: w2983 -> [_ w3006]
                      frame #0 {
                        n1939 = case shown="True" w3000 {
                          tunnel: w2999 -> [_ w3005]
                          tunnel: w2998 -> [_ w3004]
                          tunnel: w2997 -> [_ w3003]
                          tunnel: w2996 -> [_ w3001]
                          frame False {
                          }
                          frame True {
                            n1940 = Bundle(cluster=w3001, "amps"=w3005, "volts"=w3004, "pf"=w3003) -> (w3002:cluster{"amps":dbl, "volts":dbl, "pf":dbl})
                            n1941 = local write "ON L02-1"(w3002) -> ()
                          }
                        }
                      }
                      frame #1 {
                        n1942 = Unbundle(w3010) -> ("amps"=w3009:dbl, "volts"=w3008:dbl, "pf"=w3007:dbl)
                        n1943 = case shown="True" w3011 {
                          tunnel: w3018 -> [_ w3050]
                          tunnel: w3017 -> [_ w3057]
                          tunnel: w3016 -> [_ _]
                          tunnel: w3015 -> [_ _]
                          tunnel: w3014 -> [_ w3056]
                          tunnel: w3013 -> [_ w3055]
                          tunnel: w3012 -> [_ w3020]
                          tunnel: w3009 -> [_ w3052]
                          tunnel: w3008 -> [_ w3051]
                          tunnel: w3007 -> [_ w3049]
                          tunnel: w3006 -> [_ w3041]
                          frame False {
                          }
                          frame True {
                            n1944 = local read "TDMS LAB02-1"() -> (w3054:refnum<k34>)
                            n1945 = Build Array(w3051) -> (w3046:dbl[])
                            n1946 = Build Array(w3049) -> (w3045:dbl[])
                            n1947 = Build Array(w3056) -> (w3044:dbl[])
                            n1948 = Build Array(w3057) -> (w3043:dbl[])
                            n1949 = Build Array(w3052) -> (w3048:dbl[])
                            n1950 = Build Array(w3050) -> (w3047:dbl[])
                            n1951 = Build Array(w3055) -> (w3042:dbl[])
                            n1952 = Build Array("AMPS ON", "AMPS OFF", "VOLTS", "PF", "TEMP Live", "TEMP Neut", "CYCLE") -> (w3025:string[])
                            n1953 = Bundle By Name("Y"=w3048, "t0"=w3041) -> (w3040:waveform(dbl))  [unwired: 1 in]
                            n1954 = Bundle By Name("Y"=w3047, "t0"=w3041) -> (w3039:waveform(dbl))  [unwired: 1 in]
                            n1955 = Bundle By Name("Y"=w3046, "t0"=w3041) -> (w3038:waveform(dbl))  [unwired: 1 in]
                            n1956 = Bundle By Name("Y"=w3045, "t0"=w3041) -> (w3037:waveform(dbl))  [unwired: 1 in]
                            n1957 = Bundle By Name("Y"=w3044, "t0"=w3041) -> (w3036:waveform(dbl))  [unwired: 1 in]
                            n1958 = Bundle By Name("Y"=w3043, "t0"=w3041) -> (w3035:waveform(dbl))  [unwired: 1 in]
                            n1959 = Bundle By Name("Y"=w3042, "t0"=w3041) -> (w3034:waveform(dbl))  [unwired: 1 in]
                            n1960 = Build Array(w3040, w3039, w3038, w3037, w3036, w3035, w3034) -> (w3033:waveform(dbl)[])
                            n1961 = TDMS Write(0:w3054, 5:"TEST VALUES", 7:w3025, 9:w3033) -> (4:w3024:refnum<k34>, 6:w3023:string, 15:w3022:errorcluster)  [unwired: 2 in, 1 out]
                            n1962 = TDMS Write(0:w3024, 5:w3023, 7:"TIME", 9:w3020, 11:w3022) -> (15:w3019:errorcluster)  [unwired: 1 in, 3 out]
                            n1963 = local write "data file error"(w3019) -> ()
                          }
                        }
                      }
                    }
                  }
                }
              }
              frame #3 {
                n1964 = case shown="True" w3058 {
                  tunnel: w3062 -> [_ w3067]
                  tunnel: w3061 -> [_ w3066]
                  tunnel: w3060 -> [_ w3064]
                  tunnel: w3059 -> [_ w3063]
                  frame False {
                  }
                  frame True {
                    n1965 = local read "DISP LAB02-2"() -> (w3068:T4)
                    n1966 = local read "SIG LAB02-2"() -> (w3069:T2)
                    n1967 = local read "ON L02-2"() -> (w3065:cluster{"amps":dbl, "volts":dbl, "pf":dbl})
                    n1968 = Unbundle(w3069) -> ("AMPS"=w3075:dbl, "VOLTS"=w3073:dbl, "PF"=w3072:dbl, "Tmp Live"=w3071:dbl, "Tmp Neut"=w3074:dbl)
                    n1969 = Unbundle(w3068) -> ("CYCLE"=w3070:dbl)  [unwired: 2 out]
                    n1970 = stacked-sequence {
                      tunnel: w3075 -> [w3079 w3098]
                      tunnel: w3074 -> [_ w3097]
                      tunnel: w3073 -> [w3078 w3096]
                      tunnel: w3072 -> [w3077 w3095]
                      tunnel: w3071 -> [_ w3094]
                      tunnel: w3070 -> [_ w3093]
                      tunnel: w3067 -> [_ w3092]
                      tunnel: w3066 -> [w3080 _]
                      tunnel: w3065 -> [w3076 w3090]
                      tunnel: w3064 -> [_ w3091]
                      tunnel: w3063 -> [_ w3086]
                      frame #0 {
                        n1971 = case shown="True" w3080 {
                          tunnel: w3079 -> [_ w3085]
                          tunnel: w3078 -> [_ w3084]
                          tunnel: w3077 -> [_ w3083]
                          tunnel: w3076 -> [_ w3081]
                          frame False {
                          }
                          frame True {
                            n1972 = Bundle(cluster=w3081, "amps"=w3085, "volts"=w3084, "pf"=w3083) -> (w3082:cluster{"amps":dbl, "volts":dbl, "pf":dbl})
                            n1973 = local write "ON L02-2"(w3082) -> ()
                          }
                        }
                      }
                      frame #1 {
                        n1974 = Unbundle(w3090) -> ("amps"=w3089:dbl, "volts"=w3088:dbl, "pf"=w3087:dbl)
                        n1975 = case shown="True" w3091 {
                          tunnel: w3098 -> [_ w3130]
                          tunnel: w3097 -> [_ w3137]
                          tunnel: w3096 -> [_ _]
                          tunnel: w3095 -> [_ _]
                          tunnel: w3094 -> [_ w3136]
                          tunnel: w3093 -> [_ w3135]
                          tunnel: w3092 -> [_ w3100]
                          tunnel: w3089 -> [_ w3132]
                          tunnel: w3088 -> [_ w3131]
                          tunnel: w3087 -> [_ w3129]
                          tunnel: w3086 -> [_ w3121]
                          frame False {
                          }
                          frame True {
                            n1976 = local read "TDMS LAB02-2"() -> (w3134:refnum<k34>)
                            n1977 = Build Array(w3131) -> (w3126:dbl[])
                            n1978 = Build Array(w3129) -> (w3125:dbl[])
                            n1979 = Build Array(w3136) -> (w3124:dbl[])
                            n1980 = Build Array(w3137) -> (w3123:dbl[])
                            n1981 = Build Array(w3132) -> (w3128:dbl[])
                            n1982 = Build Array(w3130) -> (w3127:dbl[])
                            n1983 = Build Array(w3135) -> (w3122:dbl[])
                            n1984 = Build Array("AMPS ON", "AMPS OFF", "VOLTS", "PF", "TEMP Live", "TEMP Neut", "CYCLE") -> (w3105:string[])
                            n1985 = Bundle By Name("Y"=w3128, "t0"=w3121) -> (w3120:waveform(dbl))  [unwired: 1 in]
                            n1986 = Bundle By Name("Y"=w3127, "t0"=w3121) -> (w3119:waveform(dbl))  [unwired: 1 in]
                            n1987 = Bundle By Name("Y"=w3126, "t0"=w3121) -> (w3118:waveform(dbl))  [unwired: 1 in]
                            n1988 = Bundle By Name("Y"=w3125, "t0"=w3121) -> (w3117:waveform(dbl))  [unwired: 1 in]
                            n1989 = Bundle By Name("Y"=w3124, "t0"=w3121) -> (w3116:waveform(dbl))  [unwired: 1 in]
                            n1990 = Bundle By Name("Y"=w3123, "t0"=w3121) -> (w3115:waveform(dbl))  [unwired: 1 in]
                            n1991 = Bundle By Name("Y"=w3122, "t0"=w3121) -> (w3114:waveform(dbl))  [unwired: 1 in]
                            n1992 = Build Array(w3120, w3119, w3118, w3117, w3116, w3115, w3114) -> (w3113:waveform(dbl)[])
                            n1993 = TDMS Write(0:w3134, 5:"TEST VALUES", 7:w3105, 9:w3113) -> (4:w3104:refnum<k34>, 6:w3103:string, 15:w3102:errorcluster)  [unwired: 2 in, 1 out]
                            n1994 = TDMS Write(0:w3104, 5:w3103, 7:"TIME", 9:w3100, 11:w3102) -> (15:w3099:errorcluster)  [unwired: 1 in, 3 out]
                            n1995 = local write "data file error"(w3099) -> ()
                          }
                        }
                      }
                    }
                  }
                }
              }
              frame #4 {
                n1996 = case shown="True" w3138 {
                  tunnel: w3142 -> [_ w3147]
                  tunnel: w3141 -> [_ w3146]
                  tunnel: w3140 -> [_ w3144]
                  tunnel: w3139 -> [_ w3143]
                  frame False {
                  }
                  frame True {
                    n1997 = local read "DISP LAB03-1"() -> (w3148:T4)
                    n1998 = local read "SIG LAB03-1"() -> (w3149:T2)
                    n1999 = local read "ON L03-1"() -> (w3145:cluster{"amps":dbl, "volts":dbl, "pf":dbl})
                    n2000 = Unbundle(w3149) -> ("AMPS"=w3155:dbl, "VOLTS"=w3153:dbl, "PF"=w3152:dbl, "Tmp Live"=w3151:dbl, "Tmp Neut"=w3154:dbl)
                    n2001 = Unbundle(w3148) -> ("CYCLE"=w3150:dbl)  [unwired: 2 out]
                    n2002 = stacked-sequence {
                      tunnel: w3155 -> [w3159 w3178]
                      tunnel: w3154 -> [_ w3177]
                      tunnel: w3153 -> [w3158 w3176]
                      tunnel: w3152 -> [w3157 w3175]
                      tunnel: w3151 -> [_ w3174]
                      tunnel: w3150 -> [_ w3173]
                      tunnel: w3147 -> [_ w3172]
                      tunnel: w3146 -> [w3160 _]
                      tunnel: w3145 -> [w3156 w3170]
                      tunnel: w3144 -> [_ w3171]
                      tunnel: w3143 -> [_ w3166]
                      frame #0 {
                        n2003 = case shown="True" w3160 {
                          tunnel: w3159 -> [_ w3165]
                          tunnel: w3158 -> [_ w3164]
                          tunnel: w3157 -> [_ w3163]
                          tunnel: w3156 -> [_ w3161]
                          frame False {
                          }
                          frame True {
                            n2004 = Bundle(cluster=w3161, "amps"=w3165, "volts"=w3164, "pf"=w3163) -> (w3162:cluster{"amps":dbl, "volts":dbl, "pf":dbl})
                            n2005 = local write "ON L03-1"(w3162) -> ()
                          }
                        }
                      }
                      frame #1 {
                        n2006 = Unbundle(w3170) -> ("amps"=w3169:dbl, "volts"=w3168:dbl, "pf"=w3167:dbl)
                        n2007 = case shown="True" w3171 {
                          tunnel: w3178 -> [_ w3210]
                          tunnel: w3177 -> [_ w3217]
                          tunnel: w3176 -> [_ _]
                          tunnel: w3175 -> [_ _]
                          tunnel: w3174 -> [_ w3216]
                          tunnel: w3173 -> [_ w3215]
                          tunnel: w3172 -> [_ w3180]
                          tunnel: w3169 -> [_ w3212]
                          tunnel: w3168 -> [_ w3211]
                          tunnel: w3167 -> [_ w3209]
                          tunnel: w3166 -> [_ w3201]
                          frame False {
                          }
                          frame True {
                            n2008 = local read "TDMS LAB03-1"() -> (w3214:refnum<k34>)
                            n2009 = Build Array(w3211) -> (w3206:dbl[])
                            n2010 = Build Array(w3209) -> (w3205:dbl[])
                            n2011 = Build Array(w3216) -> (w3204:dbl[])
                            n2012 = Build Array(w3217) -> (w3203:dbl[])
                            n2013 = Build Array(w3212) -> (w3208:dbl[])
                            n2014 = Build Array(w3210) -> (w3207:dbl[])
                            n2015 = Build Array(w3215) -> (w3202:dbl[])
                            n2016 = Build Array("AMPS ON", "AMPS OFF", "VOLTS", "PF", "TEMP Live", "TEMP Neut", "CYCLE") -> (w3185:string[])
                            n2017 = Bundle By Name("Y"=w3208, "t0"=w3201) -> (w3200:waveform(dbl))  [unwired: 1 in]
                            n2018 = Bundle By Name("Y"=w3207, "t0"=w3201) -> (w3199:waveform(dbl))  [unwired: 1 in]
                            n2019 = Bundle By Name("Y"=w3206, "t0"=w3201) -> (w3198:waveform(dbl))  [unwired: 1 in]
                            n2020 = Bundle By Name("Y"=w3205, "t0"=w3201) -> (w3197:waveform(dbl))  [unwired: 1 in]
                            n2021 = Bundle By Name("Y"=w3204, "t0"=w3201) -> (w3196:waveform(dbl))  [unwired: 1 in]
                            n2022 = Bundle By Name("Y"=w3203, "t0"=w3201) -> (w3195:waveform(dbl))  [unwired: 1 in]
                            n2023 = Bundle By Name("Y"=w3202, "t0"=w3201) -> (w3194:waveform(dbl))  [unwired: 1 in]
                            n2024 = Build Array(w3200, w3199, w3198, w3197, w3196, w3195, w3194) -> (w3193:waveform(dbl)[])
                            n2025 = TDMS Write(0:w3214, 5:"TEST VALUES", 7:w3185, 9:w3193) -> (4:w3184:refnum<k34>, 6:w3183:string, 15:w3182:errorcluster)  [unwired: 2 in, 1 out]
                            n2026 = TDMS Write(0:w3184, 5:w3183, 7:"TIME", 9:w3180, 11:w3182) -> (15:w3179:errorcluster)  [unwired: 1 in, 3 out]
                            n2027 = local write "data file error"(w3179) -> ()
                          }
                        }
                      }
                    }
                  }
                }
              }
              frame #5 {
                n2028 = case shown="True" w3218 {
                  tunnel: w3222 -> [_ w3227]
                  tunnel: w3221 -> [_ w3226]
                  tunnel: w3220 -> [_ w3224]
                  tunnel: w3219 -> [_ w3223]
                  frame False {
                  }
                  frame True {
                    n2029 = local read "DISP LAB03-2"() -> (w3228:T4)
                    n2030 = local read "SIG LAB03-2"() -> (w3229:T2)
                    n2031 = local read "ON L03-2"() -> (w3225:cluster{"amps":dbl, "volts":dbl, "pf":dbl})
                    n2032 = Unbundle(w3229) -> ("AMPS"=w3235:dbl, "VOLTS"=w3233:dbl, "PF"=w3232:dbl, "Tmp Live"=w3231:dbl, "Tmp Neut"=w3234:dbl)
                    n2033 = Unbundle(w3228) -> ("CYCLE"=w3230:dbl)  [unwired: 2 out]
                    n2034 = stacked-sequence {
                      tunnel: w3235 -> [w3239 w3258]
                      tunnel: w3234 -> [_ w3257]
                      tunnel: w3233 -> [w3238 w3256]
                      tunnel: w3232 -> [w3237 w3255]
                      tunnel: w3231 -> [_ w3254]
                      tunnel: w3230 -> [_ w3253]
                      tunnel: w3227 -> [_ w3252]
                      tunnel: w3226 -> [w3240 _]
                      tunnel: w3225 -> [w3236 w3250]
                      tunnel: w3224 -> [_ w3251]
                      tunnel: w3223 -> [_ w3246]
                      frame #0 {
                        n2035 = case shown="True" w3240 {
                          tunnel: w3239 -> [_ w3245]
                          tunnel: w3238 -> [_ w3244]
                          tunnel: w3237 -> [_ w3243]
                          tunnel: w3236 -> [_ w3241]
                          frame False {
                          }
                          frame True {
                            n2036 = Bundle(cluster=w3241, "amps"=w3245, "volts"=w3244, "pf"=w3243) -> (w3242:cluster{"amps":dbl, "volts":dbl, "pf":dbl})
                            n2037 = local write "ON L03-2"(w3242) -> ()
                          }
                        }
                      }
                      frame #1 {
                        n2038 = Unbundle(w3250) -> ("amps"=w3249:dbl, "volts"=w3248:dbl, "pf"=w3247:dbl)
                        n2039 = case shown="True" w3251 {
                          tunnel: w3258 -> [_ w3290]
                          tunnel: w3257 -> [_ w3297]
                          tunnel: w3256 -> [_ _]
                          tunnel: w3255 -> [_ _]
                          tunnel: w3254 -> [_ w3296]
                          tunnel: w3253 -> [_ w3295]
                          tunnel: w3252 -> [_ w3260]
                          tunnel: w3249 -> [_ w3292]
                          tunnel: w3248 -> [_ w3291]
                          tunnel: w3247 -> [_ w3289]
                          tunnel: w3246 -> [_ w3281]
                          frame False {
                          }
                          frame True {
                            n2040 = local read "TDMS LAB03-2"() -> (w3294:refnum<k34>)
                            n2041 = Build Array(w3291) -> (w3286:dbl[])
                            n2042 = Build Array(w3289) -> (w3285:dbl[])
                            n2043 = Build Array(w3296) -> (w3284:dbl[])
                            n2044 = Build Array(w3297) -> (w3283:dbl[])
                            n2045 = Build Array(w3292) -> (w3288:dbl[])
                            n2046 = Build Array(w3290) -> (w3287:dbl[])
                            n2047 = Build Array(w3295) -> (w3282:dbl[])
                            n2048 = Build Array("AMPS ON", "AMPS OFF", "VOLTS", "PF", "TEMP Live", "TEMP Neut", "CYCLE") -> (w3265:string[])
                            n2049 = Bundle By Name("Y"=w3288, "t0"=w3281) -> (w3280:waveform(dbl))  [unwired: 1 in]
                            n2050 = Bundle By Name("Y"=w3287, "t0"=w3281) -> (w3279:waveform(dbl))  [unwired: 1 in]
                            n2051 = Bundle By Name("Y"=w3286, "t0"=w3281) -> (w3278:waveform(dbl))  [unwired: 1 in]
                            n2052 = Bundle By Name("Y"=w3285, "t0"=w3281) -> (w3277:waveform(dbl))  [unwired: 1 in]
                            n2053 = Bundle By Name("Y"=w3284, "t0"=w3281) -> (w3276:waveform(dbl))  [unwired: 1 in]
                            n2054 = Bundle By Name("Y"=w3283, "t0"=w3281) -> (w3275:waveform(dbl))  [unwired: 1 in]
                            n2055 = Bundle By Name("Y"=w3282, "t0"=w3281) -> (w3274:waveform(dbl))  [unwired: 1 in]
                            n2056 = Build Array(w3280, w3279, w3278, w3277, w3276, w3275, w3274) -> (w3273:waveform(dbl)[])
                            n2057 = TDMS Write(0:w3294, 5:"TEST VALUES", 7:w3265, 9:w3273) -> (4:w3264:refnum<k34>, 6:w3263:string, 15:w3262:errorcluster)  [unwired: 2 in, 1 out]
                            n2058 = TDMS Write(0:w3264, 5:w3263, 7:"TIME", 9:w3260, 11:w3262) -> (15:w3259:errorcluster)  [unwired: 1 in, 3 out]
                            n2059 = local write "data file error"(w3259) -> ()
                          }
                        }
                      }
                    }
                  }
                }
              }
              frame #6 {
                n2060 = case shown="True" w3298 {
                  tunnel: w3302 -> [_ w3307]
                  tunnel: w3301 -> [_ w3306]
                  tunnel: w3300 -> [_ w3304]
                  tunnel: w3299 -> [_ w3303]
                  frame False {
                  }
                  frame True {
                    n2061 = local read "DISP LAB04-1"() -> (w3308:T4)
                    n2062 = local read "SIG LAB04-1"() -> (w3309:T2)
                    n2063 = local read "ON L04-1"() -> (w3305:cluster{"amps":dbl, "volts":dbl, "pf":dbl})
                    n2064 = Unbundle(w3309) -> ("AMPS"=w3315:dbl, "VOLTS"=w3313:dbl, "PF"=w3312:dbl, "Tmp Live"=w3311:dbl, "Tmp Neut"=w3314:dbl)
                    n2065 = Unbundle(w3308) -> ("CYCLE"=w3310:dbl)  [unwired: 2 out]
                    n2066 = stacked-sequence {
                      tunnel: w3315 -> [w3319 w3338]
                      tunnel: w3314 -> [_ w3337]
                      tunnel: w3313 -> [w3318 w3336]
                      tunnel: w3312 -> [w3317 w3335]
                      tunnel: w3311 -> [_ w3334]
                      tunnel: w3310 -> [_ w3333]
                      tunnel: w3307 -> [_ w3332]
                      tunnel: w3306 -> [w3320 _]
                      tunnel: w3305 -> [w3316 w3330]
                      tunnel: w3304 -> [_ w3331]
                      tunnel: w3303 -> [_ w3326]
                      frame #0 {
                        n2067 = case shown="True" w3320 {
                          tunnel: w3319 -> [_ w3325]
                          tunnel: w3318 -> [_ w3324]
                          tunnel: w3317 -> [_ w3323]
                          tunnel: w3316 -> [_ w3321]
                          frame False {
                          }
                          frame True {
                            n2068 = Bundle(cluster=w3321, "amps"=w3325, "volts"=w3324, "pf"=w3323) -> (w3322:cluster{"amps":dbl, "volts":dbl, "pf":dbl})
                            n2069 = local write "ON L04-1"(w3322) -> ()
                          }
                        }
                      }
                      frame #1 {
                        n2070 = Unbundle(w3330) -> ("amps"=w3329:dbl, "volts"=w3328:dbl, "pf"=w3327:dbl)
                        n2071 = case shown="True" w3331 {
                          tunnel: w3338 -> [_ w3370]
                          tunnel: w3337 -> [_ w3377]
                          tunnel: w3336 -> [_ _]
                          tunnel: w3335 -> [_ _]
                          tunnel: w3334 -> [_ w3376]
                          tunnel: w3333 -> [_ w3375]
                          tunnel: w3332 -> [_ w3340]
                          tunnel: w3329 -> [_ w3372]
                          tunnel: w3328 -> [_ w3371]
                          tunnel: w3327 -> [_ w3369]
                          tunnel: w3326 -> [_ w3361]
                          frame False {
                          }
                          frame True {
                            n2072 = local read "TDMS LAB04-1"() -> (w3374:refnum<k34>)
                            n2073 = Build Array(w3371) -> (w3366:dbl[])
                            n2074 = Build Array(w3369) -> (w3365:dbl[])
                            n2075 = Build Array(w3376) -> (w3364:dbl[])
                            n2076 = Build Array(w3377) -> (w3363:dbl[])
                            n2077 = Build Array(w3372) -> (w3368:dbl[])
                            n2078 = Build Array(w3370) -> (w3367:dbl[])
                            n2079 = Build Array(w3375) -> (w3362:dbl[])
                            n2080 = Build Array("AMPS ON", "AMPS OFF", "VOLTS", "PF", "TEMP Live", "TEMP Neut", "CYCLE") -> (w3345:string[])
                            n2081 = Bundle By Name("Y"=w3368, "t0"=w3361) -> (w3360:waveform(dbl))  [unwired: 1 in]
                            n2082 = Bundle By Name("Y"=w3367, "t0"=w3361) -> (w3359:waveform(dbl))  [unwired: 1 in]
                            n2083 = Bundle By Name("Y"=w3366, "t0"=w3361) -> (w3358:waveform(dbl))  [unwired: 1 in]
                            n2084 = Bundle By Name("Y"=w3365, "t0"=w3361) -> (w3357:waveform(dbl))  [unwired: 1 in]
                            n2085 = Bundle By Name("Y"=w3364, "t0"=w3361) -> (w3356:waveform(dbl))  [unwired: 1 in]
                            n2086 = Bundle By Name("Y"=w3363, "t0"=w3361) -> (w3355:waveform(dbl))  [unwired: 1 in]
                            n2087 = Bundle By Name("Y"=w3362, "t0"=w3361) -> (w3354:waveform(dbl))  [unwired: 1 in]
                            n2088 = Build Array(w3360, w3359, w3358, w3357, w3356, w3355, w3354) -> (w3353:waveform(dbl)[])
                            n2089 = TDMS Write(0:w3374, 5:"TEST VALUES", 7:w3345, 9:w3353) -> (4:w3344:refnum<k34>, 6:w3343:string, 15:w3342:errorcluster)  [unwired: 2 in, 1 out]
                            n2090 = TDMS Write(0:w3344, 5:w3343, 7:"TIME", 9:w3340, 11:w3342) -> (15:w3339:errorcluster)  [unwired: 1 in, 3 out]
                            n2091 = local write "data file error"(w3339) -> ()
                          }
                        }
                      }
                    }
                  }
                }
              }
              frame #7 {
                n2092 = case shown="True" w3378 {
                  tunnel: w3382 -> [_ w3387]
                  tunnel: w3381 -> [_ w3386]
                  tunnel: w3380 -> [_ w3384]
                  tunnel: w3379 -> [_ w3383]
                  frame False {
                  }
                  frame True {
                    n2093 = local read "DISP LAB04-2"() -> (w3388:T4)
                    n2094 = local read "SIG LAB04-2"() -> (w3389:T2)
                    n2095 = local read "ON L04-2"() -> (w3385:cluster{"amps":dbl, "volts":dbl, "pf":dbl})
                    n2096 = Unbundle(w3389) -> ("AMPS"=w3395:dbl, "VOLTS"=w3393:dbl, "PF"=w3392:dbl, "Tmp Live"=w3391:dbl, "Tmp Neut"=w3394:dbl)
                    n2097 = Unbundle(w3388) -> ("CYCLE"=w3390:dbl)  [unwired: 2 out]
                    n2098 = stacked-sequence {
                      tunnel: w3395 -> [w3399 w3418]
                      tunnel: w3394 -> [_ w3417]
                      tunnel: w3393 -> [w3398 w3416]
                      tunnel: w3392 -> [w3397 w3415]
                      tunnel: w3391 -> [_ w3414]
                      tunnel: w3390 -> [_ w3413]
                      tunnel: w3387 -> [_ w3412]
                      tunnel: w3386 -> [w3400 _]
                      tunnel: w3385 -> [w3396 w3410]
                      tunnel: w3384 -> [_ w3411]
                      tunnel: w3383 -> [_ w3406]
                      frame #0 {
                        n2099 = case shown="True" w3400 {
                          tunnel: w3399 -> [_ w3405]
                          tunnel: w3398 -> [_ w3404]
                          tunnel: w3397 -> [_ w3403]
                          tunnel: w3396 -> [_ w3401]
                          frame False {
                          }
                          frame True {
                            n2100 = Bundle(cluster=w3401, "amps"=w3405, "volts"=w3404, "pf"=w3403) -> (w3402:cluster{"amps":dbl, "volts":dbl, "pf":dbl})
                            n2101 = local write "ON L04-2"(w3402) -> ()
                          }
                        }
                      }
                      frame #1 {
                        n2102 = Unbundle(w3410) -> ("amps"=w3409:dbl, "volts"=w3408:dbl, "pf"=w3407:dbl)
                        n2103 = case shown="True" w3411 {
                          tunnel: w3418 -> [_ w3450]
                          tunnel: w3417 -> [_ w3457]
                          tunnel: w3416 -> [_ _]
                          tunnel: w3415 -> [_ _]
                          tunnel: w3414 -> [_ w3456]
                          tunnel: w3413 -> [_ w3455]
                          tunnel: w3412 -> [_ w3420]
                          tunnel: w3409 -> [_ w3452]
                          tunnel: w3408 -> [_ w3451]
                          tunnel: w3407 -> [_ w3449]
                          tunnel: w3406 -> [_ w3441]
                          frame False {
                          }
                          frame True {
                            n2104 = local read "TDMS LAB04-2"() -> (w3454:refnum<k34>)
                            n2105 = Build Array(w3451) -> (w3446:dbl[])
                            n2106 = Build Array(w3449) -> (w3445:dbl[])
                            n2107 = Build Array(w3456) -> (w3444:dbl[])
                            n2108 = Build Array(w3457) -> (w3443:dbl[])
                            n2109 = Build Array(w3452) -> (w3448:dbl[])
                            n2110 = Build Array(w3450) -> (w3447:dbl[])
                            n2111 = Build Array(w3455) -> (w3442:dbl[])
                            n2112 = Build Array("AMPS ON", "AMPS OFF", "VOLTS", "PF", "TEMP Live", "TEMP Neut", "CYCLE") -> (w3425:string[])
                            n2113 = Bundle By Name("Y"=w3448, "t0"=w3441) -> (w3440:waveform(dbl))  [unwired: 1 in]
                            n2114 = Bundle By Name("Y"=w3447, "t0"=w3441) -> (w3439:waveform(dbl))  [unwired: 1 in]
                            n2115 = Bundle By Name("Y"=w3446, "t0"=w3441) -> (w3438:waveform(dbl))  [unwired: 1 in]
                            n2116 = Bundle By Name("Y"=w3445, "t0"=w3441) -> (w3437:waveform(dbl))  [unwired: 1 in]
                            n2117 = Bundle By Name("Y"=w3444, "t0"=w3441) -> (w3436:waveform(dbl))  [unwired: 1 in]
                            n2118 = Bundle By Name("Y"=w3443, "t0"=w3441) -> (w3435:waveform(dbl))  [unwired: 1 in]
                            n2119 = Bundle By Name("Y"=w3442, "t0"=w3441) -> (w3434:waveform(dbl))  [unwired: 1 in]
                            n2120 = Build Array(w3440, w3439, w3438, w3437, w3436, w3435, w3434) -> (w3433:waveform(dbl)[])
                            n2121 = TDMS Write(0:w3454, 5:"TEST VALUES", 7:w3425, 9:w3433) -> (4:w3424:refnum<k34>, 6:w3423:string, 15:w3422:errorcluster)  [unwired: 2 in, 1 out]
                            n2122 = TDMS Write(0:w3424, 5:w3423, 7:"TIME", 9:w3420, 11:w3422) -> (15:w3419:errorcluster)  [unwired: 1 in, 3 out]
                            n2123 = local write "data file error"(w3419) -> ()
                          }
                        }
                      }
                    }
                  }
                }
              }
              frame #8 {
                n2124 = case shown="True" w3458 {
                  tunnel: w3462 -> [_ w3467]
                  tunnel: w3461 -> [_ w3466]
                  tunnel: w3460 -> [_ w3464]
                  tunnel: w3459 -> [_ w3463]
                  frame False {
                  }
                  frame True {
                    n2125 = local read "DISP LAB05-1"() -> (w3468:T4)
                    n2126 = local read "SIG LAB05-1"() -> (w3469:T2)
                    n2127 = local read "ON L05-1"() -> (w3465:cluster{"amps":dbl, "volts":dbl, "pf":dbl})
                    n2128 = Unbundle(w3469) -> ("AMPS"=w3475:dbl, "VOLTS"=w3473:dbl, "PF"=w3472:dbl, "Tmp Live"=w3471:dbl, "Tmp Neut"=w3474:dbl)
                    n2129 = Unbundle(w3468) -> ("CYCLE"=w3470:dbl)  [unwired: 2 out]
                    n2130 = stacked-sequence {
                      tunnel: w3475 -> [w3479 w3498]
                      tunnel: w3474 -> [_ w3497]
                      tunnel: w3473 -> [w3478 w3496]
                      tunnel: w3472 -> [w3477 w3495]
                      tunnel: w3471 -> [_ w3494]
                      tunnel: w3470 -> [_ w3493]
                      tunnel: w3467 -> [_ w3492]
                      tunnel: w3466 -> [w3480 _]
                      tunnel: w3465 -> [w3476 w3490]
                      tunnel: w3464 -> [_ w3491]
                      tunnel: w3463 -> [_ w3486]
                      frame #0 {
                        n2131 = case shown="True" w3480 {
                          tunnel: w3479 -> [_ w3485]
                          tunnel: w3478 -> [_ w3484]
                          tunnel: w3477 -> [_ w3483]
                          tunnel: w3476 -> [_ w3481]
                          frame False {
                          }
                          frame True {
                            n2132 = Bundle(cluster=w3481, "amps"=w3485, "volts"=w3484, "pf"=w3483) -> (w3482:cluster{"amps":dbl, "volts":dbl, "pf":dbl})
                            n2133 = local write "ON L05-1"(w3482) -> ()
                          }
                        }
                      }
                      frame #1 {
                        n2134 = Unbundle(w3490) -> ("amps"=w3489:dbl, "volts"=w3488:dbl, "pf"=w3487:dbl)
                        n2135 = case shown="True" w3491 {
                          tunnel: w3498 -> [_ w3530]
                          tunnel: w3497 -> [_ w3537]
                          tunnel: w3496 -> [_ _]
                          tunnel: w3495 -> [_ _]
                          tunnel: w3494 -> [_ w3536]
                          tunnel: w3493 -> [_ w3535]
                          tunnel: w3492 -> [_ w3500]
                          tunnel: w3489 -> [_ w3532]
                          tunnel: w3488 -> [_ w3531]
                          tunnel: w3487 -> [_ w3529]
                          tunnel: w3486 -> [_ w3521]
                          frame False {
                          }
                          frame True {
                            n2136 = local read "TDMS LAB05-1"() -> (w3534:refnum<k34>)
                            n2137 = Build Array(w3531) -> (w3526:dbl[])
                            n2138 = Build Array(w3529) -> (w3525:dbl[])
                            n2139 = Build Array(w3536) -> (w3524:dbl[])
                            n2140 = Build Array(w3537) -> (w3523:dbl[])
                            n2141 = Build Array(w3532) -> (w3528:dbl[])
                            n2142 = Build Array(w3530) -> (w3527:dbl[])
                            n2143 = Build Array(w3535) -> (w3522:dbl[])
                            n2144 = Build Array("AMPS ON", "AMPS OFF", "VOLTS", "PF", "TEMP Live", "TEMP Neut", "CYCLE") -> (w3505:string[])
                            n2145 = Bundle By Name("Y"=w3528, "t0"=w3521) -> (w3520:waveform(dbl))  [unwired: 1 in]
                            n2146 = Bundle By Name("Y"=w3527, "t0"=w3521) -> (w3519:waveform(dbl))  [unwired: 1 in]
                            n2147 = Bundle By Name("Y"=w3526, "t0"=w3521) -> (w3518:waveform(dbl))  [unwired: 1 in]
                            n2148 = Bundle By Name("Y"=w3525, "t0"=w3521) -> (w3517:waveform(dbl))  [unwired: 1 in]
                            n2149 = Bundle By Name("Y"=w3524, "t0"=w3521) -> (w3516:waveform(dbl))  [unwired: 1 in]
                            n2150 = Bundle By Name("Y"=w3523, "t0"=w3521) -> (w3515:waveform(dbl))  [unwired: 1 in]
                            n2151 = Bundle By Name("Y"=w3522, "t0"=w3521) -> (w3514:waveform(dbl))  [unwired: 1 in]
                            n2152 = Build Array(w3520, w3519, w3518, w3517, w3516, w3515, w3514) -> (w3513:waveform(dbl)[])
                            n2153 = TDMS Write(0:w3534, 5:"TEST VALUES", 7:w3505, 9:w3513) -> (4:w3504:refnum<k34>, 6:w3503:string, 15:w3502:errorcluster)  [unwired: 2 in, 1 out]
                            n2154 = TDMS Write(0:w3504, 5:w3503, 7:"TIME", 9:w3500, 11:w3502) -> (15:w3499:errorcluster)  [unwired: 1 in, 3 out]
                            n2155 = local write "data file error"(w3499) -> ()
                          }
                        }
                      }
                    }
                  }
                }
              }
              frame #9 {
                n2156 = case shown="True" w3538 {
                  tunnel: w3542 -> [_ w3547]
                  tunnel: w3541 -> [_ w3546]
                  tunnel: w3540 -> [_ w3544]
                  tunnel: w3539 -> [_ w3543]
                  frame False {
                  }
                  frame True {
                    n2157 = local read "DISP LAB05-2"() -> (w3548:T4)
                    n2158 = local read "SIG LAB05-2"() -> (w3549:T2)
                    n2159 = local read "ON L05-2"() -> (w3545:cluster{"amps":dbl, "volts":dbl, "pf":dbl})
                    n2160 = Unbundle(w3549) -> ("AMPS"=w3555:dbl, "VOLTS"=w3553:dbl, "PF"=w3552:dbl, "Tmp Live"=w3551:dbl, "Tmp Neut"=w3554:dbl)
                    n2161 = Unbundle(w3548) -> ("CYCLE"=w3550:dbl)  [unwired: 2 out]
                    n2162 = stacked-sequence {
                      tunnel: w3555 -> [w3559 w3578]
                      tunnel: w3554 -> [_ w3577]
                      tunnel: w3553 -> [w3558 w3576]
                      tunnel: w3552 -> [w3557 w3575]
                      tunnel: w3551 -> [_ w3574]
                      tunnel: w3550 -> [_ w3573]
                      tunnel: w3547 -> [_ w3572]
                      tunnel: w3546 -> [w3560 _]
                      tunnel: w3545 -> [w3556 w3570]
                      tunnel: w3544 -> [_ w3571]
                      tunnel: w3543 -> [_ w3566]
                      frame #0 {
                        n2163 = case shown="True" w3560 {
                          tunnel: w3559 -> [_ w3565]
                          tunnel: w3558 -> [_ w3564]
                          tunnel: w3557 -> [_ w3563]
                          tunnel: w3556 -> [_ w3561]
                          frame False {
                          }
                          frame True {
                            n2164 = Bundle(cluster=w3561, "amps"=w3565, "volts"=w3564, "pf"=w3563) -> (w3562:cluster{"amps":dbl, "volts":dbl, "pf":dbl})
                            n2165 = local write "ON L05-2"(w3562) -> ()
                          }
                        }
                      }
                      frame #1 {
                        n2166 = Unbundle(w3570) -> ("amps"=w3569:dbl, "volts"=w3568:dbl, "pf"=w3567:dbl)
                        n2167 = case shown="True" w3571 {
                          tunnel: w3578 -> [_ w3610]
                          tunnel: w3577 -> [_ w3617]
                          tunnel: w3576 -> [_ _]
                          tunnel: w3575 -> [_ _]
                          tunnel: w3574 -> [_ w3616]
                          tunnel: w3573 -> [_ w3615]
                          tunnel: w3572 -> [_ w3580]
                          tunnel: w3569 -> [_ w3612]
                          tunnel: w3568 -> [_ w3611]
                          tunnel: w3567 -> [_ w3609]
                          tunnel: w3566 -> [_ w3601]
                          frame False {
                          }
                          frame True {
                            n2168 = local read "TDMS LAB05-2"() -> (w3614:refnum<k34>)
                            n2169 = Build Array(w3611) -> (w3606:dbl[])
                            n2170 = Build Array(w3609) -> (w3605:dbl[])
                            n2171 = Build Array(w3616) -> (w3604:dbl[])
                            n2172 = Build Array(w3617) -> (w3603:dbl[])
                            n2173 = Build Array(w3612) -> (w3608:dbl[])
                            n2174 = Build Array(w3610) -> (w3607:dbl[])
                            n2175 = Build Array(w3615) -> (w3602:dbl[])
                            n2176 = Build Array("AMPS ON", "AMPS OFF", "VOLTS", "PF", "TEMP Live", "TEMP Neut", "CYCLE") -> (w3585:string[])
                            n2177 = Bundle By Name("Y"=w3608, "t0"=w3601) -> (w3600:waveform(dbl))  [unwired: 1 in]
                            n2178 = Bundle By Name("Y"=w3607, "t0"=w3601) -> (w3599:waveform(dbl))  [unwired: 1 in]
                            n2179 = Bundle By Name("Y"=w3606, "t0"=w3601) -> (w3598:waveform(dbl))  [unwired: 1 in]
                            n2180 = Bundle By Name("Y"=w3605, "t0"=w3601) -> (w3597:waveform(dbl))  [unwired: 1 in]
                            n2181 = Bundle By Name("Y"=w3604, "t0"=w3601) -> (w3596:waveform(dbl))  [unwired: 1 in]
                            n2182 = Bundle By Name("Y"=w3603, "t0"=w3601) -> (w3595:waveform(dbl))  [unwired: 1 in]
                            n2183 = Bundle By Name("Y"=w3602, "t0"=w3601) -> (w3594:waveform(dbl))  [unwired: 1 in]
                            n2184 = Build Array(w3600, w3599, w3598, w3597, w3596, w3595, w3594) -> (w3593:waveform(dbl)[])
                            n2185 = TDMS Write(0:w3614, 5:"TEST VALUES", 7:w3585, 9:w3593) -> (4:w3584:refnum<k34>, 6:w3583:string, 15:w3582:errorcluster)  [unwired: 2 in, 1 out]
                            n2186 = TDMS Write(0:w3584, 5:w3583, 7:"TIME", 9:w3580, 11:w3582) -> (15:w3579:errorcluster)  [unwired: 1 in, 3 out]
                            n2187 = local write "data file error"(w3579) -> ()
                          }
                        }
                      }
                    }
                  }
                }
              }
            }
          }
          frame #14 {
            # "display test values on chart"
            n2188 = case shown="\"OFF CYCLE\"" "Select  Cycle" {
              tunnel: [1 w3623] -> w3618
              frame "ON CYCLE", Default {
              }
              frame "OFF CYCLE" {
                n2189 = local read "on loops"() -> (w3625:dbl)
                n2190 = Add(x=w3625, y=2) -> (x+y=w3623:dbl)
              }
            }
            n2191 = local read "jig cycle"() -> (w3620:dbl)
            n2192 = Equal?(x=w3620, y=w3618) -> (x = y?=w3621:bool)
            n2193 = case shown="True" w3621 {
              frame False {
              }
              frame True {
                n2194 = local read "SIG LAB05-1"() -> (w3667:T2)
                n2195 = local read "SIG LAB04-2"() -> (w3668:T2)
                n2196 = local read "SIG LAB05-2"() -> (w3666:T2)
                n2197 = local read "SIG LAB04-1"() -> (w3669:T2)
                n2198 = local read "SIG LAB03-1"() -> (w3671:T2)
                n2199 = local read "SIG LAB03-2"() -> (w3670:T2)
                n2200 = local read "SIG LAB01-1"() -> (w3675:T2)
                n2201 = local read "SIG LAB02-2"() -> (w3672:T2)
                n2202 = local read "SIG LAB02-1"() -> (w3673:T2)
                n2203 = local read "SIG LAB01-2"() -> (w3674:T2)
                n2204 = Unbundle(w3668) -> ("AMPS"=w3658:dbl, "VOLTS"=w3648:dbl, "Tmp Live"=w3638:dbl, "Tmp Neut"=w3628:dbl)  [unwired: 1 out]
                n2205 = Unbundle(w3667) -> ("AMPS"=w3657:dbl, "VOLTS"=w3647:dbl, "Tmp Live"=w3637:dbl, "Tmp Neut"=w3627:dbl)  [unwired: 1 out]
                n2206 = Unbundle(w3666) -> ("AMPS"=w3656:dbl, "VOLTS"=w3646:dbl, "Tmp Live"=w3636:dbl, "Tmp Neut"=w3626:dbl)  [unwired: 1 out]
                n2207 = Unbundle(w3669) -> ("AMPS"=w3659:dbl, "VOLTS"=w3649:dbl, "Tmp Live"=w3639:dbl, "Tmp Neut"=w3629:dbl)  [unwired: 1 out]
                n2208 = Unbundle(w3670) -> ("AMPS"=w3660:dbl, "VOLTS"=w3650:dbl, "Tmp Live"=w3640:dbl, "Tmp Neut"=w3630:dbl)  [unwired: 1 out]
                n2209 = Unbundle(w3671) -> ("AMPS"=w3661:dbl, "VOLTS"=w3651:dbl, "Tmp Live"=w3641:dbl, "Tmp Neut"=w3631:dbl)  [unwired: 1 out]
                n2210 = Unbundle(w3672) -> ("AMPS"=w3662:dbl, "VOLTS"=w3652:dbl, "Tmp Live"=w3642:dbl, "Tmp Neut"=w3632:dbl)  [unwired: 1 out]
                n2211 = Unbundle(w3673) -> ("AMPS"=w3663:dbl, "VOLTS"=w3653:dbl, "Tmp Live"=w3643:dbl, "Tmp Neut"=w3633:dbl)  [unwired: 1 out]
                n2212 = Unbundle(w3675) -> ("AMPS"=w3665:dbl, "VOLTS"=w3655:dbl, "Tmp Live"=w3645:dbl, "Tmp Neut"=w3635:dbl)  [unwired: 1 out]
                n2213 = Unbundle(w3674) -> ("AMPS"=w3664:dbl, "VOLTS"=w3654:dbl, "Tmp Live"=w3644:dbl, "Tmp Neut"=w3634:dbl)  [unwired: 1 out]
                n2214 = stacked-sequence {
                  tunnel: w3665 -> [w3686 _ _ _]
                  tunnel: w3664 -> [w3685 _ _ _]
                  tunnel: w3663 -> [w3684 _ _ _]
                  tunnel: w3662 -> [w3683 _ _ _]
                  tunnel: w3661 -> [w3682 _ _ _]
                  tunnel: w3660 -> [w3681 _ _ _]
                  tunnel: w3659 -> [w3680 _ _ _]
                  tunnel: w3658 -> [w3679 _ _ _]
                  tunnel: w3657 -> [w3678 _ _ _]
                  tunnel: w3656 -> [w3677 _ _ _]
                  tunnel: w3655 -> [_ w3697 _ _]
                  tunnel: w3654 -> [_ w3696 _ _]
                  tunnel: w3653 -> [_ w3695 _ _]
                  tunnel: w3652 -> [_ w3694 _ _]
                  tunnel: w3651 -> [_ w3693 _ _]
                  tunnel: w3650 -> [_ w3692 _ _]
                  tunnel: w3649 -> [_ w3691 _ _]
                  tunnel: w3648 -> [_ w3690 _ _]
                  tunnel: w3647 -> [_ w3689 _ _]
                  tunnel: w3646 -> [_ w3688 _ _]
                  tunnel: w3645 -> [_ _ w3708 _]
                  tunnel: w3644 -> [_ _ w3707 _]
                  tunnel: w3643 -> [_ _ w3706 _]
                  tunnel: w3642 -> [_ _ w3705 _]
                  tunnel: w3641 -> [_ _ w3704 _]
                  tunnel: w3640 -> [_ _ w3703 _]
                  tunnel: w3639 -> [_ _ w3702 _]
                  tunnel: w3638 -> [_ _ w3701 _]
                  tunnel: w3637 -> [_ _ w3700 _]
                  tunnel: w3636 -> [_ _ w3699 _]
                  tunnel: w3635 -> [_ _ _ w3719]
                  tunnel: w3634 -> [_ _ _ w3718]
                  tunnel: w3633 -> [_ _ _ w3717]
                  tunnel: w3632 -> [_ _ _ w3716]
                  tunnel: w3631 -> [_ _ _ w3715]
                  tunnel: w3630 -> [_ _ _ w3714]
                  tunnel: w3629 -> [_ _ _ w3713]
                  tunnel: w3628 -> [_ _ _ w3712]
                  tunnel: w3627 -> [_ _ _ w3711]
                  tunnel: w3626 -> [_ _ _ w3710]
                  frame #0 {
                    n2215 = Bundle("AMPS"=w3686, "AMPS"=w3685, "AMPS"=w3684, "AMPS"=w3683, "AMPS"=w3682, "AMPS"=w3681, "AMPS"=w3680, "AMPS"=w3679, "AMPS"=w3678, "AMPS"=w3677) -> (→"TEST AMPS CHART":T9)  [unwired: 1 in]
                  }
                  frame #1 {
                    n2216 = Bundle("VOLTS"=w3697, "VOLTS"=w3696, "VOLTS"=w3695, "VOLTS"=w3694, "VOLTS"=w3693, "VOLTS"=w3692, "VOLTS"=w3691, "VOLTS"=w3690, "VOLTS"=w3689, "VOLTS"=w3688) -> (→"TEST VOLTS CHART":T27)  [unwired: 1 in]
                  }
                  frame #2 {
                    n2217 = Bundle("Tmp Live"=w3708, "Tmp Live"=w3707, "Tmp Live"=w3706, "Tmp Live"=w3705, "Tmp Live"=w3704, "Tmp Live"=w3703, "Tmp Live"=w3702, "Tmp Live"=w3701, "Tmp Live"=w3700, "Tmp Live"=w3699) -> (→"TEMPERATURE (L) CHART":T28)  [unwired: 1 in]
                  }
                  frame #3 {
                    n2218 = Bundle("Tmp Neut"=w3719, "Tmp Neut"=w3718, "Tmp Neut"=w3717, "Tmp Neut"=w3716, "Tmp Neut"=w3715, "Tmp Neut"=w3714, "Tmp Neut"=w3713, "Tmp Neut"=w3712, "Tmp Neut"=w3711, "Tmp Neut"=w3710) -> (→"TEMPERATURE (N) CHART":T29)  [unwired: 1 in]
                  }
                }
              }
            }
          }
          frame #15 {
            # "check for amps fail"
            # "check for cycle test & temperature rise fail conditions"
            n2219 = local read "on loops"() -> (w3745:dbl)
            n2220 = local read "jig cycle"() -> (w3742:dbl)
            n2221 = local read "jig cycle"() -> (w3747:dbl)
            n2222 = Add(x=w3745, y=3.0) -> (x+y=w3743:dbl)
            n2223 = Equal?(x=w3742, y=w3743) -> (x = y?=w3738:bool)
            n2224 = Equal?(x=w3747, y=1.0) -> (x = y?=w3740:bool)
            n2225 = stacked-sequence {
              tunnel: w3741 -> [w3750 _ _ _ _ _ _ _ _ _]
              tunnel: w3740 -> [w3751 w3771 w3791 w3811 w3831 w3851 w3871 w3891 w3911 w3931]
              tunnel: w3739 -> [w3748 _ _ _ _ _ _ _ _ _]
              tunnel: w3738 -> [w3749 w3770 w3790 w3810 w3830 w3850 w3870 w3890 w3910 w3930]
              tunnel: w3737 -> [_ w3769 _ _ _ _ _ _ _ _]
              tunnel: w3736 -> [_ w3768 _ _ _ _ _ _ _ _]
              tunnel: w3735 -> [_ _ w3789 _ _ _ _ _ _ _]
              tunnel: w3734 -> [_ _ w3788 _ _ _ _ _ _ _]
              tunnel: w3733 -> [_ _ _ w3809 _ _ _ _ _ _]
              tunnel: w3732 -> [_ _ _ w3808 _ _ _ _ _ _]
              tunnel: w3731 -> [_ _ _ _ w3829 _ _ _ _ _]
              tunnel: w3730 -> [_ _ _ _ w3828 _ _ _ _ _]
              tunnel: w3729 -> [_ _ _ _ _ w3849 _ _ _ _]
              tunnel: w3728 -> [_ _ _ _ _ w3848 _ _ _ _]
              tunnel: w3727 -> [_ _ _ _ _ _ w3869 _ _ _]
              tunnel: w3726 -> [_ _ _ _ _ _ w3868 _ _ _]
              tunnel: w3725 -> [_ _ _ _ _ _ _ w3889 _ _]
              tunnel: w3724 -> [_ _ _ _ _ _ _ w3888 _ _]
              tunnel: w3723 -> [_ _ _ _ _ _ _ _ w3909 _]
              tunnel: w3722 -> [_ _ _ _ _ _ _ _ w3908 _]
              tunnel: w3721 -> [_ _ _ _ _ _ _ _ _ w3929]
              tunnel: w3720 -> [_ _ _ _ _ _ _ _ _ w3928]
              frame #0 {
                # "LAB01-1"
                n2226 = case shown="True" w3748 {
                  tunnel: w3751 -> [_ w3764]
                  tunnel: w3750 -> [_ w3761]
                  tunnel: w3749 -> [_ w3760]
                  frame False {
                  }
                  frame True {
                    n2227 = local read "TEMP START LAB01-1"() -> (w3766:cluster{"TL":dbl, "TN":dbl})
                    n2228 = local read "RESULT LAB01-1"() -> (w3755:bool)
                    n2229 = local read "FAIL LAB01-1"() -> (w3758:cluster{"LO":dbl, "HI":dbl})
                    n2230 = local read "TDMS LAB01-1"() -> (w3765:refnum<k34>)
                    n2231 = local read "SET LAB01-1"() -> (w3762:T5)
                    n2232 = local read "DISP LAB01-1"() -> (w3763:T4)
                    n2233 = local read "SIG LAB01-1"() -> (w3767:T2)
                    n2234 = Bundle("FAIL LAB01-1"=w3758, "SIG LAB01-1"=w3767, "TEMP START LAB01-1"=w3766, "DISP LAB01-1"=w3763, "SET LAB01-1"=w3762, "TDMS LAB01-1"=w3765) -> (w3752:T30)  [unwired: 1 in]
                    n2235 = call "sub vi - cycle&temp fail v6.vi"("Amps Lo?"=w3764, "Input Cluster"=w3752, "SELECT"=w3761, "Amps Hi?"=w3760, "Result In"=w3755) -> ("(FAIL) out"=w3757:cluster{"FAIL LO":dbl, "FAIL HI":dbl}, "(DISP) out"=w3753:T4, "T-RISE"=w3754:cluster{"T-RISE (L)":dbl, "T-RISE (N)":dbl}, "Result Out"=w3756:bool, "file error"=w3759:errorcluster)  [unwired: 10 in]
                    n2236 = local write "TEMP RISE LAB01-1"(w3754) -> ()
                    n2237 = local write "FAIL LAB01-1"(w3757) -> ()
                    n2238 = local write "DISP LAB01-1"(w3753) -> ()
                    n2239 = local write "RESULT LAB01-1"(w3756) -> ()
                    n2240 = local write "data file error"(w3759) -> ()
                  }
                }
              }
              frame #1 {
                # "LAB01-2"
                n2241 = case shown="True" w3769 {
                  tunnel: w3771 -> [_ w3784]
                  tunnel: w3768 -> [_ w3781]
                  tunnel: w3770 -> [_ w3780]
                  frame False {
                  }
                  frame True {
                    n2242 = local read "TEMP START LAB01-2"() -> (w3786:cluster{"TL":dbl, "TN":dbl})
                    n2243 = local read "FAIL LAB01-2"() -> (w3777:cluster{"LO":dbl, "HI":dbl})
                    n2244 = local read "TDMS LAB01-2"() -> (w3785:refnum<k34>)
                    n2245 = local read "SET LAB01-2"() -> (w3782:T5)
                    n2246 = local read "DISP LAB01-2"() -> (w3783:T4)
                    n2247 = local read "RESULT LAB01-2"() -> (w3774:bool)
                    n2248 = local read "SIG LAB01-2"() -> (w3787:T2)
                    n2249 = Bundle("FAIL LAB01-2"=w3777, "SIG LAB01-2"=w3787, "TEMP START LAB01-2"=w3786, "DISP LAB01-2"=w3783, "SET LAB01-2"=w3782, "TDMS LAB01-2"=w3785) -> (w3772:T31)  [unwired: 1 in]
                    n2250 = call "sub vi - cycle&temp fail v6.vi"("Amps Lo?"=w3784, "Input Cluster"=w3772, "SELECT"=w3781, "Amps Hi?"=w3780, "Result In"=w3774) -> ("(FAIL) out"=w3776:cluster{"FAIL LO":dbl, "FAIL HI":dbl}, "(DISP) out"=w3779:T4, "T-RISE"=w3773:cluster{"T-RISE (L)":dbl, "T-RISE (N)":dbl}, "Result Out"=w3775:bool, "file error"=w3778:errorcluster)  [unwired: 10 in]
                    n2251 = local write "TEMP RISE LAB01-2"(w3773) -> ()
                    n2252 = local write "FAIL LAB01-2"(w3776) -> ()
                    n2253 = local write "DISP LAB01-2"(w3779) -> ()
                    n2254 = local write "RESULT LAB01-2"(w3775) -> ()
                    n2255 = local write "data file error"(w3778) -> ()
                  }
                }
              }
              frame #2 {
                # "LAB02-1"
                n2256 = case shown="True" w3789 {
                  tunnel: w3791 -> [_ w3804]
                  tunnel: w3788 -> [_ w3801]
                  tunnel: w3790 -> [_ w3800]
                  frame False {
                  }
                  frame True {
                    n2257 = local read "TEMP START LAB02-1"() -> (w3806:cluster{"TL":dbl, "TN":dbl})
                    n2258 = local read "FAIL LAB02-1"() -> (w3797:cluster{"LO":dbl, "HI":dbl})
                    n2259 = local read "TDMS LAB02-1"() -> (w3805:refnum<k34>)
                    n2260 = local read "SET LAB02-1"() -> (w3802:T5)
                    n2261 = local read "DISP LAB02-1"() -> (w3803:T4)
                    n2262 = local read "SIG LAB02-1"() -> (w3807:T2)
                    n2263 = local read "RESULT LAB02-1"() -> (w3794:bool)
                    n2264 = Bundle("FAIL LAB02-1"=w3797, "SIG LAB02-1"=w3807, "TEMP START LAB02-1"=w3806, "DISP LAB02-1"=w3803, "SET LAB02-1"=w3802, "TDMS LAB02-1"=w3805) -> (w3792:T32)  [unwired: 1 in]
                    n2265 = call "sub vi - cycle&temp fail v6.vi"("Amps Lo?"=w3804, "Input Cluster"=w3792, "SELECT"=w3801, "Amps Hi?"=w3800, "Result In"=w3794) -> ("(FAIL) out"=w3796:cluster{"FAIL LO":dbl, "FAIL HI":dbl}, "(DISP) out"=w3799:T4, "T-RISE"=w3793:cluster{"T-RISE (L)":dbl, "T-RISE (N)":dbl}, "Result Out"=w3795:bool, "file error"=w3798:errorcluster)  [unwired: 10 in]
                    n2266 = local write "TEMP RISE LAB02-1"(w3793) -> ()
                    n2267 = local write "FAIL LAB02-1"(w3796) -> ()
                    n2268 = local write "DISP LAB02-1"(w3799) -> ()
                    n2269 = local write "RESULT LAB02-1"(w3795) -> ()
                    n2270 = local write "data file error"(w3798) -> ()
                  }
                }
              }
              frame #3 {
                # "LAB02-2"
                n2271 = case shown="True" w3809 {
                  tunnel: w3811 -> [_ w3824]
                  tunnel: w3808 -> [_ w3821]
                  tunnel: w3810 -> [_ w3820]
                  frame False {
                  }
                  frame True {
                    n2272 = local read "TEMP START LAB02-2"() -> (w3826:cluster{"TL":dbl, "TN":dbl})
                    n2273 = local read "FAIL LAB02-2"() -> (w3817:cluster{"LO":dbl, "HI":dbl})
                    n2274 = local read "TDMS LAB02-2"() -> (w3825:refnum<k34>)
                    n2275 = local read "SET LAB02-2"() -> (w3822:T5)
                    n2276 = local read "DISP LAB02-2"() -> (w3823:T4)
                    n2277 = local read "SIG LAB02-2"() -> (w3827:T2)
                    n2278 = local read "RESULT LAB02-2"() -> (w3814:bool)
                    n2279 = Bundle("FAIL LAB02-2"=w3817, "SIG LAB02-2"=w3827, "TEMP START LAB02-2"=w3826, "DISP LAB02-2"=w3823, "SET LAB02-2"=w3822, "TDMS LAB02-2"=w3825) -> (w3812:T33)  [unwired: 1 in]
                    n2280 = call "sub vi - cycle&temp fail v6.vi"("Amps Lo?"=w3824, "Input Cluster"=w3812, "SELECT"=w3821, "Amps Hi?"=w3820, "Result In"=w3814) -> ("(FAIL) out"=w3816:cluster{"FAIL LO":dbl, "FAIL HI":dbl}, "(DISP) out"=w3819:T4, "T-RISE"=w3813:cluster{"T-RISE (L)":dbl, "T-RISE (N)":dbl}, "Result Out"=w3815:bool, "file error"=w3818:errorcluster)  [unwired: 10 in]
                    n2281 = local write "TEMP RISE LAB02-2"(w3813) -> ()
                    n2282 = local write "FAIL LAB02-2"(w3816) -> ()
                    n2283 = local write "DISP LAB02-2"(w3819) -> ()
                    n2284 = local write "RESULT LAB02-2"(w3815) -> ()
                    n2285 = local write "data file error"(w3818) -> ()
                  }
                }
              }
              frame #4 {
                # "LAB03-1"
                n2286 = case shown="True" w3829 {
                  tunnel: w3831 -> [_ w3844]
                  tunnel: w3828 -> [_ w3841]
                  tunnel: w3830 -> [_ w3840]
                  frame False {
                  }
                  frame True {
                    n2287 = local read "TEMP START LAB03-1"() -> (w3846:cluster{"TL":dbl, "TN":dbl})
                    n2288 = local read "FAIL LAB03-1"() -> (w3837:cluster{"LO":dbl, "HI":dbl})
                    n2289 = local read "TDMS LAB03-1"() -> (w3845:refnum<k34>)
                    n2290 = local read "SET LAB03-1"() -> (w3842:T5)
                    n2291 = local read "DISP LAB03-1"() -> (w3843:T4)
                    n2292 = local read "SIG LAB03-1"() -> (w3847:T2)
                    n2293 = local read "RESULT LAB03-1"() -> (w3834:bool)
                    n2294 = Bundle("FAIL LAB03-1"=w3837, "SIG LAB03-1"=w3847, "TEMP START LAB03-1"=w3846, "DISP LAB03-1"=w3843, "SET LAB03-1"=w3842, "TDMS LAB03-1"=w3845) -> (w3832:T34)  [unwired: 1 in]
                    n2295 = call "sub vi - cycle&temp fail v6.vi"("Amps Lo?"=w3844, "Input Cluster"=w3832, "SELECT"=w3841, "Amps Hi?"=w3840, "Result In"=w3834) -> ("(FAIL) out"=w3836:cluster{"FAIL LO":dbl, "FAIL HI":dbl}, "(DISP) out"=w3839:T4, "T-RISE"=w3833:cluster{"T-RISE (L)":dbl, "T-RISE (N)":dbl}, "Result Out"=w3835:bool, "file error"=w3838:errorcluster)  [unwired: 10 in]
                    n2296 = local write "TEMP RISE LAB03-1"(w3833) -> ()
                    n2297 = local write "FAIL LAB03-1"(w3836) -> ()
                    n2298 = local write "DISP LAB03-1"(w3839) -> ()
                    n2299 = local write "RESULT LAB03-1"(w3835) -> ()
                    n2300 = local write "data file error"(w3838) -> ()
                  }
                }
              }
              frame #5 {
                # "LAB03-2"
                n2301 = case shown="True" w3849 {
                  tunnel: w3851 -> [_ w3864]
                  tunnel: w3848 -> [_ w3861]
                  tunnel: w3850 -> [_ w3860]
                  frame False {
                  }
                  frame True {
                    n2302 = local read "TEMP START LAB03-2"() -> (w3866:cluster{"TL":dbl, "TN":dbl})
                    n2303 = local read "FAIL LAB03-2"() -> (w3857:cluster{"LO":dbl, "HI":dbl})
                    n2304 = local read "TDMS LAB03-2"() -> (w3865:refnum<k34>)
                    n2305 = local read "SET LAB03-2"() -> (w3862:T5)
                    n2306 = local read "DISP LAB03-2"() -> (w3863:T4)
                    n2307 = local read "RESULT LAB03-2"() -> (w3854:bool)
                    n2308 = local read "SIG LAB03-2"() -> (w3867:T2)
                    n2309 = Bundle("FAIL LAB03-2"=w3857, "SIG LAB03-2"=w3867, "TEMP START LAB03-2"=w3866, "DISP LAB03-2"=w3863, "SET LAB03-2"=w3862, "TDMS LAB03-2"=w3865) -> (w3852:T35)  [unwired: 1 in]
                    n2310 = call "sub vi - cycle&temp fail v6.vi"("Amps Lo?"=w3864, "Input Cluster"=w3852, "SELECT"=w3861, "Amps Hi?"=w3860, "Result In"=w3854) -> ("(FAIL) out"=w3856:cluster{"FAIL LO":dbl, "FAIL HI":dbl}, "(DISP) out"=w3859:T4, "T-RISE"=w3853:cluster{"T-RISE (L)":dbl, "T-RISE (N)":dbl}, "Result Out"=w3855:bool, "file error"=w3858:errorcluster)  [unwired: 10 in]
                    n2311 = local write "FAIL LAB03-2"(w3856) -> ()
                    n2312 = local write "TEMP RISE LAB03-2"(w3853) -> ()
                    n2313 = local write "DISP LAB03-2"(w3859) -> ()
                    n2314 = local write "RESULT LAB03-2"(w3855) -> ()
                    n2315 = local write "data file error"(w3858) -> ()
                  }
                }
              }
              frame #6 {
                # "LAB04-1"
                n2316 = case shown="True" w3869 {
                  tunnel: w3871 -> [_ w3884]
                  tunnel: w3868 -> [_ w3881]
                  tunnel: w3870 -> [_ w3880]
                  frame False {
                  }
                  frame True {
                    n2317 = local read "TEMP START LAB04-1"() -> (w3886:cluster{"TL":dbl, "TN":dbl})
                    n2318 = local read "FAIL LAB04-1"() -> (w3877:cluster{"LO":dbl, "HI":dbl})
                    n2319 = local read "TDMS LAB04-1"() -> (w3885:refnum<k34>)
                    n2320 = local read "SET LAB04-1"() -> (w3882:T5)
                    n2321 = local read "DISP LAB04-1"() -> (w3883:T4)
                    n2322 = local read "SIG LAB04-1"() -> (w3887:T2)
                    n2323 = local read "RESULT LAB04-1"() -> (w3874:bool)
                    n2324 = Bundle("FAIL LAB04-1"=w3877, "SIG LAB04-1"=w3887, "TEMP START LAB04-1"=w3886, "DISP LAB04-1"=w3883, "SET LAB04-1"=w3882, "TDMS LAB04-1"=w3885) -> (w3872:T36)  [unwired: 1 in]
                    n2325 = call "sub vi - cycle&temp fail v6.vi"("Amps Lo?"=w3884, "Input Cluster"=w3872, "SELECT"=w3881, "Amps Hi?"=w3880, "Result In"=w3874) -> ("(FAIL) out"=w3876:cluster{"FAIL LO":dbl, "FAIL HI":dbl}, "(DISP) out"=w3879:T4, "T-RISE"=w3873:cluster{"T-RISE (L)":dbl, "T-RISE (N)":dbl}, "Result Out"=w3875:bool, "file error"=w3878:errorcluster)  [unwired: 10 in]
                    n2326 = local write "TEMP RISE LAB04-1"(w3873) -> ()
                    n2327 = local write "FAIL LAB04-1"(w3876) -> ()
                    n2328 = local write "DISP LAB04-1"(w3879) -> ()
                    n2329 = local write "RESULT LAB04-1"(w3875) -> ()
                    n2330 = local write "data file error"(w3878) -> ()
                  }
                }
              }
              frame #7 {
                # "LAB04-2"
                n2331 = case shown="True" w3889 {
                  tunnel: w3891 -> [_ w3904]
                  tunnel: w3888 -> [_ w3901]
                  tunnel: w3890 -> [_ w3900]
                  frame False {
                  }
                  frame True {
                    n2332 = local read "TEMP START LAB04-2"() -> (w3906:cluster{"TL":dbl, "TN":dbl})
                    n2333 = local read "FAIL LAB04-2"() -> (w3897:cluster{"LO":dbl, "HI":dbl})
                    n2334 = local read "TDMS LAB04-2"() -> (w3905:refnum<k34>)
                    n2335 = local read "SET LAB04-2"() -> (w3902:T5)
                    n2336 = local read "DISP LAB04-2"() -> (w3903:T4)
                    n2337 = local read "SIG LAB04-2"() -> (w3907:T2)
                    n2338 = local read "RESULT LAB04-2"() -> (w3894:bool)
                    n2339 = Bundle("FAIL LAB04-2"=w3897, "SIG LAB04-2"=w3907, "TEMP START LAB04-2"=w3906, "DISP LAB04-2"=w3903, "SET LAB04-2"=w3902, "TDMS LAB04-2"=w3905) -> (w3892:T37)  [unwired: 1 in]
                    n2340 = call "sub vi - cycle&temp fail v6.vi"("Amps Lo?"=w3904, "Input Cluster"=w3892, "SELECT"=w3901, "Amps Hi?"=w3900, "Result In"=w3894) -> ("(FAIL) out"=w3896:cluster{"FAIL LO":dbl, "FAIL HI":dbl}, "(DISP) out"=w3899:T4, "T-RISE"=w3893:cluster{"T-RISE (L)":dbl, "T-RISE (N)":dbl}, "Result Out"=w3895:bool, "file error"=w3898:errorcluster)  [unwired: 10 in]
                    n2341 = local write "TEMP RISE LAB04-2"(w3893) -> ()
                    n2342 = local write "FAIL LAB04-2"(w3896) -> ()
                    n2343 = local write "DISP LAB04-2"(w3899) -> ()
                    n2344 = local write "RESULT LAB04-2"(w3895) -> ()
                    n2345 = local write "data file error"(w3898) -> ()
                  }
                }
              }
              frame #8 {
                # "LAB05-1"
                n2346 = case shown="True" w3909 {
                  tunnel: w3911 -> [_ w3924]
                  tunnel: w3908 -> [_ w3921]
                  tunnel: w3910 -> [_ w3920]
                  frame False {
                  }
                  frame True {
                    n2347 = local read "TEMP START LAB05-1"() -> (w3926:cluster{"TL":dbl, "TN":dbl})
                    n2348 = local read "FAIL LAB05-1"() -> (w3917:cluster{"LO":dbl, "HI":dbl})
                    n2349 = local read "TDMS LAB05-1"() -> (w3925:refnum<k34>)
                    n2350 = local read "SET LAB05-1"() -> (w3922:T5)
                    n2351 = local read "DISP LAB05-1"() -> (w3923:T4)
                    n2352 = local read "SIG LAB05-1"() -> (w3927:T2)
                    n2353 = local read "RESULT LAB05-1"() -> (w3914:bool)
                    n2354 = Bundle("FAIL LAB05-1"=w3917, "SIG LAB05-1"=w3927, "TEMP START LAB05-1"=w3926, "DISP LAB05-1"=w3923, "SET LAB05-1"=w3922, "TDMS LAB05-1"=w3925) -> (w3912:T38)  [unwired: 1 in]
                    n2355 = call "sub vi - cycle&temp fail v6.vi"("Amps Lo?"=w3924, "Input Cluster"=w3912, "SELECT"=w3921, "Amps Hi?"=w3920, "Result In"=w3914) -> ("(FAIL) out"=w3916:cluster{"FAIL LO":dbl, "FAIL HI":dbl}, "(DISP) out"=w3919:T4, "T-RISE"=w3913:cluster{"T-RISE (L)":dbl, "T-RISE (N)":dbl}, "Result Out"=w3915:bool, "file error"=w3918:errorcluster)  [unwired: 10 in]
                    n2356 = local write "TEMP RISE LAB05-1"(w3913) -> ()
                    n2357 = local write "FAIL LAB05-1"(w3916) -> ()
                    n2358 = local write "DISP LAB05-1"(w3919) -> ()
                    n2359 = local write "RESULT LAB05-1"(w3915) -> ()
                    n2360 = local write "data file error"(w3918) -> ()
                  }
                }
              }
              frame #9 {
                # "LAB05-2"
                n2361 = case shown="True" w3929 {
                  tunnel: w3931 -> [_ w3944]
                  tunnel: w3928 -> [_ w3941]
                  tunnel: w3930 -> [_ w3940]
                  frame False {
                  }
                  frame True {
                    n2362 = local read "TEMP START LAB05-2"() -> (w3946:cluster{"TL":dbl, "TN":dbl})
                    n2363 = local read "FAIL LAB05-2"() -> (w3937:cluster{"LO":dbl, "HI":dbl})
                    n2364 = local read "TDMS LAB05-2"() -> (w3945:refnum<k34>)
                    n2365 = local read "SET LAB05-2"() -> (w3942:T5)
                    n2366 = local read "DISP LAB05-2"() -> (w3943:T4)
                    n2367 = local read "SIG LAB05-2"() -> (w3947:T2)
                    n2368 = local read "RESULT LAB05-2"() -> (w3934:bool)
                    n2369 = Bundle("FAIL LAB05-2"=w3937, "SIG LAB05-2"=w3947, "TEMP START LAB05-2"=w3946, "DISP LAB05-2"=w3943, "SET LAB05-2"=w3942, "TDMS LAB05-2"=w3945) -> (w3932:T39)  [unwired: 1 in]
                    n2370 = call "sub vi - cycle&temp fail v6.vi"("Amps Lo?"=w3944, "Input Cluster"=w3932, "SELECT"=w3941, "Amps Hi?"=w3940, "Result In"=w3934) -> ("(FAIL) out"=w3936:cluster{"FAIL LO":dbl, "FAIL HI":dbl}, "(DISP) out"=w3939:T4, "T-RISE"=w3933:cluster{"T-RISE (L)":dbl, "T-RISE (N)":dbl}, "Result Out"=w3935:bool, "file error"=w3938:errorcluster)  [unwired: 10 in]
                    n2371 = local write "TEMP RISE LAB05-2"(w3933) -> ()
                    n2372 = local write "FAIL LAB05-2"(w3936) -> ()
                    n2373 = local write "DISP LAB05-2"(w3939) -> ()
                    n2374 = local write "RESULT LAB05-2"(w3935) -> ()
                    n2375 = local write "data file error"(w3938) -> ()
                  }
                }
              }
            }
          }
          frame #16 {
            # "run calibration routine"
            n2376 = local read "CALIBRATE"() -> (w3948:bool)
            n2377 = case shown="True" w3948 {
              frame False {
              }
              frame True {
                n2378 = stacked-sequence {
                  seq-local: [w3949 _ _] -> [_ w3951 _]
                  frame #0 {
                    n2379 = call "CALIBRATION PASSWORD"() -> ("PASSWORD"=w3949:string)  [unwired: 17 in, 2 out]
                  }
                  frame #1 {
                    n2380 = Equal?(x=w3951, y="7777") -> (x = y?=w3950:bool)
                    n2381 = case shown="True" w3950 {
                      frame False {
                      }
                      frame True {
                        n2382 = stacked-sequence {
                          frame #0 {
                            n2383 = call "sub vi - calibration v1.vi"() -> ()  [unwired: 12 in]
                          }
                          frame #1 {
                            n2384 = call "sub vi - get calibration values v1.vi"() -> ("LAB01 (CAL)"=w3957:T7, "LAB02 (CAL)"=w3956:T8, "LAB03 (CAL)"=w3955:T7, "LAB04 (CAL)"=w3954:T7, "calibration file error out"=w3958:errorcluster, "LAB05 (CAL)"=w3953:T7)  [unwired: 10 in]
                            n2385 = local write "calibration file error out"(w3958) -> ()
                            n2386 = local write "CAL LAB04"(w3954) -> ()
                            n2387 = local write "CAL LAB05"(w3953) -> ()
                            n2388 = local write "CAL LAB01"(w3957) -> ()
                            n2389 = local write "CAL LAB02"(w3956) -> ()
                            n2390 = local write "CAL LAB03"(w3955) -> ()
                          }
                        }
                      }
                    }
                  }
                  frame #2 {
                    n2391 = local write "CALIBRATE"(FALSE) -> ()
                  }
                }
              }
            }
          }
          frame #17 {
            # "save certain settings to file"
            n2392 = String To Path(string="c:\\crabtree\\Set Up\\") -> (path=w3961:path)
            n2393 = Build Path(base path=w3961, name or relative path="settings.bin") -> (appended path=w3963:path)
            n2394 = Build Path(base path=w3961, name or relative path="mail.bin") -> (appended path=w3960:path)
            n2395 = Create Folder(path (use dialog)=w3961) -> (error out=w3966:errorcluster)  [unwired: 2 in, 2 out]
            n2396 = call <vilib>:"Clear Errors.vi"("error in (no error)"=w3966) -> ()  [unwired: 6 in, 1 out]
            n2397 = stacked-sequence {
              seq-local: [w3970 _] -> [_ w3983]
              tunnel: w3963 -> [_ w3984]
              tunnel: w3960 -> [_ w3982]
              frame #0 {
                n2398 = local read "C drive data root dir"() -> (w3969:path)
                n2399 = local read "Network Directory"() -> (w3975:path)
                n2400 = local read "SET LAB05-2"() -> (w3974:T5)
                n2401 = local read "SET LAB05-1"() -> (w3973:T5)
                n2402 = local read "SET LAB04-2"() -> (w3972:T5)
                n2403 = local read "SET LAB03-2"() -> (w3976:T5)
                n2404 = local read "SET LAB04-1"() -> (w3971:T5)
                n2405 = local read "SET LAB03-1"() -> (w3977:T5)
                n2406 = local read "SET LAB02-2"() -> (w3978:T5)
                n2407 = local read "SET LAB02-1"() -> (w3979:T5)
                n2408 = local read "SET LAB01-2"() -> (w3980:T5)
                n2409 = local read "SET LAB01-1"() -> (w3981:T5)
                n2410 = local read "RATE (Hz)"() -> (w3968:dbl)
                n2411 = local read "SAMPLES"() -> (w3967:dbl)
                n2412 = Bundle("SET LAB01-1"=w3981, "SET LAB01-2"=w3980, "SET LAB02-1"=w3979, "SET LAB02-2"=w3978, "SET LAB03-1"=w3977, "SET LAB03-2"=w3976, "SET LAB04-1"=w3971, "SET LAB04-2"=w3972, "SET LAB05-1"=w3973, "SET LAB05-2"=w3974, "Network Directory"=w3975, "C drive data root dir"=w3969, "RATE (Hz)"=w3968, "SAMPLES"=w3967) -> (w3970:T19)  [unwired: 1 in]
              }
              frame #1 {
                n2413 = event shown="[1] \"SET LAB01-1\", \"SET LAB01-2\", \"SET LAB02-1\", \"SET LAB02-2\", \"SET LAB03-1\", \"SET LAB03-2\", \"SET LAB04-1\", \"SET LAB04-2\", \"SET LAB05-1\", \"SET LAB05-2\", \"Network Directory\", \"C drive data root dir\", \"RATE (Hz)\", \"SAMPLES\": Value Change" {
                  selector: _ -> [_ _ _]
                  dyn-events: _ -> [_ _ _]
                  timeout: 10.0 -> [_ _ _]
                  tunnel: w3984 -> [_ w3986 _]
                  tunnel: w3983 -> [_ w3987 _]
                  tunnel: w3982 -> [_ _ w3998]
                  event Timeout {
                    n2414 = event-data() -> ()  [unwired: 1 in, 3 out]
                  }
                  event "SET LAB01-1", "SET LAB01-2", "SET LAB02-1", "SET LAB02-2", "SET LAB03-1", "SET LAB03-2", "SET LAB04-1", "SET LAB04-2", "SET LAB05-1", "SET LAB05-2", "Network Directory", "C drive data root dir", "RATE (Hz)", "SAMPLES": Value Change {
                    n2415 = event-data() -> ()  [unwired: 1 in, 6 out]
                    n2416 = Open/Create/Replace File(file path (use dialog)=w3986, operation (0:open)=T18."replace or create") -> (refnum out=w3992:refnum<file>, error out=w3991:errorcluster)  [unwired: 4 in, 1 out]
                    n2417 = Write to Binary File(file (use dialog)=w3992, data=w3987, error in=w3991) -> (refnum out=w3990:refnum<file>, error out=w3989:errorcluster)  [unwired: 3 in, 1 out]
                    n2418 = Close File(refnum=w3990, error in=w3989) -> (error out=w3988:errorcluster)  [unwired: 1 out]
                    n2419 = local write "data file error"(w3988) -> ()
                  }
                  event "MAIL SETTINGS.OUT SERVER ADDRESS", "MAIL SETTINGS.FROM ACCOUNT", "MAIL SETTINGS.USER NAME", "MAIL SETTINGS.PASSWORD", "Auto Mail Send", "TO (string):": Value Change {
                    n2420 = event-data() -> ()  [unwired: 1 in, 6 out]
                    n2421 = local read "MAIL SETTINGS"() -> (w3997:T6)
                    n2422 = local read "Auto Mail Send"() -> (w3995:bool)
                    n2423 = local read "TO (string):"() -> (w3994:string)
                    n2424 = Open/Create/Replace File(file path (use dialog)=w3998, operation (0:open)=T18."replace or create") -> (refnum out=w4003:refnum<file>, error out=w4002:errorcluster)  [unwired: 4 in, 1 out]
                    n2425 = Bundle("MAIL SETTINGS"=w3997, "Auto Mail Send"=w3995, "TO (string):"=w3994) -> (w3996:T40)  [unwired: 1 in]
                    n2426 = Write to Binary File(file (use dialog)=w4003, data=w3996, error in=w4002) -> (refnum out=w4001:refnum<file>, error out=w4000:errorcluster)  [unwired: 3 in, 1 out]
                    n2427 = Close File(refnum=w4001, error in=w4000) -> (error out=w3999:errorcluster)  [unwired: 1 out]
                    n2428 = local write "data file error"(w3999) -> ()
                  }
                }
              }
            }
          }
          frame #18 {
            # "mail control"
            n2429 = local read "MAIL SETTINGS"() -> (w4020:T6)
            n2430 = local read "Auto Mail Send"() -> (w4006:bool)
            n2431 = Unbundle(w4020) -> ("OUT SERVER ADDRESS"=w4019:string, "FROM ACCOUNT"=w4018:string, "TEST MAIL"=w4017:bool)  [unwired: 4 out]
            n2432 = stacked-sequence {
              tunnel: "TO (string):" -> [_ w4059]
              tunnel: w4020 -> [w4025 w4058]
              tunnel: w4019 -> [w4024 w4057]
              tunnel: w4018 -> [w4023 w4056]
              tunnel: w4017 -> [w4022 _]
              tunnel: w4006 -> [_ w4055]
              tunnel: w4016 -> [_ w4054]
              tunnel: w4015 -> [_ w4053]
              tunnel: w4014 -> [_ w4052]
              tunnel: w4013 -> [_ w4051]
              tunnel: w4012 -> [_ w4050]
              tunnel: w4011 -> [_ w4049]
              tunnel: w4010 -> [_ w4048]
              tunnel: w4009 -> [_ w4047]
              tunnel: w4008 -> [_ w4046]
              tunnel: w4007 -> [_ w4045]
              tunnel: "TO (string):" -> [w4021 _]
              frame #0 {
                # "mail test"
                n2433 = case shown="True" w4022 {
                  tunnel: w4025 -> [_ w4029]
                  tunnel: w4021 -> [_ w4028]
                  tunnel: w4024 -> [_ w4027]
                  tunnel: w4023 -> [_ w4026]
                  frame False {
                  }
                  frame True {
                    n2434 = stacked-sequence {
                      seq-local: [_ _ w4039 _] -> [_ _ _ w4040]
                      tunnel: w4029 -> [w4032 _ _ w4044]
                      tunnel: w4028 -> [_ _ w4037 _]
                      tunnel: w4027 -> [_ _ w4035 _]
                      tunnel: w4026 -> [_ _ w4036 _]
                      frame #0 {
                        n2435 = Bundle(cluster=w4032, "TEST MAIL STATUS"="TEST START") -> (w4030:T6)  [unwired: 6 in]
                        n2436 = local write "MAIL SETTINGS"(w4030) -> ()
                      }
                      frame #1 {
                        n2437 = Wait (ms)(milliseconds to wait=500) -> ()  [unwired: 1 out]
                      }
                      frame #2 {
                        n2438 = call "sub vi - send mail with attach v5.vi"("TO:"=w4037, "subject"="MAIL TEST FROM LAB PANEL", "from"=w4036, "out going server"=w4035, "message"="TEST MESSAGE") -> ("error out"=w4039:errorcluster)  [unwired: 10 in]
                      }
                      frame #3 {
                        n2439 = Bundle(cluster=w4044, "TEST MAIL"=FALSE, "TEST MAIL STATUS"="TEST END", "mail error"=w4040) -> (w4042:T6)  [unwired: 4 in]
                        n2440 = local write "MAIL SETTINGS"(w4042) -> ()
                      }
                    }
                  }
                }
              }
              frame #1 {
                # "mail report"
                n2441 = stacked-sequence {
                  seq-local: [_ w4124 _ _] -> [_ _ _ w4292]
                  seq-local: [_ _ w4205 _] -> [_ _ _ w4282]
                  seq-local: [w4069 _ _ _] -> [_ w4118 _ _]
                  seq-local: [w4068 _ _ _] -> [_ w4117 _ _]
                  seq-local: [w4066 _ _ _] -> [_ w4115 _ _]
                  seq-local: [w4067 _ _ _] -> [_ w4116 _ _]
                  seq-local: [w4065 _ _ _] -> [_ w4114 _ _]
                  seq-local: [w4064 _ _ _] -> [_ w4109 _ _]
                  seq-local: [w4063 _ _ _] -> [_ w4110 _ _]
                  seq-local: [w4062 _ _ _] -> [_ w4111 _ _]
                  seq-local: [w4061 _ _ _] -> [_ w4112 _ _]
                  seq-local: [w4060 _ _ _] -> [_ w4113 _ _]
                  tunnel: w4059 -> [_ _ _ w4293]
                  tunnel: w4058 -> [_ _ _ w4276]
                  tunnel: w4057 -> [_ _ _ w4290]
                  tunnel: w4056 -> [_ _ _ w4289]
                  tunnel: w4055 -> [w4100 _ _ w4284]
                  tunnel: w4054 -> [_ _ w4235 _]
                  tunnel: w4053 -> [_ _ w4232 _]
                  tunnel: w4052 -> [_ _ w4231 _]
                  tunnel: w4051 -> [_ _ w4230 _]
                  tunnel: w4050 -> [_ _ w4229 _]
                  tunnel: w4049 -> [_ _ w4228 _]
                  tunnel: w4048 -> [_ _ w4227 _]
                  tunnel: w4047 -> [_ _ w4226 _]
                  tunnel: w4046 -> [_ _ w4225 _]
                  tunnel: w4045 -> [_ _ w4224 _]
                  frame #0 {
                    n2442 = case shown="False" w4100 {
                      frame False {
                        n2443 = local write "mail control"("") -> ()
                      }
                      frame True {
                      }
                    }
                    n2444 = local read "SET LAB01-1"() -> (w4099:T5)
                    n2445 = local read "SET LAB01-2"() -> (w4098:T5)
                    n2446 = local read "SET LAB02-1"() -> (w4097:T5)
                    n2447 = local read "SET LAB02-2"() -> (w4096:T5)
                    n2448 = local read "SET LAB03-1"() -> (w4095:T5)
                    n2449 = local read "SET LAB04-1"() -> (w4093:T5)
                    n2450 = local read "SET LAB05-1"() -> (w4091:T5)
                    n2451 = local read "SET LAB03-2"() -> (w4094:T5)
                    n2452 = local read "SET LAB04-2"() -> (w4092:T5)
                    n2453 = local read "SET LAB05-2"() -> (w4090:T5)
                    n2454 = Unbundle(w4095) -> ("DESCRIPTION"=w4075:string)  [unwired: 4 out]
                    n2455 = Unbundle(w4094) -> ("DESCRIPTION"=w4074:string)  [unwired: 4 out]
                    n2456 = Unbundle(w4093) -> ("DESCRIPTION"=w4073:string)  [unwired: 4 out]
                    n2457 = Unbundle(w4090) -> ("DESCRIPTION"=w4070:string)  [unwired: 4 out]
                    n2458 = Unbundle(w4096) -> ("DESCRIPTION"=w4076:string)  [unwired: 4 out]
                    n2459 = Unbundle(w4092) -> ("DESCRIPTION"=w4072:string)  [unwired: 4 out]
                    n2460 = Unbundle(w4099) -> ("DESCRIPTION"=w4088:string)  [unwired: 4 out]
                    n2461 = Unbundle(w4097) -> ("DESCRIPTION"=w4077:string)  [unwired: 4 out]
                    n2462 = Unbundle(w4091) -> ("DESCRIPTION"=w4071:string)  [unwired: 4 out]
                    n2463 = Unbundle(w4098) -> ("DESCRIPTION"=w4078:string)  [unwired: 4 out]
                    n2464 = Concatenate Strings("[LAB05-1/", w4070) -> (w4060:string)
                    n2465 = Concatenate Strings("[LAB05-2/", w4071) -> (w4061:string)
                    n2466 = Concatenate Strings("[LAB04-2/", w4072) -> (w4062:string)
                    n2467 = Concatenate Strings("[LAB03-2/", w4074) -> (w4064:string)
                    n2468 = Concatenate Strings("[LAB04-1/", w4073) -> (w4063:string)
                    n2469 = Concatenate Strings("[LAB03-1/", w4075) -> (w4065:string)
                    n2470 = Concatenate Strings("[LAB01-2/", w4078) -> (w4068:string)
                    n2471 = Concatenate Strings("[LAB02-2/", w4076) -> (w4066:string)
                    n2472 = Concatenate Strings("[LAB01-1/", w4088) -> (w4069:string)
                    n2473 = Concatenate Strings("[LAB02-1/", w4077) -> (w4067:string)
                  }
                  frame #1 {
                    w4122 = "/"
                    w4123 = 2.0
                    n2474 = local read "DISP LAB01-2"() -> (w4203:T4)
                    n2475 = local read "DISP LAB01-1"() -> (w4204:T4)
                    n2476 = local read "DISP LAB02-1"() -> (w4202:T4)
                    n2477 = local read "DISP LAB03-2"() -> (w4199:T4)
                    n2478 = local read "DISP LAB02-2"() -> (w4201:T4)
                    n2479 = local read "DISP LAB03-1"() -> (w4200:T4)
                    n2480 = local read "DISP LAB04-2"() -> (w4197:T4)
                    n2481 = local read "DISP LAB04-1"() -> (w4198:T4)
                    n2482 = local read "DISP LAB05-1"() -> (w4196:T4)
                    n2483 = local read "DISP LAB05-2"() -> (w4195:T4)
                    n2484 = Unbundle(w4203) -> ("CYCLE"=w4187:dbl, "MINS"=w4186:dbl, "STATUS"=w4183:string)
                    n2485 = Unbundle(w4204) -> ("CYCLE"=w4192:dbl, "MINS"=w4191:dbl, "STATUS"=w4188:string)
                    n2486 = Unbundle(w4202) -> ("CYCLE"=w4180:dbl, "MINS"=w4179:dbl, "STATUS"=w4178:string)
                    n2487 = Unbundle(w4199) -> ("CYCLE"=w4167:dbl, "MINS"=w4166:dbl, "STATUS"=w4163:string)
                    n2488 = Unbundle(w4200) -> ("CYCLE"=w4172:dbl, "MINS"=w4171:dbl, "STATUS"=w4168:string)
                    n2489 = Unbundle(w4201) -> ("CYCLE"=w4177:dbl, "MINS"=w4176:dbl, "STATUS"=w4173:string)
                    n2490 = Unbundle(w4198) -> ("CYCLE"=w4162:dbl, "MINS"=w4161:dbl, "STATUS"=w4158:string)
                    n2491 = Unbundle(w4197) -> ("CYCLE"=w4157:dbl, "MINS"=w4156:dbl, "STATUS"=w4153:string)
                    n2492 = Unbundle(w4196) -> ("CYCLE"=w4152:dbl, "MINS"=w4151:dbl, "STATUS"=w4148:string)
                    n2493 = Unbundle(w4195) -> ("CYCLE"=w4194:dbl, "MINS"=w4193:dbl, "STATUS"=w4145:string)
                    n2494 = Number To Decimal String(number=w4180) -> (decimal integer string=w4182:string)  [unwired: 1 in]
                    n2495 = Number To Decimal String(number=w4177) -> (decimal integer string=w4175:string)  [unwired: 1 in]
                    n2496 = Number To Decimal String(number=w4172) -> (decimal integer string=w4170:string)  [unwired: 1 in]
                    n2497 = Number To Decimal String(number=w4187) -> (decimal integer string=w4185:string)  [unwired: 1 in]
                    n2498 = Number To Decimal String(number=w4167) -> (decimal integer string=w4165:string)  [unwired: 1 in]
                    n2499 = Number To Decimal String(number=w4192) -> (decimal integer string=w4190:string)  [unwired: 1 in]
                    n2500 = Number To Decimal String(number=w4194) -> (decimal integer string=w4147:string)  [unwired: 1 in]
                    n2501 = Number To Decimal String(number=w4162) -> (decimal integer string=w4160:string)  [unwired: 1 in]
                    n2502 = Number To Decimal String(number=w4157) -> (decimal integer string=w4155:string)  [unwired: 1 in]
                    n2503 = Number To Decimal String(number=w4152) -> (decimal integer string=w4150:string)  [unwired: 1 in]
                    n2504 = Number To Fractional String(number=w4179, precision (6)=w4123) -> (F-format string=w4181:string)  [unwired: 2 in]
                    n2505 = Number To Fractional String(number=w4166, precision (6)=w4123) -> (F-format string=w4164:string)  [unwired: 2 in]
                    n2506 = Number To Fractional String(number=w4176, precision (6)=w4123) -> (F-format string=w4174:string)  [unwired: 2 in]
                    n2507 = Number To Fractional String(number=w4171, precision (6)=w4123) -> (F-format string=w4169:string)  [unwired: 2 in]
                    n2508 = Number To Fractional String(number=w4156, precision (6)=w4123) -> (F-format string=w4154:string)  [unwired: 2 in]
                    n2509 = Number To Fractional String(number=w4161, precision (6)=w4123) -> (F-format string=w4159:string)  [unwired: 2 in]
                    n2510 = Number To Fractional String(number=w4186, precision (6)=w4123) -> (F-format string=w4184:string)  [unwired: 2 in]
                    n2511 = Number To Fractional String(number=w4151, precision (6)=w4123) -> (F-format string=w4149:string)  [unwired: 2 in]
                    n2512 = Number To Fractional String(number=w4191, precision (6)=w4123) -> (F-format string=w4189:string)  [unwired: 2 in]
                    n2513 = Number To Fractional String(number=w4193, precision (6)=w4123) -> (F-format string=w4146:string)  [unwired: 2 in]
                    n2514 = Concatenate Strings(w4122, w4165, w4122, w4164, w4122, w4163) -> (w4139:string)
                    n2515 = Concatenate Strings(w4122, w4160, w4122, w4159, w4122, w4158) -> (w4138:string)
                    n2516 = Concatenate Strings(w4122, w4155, w4122, w4154, w4122, w4153) -> (w4137:string)
                    n2517 = Concatenate Strings(w4122, w4150, w4122, w4149, w4122, w4148) -> (w4136:string)
                    n2518 = Concatenate Strings(w4122, w4147, w4122, w4146, w4122, w4145) -> (w4135:string)
                    n2519 = Concatenate Strings(w4122, w4190, w4122, w4189, w4122, w4188) -> (w4144:string)
                    n2520 = Concatenate Strings(w4122, w4170, w4122, w4169, w4122, w4168) -> (w4140:string)
                    n2521 = Concatenate Strings(w4122, w4185, w4122, w4184, w4122, w4183) -> (w4143:string)
                    n2522 = Concatenate Strings(w4122, w4182, w4122, w4181, w4122, w4178) -> (w4142:string)
                    n2523 = Concatenate Strings(w4122, w4175, w4122, w4174, w4122, w4173) -> (w4141:string)
                    n2524 = Concatenate Strings("]", "\r") -> (w4119:string)
                    n2525 = Concatenate Strings(w4114, w4140, w4119) -> (w4130:string)
                    n2526 = Concatenate Strings(w4116, w4142, w4119) -> (w4132:string)
                    n2527 = Concatenate Strings(w4115, w4141, w4119) -> (w4131:string)
                    n2528 = Concatenate Strings(w4111, w4137, w4119) -> (w4127:string)
                    n2529 = Concatenate Strings(w4112, w4136, w4119) -> (w4128:string)
                    n2530 = Concatenate Strings(w4110, w4138, w4119) -> (w4126:string)
                    n2531 = Concatenate Strings(w4109, w4139, w4119) -> (w4125:string)
                    n2532 = Concatenate Strings(w4113, w4135, w4119) -> (w4129:string)
                    n2533 = Concatenate Strings(w4117, w4143, w4119) -> (w4133:string)
                    n2534 = Concatenate Strings(w4118, w4144, w4119) -> (w4134:string)
                    n2535 = Concatenate Strings(w4134, w4133, w4132, w4131, w4130, w4125, w4126, w4127, w4128, w4129) -> (w4102:string)
                    n2536 = Concatenate Strings("[PANEL/", "DESC/", "CYCLES/", "MINS/", "STATUS]", "\r", w4102) -> (w4124:string)
                    "MAIL REPORT" <- w4124
                  }
                  frame #2 {
                    w4233 = "END"
                    n2537 = local read "mail control"() -> (w4234:string)
                    n2538 = case shown="False" w4229 {
                      tunnel: w4234 -> [w4258 _]
                      tunnel: w4233 -> [w4257 _]
                      tunnel: [w4256 FALSE] -> w4219
                      frame False {
                        n2539 = Equal?(x=w4258, y=w4257) -> (x = y?=w4256:bool)
                      }
                      frame True {
                      }
                    }
                    n2540 = case shown="False" w4235 {
                      tunnel: w4234 -> [w4274 _]
                      tunnel: w4233 -> [w4273 _]
                      tunnel: [w4272 FALSE] -> w4223
                      frame False {
                        n2541 = Equal?(x=w4274, y=w4273) -> (x = y?=w4272:bool)
                      }
                      frame True {
                      }
                    }
                    n2542 = case shown="False" w4232 {
                      tunnel: w4234 -> [w4270 _]
                      tunnel: w4233 -> [w4269 _]
                      tunnel: [w4268 FALSE] -> w4222
                      frame False {
                        n2543 = Equal?(x=w4270, y=w4269) -> (x = y?=w4268:bool)
                      }
                      frame True {
                      }
                    }
                    n2544 = case shown="False" w4230 {
                      tunnel: w4234 -> [w4262 _]
                      tunnel: w4233 -> [w4261 _]
                      tunnel: [w4260 FALSE] -> w4220
                      frame False {
                        n2545 = Equal?(x=w4262, y=w4261) -> (x = y?=w4260:bool)
                      }
                      frame True {
                      }
                    }
                    n2546 = case shown="False" w4231 {
                      tunnel: w4234 -> [w4266 _]
                      tunnel: w4233 -> [w4265 _]
                      tunnel: [w4264 FALSE] -> w4221
                      frame False {
                        n2547 = Equal?(x=w4266, y=w4265) -> (x = y?=w4264:bool)
                      }
                      frame True {
                      }
                    }
                    n2548 = Or(x=w4221, y=w4220) -> (x .or. y?=w4212:bool)
                    n2549 = Or(x=w4223, y=w4222) -> (x .or. y?=w4213:bool)
                    n2550 = Or(x=w4213, y=w4212) -> (x .or. y?=w4208:bool)
                    n2551 = case shown="False" w4225 {
                      tunnel: w4234 -> [w4242 _]
                      tunnel: w4233 -> [w4241 _]
                      tunnel: [w4240 FALSE] -> w4214
                      frame False {
                        n2552 = Equal?(x=w4242, y=w4241) -> (x = y?=w4240:bool)
                      }
                      frame True {
                      }
                    }
                    n2553 = case shown="False" w4224 {
                      tunnel: w4234 -> [w4238 _]
                      tunnel: w4233 -> [w4237 _]
                      tunnel: [w4236 FALSE] -> w4218
                      frame False {
                        n2554 = Equal?(x=w4238, y=w4237) -> (x = y?=w4236:bool)
                      }
                      frame True {
                      }
                    }
                    n2555 = case shown="False" w4226 {
                      tunnel: w4234 -> [w4246 _]
                      tunnel: w4233 -> [w4245 _]
                      tunnel: [w4244 FALSE] -> w4215
                      frame False {
                        n2556 = Equal?(x=w4246, y=w4245) -> (x = y?=w4244:bool)
                      }
                      frame True {
                      }
                    }
                    n2557 = case shown="False" w4228 {
                      tunnel: w4234 -> [w4254 _]
                      tunnel: w4233 -> [w4253 _]
                      tunnel: [w4252 FALSE] -> w4217
                      frame False {
                        n2558 = Equal?(x=w4254, y=w4253) -> (x = y?=w4252:bool)
                      }
                      frame True {
                      }
                    }
                    n2559 = case shown="False" w4227 {
                      tunnel: w4234 -> [w4250 _]
                      tunnel: w4233 -> [w4249 _]
                      tunnel: [w4248 FALSE] -> w4216
                      frame False {
                        n2560 = Equal?(x=w4250, y=w4249) -> (x = y?=w4248:bool)
                      }
                      frame True {
                      }
                    }
                    n2561 = Or(x=w4217, y=w4216) -> (x .or. y?=w4211:bool)
                    n2562 = Or(x=w4215, y=w4214) -> (x .or. y?=w4210:bool)
                    n2563 = Or(x=w4218, y=w4219) -> (x .or. y?=w4206:bool)
                    n2564 = Or(x=w4211, y=w4210) -> (x .or. y?=w4209:bool)
                    n2565 = Or(x=w4208, y=w4209) -> (x .or. y?=w4207:bool)
                    n2566 = Or(x=w4207, y=w4206) -> (x .or. y?=w4205:bool)
                  }
                  frame #3 {
                    n2567 = local read "on loops"() -> (w4288:dbl)
                    n2568 = local read "jig cycle"() -> (w4285:dbl)
                    n2569 = local read "Send Mail Now"() -> (w4279:bool)
                    n2570 = Add(x=w4288, y=3.0) -> (x+y=w4286:dbl)
                    n2571 = Equal?(x=w4285, y=w4286) -> (x = y?=w4280:bool)
                    n2572 = And(x=w4280, y=w4279) -> (x .and. y?=w4278:bool)
                    n2573 = And(x=w4284, y=w4280) -> (x .and. y?=w4283:bool)
                    n2574 = And(x=w4283, y=w4282) -> (x .and. y?=w4281:bool)
                    n2575 = Or(x=w4281, y=w4278) -> (x .or. y?=w4277:bool)
                    n2576 = case shown="True" w4277 {
                      tunnel: w4293 -> [_ w4299]
                      tunnel: w4292 -> [_ w4298]
                      tunnel: "Lab Panel Test Status" -> [_ w4297]
                      tunnel: w4290 -> [_ w4296]
                      tunnel: w4289 -> [_ w4295]
                      tunnel: w4276 -> [_ w4294]
                      frame False {
                      }
                      frame True {
                        n2577 = stacked-sequence {
                          tunnel: w4299 -> [w4307 _]
                          tunnel: w4298 -> [w4306 _]
                          tunnel: w4297 -> [w4305 _]
                          tunnel: w4296 -> [w4304 _]
                          tunnel: w4295 -> [w4303 _]
                          tunnel: w4294 -> [w4302 _]
                          frame #0 {
                            n2578 = call "sub vi - send mail with attach v5.vi"("TO:"=w4307, "subject"=w4305, "from"=w4303, "out going server"=w4304, "message"=w4306) -> ("error out"=w4301:errorcluster)  [unwired: 10 in]
                            n2579 = Bundle(cluster=w4302, "mail error"=w4301) -> (w4300:T6)  [unwired: 6 in]
                            n2580 = local write "MAIL SETTINGS"(w4300) -> ()
                          }
                          frame #1 {
                            n2581 = local write "mail control"("") -> ()
                            n2582 = local write "Send Mail Now"(FALSE) -> ()
                          }
                        }
                      }
                    }
                  }
                }
              }
            }
          }
        }
        n2583 = node-c288() -> ()  [unwired: 1 in, 1 out]
        "loops" <- w165
        "stop2" <- "stop"
      }
      n2584 = node-c288(w142) -> ()  [unwired: 1 out]
    }
  }
